vi "main4Ch.vi"() -> ()   [LabVIEW 2024]
doc: "Main VI for FLS imaging system."
uses:
  SubVI/DigitizerConfiguration/FLImDAQ.ctl
  <instrlib>/niScope/Controls/niScope trigger source.ctl
  SubVI/LabJack/LJ Pin Setting.ctl
  ConfigFiles/AimingBeamVideoConfig.ctl
  LaguerreDeconLib/DeconEngineClass/LaguerreDeconEngineClass.lvclass/LaguerreDeconEngineClass.ctl
  <vilib>/Utility/error.llb/DialogType.ctl
  LaguerreDeconLib/DeconEngineClass/LaguerreDeconEngineClass.lvclass
  <vilib>/event_ctls.llb/usereventprio.ctl
  <vilib>/Utility/miscctls.llb/LVMinMaxIncTypeDef.ctl
  SubVI/APD/APDClass.lvclass
  <vilib>/Analysis/baseanly.llb/Mean (DBL).vi
  SubVI/GlobalVariables.vi
  <vilib>/addons/control/pid/pid.llb/PID (DBL).vi
  <instrlib>/niScope/Acquire/Fetch/niScope Multi Fetch Binary 16.vi
  <vilib>/Instr/_visa.llb/VISA Configure Serial Port (Instr).vi
  <userlib>/_OpenG.lib/file/file.llb/openg_file.lvlib
  <userlib>/_OpenG.lib/time/time.llb/openg_time.lvlib
  <vilib>/Analysis/NI_AALBase.lvlib
  <vilib>/Utility/miscctls.llb/LVPointTypeDef.ctl
  <vilib>/addons/control/pid/NI_PID_pid.lvlib
panel:
  in  "Overlay selection":u16(ring)=1 items=["Gain", "Lifetime"]
  out "Record Backlog 2":i32
  in  "Auto gain ch4":bool=TRUE caption="Auto gain ch3"
  in  "V 4":dbl caption="Gain 3" min=0.0 max=4.67 step=0.1
  out "Gain4":dbl
  out "Lifetime 4":dbl caption="Lifetime 3"
  out "IntR4":dbl format="%#_2g"
  out "SNR4":dbl format="%#_3g"
  out "Channel 4":dbl[][](graph) caption="Channel 3"
  out "RunStartTime":u32
  out "Dig1 Temp":dbl
  out "Dig2 Temp":dbl
  out "Visualization PC video source":T1
  in  "V target(1.0)":dbl=1.0 caption="V target(1.5)" min=0.3 max=1.5 step=0.1 format="%#_4g"
  out "SNR3":dbl format="%#_3g"
  out "SNR2":dbl format="%#_3g"
  out "SNR1":dbl format="%#_3g"
  in  "Show BG removed?":bool=TRUE
  out "IntR3":dbl format="%#_2g"
  out "IntR2":dbl format="%#_2g"
  out "IntR1":dbl format="%#_2g"
  in  "Video Display":bool
  out "Gain3":dbl
  out "Gain2":dbl
  out "Gain1":dbl
  in  "Skip Data Save?":bool
  out "Aq Loop?":bool
  out "ML?":bool
  out "aquisition loop Error Out":errorcluster
  out "Laser f (Hz)":dbl
  out "Record Backlog":i32
  out "Fetch Record #":i32
  out "Sync Success?":bool
  out "Disclamer":picture
  out "Calibration #":i8
  out "BG #":i8
  in  "TCP Connect":bool
  out "Help":string
  in  "355nm Laser toggle":bool caption="355nm 460Hz"
  in  "Cali&iRF alignment":bool
  in  "Background":bool
  in  "Aiming beam toggle":bool caption="445nm 0Hz 32mA"
  out "Lifetime 3":dbl
  out "Lifetime 2":dbl
  in  "Auto gain ch3":bool=TRUE
  in  "Auto gain ch2":bool=TRUE
  in  "Auto gain ch1":bool=TRUE
  out "Run #":i8
  in  "StopButton":bool caption="Stop"
  out "Aquisition Status:":bool
  in  "StartButton":bool caption="Start"
  in  "V 3":dbl caption="Gain 3" min=0.0 max=4.65 step=0.1
  in  "V 2":dbl caption="Gain 2" min=0.0 max=4.59 step=0.1
  out "Lifetime 1":dbl
  in  "V 1":dbl caption="Gain 1" min=0.0 max=4.63 step=0.1 format="%#_4g"
  in  "Video Source":enum32{"Camera", "FrameGrabber"}(radio)
  out "Case #":string
  out "System Hardware Connection Status":T2
  out "Channel 3":dbl[][](graph)
  out "Channel 2":dbl[][](graph)
  out "Channel 1":dbl[][](graph)
  in  "Tab Control":T3(tab)
  out "display loop timing(ms)":u32
  out "Aquisition loop timing(ms)":u32 format="%.2f"
  out "DisplayLoop":i32
  out "PID loop":i32 caption="processing loop"
  out "PID loop timing(ms)":u32 caption="processing loop timing(ms)"
  out "Communication loop(ms)":u32
  out "laser EM lamp V":dbl format="%0.6f"
  out "Decon Loop timing (ms)":dbl
  out "Auisition Loop idx":i32
  out "LJ process (ms)":u32
  out "LJ time(ms)":u32[](array[numeric])
  out "output variable":i32
  out "Lifetime (ns)":dbl(graph)
  out "DeCon Speed(ms)":dbl(graph)
  in  "Truncation":u32=600
  out "iRF Graph":dbl[][](graph)
  in  "Show BG":bool
  out "iRF length":i32
  out "BG length":i32
  out "data length":i32
  out "LJ Pinout":T4={"Ch1 Bias"="DAC0", "Ch2 Bias"="DAC1", "Ch3 Bias"="DAC2", "Ch4 Bias"="DAC0", "355 PWM"="FIO0", "AimingBeam PWM"="FIO2", "Laser Ready"="FIO3", "Interlock"="FIO1", "Laser Start/Stop"="FIO1", "Red LED"="FIO1", "Green LED"="DIO3", "Foot Pedal"="DIO15"}
  out "FLImDAQ":T5={"Digitizer 1"="", "Digitizer 2"="", "Channel"=enum."Channel 0", "trigger source"="VAL_EXTERNAL", "trigger level"=0.5, "trigger delay"=1.35e-07, "min sample rate"=12500000000.0, "min record length"=2500, "vertical range"=1.0, "vertical offset"=-0.25, "Waveform to Avg"=2000} caption="FLIm DAQ Configuration" {"trigger delay" format="%^#.4e"; "trigger level" min=0.0 max=3.5 step=0.5 format="%.2f"; "vertical offset" format="%.4f"; "vertical range" format="%.2f"; "min sample rate" format="%#.2p"}
  in  "Sys Reconfig":bool
  out "data out(communcation loop)":string
  out "PID loop error out":errorcluster caption="processing Error Out"
  out "decon error out":errorcluster
  out "Laser Rep Rate":dbl
  out "V4 Size":i32 caption="V3 Size"
  in  "Data Class":enum16{"Data", "BG", "Cali"}(ring)
  out "V1 Size":i32
  out "V2 Size":i32
  out "V3 Size":i32
  out "data Size":i32[](array[numeric])
  out "State log":string
  out "SysConfigCluster":T7
  in  "Ch4 PID gains":T8={"proportional gain (Kc)"=30.0, "integral time (Ti, min)"=0.0003, "derivative time (Td, min)"=1e-05}
  in  "Ch3 PID gains":T8={"proportional gain (Kc)"=30.0, "integral time (Ti, min)"=0.0003, "derivative time (Td, min)"=1e-05}
  in  "Ch2 PID gains":T8={"proportional gain (Kc)"=30.0, "integral time (Ti, min)"=0.0003, "derivative time (Td, min)"=1e-05}
  in  "Ch1 PID gains":T8={"proportional gain (Kc)"=30.0, "integral time (Ti, min)"=0.0003, "derivative time (Td, min)"=1e-05}
  in  "Quit":bool
  in  "Radio Buttons":T9(radio)=enum."Ch2" caption="DeCon Chan"
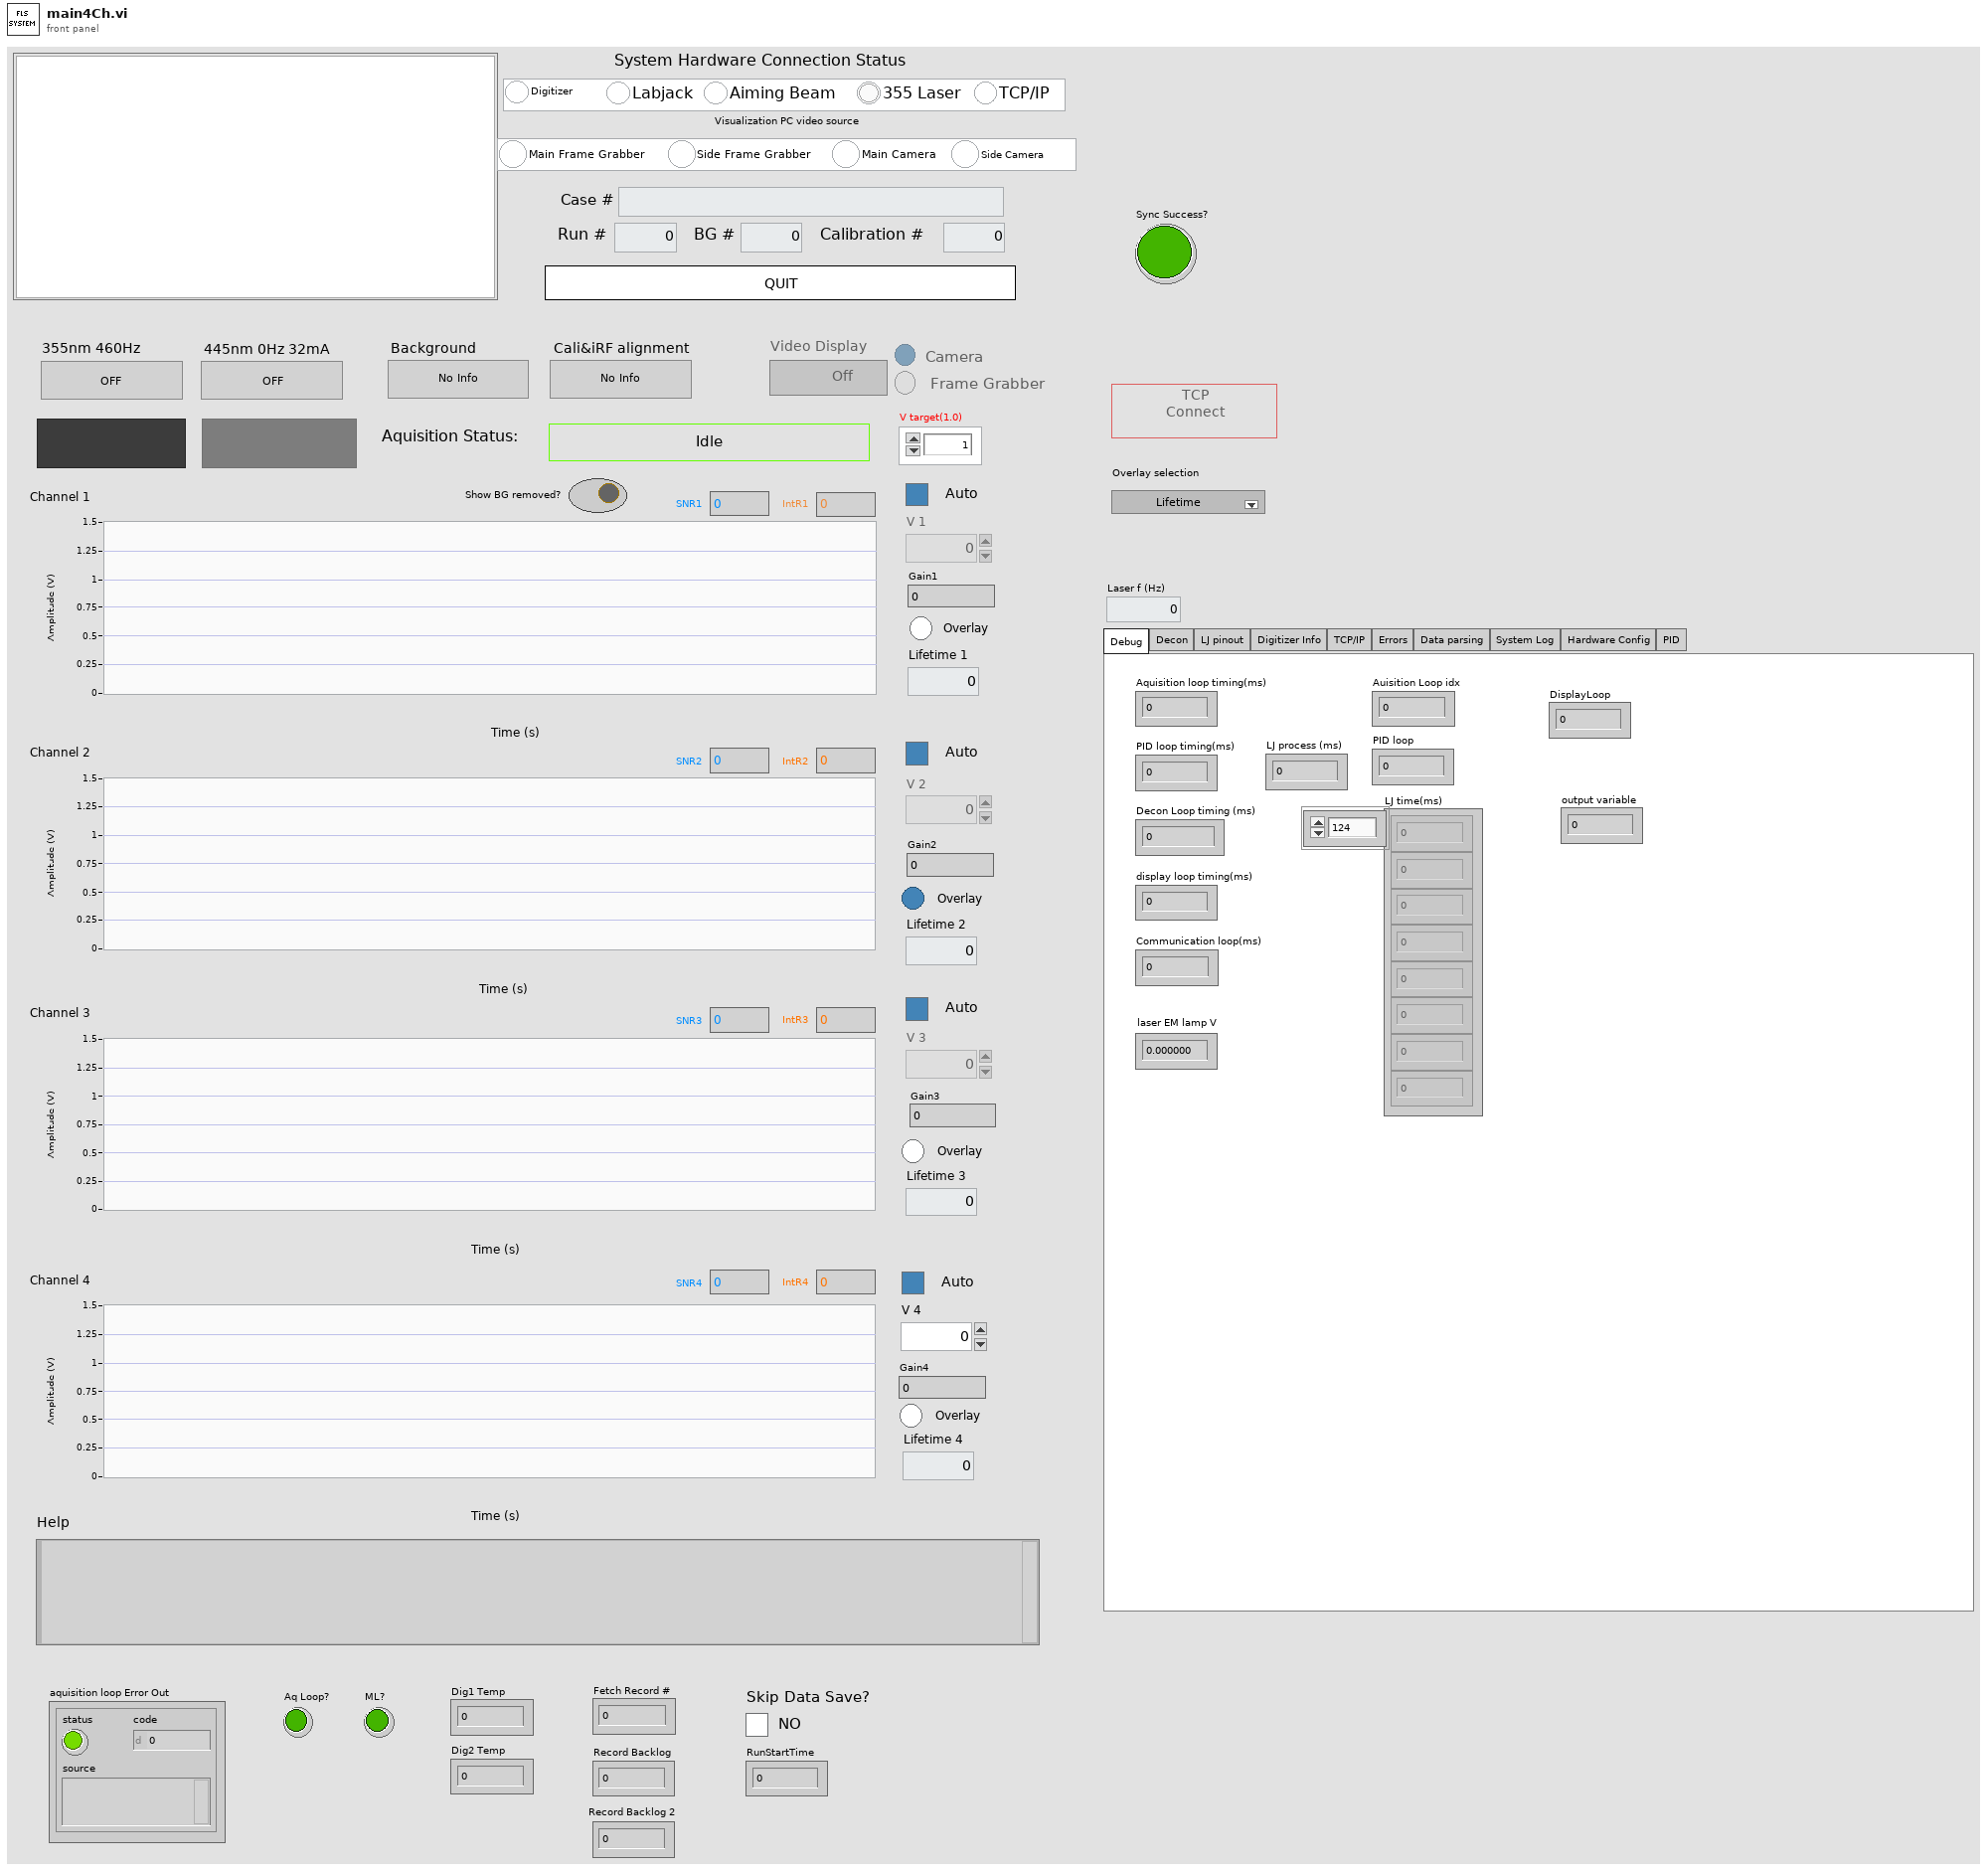
[diagram p1: front panel]
types:
  T1 = cluster{"Main Frame Grabber":bool, "Side Frame Grabber":bool, "Main Camera":bool, "Side Camera":bool}
  T2 = cluster{"Digitizer":bool, "Labjack":bool, "Aiming Beam":bool, "355 Laser":bool, "TCP/IP":bool}
  T3 = enum32{"Debug", "Decon", "LJ pinout", "Digitizer Info", "TCP/IP", "Errors", "Data parsing", "System Log", "Hardware Config", "PID"}
  T4 = typedef "LJ Pin Setting.ctl" = cluster{"Ch1 Bias":string, "Ch2 Bias":string, "Ch3 Bias":string, "Ch4 Bias":string, "355 PWM":string, "AimingBeam PWM":string, "Laser Ready":string, "Interlock":string, "Laser Start/Stop":string, "Red LED":string, "Green LED":string, "Foot Pedal":string}
  T5 = typedef "FLImDAQ.ctl" = cluster{"Digitizer 1":refnum<k15>, "Digitizer 2":refnum<k15>, "Channel":enum16{"Channel 0", "Channel 1", "Channel 0&1"}, "trigger source":T6, "trigger level":dbl, "trigger delay":dbl, "min sample rate":dbl, "min record length":i32, "vertical range":dbl, "vertical offset":dbl, "Waveform to Avg":i16}
  T6 = typedef "niScope trigger source.ctl" = string
  T7 = cluster{"Ch1Enable?":bool, "Ch2Enable?":bool, "Ch3Enable?":bool, "Ch1AutoGain?":bool, "Ch2AutoGain?":bool, "Ch3AutoGain?":bool, "AimingBeamEnable?":bool}
  T8 = cluster{"proportional gain (Kc)":dbl, "integral time (Ti, min)":dbl, "derivative time (Td, min)":dbl}
  T9 = enum32{"No Selection", "Ch1", "Ch2", "Ch3", "Ch4"}
  T10 = cluster{"remote start event":refnum<user-event>, "remote stop  event":refnum<user-event>}
  T11 = enum8{"Enabled", "Disabled", "Disabled and Grayed Out"}
  T12 = enum16{"open", "replace", "create", "open or create", "replace or create", "replace or create with confirmation"}
  T13 = cluster{"CH1":dbl[][], "CH2":dbl[][], "CH3":dbl[][], "CH4":dbl[][], "Gain cluster":cluster{"V1":dbl, "V2":dbl, "V3":dbl, "V4":dbl}}
  T14 = cluster{"idx":i32, "CH1&2":dbl[][], "CH3":dbl[][], "V cluster":cluster{"V1":dbl, "V2":dbl, "V3":dbl, "V4":dbl}}
  T15 = typedef "usereventprio.ctl" = enum32{"high priority", "normal priority"}
  T16 = cluster{"actualSamples":i32, "absoluteInitialX":dbl, "relativeInitialX":dbl, "xIncrement":dbl, "offset":dbl, "gain":dbl, "reserved1":dbl, "reserved2":dbl}[]
  T17 = cluster{"V1 out":dbl, "V2 out":dbl, "V3 out":dbl, "V3 out":dbl}
  T18 = cluster{i32, dbl[][], dbl[][], cluster{"V1 out":dbl, "V2 out":dbl, "V3 out":dbl, "V3 out":dbl}}
  T19 = cluster{"Ch1 iRF":dbl[], "Ch2 iRF":dbl[], "Ch3 iRF":dbl[], "Ch4 iRF":dbl[]}
  T20 = enum16{"open", "open or create", "create or replace", "create", "open (read-only)"}
  T21 = enum32{"Invalid", "Standard", "Closed", "Hidden", "Minimized", "Maximized"}
  T22 = enum32{"invalid app kind", "Development System", "Run Time System", "Student Edition", "Embedded LabVIEW", "Evaluation", "Custom"}
  T23 = enum32{"Bad", "Idle", "Run top level", "Running"}
  T24 = enum16{"Standard", "Buffered", "CRLF", "Immediate"}
  T25 = typedef "AimingBeamVideoConfig.ctl" = cluster{"DeCon Channel":enum16{"1", "2", "3"}, "Scale Bar":bool, "Scale Low":dbl, "Scale High":dbl, "ANSI":dbl, "Radius":dbl, "3D?":bool, "Firefly?":bool, "Pentero?":bool}
  T26 = cluster{"Core":cluster{"Current VI Reference":refnum<vi>, "Close Panel on Exit?":bool}, "SysConfigCluster":cluster{"Ch1Enable?":bool, "Ch2Enable?":bool, "Ch3Enable?":bool, "Ch1AutoGain?":bool, "Ch2AutoGain?":bool, "Ch3AutoGain?":bool, "AimingBeamEnable?":bool}, "System Status":cluster{"Digitizer":bool, "Labjack":bool, "Aiming Beam":bool, "355 Laser":bool, "TCP/IP":bool}, "IDs":cluster{"RunID":i8, "BG ID":i8, "Cali ID":i8}, "CaseID":string, "DefaultPath":path, "Pathes":cluster{"DataPath":path, "BG Path":path, "iRFPath":path, "CaliPath":path}, "FLImDAQ":cluster{"resource name":refnum<k15>, "resource name 2":refnum<k15>, "Channel":enum16{"Channel 0", "Channel 1", "Channel 0&1"}, "trigger source":T6, "trigger level":dbl, "trigger delay":dbl, "min sample rate":dbl, "min record length":i32, "vertical range":dbl, "vertical offset":dbl, "Waveform to Avg":i32}, "SysRunning?":bool, "AB Cluster":cluster{"Aiming Beam COM Port":refnum<visa-resource-name>, "Min Current":dbl, "Max Current":dbl, "Default Current":dbl, "Freq":i32}, "LJ Pinout":T4, "355 PWM setting":cluster{"DIO_EF_CLOCK1_DIVISOR":i16, "DIO_EF_CLOCK1_ROLL_VALUE":i32, "DIO#_EF_INDEX":i16, "DIO#_EF_OPTIONS":i16, "DIO#_EF_CONFIG_A":i32}, "AB PWM setting":cluster{"DIO_EF_CLOCK1_DIVISOR":i16, "DIO_EF_CLOCK1_ROLL_VALUE":i32, "DIO#_EF_INDEX":i16, "DIO#_EF_OPTIONS":i16, "DIO#_EF_CONFIG_A":i32}, "Last Trigger":u32, "niTClk sessions":refnum<k20>[], "Laser start tic":u32, "TCP attempt count":i32, "Ch1Data":dbl[][], "Ch2Data":dbl[][], "Ch3Data":dbl[][], "Ch4Data":dbl[][], "V1":dbl[], "V2":dbl[], "V3":dbl[], "V4":dbl[], "SlowTimer":u32, "FastTimer":u32, "listener ID":refnum<k5>, "TempPath":path, "CaliPath":path, "LED vi reference":refnum<vi>, "Aquisition Timer":u32, "APDSerialNum":cluster{"Ch1APDSerial#":string, "Ch2APDSerial#":string, "Ch3APDSerial#":string, "Ch4APDSerial#":string}, "VideoConfig":T25, "LED vi ref open?":bool, "video source":cluster{"Main Frame Grabber":bool, "Side Frame Grabber":bool, "Main Camera":bool, "Side Camera":bool}, "bothVidSourceAvail":bool}
  T27 = typedef "LVCursorListTypeDef.ctl" = cluster{"Name":string, "Color":u32, "Style":u8, "Point Style":u8, "Name Visible":bool, "Allow Drag":bool, "Cursor Mode":u32, "Plot":i32, "Index":i32, "Position":cluster{"X":dbl, "Y":dbl}, "X Scale":u32, "Y Scale":u32, "Watch Plots":i32[], "Watch All Plots":bool, "Plot Area":i32, "Label Offset":cluster{"X":dbl, "Y":dbl}}[]
  T28 = cluster{"Name":string, "Color":u32, "Style":u8, "Point Style":u8, "Name Visible":bool, "Allow Drag":bool, "Cursor Mode":u32, "Plot":i32, "Index":i32, "Position":cluster{"X":dbl, "Y":dbl}, "X Scale":u32, "Y Scale":u32, "Watch Plots":i32[], "Watch All Plots":bool, "Plot Area":i32, "Label Offset":cluster{"X":dbl, "Y":dbl}}
  T29 = cluster{"Ch1APDSerial#":string, "Ch2APDSerial#":string, "Ch3APDSerial#":string, "Ch4APDSerial#":string}
  T30 = cluster{"DataPath":path, "BG Path":path, "iRFPath":path, "CaliPath":path}
  T31 = cluster{"DIO_EF_CLOCK1_DIVISOR":i16, "DIO_EF_CLOCK1_ROLL_VALUE":i32, "DIO#_EF_INDEX":i16, "DIO#_EF_OPTIONS":i16, "DIO#_EF_CONFIG_A":i32}
  T32 = cluster{"Aiming Beam COM Port":refnum<visa-resource-name>, "Min Current":dbl, "Max Current":dbl, "Default Current":dbl, "Freq":i32}
  T33 = cluster{"resource name":refnum<k15>, "resource name 2":refnum<k15>, "Channel":enum16{"Channel 0", "Channel 1", "Channel 0&1"}, "trigger source":T6, "trigger level":dbl, "trigger delay":dbl, "min sample rate":dbl, "min record length":i32, "vertical range":dbl, "vertical offset":dbl, "Waveform to Avg":i32}
  T34 = cluster{"Current VI Reference":refnum<vi>, "Close Panel on Exit?":bool}
  T35 = cluster{"Channel 1":dbl[], "Channel 2":dbl[], "Channel 3":dbl[], "Channel 4":dbl[]}
  T36 = cluster{"V 1":dbl[], "V 2":dbl[], "V 3":dbl[], "V 4":dbl[]}
  T37 = cluster{"Ch1 WF":dbl[], "Ch2 WF":dbl[], "Ch3 WF":dbl[], "Ch4 WF":dbl[], "V1":dbl, "V2":dbl, "V3":dbl, "V4":dbl}
  T38 = typedef "iRFData.ctl" = cluster{"dt":dbl, "NumOfWFs":i32, "WFLength":i32, "iRFCtrlV":dbl[], "iRFWFsAvg":dbl[][], "iRFRaw":dbl[][]}
  T39 = cluster{"mean":dbl, "mean":dbl, "mean":dbl, "mean":dbl}
  T40 = cluster{"V1":dbl, "V2":dbl, "V3":dbl, "V4":dbl}[]
  T41 = cluster{"DataPath":path, "CaseID":string, "RunID":i16, "Ch1Data":dbl[][], "Ch2Data":dbl[][], "Ch3Data":dbl[][], "Ch4Data":dbl[][], "V1":dbl[], "V2":dbl[], "V3":dbl[], "V4":dbl[], "LaserRepRate":u16, "WFAverage":i16, "RunStartTime":u64}
  T42 = typedef "DialogType.ctl" = u16
  T43 = typedef "LJ PWM Setting.ctl" = cluster{"DIO_EF_CLOCK1_DIVISOR":i16, "DIO_EF_CLOCK1_ROLL_VALUE":i32, "DIO#_EF_INDEX":i16, "DIO#_EF_OPTIONS":i16, "DIO#_EF_CONFIG_A":i32}
  T44 = typedef "AimingBeam.ctl" = cluster{"Aiming Beam COM Port":refnum<visa-resource-name>, "Min Current":dbl, "Max Current":dbl, "Default Current":dbl, "Frequency(Hz)":u32}
  T45 = cluster{"DC1":i32, "DC2":i32, "BG1":i32, "BG2":i32}
  T46 = typedef "LVMinMaxIncTypeDef.ctl" = cluster{"Minimum":dbl, "Maximum":dbl, "Increment":dbl}
  T47 = typedef "LVBoundsTypeDef.ctl" = cluster{"Width":u32, "Height":u32}
  T48 = typedef "imagedata.ctl" = cluster{"image type":i32, "image depth":i32, "image":u8[], "mask":u8[], "colors":u32[], "Rectangle":cluster{"left":i16, "top":i16, "right":i16, "bottom":i16}}
  T49 = cluster{"DC Idx1":i32, "DC Idx2":i32, "BG Idx1":i32, "BG Idx2":i32}
  T50 = cluster{dbl[][], dbl[][], dbl[][], dbl[][], "V cluster":cluster{"V1":dbl, "V2":dbl, "V3":dbl, "V4":dbl}}
  T51 = typedef "LVPointTypeDef.ctl" = cluster{"Horizontal":i16, "Vertical":i16}
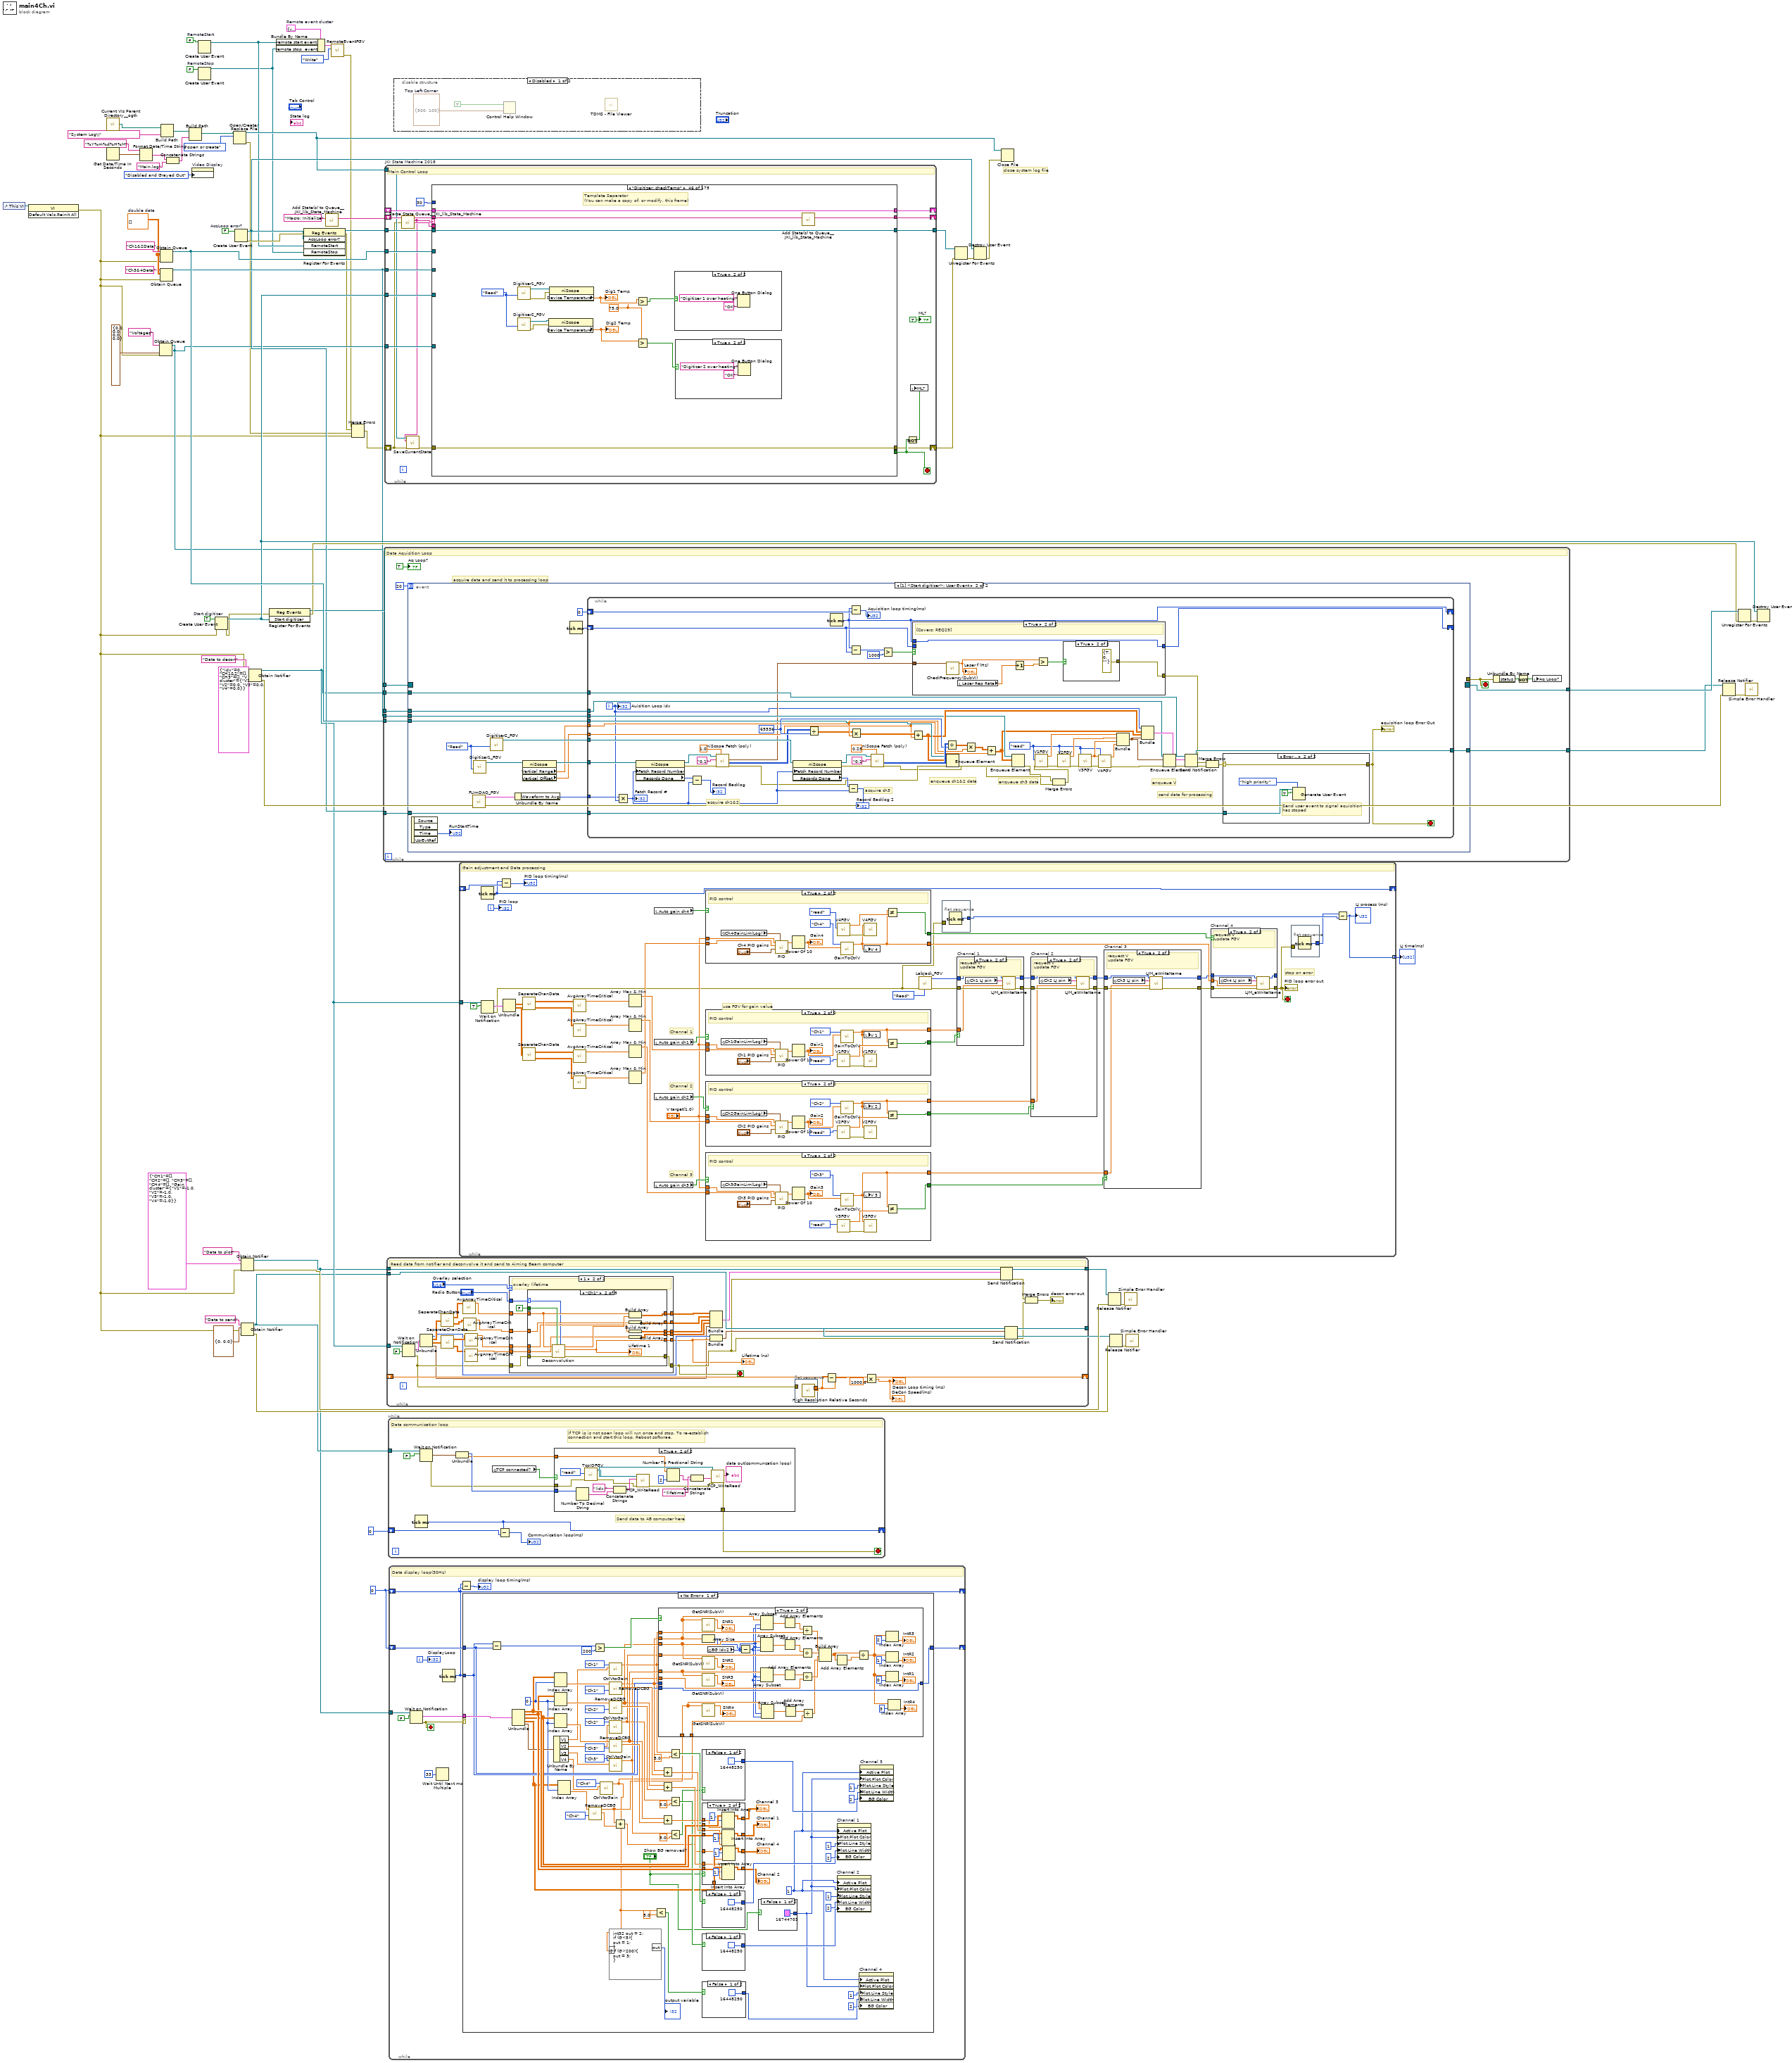
[diagram p0: block diagram]
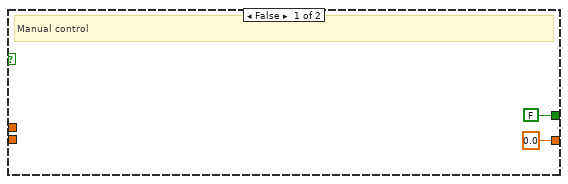
[diagram p6: hidden frame]
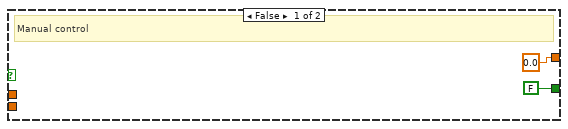
[diagram p7: hidden frame]
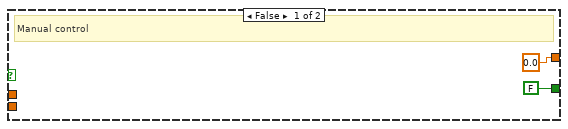
[diagram p8: hidden frame]
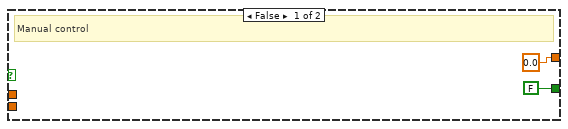
[diagram p9: hidden frame]
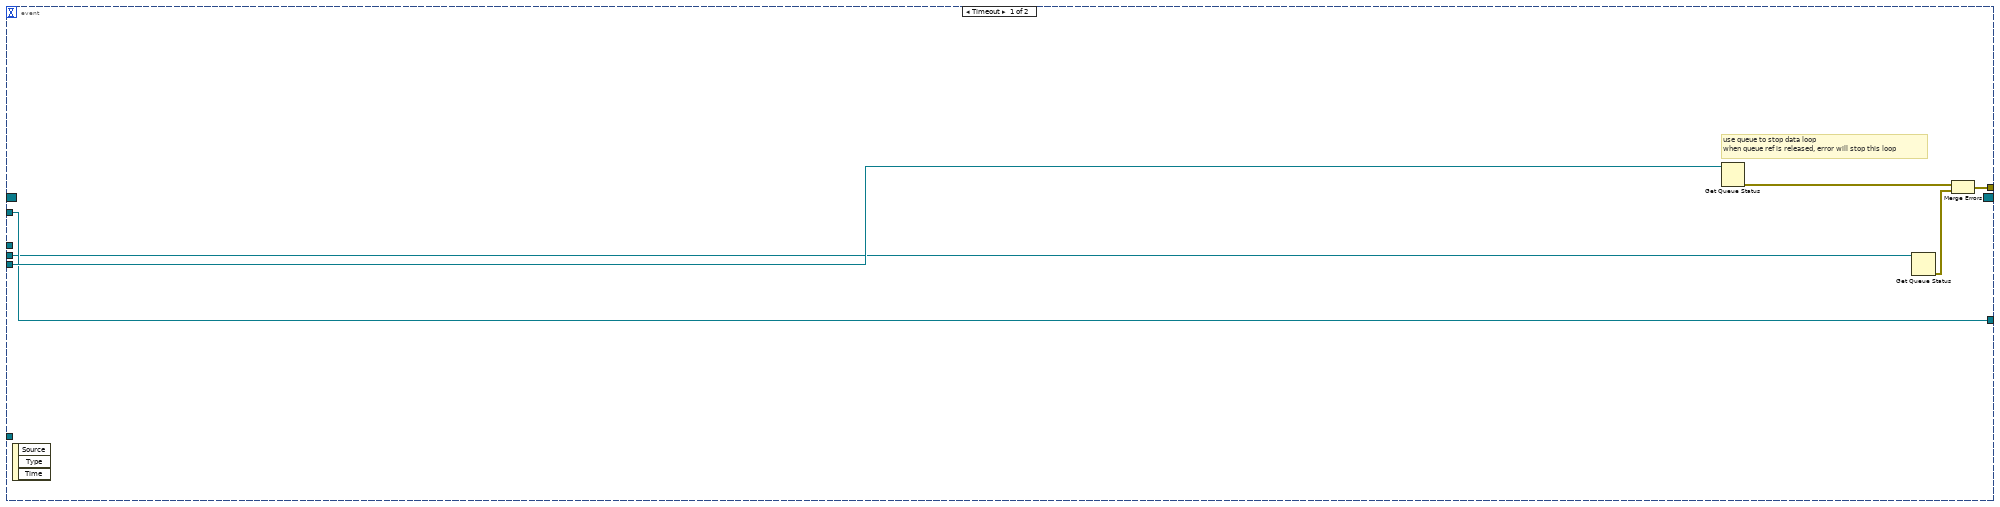
[diagram p10: hidden frame]
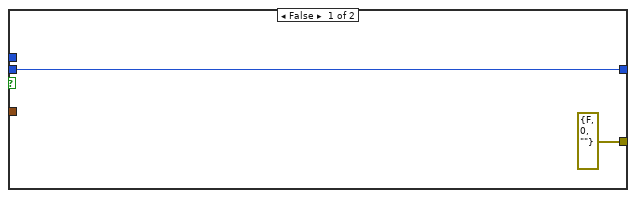
[diagram p11: hidden frame]
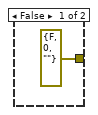
[diagram p12: hidden frame]
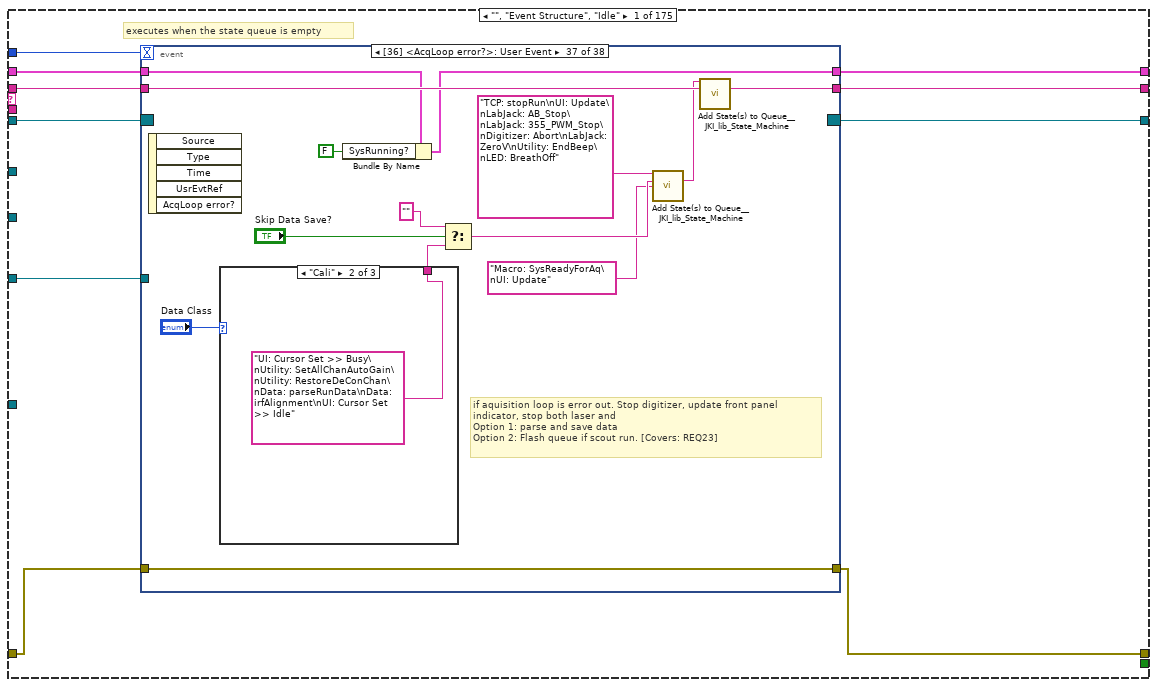
[diagram p14: hidden frame]
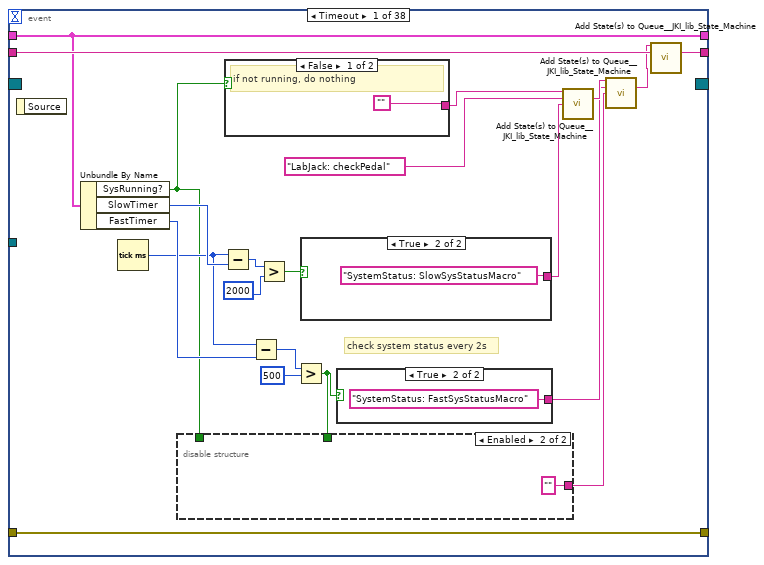
[diagram p15: hidden frame]
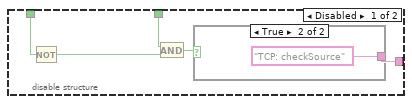
[diagram p16: hidden frame]
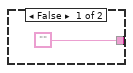
[diagram p17: hidden frame]
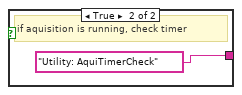
[diagram p18: hidden frame]
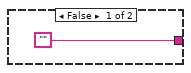
[diagram p19: hidden frame]
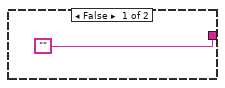
[diagram p20: hidden frame]
diagram:
  w8 = T10 {"remote start event"=refnum, "remote stop  event"=refnum}  # Remote event cluster
  w11 = FALSE  # RemoteStop
  w12 = FALSE  # RemoteStart
  w15 = u32 0 ("millisecond timer value")
  w54 = FALSE  # AcqLoop error?
  w64 = TRUE  # Start digitizer
  w67 = dbl[][] []  # double data
  # "close system log file"
  n1 = control-ref of="This VI"() -> (w69:refnum<vi>)
  n2 = invoke on="Invoke Node" class="VI" method="Default Vals.Reinit All"(reference=w69) -> (error out=w23:errorcluster)  [unwired: 2 in, 2 out]
  n3 = call <userlib>:"Current VIs Parent Directory__ogtk.vi"() -> ("Parent Directory (+ Relative)"=w34:path)  [unwired: 5 in]
  n4 = Get Date/Time In Seconds() -> (seconds since 1Jan1904=w32:timestamp)
  n5 = Format Date/Time String(time format string (%c)="%Y%m%d%H%M", seconds (now)=w32) -> (date/time string=w29:string)  [unwired: 1 in]
  n6 = Obtain Queue(name (unnamed)="Voltages", element data type=cluster{"V1":dbl, "V2":dbl, "V3":dbl, "V4":dbl} {"V1"=0.0, "V2"=0.0, "V3"=0.0, "V4"=0.0}, error in (no error)=w23) -> (queue out=w35:refnum<queue>)  [unwired: 2 in, 2 out]
  n7 = Obtain Queue(name (unnamed)="Ch3&4Data", element data type=w67, error in (no error)=w23) -> (queue out=w48:refnum<queue>)  [unwired: 2 in, 2 out]
  n8 = Obtain Queue(name (unnamed)="Ch1&2Data", element data type=w67, error in (no error)=w23) -> (queue out=w65:refnum<queue>)  [unwired: 2 in, 2 out]
  n9 = Build Path(base path=w34, name or relative path="System Log\\") -> (appended path=w25:path)
  n10 = Concatenate Strings(w29, "Main.log" ("string")) -> (w27:string)
  n11 = Build Path(base path=w25, name or relative path=w27) -> (appended path=w30:path)
  n12 = property on="Video Display" class="Bool (strict)"("DisabledEnum"=T11."Disabled and Grayed Out" ("Disabled")) -> ()  [unwired: 2 in, 2 out]
  n13 = Create User Event(user event datatype=w12) -> (user event=w10:refnum<user-event>)  [unwired: 1 in, 1 out]
  n14 = Create User Event(user event datatype=w11) -> (user event=w9:refnum<user-event>)  [unwired: 1 in, 1 out]
  n15 = Create User Event(user event datatype=w64, error in=w23) -> (user event=w53:refnum<user-event>, error out=w40:errorcluster)
  n16 = Open/Create/Replace File(file path (use dialog)=w30, operation (0:open)=T12."open or create") -> (refnum out=w21:refnum<file>, error out=w22:errorcluster)  [unwired: 4 in, 1 out]
  n17 = Create User Event(user event datatype=w54) -> (user event=w39:refnum<user-event>, error out=w41:errorcluster)  [unwired: 1 in]
  n18 = Obtain Notifier(name (unnamed)="Data to plot", notification data type=T13 {"CH1"=[], "CH2"=[], "CH3"=[], "CH4"=[], "Gain cluster"={"V1"=-1.0, "V2"=-1.0, "V3"=-1.0, "V4"=-1.0}}, error in (no error)=w23) -> (notifier out=w13:refnum<notifier>, error out=w49:errorcluster)  [unwired: 1 in, 1 out]
  n19 = Obtain Notifier(name (unnamed)="Data to send", notification data type=cluster{"idx":i32, "lifetime":dbl} {"idx"=0, "lifetime"=0.0}, error in (no error)=w23) -> (notifier out=w18:refnum<notifier>, error out=w38:errorcluster)  [unwired: 1 in, 1 out]
  n20 = Obtain Notifier(name (unnamed)="Data to decon", notification data type=T14 {"idx"=0, "CH1&2"=[], "CH3"=[], "V cluster"={"V1"=0.0, "V2"=0.0, "V3"=0.0, "V4"=0.0}}, error in (no error)=w23) -> (notifier out=w19:refnum<notifier>, error out=w58:errorcluster)  [unwired: 1 in, 1 out]
  n21 = register-events(error in=w40, w53) -> (reference out=w55:refnum<event-registration>, error out=w61:errorcluster)  [unwired: 1 in]
  n22 = Bundle By Name(cluster=w8, "remote start event"=w10, "remote stop  event"=w9) -> (w6:T10)
  n23 = register-events(error in=w41, w39, w10, w9) -> (reference out=w47:refnum<event-registration>, error out=w5:errorcluster)  [unwired: 1 in]
  n24 = call <vilib>:"Add State(s) to Queue__JKI_lib_State_Machine.vi"("State(s) in (\"\")"="Macro: Initialize") -> ("States Out"=w71:string)  [unwired: 14 in]
  n25 = call "RemoteEventFGV.vi"("Operation (Read)"=enum16{"Read", "Write"}."Write", "Remote Event in"=w6) -> ("Error Out"=w2:errorcluster)  [unwired: 8 in, 1 out]
  n26 = Merge Errors(w2, w5, w22, w23) -> (w24:errorcluster)
  n27 = while {
    tunnel: w65 -> [w84]
    tunnel: w55 -> [w83]
    tunnel: [w82] -> w63
    tunnel: w19 -> [w81]
    tunnel: [w80] -> w59
    tunnel: w39 -> [w78]
    tunnel: w48 -> [w77]
    tunnel: w35 -> [w72]
    stop <- w75 stop-if-true
    # "acquire data and send it to processing loop"
    # "Data Aquisition Loop"
    n28 = event shown="[1] <Start digitizer>: User Event" {
      selector: w83 -> [_ _]
      dyn-events: [_ _] -> w82
      timeout: 20 -> [_ _]
      tunnel: w84 -> [w90 w100]
      tunnel: [w85 _] -> w75
      tunnel: w81 -> [w89 w107]
      tunnel: [w89 w106] -> w80
      tunnel: w78 -> [_ w104]
      tunnel: w77 -> [w88 w99]
      tunnel: w72 -> [_ w97]
      event Timeout {
        # "use queue to stop data loop\nwhen queue ref is released, error will stop this loop"
        n29 = event-data() -> ()  [unwired: 1 in, 3 out]
        n30 = Get Queue Status(queue=w90) -> (error out=w87:errorcluster)  [unwired: 2 in, 7 out]
        n31 = Get Queue Status(queue=w88) -> (error out=w86:errorcluster)  [unwired: 2 in, 7 out]
        n32 = Merge Errors(w87, w86) -> (w85:errorcluster)
      }
      event User Event {
        w105 = enum16{"Write", "Read"}."Read" ("Operation")
        n33 = event-data() -> ("Time"=→"RunStartTime":u32)  [unwired: 1 in, 3 out]
        n34 = call "FLImDAQ_FGV.vi"() -> ("Read data"=w102:T5)  [unwired: 10 in, 1 out]
        n35 = call "Digitizer1_FGV.vi"("Operation (Read)"=w105) -> ("Read data"=w96:refnum<k15>)  [unwired: 9 in, 1 out]
        n36 = call "Digitizer2_FGV.vi"("Operation (Read)"=w105) -> ("Read data"=w103:refnum<k15>)  [unwired: 9 in, 1 out]
        n37 = Unbundle By Name(w102) -> ("Waveform to Avg"=w101:i16)
        n38 = property on="Property Node" class="niScope"(reference=w96) -> (reference out=w95:refnum<k15>, "Vertical Range"=w94:dbl, "Vertical Offset"=w93:dbl)  [unwired: 1 in, 1 out]
        n39 = Tick Count (ms)() -> (millisecond timer value=w92:u32)
        n40 = while {
          tunnel: w107 -> [w167]
          tunnel: [w166] -> w106
          tunnel: w103 -> [w160]
          tunnel: w95 -> [w159]
          tunnel: w104 -> [w158]
          shift-right: [w127] -> _
          shift-left: u32 0 ("millisecond timer value") -> [w152]
          tunnel: w101 -> [w108]
          tunnel: w100 -> [w149]
          tunnel: w99 -> [w147]
          tunnel: w97 -> [w140]
          tunnel: w94 -> [w137]
          tunnel: w93 -> [w138]
          shift-right: [w132] -> _
          shift-left: w92 -> [w131]
          i -> [w109]
          stop <- w130 stop-if-true
          w120 = enum16{"write", "read"}."read" ("action")
          w153 = 65536
          # "enqueue V"
          # "enqueue ch3 data"
          # "enqueue ch1&2 data"
          # "acquire ch3"
          # "acquire ch1&2"
          # "send data for processing"
          n41 = Multiply(x=w108, y=w109) -> (x*y=w117:i32)
          "Fetch Record #" <- w117
          n42 = property on="Property Node" class="niScope"(reference=w159, "Fetch Record Number"=w117) -> (reference out=w171:refnum<k15>, error out=w170:errorcluster, "Records Done"=w139:i32)  [unwired: 1 in]
          n43 = Subtract(x=w139, y=w117) -> (x-y=→"Record Backlog":i32)
          n44 = call-poly <instrlib>:"niScope Fetch (poly).vi"("timeout"=1.0, "error in"=w170, "channels"="0,1", "instrument handle"=w171) -> ("error out"=w114:errorcluster, "wfm"=w115:i16[][], "wfm info"=w136:T16)  [unwired: 4 in, 1 out]
          n45 = property on="Property Node" class="niScope"(reference=w160, "Fetch Record Number"=w117) -> (reference out=w164:refnum<k15>, error out=w161:errorcluster, "Records Done"=w118:i32)  [unwired: 1 in]
          n46 = Divide(x=w115, y=w153) -> (x/y=w126:dbl[][])
          n47 = Tick Count (ms)() -> (millisecond timer value=w127:u32)
          n48 = Subtract(x=w118, y=w117) -> (x-y=→"Record Backlog 2":i32)
          n49 = Subtract(x=w127, y=w152) -> (x-y=→"Aquisition loop timing(ms)":u32)
          n50 = Subtract(x=w127, y=w131) -> (x-y=w135:u32)
          n51 = Multiply(x=w126, y=w137) -> (x*y=w157:dbl[][])
          n52 = call-poly <instrlib>:"niScope Fetch (poly).vi"("timeout"=0.25, "error in"=w161, "channels"="0,1", "instrument handle"=w164) -> ("error out"=w113:errorcluster, "wfm"=w154:i16[][])  [unwired: 4 in, 2 out]
          n53 = Greater?(x=w135, y=u32 1000) -> (0:w133:bool)
          n54 = Add(x=w157, y=w138) -> (x+y=w148:dbl[][])
          n55 = case shown="True" w133 {
            tunnel: w136 -> [_ w180]
            tunnel: w127 -> [_ w179]
            tunnel: [w173 w179] -> w132
            tunnel: w131 -> [w173 _]
            tunnel: [errorcluster {"status"=FALSE, "code"=0, "source"=""} ("error constant") w176] -> w128
            frame False {
            }
            frame True {
              # "[Covers: REQ29]"
              n56 = call "CheckFrequency(SubVI).vi"("wfm info"=w180) -> ("f (Hz)"=w178:dbl)  [unwired: 10 in]
              "Laser f (Hz)" <- w178
              n57 = local read "Laser Rep Rate"() -> (w175:dbl)
              n58 = Increment(x=w175) -> (x+1=w174:dbl)
              n59 = Greater?(x=w178, y=w174) -> (0:w177:bool)
              n60 = case shown="True" w177 {
                tunnel: [errorcluster {"status"=FALSE, "code"=0, "source"=""} ("error constant") errorcluster {"status"=TRUE, "code"=0, "source"=""} ("error constant")] -> w176
                frame False {
                }
                frame True {
                }
              }
            }
          }
          n61 = Divide(x=w154, y=w153) -> (x/y=w156:dbl[][])
          n62 = Enqueue Element(queue=w149, element=w148, error in (no error)=w114) -> (error out=w112:errorcluster)  [unwired: 1 in, 2 out]
          n63 = Multiply(x=w156, y=w137) -> (x*y=w155:dbl[][])
          n64 = Add(x=w155, y=w138) -> (x+y=w146:dbl[][])
          n65 = Enqueue Element(queue=w147, element=w146, error in (no error)=w113) -> (error out=w111:errorcluster)  [unwired: 1 in, 2 out]
          n66 = Merge Errors(w112, w111) -> (w110:errorcluster)
          n67 = call "V1FGV.vi"("Error In"=w110, "action (write)"=w120) -> ("Error Out"=w144:errorcluster, "V1 out"=w142:dbl)  [unwired: 8 in]
          n68 = call "V2FGV.vi"("Error In"=w144, "action(write)"=w120) -> ("Error Out"=w143:errorcluster, "V2 out"=w141:dbl)  [unwired: 8 in]
          n69 = call "V3FGV.vi"("Error In"=w143, "action(write)"=w120) -> ("Error Out"=w123:errorcluster, "V3 out"=w122:dbl)  [unwired: 8 in]
          n70 = call "V4FGV.vi"("Error In"=w123, "action(write)"=w120, "V3 in"=w122) -> ("Error Out"=w121:errorcluster, "V3 out"=w119:dbl)  [unwired: 7 in]
          n71 = Bundle("V1 out"=w142, "V2 out"=w141, "V3 out"=w122, "V3 out"=w119) -> (w125:T17)  [unwired: 1 in]
          n72 = Bundle(w109, w148, w146, w125) -> (w150:T18)  [unwired: 1 in]
          n73 = Enqueue Element(queue=w140, element=w125, error in (no error)=w121) -> (error out=w124:errorcluster)  [unwired: 1 in, 2 out]
          n74 = Send Notification(notification=w150, notifier=w167, error in (no error)=w124) -> (notifier out=w166:refnum<notifier>, error out=w129:errorcluster)
          n75 = Merge Errors(w128, w129) -> (w145:errorcluster)
          n76 = case shown="Error .." w145 {
            selector: w145 -> [w183 w184]
            tunnel: w158 -> [_ w187]
            tunnel: [w183 w184] -> w130
            frame No Error {
            }
            frame Error {
              # "Send user event to signal aquisition has stoped"
              n77 = Generate User Event(priority (normal)=usereventprio."high priority", user event=w187, event data cluster=TRUE ("event data")) -> ()  [unwired: 1 in, 2 out]
            }
          }
          "aquisition loop Error Out" <- w130
          "Auisition Loop idx" <- w109
        }
      }
    }
    n78 = Unbundle By Name(w75) -> ("status"=w74:bool)
    n79 = Not(x=w74) -> (.not. x?=w73:bool)
    n80 = local write "Aq Loop?"(w73) -> ()
    "Aq Loop?" <- TRUE ("Aq L?")
  }
  n81 = while "JKI State Machine 2018" {
    shift-right: [w204] -> _
    shift-left: _ -> [w203]
    shift-right: [w188] -> w4
    shift-left: w24 -> [w190]
    shift-right: [w205] -> _
    shift-left: w71 -> [w206]
    tunnel: w65 -> [w201]
    tunnel: w48 -> [w200]
    tunnel: w53 -> [w199]
    tunnel: w47 -> [w198]
    tunnel: [w197] -> w46
    tunnel: w35 -> [w193]
    tunnel: w21 -> [w192]
    stop <- w196 stop-if-true
    # "Main Control Loop"
    n82 = call <vilib>:"Parse State Queue__JKI_lib_State_Machine.vi"("State Queue"=w206, "Error In (no error)"=w190) -> ("Remaining States"=w208:string, "Current State"=w191:string, "Arguments"=w207:string)  [unwired: 11 in]
    n83 = call "SaveCurrentState.vi"("error in (no error)"=w190, "Current State"=w191, "Byte Stream File in"=w192) -> ("error out"=w189:errorcluster)  [unwired: 8 in]
    n84 = case shown="\"Digitizer: checkTemp\"" w191 {
      selector: w191 -> [_ _ _ _ _ _ _ _ _ _ _ _ _ _ _ _ _ _ _ _ _ _ _ _ w1190 _ _ _ _ _ _ _ _ _ _ _ _ _ _ _ _ _ _ _ _ _ _ _ _ _ _ _ _ _ _ _ _ _ _ _ _ _ _ _ _ _ _ _ _ _ _ _ _ _ _ _ _ _ _ _ _ _ _ _ _ _ _ _ _ _ _ _ _ _ _ _ _ _ _ _ _ _ _ _ _ _ _ _ _ _ _ _ _ _ _ _ _ _ _ _ _ _ _ _ _ _ _ _ _ _ _ _ _ _ _ _ _ _ _ _ _ _ _ _ _ _ _ _ _ _ _ _ _ _ _ _ _ _ _ _ _ _ _ _ _ _ _ _ _ _ _ _ _ _ _]
      tunnel: w208 -> [w218 w626 w635 w641 w647 w669 w682 w724 w730 w757 w776 w847 w862 w893 w920 w952 w966 w995 w1009 w1094 w1131 w1170 w1183 w1188 w1194 w1222 w1230 w1253 w1258 w1271 w1290 w1318 w1346 w1384 w1389 w1395 w1419 w1443 w1467 w1491 w1496 w1513 w1560 w1582 w1598 w1613 w1633 w1638 w1650 w1679 w1705 w1717 w1755 w1768 w1774 w1785 w1797 w1828 w1841 w1855 w1870 w1889 w1924 w1929 w1943 w1953 w1969 w1981 w1993 w2021 w2036 w2041 w2053 w2065 w2070 w2078 w2086 w2095 w2104 w2109 w2117 w2126 w2144 w2161 w2181 w2192 w2214 w2229 w2246 w2251 w2259 w2267 w2272 w2280 w2287 w2295 w2302 w2312 w2340 w2348 w2355 w2363 w2368 w2376 w2383 w2389 w2398 w2414 w2419 w2426 w2438 w2508 w2520 w2529 w2546 w2555 w2578 w2595 w2606 w2619 w2644 w2667 w2673 w2689 w2711 w2719 w2725 w2730 w2737 w2747 w2759 w2768 w2773 w2785 w2790 w2800 w2806 w2812 w2817 w2822 w2827 w2837 w2861 w2882 w2887 w2898 w2923 w2950 w2973 w2978 w2993 w3044 w3090 w3135 w3146 w3164 w3184 w3198 w3211 w3219 w3236 w3258 w3282 w3301 w3319 w3337 w3355 w3369 w3383 w3402 w3416 w3431 w3446 w3455 w3460]
      tunnel: w207 -> [_ _ _ _ _ _ _ _ _ _ _ _ _ _ _ _ _ _ _ _ _ _ _ _ _ _ _ _ _ _ _ _ _ _ _ _ _ _ _ _ _ _ _ _ _ _ _ _ _ _ _ _ _ _ _ _ w1795 _ _ _ _ _ _ _ _ _ _ _ _ _ _ _ _ _ _ _ _ _ _ _ _ _ _ _ _ _ _ _ _ _ _ _ _ _ _ _ _ w2303 _ _ _ _ _ _ _ _ _ _ _ w2421 w2432 _ _ _ _ w2552 _ _ _ _ _ w2663 _ _ _ _ _ _ w2732 _ _ _ _ _ _ w2796 _ _ _ _ _ _ _ _ _ _ _ _ _ _ _ _ _ _ _ _ _ _ _ _ _ _ _ _ _ _ _ _ _ _ _ _ _ _ _]
      tunnel: w203 -> [w216 w623 w631 w638 w644 w666 w679 _ w726 w753 w772 w844 w853 w890 w912 w943 w963 w992 w1006 w1055 w1123 w1158 w1178 w1185 w1192 w1215 w1227 w1251 w1255 w1259 w1280 w1310 w1338 w1380 w1386 w1392 w1400 w1424 w1449 w1473 w1493 w1506 w1550 w1579 w1583 w1610 w1630 w1635 w1639 w1668 w1695 w1710 w1738 w1766 w1771 w1778 w1793 w1811 w1836 w1847 w1865 w1882 w1907 w1926 w1939 w1947 w1966 w1978 w1990 w2009 w2025 w2038 w2051 w2063 w2067 w2072 w2079 w2091 w2100 w2106 w2113 w2123 w2131 w2148 w2176 w2182 w2211 w2222 w2244 w2248 w2252 w2260 w2269 w2278 w2284 w2292 w2299 w2309 w2337 w2345 w2352 w2360 w2365 w2370 w2381 w2386 w2392 w2411 w2416 w2424 w2434 w2505 w2510 w2523 w2544 w2553 w2568 w2592 w2603 w2613 w2637 w2664 w2670 w2682 w2707 w2716 w2722 w2727 w2734 w2741 w2755 w2765 w2770 w2782 w2787 w2793 w2803 w2809 w2814 w2819 w2824 w2834 w2859 w2880 w2884 w2896 w2921 w2948 w2971 w2975 w2986 w3038 w3086 w3132 w3142 w3159 w3179 w3193 w3207 w3213 w3231 w3253 w3277 w3296 w3314 w3332 w3350 w3364 w3378 w3397 w3411 w3426 w3443 w3453 w3457]
      tunnel: [w209 w624 w633 w639 w645 w667 w680 w722 w728 w749 w768 w821 w849 w891 w900 w932 w956 w983 w1007 w1031 w1120 w1157 w1179 w1186 w1196 w1219 errorcluster {"status"=FALSE, "code"=0, "source"=""} ("error out") w1250 w1256 w1269 w1288 w1302 w1325 w1382 w1387 w1393 w1401 w1425 w1450 w1474 w1494 w1497 w1542 w1573 w1587 w1611 w1621 w1636 w1642 w1666 w1694 w1709 w1725 w1760 w1772 w1783 w1787 w1802 w1831 w1843 w1861 w1881 w1898 w1927 w1931 w1949 w1964 w1976 w1988 w2011 w2026 w2039 w2043 w2060 w2068 w2076 w2084 w2088 w2097 w2107 w2110 w2119 w2134 w2156 w2175 w2186 w2204 w2226 w2242 w2249 w2257 w2265 w2270 w2277 w2285 w2293 w2300 w2310 w2338 w2346 w2353 w2361 w2366 w2374 w2380 w2387 w2395 w2412 w2417 w2422 w2435 w2506 w2514 w2526 w2536 w2549 w2569 w2593 w2602 w2615 w2639 w2665 w2671 w2679 w2701 w2717 w2723 w2728 w2735 w2745 w2757 w2766 w2771 w2783 w2788 w2798 w2804 w2810 w2815 w2820 w2825 w2835 w2849 w2873 w2885 w2889 w2908 w2940 w2965 w2976 w2980 w3039 w3087 w3133 w3141 w3161 w3181 w3195 w3209 w3215 w3233 w3255 w3279 w3298 w3316 w3334 w3352 w3366 w3380 w3399 w3413 w3427 w3444 w3451 w3458] -> w188
      tunnel: w189 -> [w215 w624 w633 w639 w645 w667 w680 w722 w728 w750 w766 w821 w848 w891 w901 w939 w956 w973 w1007 w1031 w1121 w1160 w1180 w1186 w1195 w1219 w1223 w1250 w1256 w1269 w1288 w1301 w1337 w1382 w1387 w1393 w1405 w1429 w1454 w1478 w1494 w1504 w1545 w1572 w1586 w1611 w1623 w1636 w1641 w1667 w1685 w1715 w1736 w1759 w1772 w1780 w1790 w1801 w1830 w1846 w1860 w1880 w1897 w1927 w1937 w1950 w1963 w1975 w1987 w2010 w2027 w2039 w2042 w2055 w2068 w2076 w2084 w2087 w2096 w2107 w2111 w2120 w2139 w2155 w2174 w2185 w2210 w2225 w2241 w2249 w2257 w2265 w2270 w2277 w2285 w2293 w2300 w2310 w2338 w2346 w2353 w2361 w2366 w2374 w2380 w2387 w2395 w2412 w2417 w2423 w2436 w2506 w2515 w2525 w2532 w2548 w2570 w2593 w2602 w2610 w2642 w2665 w2671 w2684 w2700 w2717 w2723 w2728 w2735 w2745 w2757 w2766 w2771 w2783 w2788 w2798 w2804 w2810 w2815 w2820 w2825 w2835 w2848 w2872 w2885 w2888 w2907 w2930 w2956 w2976 _ w3040 w3087 w3133 w3140 w3160 w3180 w3194 w3209 w3214 w3232 w3254 w3278 w3297 w3315 w3333 w3351 w3365 w3379 w3398 w3412 w3425 w3444 w3450 w3458]
      tunnel: [w217 w625 w634 w640 w646 w668 w681 w723 w729 w756 w775 w846 w861 w892 w919 w951 w965 w994 w1008 w1093 w1130 w1169 w1182 w1187 w1193 w1221 w1229 w1252 w1257 w1270 w1289 w1317 w1345 w1383 w1388 w1394 w1418 w1442 w1466 w1490 w1495 w1512 w1559 w1581 w1597 w1612 w1632 w1637 w1649 w1678 w1704 w1716 w1754 w1767 w1773 w1784 w1796 w1827 w1840 w1854 w1869 w1888 w1923 w1928 w1942 w1952 w1968 w1980 w1992 w2020 w2035 w2040 w2052 w2064 w2069 w2077 w2085 w2094 w2103 w2108 w2116 w2125 w2143 w2160 w2180 w2191 w2213 w2228 w2245 w2250 w2258 w2266 w2271 w2279 w2286 w2294 w2301 w2311 w2339 w2347 w2354 w2362 w2367 w2375 w2382 w2388 w2397 w2413 w2418 w2425 w2437 w2507 w2519 w2528 w2545 w2554 w2577 w2594 w2605 w2618 w2643 w2666 w2672 w2688 w2710 w2718 w2724 w2729 w2736 w2746 w2758 w2767 w2772 w2784 w2789 w2799 w2805 w2811 w2816 w2821 w2826 w2836 w2860 w2881 w2886 w2897 w2922 w2949 w2972 w2977 w2992 w3043 w3089 w3134 w3145 w3163 w3183 w3197 w3210 w3218 w3235 w3257 w3281 w3300 w3318 w3336 w3354 w3368 w3382 w3401 w3415 w3430 w3445 w3454 w3459] -> w205
      tunnel: [_ _ _ _ _ _ _ _ _ _ _ _ _ _ _ _ _ _ _ _ _ _ _ _ _ _ _ TRUE _ _ _ _ _ _ _ _ _ _ _ _ _ _ _ _ _ _ _ _ _ _ _ _ _ _ _ _ _ _ _ _ _ _ _ _ _ _ _ _ _ _ _ _ _ _ _ _ _ _ _ _ _ _ _ _ _ _ _ _ _ _ _ _ _ _ _ _ _ _ _ _ _ _ _ _ _ _ _ _ _ _ _ _ _ _ _ _ _ _ _ _ _ _ _ _ _ _ _ _ _ _ _ _ _ _ _ _ _ _ _ _ _ _ _ _ _ _ _ _ _ _ _ _ _ _ _ _ _ _ _ _ _ _ _ _ _ _ _ _ _ _ _ _ _ _ _] -> w196
      tunnel: [w214 w623 w631 w638 w644 w666 w679 w697 w726 w753 w772 w844 w853 w890 w912 w943 w963 w992 w1006 w1055 w1124 w1159 w1178 w1185 w1192 w1220 w1227 w1251 w1255 w1260 w1281 w1311 w1339 w1381 w1386 w1392 w1400 w1424 w1449 w1473 w1493 w1506 w1551 w1579 w1584 w1610 w1631 w1635 w1640 w1668 w1695 w1714 w1738 w1766 w1771 w1781 w1793 w1811 w1836 w1847 w1865 w1882 w1907 w1926 w1940 w1947 w1966 w1978 w1990 w2009 w2025 w2038 w2051 w2063 w2067 w2073 w2080 w2092 w2101 w2106 w2114 w2124 w2132 w2154 w2163 w2187 w2212 w2223 w2244 w2248 w2253 w2261 w2269 w2278 w2284 w2292 w2299 w2309 w2337 w2345 w2352 w2360 w2365 w2370 w2381 w2386 w2392 w2411 w2416 w2424 w2434 w2505 w2511 w2524 w2544 w2553 w2568 w2592 w2603 w2614 w2638 w2664 w2670 w2683 w2707 w2716 w2722 w2727 w2734 w2742 w2755 w2765 w2770 w2782 w2787 w2793 w2803 w2809 w2814 w2819 w2824 w2834 w2859 w2880 w2884 w2896 w2921 w2948 w2971 w2975 w2991 w3037 w3086 w3132 w3142 w3159 w3179 w3193 w3207 w3213 w3231 w3253 w3277 w3296 w3314 w3332 w3350 w3364 w3378 w3397 w3411 w3428 w3443 w3453 w3457] -> w204
      tunnel: 30 ("Timeout") -> [w213 _ _ _ _ _ _ _ _ _ _ _ _ _ _ _ _ _ _ _ _ _ _ _ _ _ _ _ _ _ _ _ _ _ _ _ _ _ _ _ _ _ _ _ _ _ _ _ _ _ _ _ _ _ _ _ _ _ _ _ _ _ _ _ _ _ _ _ _ _ _ _ _ _ _ _ _ _ _ _ _ _ _ _ _ _ _ _ _ _ _ _ _ _ _ _ _ _ _ _ _ _ _ _ _ _ _ _ _ _ _ _ _ _ _ _ _ _ _ _ _ _ _ _ _ _ _ _ _ _ _ _ _ _ _ _ _ _ _ _ _ _ _ _ _ _ _ _ _ _ _ _ _ _ _ _ _ _ _ _ _ _ _ _ _ _ _ _ _ _ _ _ _ _ _]
      tunnel: w201 -> [_ _ _ _ _ _ _ _ _ _ _ _ _ _ _ _ _ _ _ _ w1128 _ _ _ _ _ _ _ _ _ _ _ _ _ _ _ _ _ _ _ _ _ _ _ _ _ _ _ _ _ _ _ _ _ _ _ _ _ _ _ _ _ _ _ _ _ _ _ _ _ _ _ w2048 w2059 _ _ _ _ _ _ _ _ _ _ _ _ _ _ _ _ _ _ _ _ _ _ _ _ _ _ _ _ _ _ _ _ _ _ _ _ _ _ _ _ _ _ _ _ _ _ _ _ _ _ _ _ _ _ _ _ _ _ _ _ _ _ _ _ _ _ _ _ _ _ _ _ _ _ _ _ _ _ _ _ _ _ _ _ _ _ _ _ _ _ _ _ _ _ _ _ _ _ _ _ _]
      tunnel: w200 -> [_ _ _ _ _ _ _ _ _ _ _ _ _ _ _ _ _ _ _ _ w1127 _ _ _ _ _ _ _ _ _ _ _ _ _ _ _ _ _ _ _ _ _ _ _ _ _ _ _ _ _ _ _ _ _ _ _ _ _ _ _ _ _ _ _ _ _ _ _ _ _ _ _ w2049 w2058 _ _ _ _ _ _ _ _ _ _ _ _ _ _ _ _ _ _ _ _ _ _ _ _ _ _ _ _ _ _ _ _ _ _ _ _ _ _ _ _ _ _ _ _ _ _ _ _ _ _ _ _ _ _ _ _ _ _ _ _ _ _ _ _ _ _ _ _ _ _ _ _ _ _ _ _ _ _ _ _ _ _ _ _ _ _ _ _ _ _ _ _ _ _ _ _ _ _ _ _ _]
      tunnel: w199 -> [w212 _ _ _ _ _ _ _ _ _ _ _ _ _ _ _ _ _ _ _ _ _ _ _ _ _ _ _ _ _ _ _ _ _ _ _ _ _ _ _ _ _ _ w1575 _ _ _ _ _ _ _ _ _ _ _ _ _ _ _ _ _ _ _ _ _ _ _ _ _ _ _ _ _ _ _ _ _ _ _ _ _ _ _ _ _ _ _ _ _ _ _ _ _ _ _ _ _ _ _ _ _ _ _ _ _ _ _ _ _ _ _ _ _ _ _ _ _ _ _ _ _ _ _ _ _ _ _ _ _ _ _ _ _ _ _ _ _ _ _ _ _ _ _ _ _ _ _ _ _ _ _ _ _ _ _ _ _ _ _ _ _ _ _ _ _ _ _ _ _ _ _ _ _ _ _]
      tunnel: w198 -> [w211 w622 w632 w637 w643 w658 w678 w707 w727 w755 w774 w845 w860 w889 w918 w950 w964 w993 w1005 w1092 w1129 w1168 w1177 w1184 w1189 w1207 w1226 w1249 w1254 w1268 w1287 w1316 w1336 w1379 w1385 w1391 w1399 w1423 w1448 w1472 w1492 w1501 w1525 w1580 w1596 w1609 w1618 w1634 w1648 w1677 w1703 w1708 w1753 w1758 w1770 w1777 w1786 w1798 w1829 w1845 w1859 w1879 w1894 w1925 w1941 w1951 w1967 w1979 w1991 w2019 w2022 w2037 w2050 w2057 w2066 w2075 w2083 w2090 w2099 w2105 w2115 w2118 w2130 w2149 w2164 w2183 w2209 w2227 w2243 w2247 w2255 w2263 w2268 w2276 w2283 w2291 w2298 w2308 w2336 w2344 w2351 w2356 w2364 w2373 w2379 w2385 w2394 w2406 w2415 w2420 w2431 w2504 w2509 w2521 w2531 w2547 w2576 w2591 w2604 w2616 w2640 w2660 w2668 w2681 w2709 w2714 w2720 w2726 w2733 w2744 w2756 w2764 w2769 w2781 w2786 w2797 w2802 w2808 w2813 w2818 w2823 w2833 w2858 w2879 w2883 w2895 w2920 w2947 w2970 w2974 w2990 w3042 w3088 w3129 w3144 w3162 w3182 w3196 w3208 w3217 w3234 w3256 w3280 w3299 w3317 w3335 w3353 w3367 w3381 w3400 w3414 w3429 w3442 w3452 w3456]
      tunnel: [w210 w622 w632 w637 w643 w658 w678 w707 w727 w755 w774 w845 w860 w889 w918 w950 w964 w993 w1005 w1092 w1129 w1168 w1177 w1184 w1189 w1207 w1226 w1249 w1254 w1268 w1287 w1316 w1336 w1379 w1385 w1391 w1399 w1423 w1448 w1472 w1492 w1501 w1525 w1580 w1596 w1609 w1618 w1634 w1648 w1677 w1703 w1708 w1753 w1758 w1770 w1777 w1786 w1798 w1829 w1845 w1859 w1879 w1894 w1925 w1941 w1951 w1967 w1979 w1991 w2019 w2022 w2037 w2050 w2057 w2066 w2075 w2083 w2090 w2099 w2105 w2115 w2118 w2130 w2149 w2164 w2183 w2209 w2227 w2243 w2247 w2255 w2263 w2268 w2276 w2283 w2291 w2298 w2308 w2336 w2344 w2351 w2356 w2364 w2373 w2379 w2385 w2394 w2406 w2415 w2420 w2431 w2504 w2509 w2521 w2531 w2547 w2576 w2591 w2604 w2616 w2640 w2660 w2668 w2681 w2709 w2714 w2720 w2726 w2733 w2744 w2756 w2764 w2769 w2781 w2786 w2797 w2802 w2808 w2813 w2818 w2823 w2833 w2858 w2879 w2883 w2895 w2920 w2947 w2970 w2974 w2990 w3042 w3088 w3129 w3144 w3162 w3182 w3196 w3208 w3217 w3234 w3256 w3280 w3299 w3317 w3335 w3353 w3367 w3381 w3400 w3414 w3429 w3442 w3452 w3456] -> w197
      tunnel: w193 -> [_ _ _ _ _ _ _ _ _ _ _ _ _ _ _ _ _ _ _ _ w1122 _ _ _ _ _ _ _ _ _ _ _ _ _ _ _ _ _ _ _ _ _ _ _ _ _ _ _ _ _ _ _ _ _ _ _ _ _ _ _ _ _ _ _ _ _ _ _ _ _ _ _ w2047 w2056 _ _ _ _ _ _ _ _ _ _ _ _ _ _ _ _ _ _ _ _ _ _ _ _ _ _ _ _ _ _ _ _ _ _ _ _ _ _ _ _ _ _ _ _ _ _ _ _ _ _ _ _ _ _ _ _ _ _ _ _ _ _ _ _ _ _ _ _ _ _ _ _ _ _ _ _ _ _ _ _ _ _ _ _ _ _ _ _ _ _ _ _ _ _ _ _ _ _ _ _ _]
      frame "", "Event Structure", "Idle" {
        # "executes when the state queue is empty"
        n85 = event shown="[36] <AcqLoop error?>: User Event" {
          selector: w211 -> [_ _ _ _ _ _ _ _ _ _ _ _ _ _ _ _ _ _ _ _ _ _ _ _ _ _ _ _ _ _ _ _ _ _ _ _ _ _]
          dyn-events: [_ _ _ _ _ _ _ _ _ _ _ _ _ _ _ _ _ _ _ _ _ _ _ _ _ _ _ _ _ _ _ _ _ _ _ _ _ _] -> w210
          timeout: w213 -> [_ _ _ _ _ _ _ _ _ _ _ _ _ _ _ _ _ _ _ _ _ _ _ _ _ _ _ _ _ _ _ _ _ _ _ _ _ _]
          tunnel: w218 -> [w238 w257 w265 w269 w273 w281 w287 w295 w303 w313 w320 w349 w369 w389 w409 w413 w420 w443 w457 w471 w485 w490 w493 w499 w506 w513 w519 w525 w531 w538 w551 w562 w574 w581 w585 w589 w605 w621]
          tunnel: [w239 w257 w264 w269 w272 w281 w287 w295 w303 w313 w319 w349 w369 w389 w409 w413 w419 w443 w457 w471 w485 w489 w492 w499 w507 w514 w518 w524 w531 w539 w552 w562 w575 w581 w585 w588 w606 w620] -> w217
          tunnel: w216 -> [w222 w255 w259 w267 w274 w280 w288 w296 w304 w311 w315 w347 w367 w387 w407 w411 w415 w442 w456 w470 w484 w486 w494 w497 w502 w509 w521 w526 w529 w533 w546 w560 w570 w579 w583 w590 w603 w618]
          tunnel: [w237 w256 w260 w268 w275 w279 w286 w294 w302 w312 w321 w348 w368 w388 w408 w412 w421 w440 w444 w467 w482 w488 w495 w498 w503 w510 w522 w527 w530 w537 w550 w561 w571 w580 w584 w591 w607 w619] -> w209
          tunnel: w215 -> [w237 w256 w260 w268 w275 w279 w286 w294 w302 w312 w321 w348 w368 w388 w408 w412 w421 w437 w446 w458 w474 w488 w495 w498 w503 w510 w522 w527 w530 w537 w550 w561 w573 w580 w584 w591 w607 w619]
          tunnel: [w222 w255 w259 w267 w274 w280 w288 w296 w304 w311 w316 w347 w367 w387 w407 w411 w416 w442 w456 w470 w484 w486 w494 w497 w504 w511 w521 w526 w529 w534 w547 w560 w576 w579 w583 w590 w604 w618] -> w214
          tunnel: w212 -> [_ _ _ _ _ _ _ _ _ _ _ _ _ _ _ _ _ _ _ _ _ _ _ _ _ _ _ _ _ _ _ _ _ _ _ _ _ _]
          event Timeout {
            # "check system status every 2s"
            n86 = event-data() -> ()  [unwired: 1 in, 1 out]
            n87 = Unbundle By Name(w222) -> ("SysRunning?"=w220:bool, "SlowTimer"=w236:u32, "FastTimer"=w230:u32)
            n88 = Tick Count (ms)() -> (millisecond timer value=w223:u32)
            n89 = Subtract(x=w223, y=w236) -> (x-y=w233:u32)
            n90 = case shown="False" w220 {
              tunnel: ["" "Utility: AquiTimerCheck" ("State(s) in Front (\"\")")] -> w228
              frame False {
                # "if not running, do nothing"
              }
              frame True {
                # "if aquisition is running, check timer"
              }
            }
            n91 = Subtract(x=w223, y=w230) -> (x-y=w231:u32)
            n92 = Greater?(x=w233, y=u32 2000) -> (0:w234:bool)
            n93 = Greater?(x=w231, y=u32 500) -> (0:w221:bool)
            n94 = disable-structure shown="Enabled" {
              disable-tunnel: w221 -> [w244 _]
              disable-tunnel: w220 -> [w243 _]
              disable-tunnel: [w240 "" ("State(s) at Back (\"\")")] -> w219
              frame Disabled {
                n95 = Not(x=w243) -> (.not. x?=w242:bool)
                n96 = And(x=w244, y=w242) -> (x .and. y?=w241:bool)
                n97 = case shown="True" w241 {
                  tunnel: ["" ("Empty String Constant") "TCP: checkSource" ("State(s) in Front (\"\")")] -> w240
                  frame False {
                  }
                  frame True {
                  }
                }
              }
              frame Enabled {
              }
            }
            n98 = case shown="True" w234 {
              tunnel: ["" ("Empty String Constant") "SystemStatus: SlowSysStatusMacro" ("State(s) in Front (\"\")")] -> w226
              frame False {
              }
              frame True {
              }
            }
            n99 = case shown="True" w221 {
              tunnel: ["" ("Empty String Constant") "SystemStatus: FastSysStatusMacro" ("State(s) in Front (\"\")")] -> w224
              frame False {
              }
              frame True {
              }
            }
            n100 = call <vilib>:"Add State(s) to Queue__JKI_lib_State_Machine.vi"("State(s) in Front (\"\")"=w228, "State(s) in (\"\")"="LabJack: checkPedal" ("State(s) in Front (\"\")"), "State(s) at Back (\"\")"=w226) -> ("States Out"=w225:string)  [unwired: 12 in]
            n101 = call <vilib>:"Add State(s) to Queue__JKI_lib_State_Machine.vi"("State(s) in Front (\"\")"=w225, "State(s) in (\"\")"=w224, "State(s) at Back (\"\")"=w219) -> ("States Out"=w229:string)  [unwired: 12 in]
            n102 = call <vilib>:"Add State(s) to Queue__JKI_lib_State_Machine.vi"("State(s) in Front (\"\")"=w229, "State(s) in (\"\")"=w238) -> ("States Out"=w239:string)  [unwired: 13 in]
          }
          event "355nm Laser toggle": Mouse Enter {
            n103 = event-data() -> ()  [unwired: 1 in, 4 out]
            n104 = local write "Help"("Toggle 355nm laser." ("Help")) -> ()
          }
          event "355nm Laser toggle": Value Change {
            # "[Covers: REQ34]"
            n105 = event-data() -> ()  [unwired: 1 in, 6 out]
            n106 = Select(t="LabJack: 355_PWM_Start\nLabJack: AB_Start", s="355nm Laser toggle", f="LabJack: 355_PWM_Stop\nLabJack: AB_Stop") -> (s? t:f=w262:string)
            n107 = call <vilib>:"Add State(s) to Queue__JKI_lib_State_Machine.vi"("State(s) in Front (\"\")"=w262, "State(s) in (\"\")"=w265) -> ("States Out"=w264:string)  [unwired: 13 in]
          }
          event "Aiming beam toggle": Mouse Enter {
            n108 = event-data() -> ()  [unwired: 1 in, 4 out]
            n109 = local write "Help"("Toggle aiming beam laser." ("Help")) -> ()
          }
          event "Aiming beam toggle": Value Change {
            # "[Covers: REQ33]"
            n110 = event-data() -> ()  [unwired: 1 in, 6 out]
            n111 = case shown="True" "Aiming beam toggle" {
              tunnel: ["LabJack: AB_Stop" ("State(s) in Front (\"\")") "LabJack: AB_Start" ("State(s) in Front (\"\")")] -> w271
              frame False {
              }
              frame True {
              }
            }
            n112 = call <vilib>:"Add State(s) to Queue__JKI_lib_State_Machine.vi"("State(s) in Front (\"\")"=w271, "State(s) in (\"\")"=w273) -> ("States Out"=w272:string)  [unwired: 13 in]
          }
          event "Auto gain ch1": Value Change {
            n113 = event-data() -> ("NewVal"=w278:bool)  [unwired: 1 in, 5 out]
            n114 = case shown="True" w278 {
              frame False {
                n115 = local read "V 1"() -> (w282:dbl)
                n116 = call "V1FGV.vi"("action (write)"=enum16{"write", "read"}."write" ("action"), "V1 in"=w282) -> ()  [unwired: 8 in, 2 out]
                n117 = property on="V 1" class="DigNum (strict)"("DisabledEnum"=T11."Enabled" ("Disabled")) -> ()  [unwired: 2 in, 2 out]
              }
              frame True {
                n118 = property on="V 1" class="DigNum (strict)"("DisabledEnum"=T11."Disabled and Grayed Out" ("Disabled")) -> ()  [unwired: 2 in, 2 out]
              }
            }
          }
          event "Auto gain ch2": Value Change {
            n119 = event-data() -> ("NewVal"=w289:bool)  [unwired: 1 in, 5 out]
            n120 = case shown="False" w289 {
              frame False {
                n121 = local read "V 2"() -> (w290:dbl)
                n122 = property on="V 2" class="DigNum (strict)"("DisabledEnum"=T11."Enabled" ("Disabled")) -> ()  [unwired: 2 in, 2 out]
                n123 = call "V2FGV.vi"("action(write)"=enum16{"write", "read"}."write" ("action"), "V2 in"=w290) -> ()  [unwired: 8 in, 2 out]
              }
              frame True {
                n124 = property on="V 2" class="DigNum (strict)"("DisabledEnum"=T11."Disabled and Grayed Out" ("Disabled")) -> ()  [unwired: 2 in, 2 out]
              }
            }
          }
          event "Auto gain ch3": Value Change {
            n125 = event-data() -> ("NewVal"=w297:bool)  [unwired: 1 in, 5 out]
            n126 = case shown="False" w297 {
              frame False {
                n127 = local read "V 3"() -> (w298:dbl)
                n128 = property on="V 3" class="DigNum (strict)"("DisabledEnum"=T11."Enabled" ("Disabled")) -> ()  [unwired: 2 in, 2 out]
                n129 = call "V3FGV.vi"("action(write)"=enum16{"write", "read"}."write" ("action"), "V3 in"=w298) -> ()  [unwired: 8 in, 2 out]
              }
              frame True {
                n130 = property on="V 3" class="DigNum (strict)"("DisabledEnum"=T11."Disabled and Grayed Out" ("Disabled")) -> ()  [unwired: 2 in, 2 out]
              }
            }
          }
          event "Auto gain ch4": Value Change {
            n131 = event-data() -> ("NewVal"=w305:bool)  [unwired: 1 in, 5 out]
            n132 = case shown="False" w305 {
              frame False {
                n133 = local read "V 4"() -> (w306:dbl)
                n134 = property on="V 4" class="DigNum (strict)"("DisabledEnum"=T11."Enabled" ("Disabled")) -> ()  [unwired: 2 in, 2 out]
                n135 = call "V4FGV.vi"("action(write)"=enum16{"write", "read"}."write" ("action"), "V3 in"=w306) -> ()  [unwired: 8 in, 2 out]
              }
              frame True {
                n136 = property on="V 4" class="DigNum (strict)"("DisabledEnum"=T11."Disabled and Grayed Out" ("Disabled")) -> ()  [unwired: 2 in, 2 out]
              }
            }
          }
          event "Background": Mouse Enter {
            n137 = event-data() -> ()  [unwired: 1 in, 4 out]
            n138 = local write "Help"("Click to record a background." ("Help")) -> ()
          }
          event "Background": Value Change {
            n139 = event-data() -> ("NewVal"=w317:bool)  [unwired: 1 in, 5 out]
            n140 = case shown="True" w317 {
              tunnel: ["Utility: SetAllChanManualGain\nQueue: Flash\nUtility: Dewelling >> 2500\nLabJack: 355_PWM_Stop\nLabJack: AB_Stop" "Utility: SetDataClass >> Bg\nUI: Update\nLabJack: 355_PWM_Start\nLabJack: AB_Start\nUtility: SaveDeconChan\nUtility: Dewelling >> 50\nLabJack: SetV\nDigitizer: Start\nUtility: AquiTimerReset\nLED: BreathGreen\nUI: duringBGAcquire"] -> w318
              tunnel: [FALSE TRUE] -> w314
              frame False {
                n141 = local read "Skip Data Save?"() -> (w322:bool)
                n142 = case shown="False" w322 {
                  frame False {
                    n143 = property on="Background" class="Bool (strict)"("BoolText.Text"="Done!" ("Boolean Text.Text")) -> ()  [unwired: 2 in, 2 out]
                  }
                  frame True {
                  }
                }
              }
              frame True {
                # "[Covers: REQ6]"
                n144 = property on="Background" class="Bool (strict)"("BoolText.Text"="Running" ("Boolean Text.Text"), "Colors [4]"=cluster{u32, u32}[] [{6618880, 6618880}, {16711680, 16711680}]) -> ()  [unwired: 2 in, 2 out]
              }
            }
            n145 = Bundle By Name(cluster=w315, "SysRunning?"=w314) -> (w316:T26)
            n146 = call <vilib>:"Add State(s) to Queue__JKI_lib_State_Machine.vi"("State(s) in Front (\"\")"=w318, "State(s) in (\"\")"=w320) -> ("States Out"=w319:string)  [unwired: 13 in]
          }
          event "Channel 1": Cursor Move {
            n147 = event-data() -> ("CursIdx"=w333:i32, "CursLoc"=w345:cluster{"X":dbl, "Y":dbl})  [unwired: 1 in, 7 out]
            n148 = property on="Channel 3" class="WFGraph (strict)"() -> ("CrsrList"=w340:T27)  [unwired: 2 in, 2 out]
            n149 = property on="Channel 4" class="WFGraph (strict)"() -> ("CrsrList"=w332:T27)  [unwired: 2 in, 2 out]
            n150 = property on="Channel 2" class="WFGraph (strict)"() -> ("CrsrList"=w343:T27)  [unwired: 2 in, 2 out]
            n151 = Index Array(array=w340, index=w333) -> (element=w344:T28)
            n152 = Index Array(array=w332, index=w333) -> (element=w335:T28)
            n153 = Unbundle By Name(w345) -> ("X"=w334:dbl)
            n154 = Index Array(array=w343, index=w333) -> (element=w346:T28)
            n155 = Bundle By Name(cluster=w344, "Position.X"=w334) -> (w339:T28)
            n156 = Bundle By Name(cluster=w335, "Position.X"=w334) -> (w331:T28)
            n157 = Bundle By Name(cluster=w346, "Position.X"=w334) -> (w342:T28)
            n158 = control-ref of="Channel 1"() -> (w336:refnum<vi>)
            n159 = Replace Array Subset(array=w340, new element=w339, index=w333) -> (w338:T27)
            n160 = Replace Array Subset(array=w332, new element=w331, index=w333) -> (w330:T27)
            n161 = Replace Array Subset(array=w343, new element=w342, index=w333) -> (w341:T27)
            n162 = property on="Channel 3" class="WFGraph (strict)"("CrsrList"=w338) -> (error out=w337:errorcluster)  [unwired: 2 in, 1 out]
            n163 = property on="Channel 4" class="WFGraph (strict)"("CrsrList"=w330) -> ()  [unwired: 2 in, 2 out]
            n164 = property on="Channel 2" class="WFGraph (strict)"("CrsrList"=w341) -> ()  [unwired: 2 in, 2 out]
            n165 = call "UpdateCurserIdx(SubVI).vi"("error in (no error)"=w337, "WaveformGraph in"=w336) -> ()  [unwired: 9 in, 1 out]
          }
          event "Channel 2": Cursor Move {
            n166 = event-data() -> ("CursIdx"=w352:i32, "CursLoc"=w366:cluster{"X":dbl, "Y":dbl})  [unwired: 1 in, 7 out]
            n167 = Unbundle By Name(w366) -> ("X"=w354:dbl)
            n168 = property on="Channel 1" class="WFGraph (strict)"() -> ("CrsrList"=w360:T27)  [unwired: 2 in, 2 out]
            n169 = property on="Channel 3" class="WFGraph (strict)"() -> ("CrsrList"=w362:T27)  [unwired: 2 in, 2 out]
            n170 = property on="Channel 4" class="WFGraph (strict)"() -> ("CrsrList"=w353:T27)  [unwired: 2 in, 2 out]
            n171 = Index Array(array=w360, index=w352) -> (element=w365:T28)
            n172 = Index Array(array=w362, index=w352) -> (element=w364:T28)
            n173 = Index Array(array=w353, index=w352) -> (element=w355:T28)
            n174 = Bundle By Name(cluster=w355, "Position.X"=w354) -> (w351:T28)
            n175 = Bundle By Name(cluster=w365, "Position.X"=w354) -> (w363:T28)
            n176 = Bundle By Name(cluster=w364, "Position.X"=w354) -> (w361:T28)
            n177 = Replace Array Subset(array=w360, new element=w363, index=w352) -> (w359:T27)
            n178 = Replace Array Subset(array=w362, new element=w361, index=w352) -> (w358:T27)
            n179 = Replace Array Subset(array=w353, new element=w351, index=w352) -> (w350:T27)
            n180 = control-ref of="Channel 1"() -> (w357:refnum<vi>)
            n181 = property on="Channel 1" class="WFGraph (strict)"("CrsrList"=w359) -> ()  [unwired: 2 in, 2 out]
            n182 = property on="Channel 3" class="WFGraph (strict)"("CrsrList"=w358) -> (error out=w356:errorcluster)  [unwired: 2 in, 1 out]
            n183 = property on="Channel 4" class="WFGraph (strict)"("CrsrList"=w350) -> ()  [unwired: 2 in, 2 out]
            n184 = call "UpdateCurserIdx(SubVI).vi"("error in (no error)"=w356, "WaveformGraph in"=w357) -> ()  [unwired: 9 in, 1 out]
          }
          event "Channel 3": Cursor Move {
            n185 = event-data() -> ("CursIdx"=w372:i32, "CursLoc"=w386:cluster{"X":dbl, "Y":dbl})  [unwired: 1 in, 7 out]
            n186 = Unbundle By Name(w386) -> ("X"=w374:dbl)
            n187 = property on="Channel 4" class="WFGraph (strict)"() -> ("CrsrList"=w373:T27)  [unwired: 2 in, 2 out]
            n188 = property on="Channel 1" class="WFGraph (strict)"() -> ("CrsrList"=w383:T27)  [unwired: 2 in, 2 out]
            n189 = property on="Channel 2" class="WFGraph (strict)"() -> ("CrsrList"=w381:T27)  [unwired: 2 in, 2 out]
            n190 = Index Array(array=w373, index=w372) -> (element=w375:T28)
            n191 = Index Array(array=w383, index=w372) -> (element=w385:T28)
            n192 = Index Array(array=w381, index=w372) -> (element=w384:T28)
            n193 = Bundle By Name(cluster=w375, "Position.X"=w374) -> (w371:T28)
            n194 = Bundle By Name(cluster=w385, "Position.X"=w374) -> (w382:T28)
            n195 = Bundle By Name(cluster=w384, "Position.X"=w374) -> (w380:T28)
            n196 = Replace Array Subset(array=w373, new element=w371, index=w372) -> (w370:T27)
            n197 = Replace Array Subset(array=w383, new element=w382, index=w372) -> (w379:T27)
            n198 = Replace Array Subset(array=w381, new element=w380, index=w372) -> (w378:T27)
            n199 = control-ref of="Channel 1"() -> (w376:refnum<vi>)
            n200 = property on="Channel 4" class="WFGraph (strict)"("CrsrList"=w370) -> ()  [unwired: 2 in, 2 out]
            n201 = property on="Channel 1" class="WFGraph (strict)"("CrsrList"=w379) -> ()  [unwired: 2 in, 2 out]
            n202 = property on="Channel 2" class="WFGraph (strict)"("CrsrList"=w378) -> (error out=w377:errorcluster)  [unwired: 2 in, 1 out]
            n203 = call "UpdateCurserIdx(SubVI).vi"("error in (no error)"=w377, "WaveformGraph in"=w376) -> ()  [unwired: 9 in, 1 out]
          }
          event "Channel 4": Cursor Move {
            n204 = event-data() -> ("CursIdx"=w394:i32, "CursLoc"=w406:cluster{"X":dbl, "Y":dbl})  [unwired: 1 in, 7 out]
            n205 = Unbundle By Name(w406) -> ("X"=w392:dbl)
            n206 = property on="Channel 1" class="WFGraph (strict)"() -> ("CrsrList"=w404:T27)  [unwired: 2 in, 2 out]
            n207 = property on="Channel 2" class="WFGraph (strict)"() -> ("CrsrList"=w400:T27)  [unwired: 2 in, 2 out]
            n208 = property on="Channel 3" class="WFGraph (strict)"() -> ("CrsrList"=w395:T27)  [unwired: 2 in, 2 out]
            n209 = Index Array(array=w404, index=w394) -> (element=w405:T28)
            n210 = Index Array(array=w400, index=w394) -> (element=w401:T28)
            n211 = Index Array(array=w395, index=w394) -> (element=w397:T28)
            n212 = Bundle By Name(cluster=w405, "Position.X"=w392) -> (w403:T28)
            n213 = Bundle By Name(cluster=w401, "Position.X"=w392) -> (w399:T28)
            n214 = Bundle By Name(cluster=w397, "Position.X"=w392) -> (w396:T28)
            n215 = Replace Array Subset(array=w404, new element=w403, index=w394) -> (w402:T27)
            n216 = Replace Array Subset(array=w400, new element=w399, index=w394) -> (w398:T27)
            n217 = Replace Array Subset(array=w395, new element=w396, index=w394) -> (w393:T27)
            n218 = control-ref of="Channel 1"() -> (w390:refnum<vi>)
            n219 = call "UpdateCurserIdx(SubVI).vi"() -> ()  [unwired: 11 in, 1 out]
            n220 = call "UpdateCurserIdx(SubVI).vi"() -> ()  [unwired: 11 in, 1 out]
            n221 = property on="Channel 1" class="WFGraph (strict)"("CrsrList"=w402) -> ()  [unwired: 2 in, 2 out]
            n222 = property on="Channel 2" class="WFGraph (strict)"("CrsrList"=w398) -> ()  [unwired: 2 in, 2 out]
            n223 = property on="Channel 3" class="WFGraph (strict)"("CrsrList"=w393) -> (error out=w391:errorcluster)  [unwired: 2 in, 1 out]
            n224 = call "UpdateCurserIdx(SubVI).vi"("error in (no error)"=w391, "WaveformGraph in"=w390) -> ()  [unwired: 9 in, 1 out]
          }
          event "Cali&iRF alignment": Mouse Enter {
            n225 = event-data() -> ()  [unwired: 1 in, 4 out]
            n226 = local write "Help"("Click to run system intensity calibration and irf alignment" ("Help")) -> ()
          }
          event "Cali&iRF alignment": Value Change {
            n227 = event-data() -> ("NewVal"=w417:bool)  [unwired: 1 in, 5 out]
            n228 = case shown="False" w417 {
              tunnel: ["Utility: SetAllChanManualGain\nQueue: Flash\nUtility: Dewelling >> 2500\nLabJack: 355_PWM_Stop\nLabJack: AB_Stop" "Utility: SetDataClass >> Cali\nUI: Update\nUtility: SaveDeconChan\nLabJack: 355_PWM_Start\nLabJack: AB_Start\nLabJack: SetV\nDigitizer: Start\nUtility: AquiTimerReset\nLED: BreathGreen\nUI: duringIRFAlign"] -> w418
              tunnel: [FALSE TRUE] -> w414
              frame False {
                n229 = local read "Skip Data Save?"() -> (w422:bool)
                n230 = case shown="False" w422 {
                  frame False {
                    n231 = property on="Cali&iRF alignment" class="Bool (strict)"("BoolText.Text"="Done!" ("Boolean Text.Text")) -> ()  [unwired: 2 in, 2 out]
                  }
                  frame True {
                  }
                }
              }
              frame True {
                n232 = property on="Cali&iRF alignment" class="Bool (strict)"("BoolText.Text"="Running" ("Boolean Text.Text"), "Colors [4]"=cluster{u32, u32}[] [{6618880, 6618880}, {16711680, 16711680}]) -> ()  [unwired: 2 in, 2 out]
              }
            }
            n233 = Bundle By Name(cluster=w415, "SysRunning?"=w414) -> (w416:T26)
            n234 = call <vilib>:"Add State(s) to Queue__JKI_lib_State_Machine.vi"("State(s) in Front (\"\")"=w418, "State(s) in (\"\")"=w420) -> ("States Out"=w419:string)  [unwired: 13 in]
          }
          event "V 1": Value Change {
            n235 = event-data() -> ()  [unwired: 1 in, 6 out]
            n236 = call "LabJack_FGV.vi"("Operation(Read)"=enum16{"Write", "Read"}."Read" ("Operation"), "error in (no error)"=w437) -> ("error out"=w434:errorcluster, "Read data"=w435:i32)  [unwired: 8 in]
            n237 = global read "GlobalVariables.vi" "Ch1 LJ pin"() -> (w433:string)
            n238 = call "LJM_eWriteName.vi"("Handle In"=w435, "Name"=w433, "Value"="V 1", "error in"=w434) -> ("error out"=w431:errorcluster)  [unwired: 10 in, 1 out]
            n239 = call "V1FGV.vi"("Error In"=w431, "action (write)"=enum16{"write", "read"}."write" ("action"), "V1 in"="V 1") -> ("Error Out"=w430:errorcluster)  [unwired: 7 in, 1 out]
            n240 = call "CtrlVtoGain.vi"("error in (no error)"=w430, "CtrlV(V)"="V 1", "Channel"=enum16{"Ch1", "Ch2", "Ch3"}."Ch1" ("Enum")) -> ("error out"=w440:errorcluster, "Gain"=w439:dbl)  [unwired: 7 in]
            n241 = local write "Gain1"(w439) -> ()
          }
          event "V 2": Value Change {
            n242 = event-data() -> ()  [unwired: 1 in, 6 out]
            n243 = call "LabJack_FGV.vi"("Operation(Read)"=enum16{"Write", "Read"}."Read" ("Operation"), "error in (no error)"=w446) -> ("error out"=w451:errorcluster, "Read data"=w452:i32)  [unwired: 8 in]
            n244 = global read "GlobalVariables.vi" "Ch2 LJ pin"() -> (w450:string)
            n245 = call "LJM_eWriteName.vi"("Handle In"=w452, "Name"=w450, "Value"="V 2", "error in"=w451) -> ("error out"=w449:errorcluster)  [unwired: 10 in, 1 out]
            n246 = call "V2FGV.vi"("Error In"=w449, "action(write)"=enum16{"write", "read"}."write" ("action"), "V2 in"="V 2") -> ("Error Out"=w448:errorcluster)  [unwired: 7 in, 1 out]
            n247 = call "CtrlVtoGain.vi"("error in (no error)"=w448, "CtrlV(V)"="V 2", "Channel"=enum16{"Ch1", "Ch2", "Ch3"}."Ch2" ("Enum")) -> ("error out"=w444:errorcluster, "Gain"=w445:dbl)  [unwired: 7 in]
            n248 = local write "Gain2"(w445) -> ()
          }
          event "V 3": Value Change {
            n249 = event-data() -> ()  [unwired: 1 in, 6 out]
            n250 = call "LabJack_FGV.vi"("Operation(Read)"=enum16{"Write", "Read"}."Read" ("Operation"), "error in (no error)"=w458) -> ("error out"=w463:errorcluster, "Read data"=w464:i32)  [unwired: 8 in]
            n251 = global read "GlobalVariables.vi" "Ch3 LJ pin"() -> (w462:string)
            n252 = call "LJM_eWriteName.vi"("Handle In"=w464, "Name"=w462, "Value"="V 3", "error in"=w463) -> ("error out"=w460:errorcluster)  [unwired: 10 in, 1 out]
            n253 = call "V3FGV.vi"("Error In"=w460, "action(write)"=enum16{"write", "read"}."write" ("action"), "V3 in"="V 3") -> ("Error Out"=w459:errorcluster)  [unwired: 7 in, 1 out]
            n254 = call "CtrlVtoGain.vi"("error in (no error)"=w459, "CtrlV(V)"="V 3", "Channel"=enum16{"Ch1", "Ch2", "Ch3"}."Ch3" ("Enum")) -> ("error out"=w467:errorcluster, "Gain"=w466:dbl)  [unwired: 7 in]
            n255 = local write "Gain3"(w466) -> ()
          }
          event "V 4": Value Change {
            n256 = event-data() -> ()  [unwired: 1 in, 6 out]
            n257 = call "LabJack_FGV.vi"("Operation(Read)"=enum16{"Write", "Read"}."Read" ("Operation"), "error in (no error)"=w474) -> ("error out"=w478:errorcluster, "Read data"=w479:i32)  [unwired: 8 in]
            n258 = global read "GlobalVariables.vi" "Ch4 LJ pin"() -> (w477:string)
            n259 = call "LJM_eWriteName.vi"("Handle In"=w479, "Name"=w477, "Value"="V 4", "error in"=w478) -> ("error out"=w476:errorcluster)  [unwired: 10 in, 1 out]
            n260 = call "V4FGV.vi"("Error In"=w476, "action(write)"=enum16{"write", "read"}."write" ("action"), "V3 in"="V 4") -> ("Error Out"=w475:errorcluster)  [unwired: 7 in, 1 out]
            n261 = call "CtrlVtoGain.vi"("error in (no error)"=w475, "CtrlV(V)"="V 4", "Channel"=enum16{"Ch1", "Ch2", "Ch3", "Ch4"}."Ch4") -> ("error out"=w482:errorcluster, "Gain"=w481:dbl)  [unwired: 7 in]
            n262 = local write "Gain4"(w481) -> ()
          }
          event "Quit": Value Change {
            # "Exit Button Value Change (pressed) Event\n(when pressed.  quite)"
            n263 = event-data() -> ()  [unwired: 1 in, 1 out]
            n264 = call <vilib>:"Add State(s) to Queue__JKI_lib_State_Machine.vi"("State(s) in Front (\"\")"="LED: Off\nMacro: Exit", "State(s) in (\"\")"=w490) -> ("States Out"=w489:string)  [unwired: 13 in]
          }
          event "Show BG": Value Change {
            n265 = event-data() -> ()  [unwired: 1 in, 6 out]
            n266 = call <vilib>:"Add State(s) to Queue__JKI_lib_State_Machine.vi"("State(s) in Front (\"\")"="Data: showBG" ("State(s) in Front (\"\")"), "State(s) in (\"\")"=w493) -> ("States Out"=w492:string)  [unwired: 13 in]
          }
          event "StartButton": Mouse Enter {
            n267 = event-data() -> ()  [unwired: 1 in, 4 out]
            n268 = local write "Help"("Press to start aquisition." ("Help")) -> ()
          }
          event "StartButton": Value Change {
            # "[Covers: REQ32]"
            # "start PWM before acquisition"
            # "Initialize both digitizer aquisition and\n send user event to trigger aquisition loop"
            n269 = event-data() -> ()  [unwired: 1 in, 6 out]
            n270 = local write "StartButton"(FALSE ("StartButton")) -> ()
            n271 = Bundle By Name(cluster=w502, "SysRunning?"=TRUE) -> (w504:T26)
            n272 = call <vilib>:"Add State(s) to Queue__JKI_lib_State_Machine.vi"("State(s) in Front (\"\")"="TCP: stopCam\nUtility: SetDataClass >> Data\nQueue: Flash\nUI: Update\nUtility: StartBeep\nLabJack: 355_PWM_Start\nLabJack: AB_Start\nLabJack: SetV\nDigitizer: Start\nUtility: AquiTimerReset\nUI: DuringAquisition\nLED: BreathGreen\nTCP: sendRunNum\nTCP: sendVideoSource\nTCP: sendChannel\nTCP: startRun", "State(s) in (\"\")"=w506) -> ("States Out"=w507:string)  [unwired: 13 in]
          }
          event User Event {
            # "[Covers: REQ32]"
            # "start PWM before acquisition"
            # "Initialize both digitizer aquisition and\n send user event to trigger aquisition loop"
            n273 = event-data() -> ()  [unwired: 1 in, 5 out]
            n274 = Bundle By Name(cluster=w509, "SysRunning?"=TRUE) -> (w511:T26)
            n275 = call <vilib>:"Add State(s) to Queue__JKI_lib_State_Machine.vi"("State(s) in Front (\"\")"="TCP: stopCam\nUtility: SetDataClass >> Data\nQueue: Flash\nUI: Update\nUtility: StartBeep\nLabJack: 355_PWM_Start\nLabJack: AB_Start\nLabJack: SetV\nDigitizer: Start\nUtility: AquiTimerReset\nUI: DuringAquisition\nLED: BreathGreen\nTCP: sendRunNum\nTCP: sendVideoSource\nTCP: sendChannel\nTCP: startRun", "State(s) in (\"\")"=w513) -> ("States Out"=w514:string)  [unwired: 13 in]
          }
          event "Video Display": Value Change {
            n276 = event-data() -> ("NewVal"=w520:bool)  [unwired: 1 in, 5 out]
            n277 = Select(t="TCP: startCam", s=w520, f="TCP: stopCam") -> (s? t:f=w517:string)
            n278 = call <vilib>:"Add State(s) to Queue__JKI_lib_State_Machine.vi"("State(s) in (\"\")"=w519, "State(s) at Back (\"\")"=w517) -> ("States Out"=w518:string)  [unwired: 13 in]
          }
          event "Video Source": Value Change {
            n279 = event-data() -> ()  [unwired: 1 in, 6 out]
            n280 = call <vilib>:"Add State(s) to Queue__JKI_lib_State_Machine.vi"("State(s) in Front (\"\")"="TCP: sendVideoSource" ("State(s) in Front (\"\")"), "State(s) in (\"\")"=w525) -> ("States Out"=w524:string)  [unwired: 13 in]
          }
          event "StopButton": Mouse Enter {
            n281 = event-data() -> ()  [unwired: 1 in, 4 out]
            n282 = local write "Help"("Press to stop data aquisition." ("Help")) -> ()
          }
          event "StopButton": Value Change {
            # "if system is running, send stop command, if not do nothing."
            # "stop aquisition\nupdate UI"
            n283 = event-data() -> ()  [unwired: 1 in, 6 out]
            n284 = Unbundle By Name(w533) -> ("SysRunning?"=w535:bool)
            n285 = case shown="True" w535 {
              tunnel: ["" ("Empty String Constant") "LabJack: AB_Stop\nLabJack: 355_PWM_Stop\n/*Digitizer: Abort"] -> w536
              tunnel: w533 -> [w540 w544]
              tunnel: [w540 w543] -> w534
              frame False {
              }
              frame True {
                n286 = Bundle By Name(cluster=w544, "SysRunning?"=FALSE) -> (w543:T26)
              }
            }
            n287 = call <vilib>:"Add State(s) to Queue__JKI_lib_State_Machine.vi"("State(s) in Front (\"\")"=w536, "State(s) in (\"\")"=w538) -> ("States Out"=w539:string)  [unwired: 13 in]
            n288 = local write "StopButton"(FALSE ("StopButton")) -> ()
          }
          event User Event {
            # "if system is running, send stop command, if not do nothing."
            # "stop aquisition\nupdate UI"
            n289 = event-data() -> ()  [unwired: 1 in, 5 out]
            n290 = Unbundle By Name(w546) -> ("SysRunning?"=w548:bool)
            n291 = case shown="True" w548 {
              tunnel: ["" ("Empty String Constant") "LabJack: AB_Stop\nLabJack: 355_PWM_Stop\n/*Digitizer: Abort"] -> w549
              tunnel: w546 -> [w553 w557]
              tunnel: [w553 w556] -> w547
              frame False {
              }
              frame True {
                n292 = Bundle By Name(cluster=w557, "SysRunning?"=FALSE) -> (w556:T26)
              }
            }
            n293 = call <vilib>:"Add State(s) to Queue__JKI_lib_State_Machine.vi"("State(s) in Front (\"\")"=w549, "State(s) in (\"\")"=w551) -> ("States Out"=w552:string)  [unwired: 13 in]
          }
          event "Sys Reconfig": Mouse Enter {
            n294 = event-data() -> ()  [unwired: 1 in, 4 out]
            n295 = local write "Help"("Click to reconfig digitizer settings." ("Help")) -> ()
          }
          event "Sys Reconfig": Value Change {
            # "everytime the user change data aquisition setting, need to reinitilize decon engine and realign iRF.\ncheck whether data length has changed, if changed, reinitialize Decon engine\nreset BG ready, need a new BG"
            # "update DAQ FGV"
            n296 = event-data() -> ()  [unwired: 1 in, 6 out]
            n297 = call "SystemConfigEditorV6.vi"("error in"=w573) -> ("error out"=w572:errorcluster, "FLImDAQ out"=w567:T5)  [unwired: 1 in]
            n298 = Unbundle By Name(w570) -> ("FLImDAQ.min record length"=w569:i32)
            n299 = Unbundle By Name(w567) -> ("min record length"=w568:i32)
            n300 = call "FLImDAQ_FGV.vi"("error in (no error)"=w572, "Operation (Read)"=enum16{"Write", "Read"}."Write" ("Operation"), "Write data"=w567) -> ("error out"=w571:errorcluster, "Read data"=w566:T5)  [unwired: 7 in]
            n301 = Equal?(x=w569, y=w568) -> (x = y?=w565:bool)
            n302 = case shown="False" w565 {
              tunnel: ["UI: Cursor Set >> Busy\nDigitizer: Config\nDeconEngine: InitializeCh1\nDeconEngine: InitializeCh2\nDeconEngine: InitializeCh3\nUI: CaliAndiRFNotReady\n/*UI iRF not ready\nUI: Update\nUI: Cursor Set >> Idle" "UI: Cursor Set >> Busy\nDigitizer: Config\nUI: Update\nUI: Cursor Set >> Idle"] -> w564
              frame False {
              }
              frame True {
              }
            }
            n303 = Bundle By Name(cluster=w570, "FLImDAQ"=w566) -> (w576:T26)
            n304 = call <vilib>:"Add State(s) to Queue__JKI_lib_State_Machine.vi"("State(s) in Front (\"\")"=w564, "State(s) in (\"\")"=w574) -> ("States Out"=w575:string)  [unwired: 13 in]
          }
          event "System Hardware Connection Status", "StartButton", "StopButton", "355nm Laser toggle", "Aiming beam toggle", "Cali&iRF alignment", "Background", "Sys Reconfig": Mouse Leave {
            n305 = event-data() -> ()  [unwired: 1 in, 4 out]
            n306 = invoke on="Help" class="Str" method="Reinit To Default"() -> ()  [unwired: 3 in, 3 out]
          }
          event "System Hardware Connection Status.Digitizer": Mouse Enter {
            n307 = event-data() -> ()  [unwired: 1 in, 4 out]
            n308 = local write "Help"("Status of hardware connections. TCP/IP is optional." ("Help")) -> ()
          }
          event "TCP Connect": Value Change {
            n309 = event-data() -> ("NewVal"=w586:bool)  [unwired: 1 in, 5 out]
            n310 = case shown="True" w586 {
              tunnel: ["TCP: Close\nUI: Update" ("State(s) in Front (\"\")") "TCP: SendSettingMacro\nUI: Update" ("State(s) in Front (\"\")")] -> w587
              frame False {
              }
              frame True {
              }
            }
            n311 = call <vilib>:"Add State(s) to Queue__JKI_lib_State_Machine.vi"("State(s) in Front (\"\")"=w587, "State(s) in (\"\")"=w589) -> ("States Out"=w588:string)  [unwired: 13 in]
          }
          event User Event {
            # "if aquisition loop is error out. Stop digitizer, update front panel indicator, stop both laser and \nOption 1: parse and save data\nOption 2: Flash queue if scout run. [Covers: REQ23]"
            n312 = event-data() -> ()  [unwired: 1 in, 5 out]
            n313 = case shown="\"Cali\"" "Data Class" {
              tunnel: [w611 "UI: Cursor Set >> Busy\nUtility: SetAllChanAutoGain\nUtility: RestoreDeConChan\nData: parseRunData\nData: irfAlignment\nUI: Cursor Set >> Idle" "UI: Cursor Set >> Busy\nUtility: SetAllChanAutoGain\nUtility: RestoreDeConChan\nData: parseRunData\nData: saveBGtoFGV\nData: saveBGtoFile\nUI: Cursor Set >> Idle\nData: showBG\nRun: BGIncrement"] -> w601
              frame "Data", Default {
                n314 = local read "Video Display"() -> (w613:bool)
                n315 = Select(t="TCP: startCam", s=w613, f="") -> (s? t:f=w609:string)
                n316 = call <vilib>:"Add State(s) to Queue__JKI_lib_State_Machine.vi"("State(s) in Front (\"\")"="UI: Cursor Set >> Busy\nData: parseRunData\nData: saveRunData\nUI: Cursor Set>>Idle" ("State(s) in Front (\"\")"), "State(s) in (\"\")"=w609) -> ("States Out"=w611:string)  [unwired: 13 in]
              }
              frame "Cali" {
              }
              frame "BG" {
              }
            }
            n317 = Bundle By Name(cluster=w603, "SysRunning?"=FALSE) -> (w604:T26)
            n318 = Select(t="" ("State(s) in Front (\"\")"), s="Skip Data Save?", f=w601) -> (s? t:f=w598:string)
            n319 = call <vilib>:"Add State(s) to Queue__JKI_lib_State_Machine.vi"("State(s) in Front (\"\")"="TCP: stopRun\nUI: Update\nLabJack: AB_Stop\nLabJack: 355_PWM_Stop\nDigitizer: Abort\nLabJack: ZeroV\nUtility: EndBeep\nLED: BreathOff" ("State(s) in Front (\"\")"), "State(s) in (\"\")"=w598, "State(s) at Back (\"\")"="Macro: SysReadyForAq\nUI: Update" ("State(s) in Front (\"\")")) -> ("States Out"=w596:string)  [unwired: 12 in]
            n320 = call <vilib>:"Add State(s) to Queue__JKI_lib_State_Machine.vi"("State(s) in Front (\"\")"=w596, "State(s) in (\"\")"=w605) -> ("States Out"=w606:string)  [unwired: 13 in]
          }
          event Panel Close? {
            # "Discard the event because we'll close the front panel ourselves in Macro: Exit"
            # "Close Panel button (pressed) Event\n(this executes Macro: Exit to terminate the VI)"
            n321 = event-data() -> ()  [unwired: 1 in, 1 out]
            n322 = event-data ("Event Filter Node")("Discard?"=TRUE) -> ()  [unwired: 1 in, 1 out]
            n323 = call <vilib>:"Add State(s) to Queue__JKI_lib_State_Machine.vi"("State(s) in Front (\"\")"="Macro: Exit", "State(s) in (\"\")"=w621) -> ("States Out"=w620:string)  [unwired: 13 in]
          }
        }
      }
      frame "---------- Macro ----------" {
        # "Do not put any code in this frame.\n(It is a separator no-op. You can make a copy of this frame to create a new Macro frame)"
        n324 = call <vilib>:"Add State(s) to Queue__JKI_lib_State_Machine.vi"("State(s) in (\"\")"=w626) -> ("States Out"=w625:string)  [unwired: 14 in]
      }
      frame "Macro: Initialize" {
        # "load Labjack setting 1st as it contaisn laser pin infortmation"
        # "start laser 1st, need 7.5s for laser to get ready"
        # "Initialization Macro\n(This is called once, when the VI starts)"
        n325 = call <vilib>:"Add State(s) to Queue__JKI_lib_State_Machine.vi"("State(s) in Front (\"\")"="UI: showDisclaimer\nUI: Cursor Set >> Busy\nData: Initialize\nInitialize Core Data\nUI: Initialize\nUI: Front Panel State >> Open\nMacro: LoadSysConfig\nTCP: InitializeNew\nTCP: checkSource\nUI: Update\nLabJack: Open\nLabJack: SetDefaultSub\nLED: OpenVIRef\nLED: BreathOrange\nUI: Update\n355 Laser: CheckControllerStatus\n355 Laser: Laser enable\n355 Laser: Dewelling>>500\n355 Laser: CheckControllerStatus\nUI: Update\nLabJack: 355_PWM_Config\nLabJack: AB_PWM_Config\nUI: Update", "State(s) in (\"\")"="Digitizer: Initialize\nDigitizer: Config\nUI: Update\nAimingBeam: Initialize\nAimingBeam: Set Status>>Enable\nAimingBeam: Set Current\nUI: Update\n355 Laser: Check Dewelling\nUI: Cursor Set >> Idle\nCase: GetID\nUI: Update\nTCP: SendSettingMacro\nCase: CreatFileStruct\nUI: Update\nData: loadLastUseMacro\nDeconEngine: InitilizeMacro\nGraph: SetXMultiplier\nGraph: AddCursors\nAPD: Initialize\nAPD: LoadFromSerial\nAPD: UpdateCtrlVLimit\nAPD: GetGainLimits\nPID: loadPID\nLED: BreathOff\nMacro: SysReadyForAq") -> ("States Out"=w627:string)  [unwired: 13 in]
        n326 = call <vilib>:"Add State(s) to Queue__JKI_lib_State_Machine.vi"("State(s) in Front (\"\")"=w627, "State(s) in (\"\")"=w635) -> ("States Out"=w634:string)  [unwired: 13 in]
        "Help" <- "Hover over controls to see help!" ("Help")
      }
      frame "Macro: LoadSysConfig" {
        # "System configuration Macro. [Covers: REQ15]\n(Load configurations for different component of the system)"
        n327 = call <vilib>:"Add State(s) to Queue__JKI_lib_State_Machine.vi"("State(s) in Front (\"\")"="SysConfig: Load Sys Config\nSysConfig: Load Digitizer Setting\nSysConfig: Load AB setting\nSysConfig: Load LJ Pinout\nSysConfig: Load 355 PWM\nSysConfig: LoadAPDSerialNumber\nSysConfig: LoadABVideoSetting\nSysConfig: LoadCursorLocation", "State(s) in (\"\")"=w641) -> ("States Out"=w640:string)  [unwired: 13 in]
      }
      frame "Macro: SysReadyForAq" {
        # "Macro for system ready\n(It is a separator no-op. You can make a copy of this frame to create a new Macro frame)"
        n328 = call <vilib>:"Add State(s) to Queue__JKI_lib_State_Machine.vi"("State(s) in Front (\"\")"="UI: ReadyForAquisition\nLED: Green" ("State(s) in Front (\"\")"), "State(s) in (\"\")"=w647) -> ("States Out"=w646:string)  [unwired: 13 in]
      }
      frame "Macro: Exit" {
        # "close LJ last"
        # "check whether hardware is initilized, if so close, if not do nothing"
        # "Exit Macro, close all hardware\n(This is called once, when the VI exits)"
        n329 = Unbundle By Name(w666) -> ("System Status.Digitizer"=w662:bool, "System Status.Aiming Beam"=w661:bool, "System Status.355 Laser"=w660:bool, "System Status.Labjack"=w651:bool, "Core.Close Panel on Exit?"=w655:bool)
        n330 = case shown="True" w662 {
          tunnel: ["" ("Empty String Constant") "Digitizer: Close"] -> w657
          frame False {
          }
          frame True {
          }
        }
        n331 = case shown="True" w651 {
          tunnel: ["" ("Empty String Constant") "LabJack: SetDefaultAndClose"] -> w648
          frame False {
          }
          frame True {
          }
        }
        n332 = case shown="True" w661 {
          tunnel: ["" ("Empty String Constant") w673] -> w650
          frame False {
          }
          frame True {
            w673 = "AimingBeam: Set Status >> Disable\nAimingBeam: Close"  # AimingBeam: Set Status >> Disable AimingBeam: Close
          }
        }
        n333 = case shown="True" w660 {
          tunnel: ["" ("Empty String Constant") "355 Laser: Close\n355 Laser: CheckControllerStatus"] -> w649
          frame False {
          }
          frame True {
          }
        }
        n334 = Select(t="UI: Front Panel State >> Close", s=w655, f="" ("Empty String Constant")) -> (s? t:f=w652:string)
        n335 = call <vilib>:"Add State(s) to Queue__JKI_lib_State_Machine.vi"("State(s) in Front (\"\")"="TCP: Close", "State(s) in (\"\")"=w657, "State(s) at Back (\"\")"=w650) -> ("States Out"=w659:string)  [unwired: 12 in]
        n336 = call <vilib>:"Add State(s) to Queue__JKI_lib_State_Machine.vi"("State(s) in Front (\"\")"=w659, "State(s) in (\"\")"=w649, "State(s) at Back (\"\")"=w648) -> ("States Out"=w654:string)  [unwired: 12 in]
        n337 = call <vilib>:"Add State(s) to Queue__JKI_lib_State_Machine.vi"("State(s) in Front (\"\")"=w654, "State(s) in (\"\")"="UI: Update\nUI: Reset\nGraph: SaveCursorLoc\nLED: CloseVIRef\nQueue: Destory\nData: Cleanup\nExit", "State(s) at Back (\"\")"=w652) -> ("States Out"=w663:string)  [unwired: 12 in]
        n338 = call <vilib>:"Add State(s) to Queue__JKI_lib_State_Machine.vi"("State(s) in Front (\"\")"=w663, "State(s) in (\"\")"=w669) -> ("States Out"=w668:string)  [unwired: 13 in]
      }
      frame "---------- Data ----------" {
        # "Do not put any code in this frame.\n(It is a separator no-op. You can make a copy of this frame to create a new Data frame)"
        n339 = call <vilib>:"Add State(s) to Queue__JKI_lib_State_Machine.vi"("State(s) in (\"\")"=w682) -> ("States Out"=w681:string)  [unwired: 14 in]
      }
      frame "Data: Initialize" {
        w683 = path ""  # CaliPath
        w684 = dbl[] []  # V4
        w685 = dbl[][] []  # Ch4Data
        w686 = FALSE  # bothVidSourceAvail
        w687 = T1 {"Main Frame Grabber"=FALSE, "Side Frame Grabber"=FALSE, "Main Camera"=FALSE, "Side Camera"=FALSE}  # video source
        w688 = FALSE  # LED vi ref open?
        w690 = T25 {"DeCon Channel"=enum."1", "Scale Bar"=FALSE, "Scale Low"=3.0, "Scale High"=8.0, "ANSI"=20.0, "Radius"=1.0, "3D?"=FALSE, "Firefly?"=FALSE, "Pentero?"=FALSE}  # VideoConfig
        w691 = T29 {"Ch1APDSerial#"="", "Ch2APDSerial#"="", "Ch3APDSerial#"="", "Ch4APDSerial#"=""}  # APDSerialNum
        w692 = u32 0  # Aquisition Timer
        w693 = cluster{"RunID":i8, "BG ID":i8, "Cali ID":i8} {"RunID"=1, "BG ID"=1, "Cali ID"=1}  # IDs
        w694 = refnum<vi> refnum  # LED vi reference
        w695 = path ""  # TempPath
        w696 = T30 {"DataPath"=path "", "BG Path"=path "", "iRFPath"=path "", "CaliPath"=path ""}  # Pathes
        w698 = dbl[] []  # V3
        w699 = dbl[] []  # V2
        w700 = dbl[] []  # V1
        w702 = u32 0  # FastTimer
        w703 = u32 0  # SlowTimer
        w704 = dbl[][] []  # Ch3Data
        w705 = dbl[][] []  # Ch2Data
        w689 = dbl[][] []  # Ch1Data
        w708 = T2 {"Digitizer"=FALSE, "Labjack"=FALSE, "Aiming Beam"=FALSE, "355 Laser"=FALSE, "TCP/IP"=FALSE}  # System Status
        w709 = T31 {"DIO_EF_CLOCK1_DIVISOR"=16, "DIO_EF_CLOCK1_ROLL_VALUE"=25000, "DIO#_EF_INDEX"=0, "DIO#_EF_OPTIONS"=1, "DIO#_EF_CONFIG_A"=6250}  # AB PWM setting
        w710 = T4 {"Ch1 Bias"="TDA11", "Ch2 Bias"="DAC10", "Ch3 Bias"="DAC0", "Ch4 Bias"="DAC0", "355 PWM"="FIO0", "AimingBeam PWM"="FIO2", "Laser Ready"="FIO3", "Interlock"="FIO1", "Laser Start/Stop"="FIO1", "Red LED"="FIO1", "Green LED"="FIO1", "Foot Pedal"="DIO15"}  # LJ Pinout
        w711 = 0  # TCP attempt count
        w712 = u32 0  # Laser start tic
        w713 = refnum<k20>[] []  # niTClk sessions
        w714 = u32 0  # Last Trigger
        w715 = T31 {"DIO_EF_CLOCK1_DIVISOR"=16, "DIO_EF_CLOCK1_ROLL_VALUE"=25000, "DIO#_EF_INDEX"=0, "DIO#_EF_OPTIONS"=1, "DIO#_EF_CONFIG_A"=6250}  # 355 PWM setting
        w716 = T32 {"Aiming Beam COM Port"="COM3", "Min Current"=0.0, "Max Current"=63.0, "Default Current"=20.0, "Freq"=0}  # AB Cluster
        w717 = T33 {"resource name"="", "resource name 2"="", "Channel"=enum."Channel 0", "trigger source"="VAL_EXTERNAL", "trigger level"=0.5, "trigger delay"=1.35e-07, "min sample rate"=12500000000.0, "min record length"=2500, "vertical range"=1.0, "vertical offset"=-0.25, "Waveform to Avg"=2000}  # FLImDAQ
        w718 = FALSE  # SysRunning?
        w706 = path ""  # DefaultPath
        w719 = ""  # CaseID
        w720 = T7 {"Ch1Enable?"=FALSE, "Ch2Enable?"=FALSE, "Ch3Enable?"=FALSE, "Ch1AutoGain?"=FALSE, "Ch2AutoGain?"=FALSE, "Ch3AutoGain?"=FALSE, "AimingBeamEnable?"=FALSE}  # SysConfigCluster
        w721 = T34 {"Current VI Reference"=refnum, "Close Panel on Exit?"=FALSE}  # Core
        # "Initialize the shift-register data, here.\n(data names are defined by what you wire into the bundle function)"
        n340 = Bundle("Core"=w721, "SysConfigCluster"=w720, "System Status"=w708, "IDs"=w693, "CaseID"=w719, "DefaultPath"=w706, "Pathes"=w696, "FLImDAQ"=w717, "SysRunning?"=w718, "AB Cluster"=w716, "LJ Pinout"=w710, "355 PWM setting"=w715, "AB PWM setting"=w709, "Last Trigger"=w714, "niTClk sessions"=w713, "Laser start tic"=w712, "TCP attempt count"=w711, "Ch1Data"=w689, "Ch2Data"=w705, "Ch3Data"=w704, "Ch4Data"=w685, "V1"=w700, "V2"=w699, "V3"=w698, "V4"=w684, "SlowTimer"=w703, "FastTimer"=w702, "listener ID"=refnum<k5> refnum, "TempPath"=w695, "CaliPath"=w683, "LED vi reference"=w694, "Aquisition Timer"=w692, "APDSerialNum"=w691, "VideoConfig"=w690, "LED vi ref open?"=w688, "video source"=w687, "bothVidSourceAvail"=w686) -> (w697:T26)  [unwired: 1 in]
        n341 = call <vilib>:"Add State(s) to Queue__JKI_lib_State_Machine.vi"("State(s) in (\"\")"=w724) -> ("States Out"=w723:string)  [unwired: 14 in]
      }
      frame "Data: loadLastUseMacro" {
        # "Load last use BG and Cali and iRF.\n(It is a separator no-op. You can make a copy of this frame to create a new Data frame)"
        n342 = call <vilib>:"Add State(s) to Queue__JKI_lib_State_Machine.vi"("State(s) in Front (\"\")"="Data: loadLastUseBG\nData: loadSystemCali\nData: loadLastUseiRF\n/*Data: LoadiRFFromAPDFile\nUI: CaliAndiRFLoaded\nData: ShowiRF" ("State(s) in Front (\"\")"), "State(s) in (\"\")"=w730) -> ("States Out"=w729:string)  [unwired: 13 in]
      }
      frame "Data: loadLastUseBG" {
        w734 = enum16{"write", "read"}."write" ("action")
        # "Load last use BG.\n()"
        n343 = Unbundle By Name(w753) -> ("TempPath"=w752:path)
        n344 = call "FLImDAQ_FGV.vi"() -> ("Read data"=w748:T5)  [unwired: 10 in, 1 out]
        n345 = Build Path(base path=w752, name or relative path="Background.tdms") -> (appended path=w751:path)
        n346 = call "ReadBGorCali (SubVI).vi"("DataType"=enum16{"BG", "Cali"}."BG", "error in (no error)"=w750, "file path in"=w751) -> ("error out"=w749:errorcluster, "AvgDataCluster"=w744:T35)  [unwired: 6 in, 1 out]
        n347 = Unbundle By Name(w744) -> ("Channel 1"=w731:dbl[], "Channel 2"=w743:dbl[], "Channel 3"=w736:dbl[], "Channel 4"=w733:dbl[])
        n348 = Unbundle By Name(w748) -> ("min record length"=w740:i32)
        n349 = Array Size(array=w731) -> (size(s)=w742:i32)
        "BG length" <- w742
        n350 = Equal?(x=w742, y=w740) -> (x = y?=w741:bool)
        n351 = Select(t="UI: BGLoaded" ("State(s) in Front (\"\")"), s=w741, f="UI: BGSizeError" ("State(s) in Front (\"\")")) -> (s? t:f=w745:string)
        n352 = case shown="True" w741 {
          tunnel: w731 -> [_ w764]
          tunnel: w743 -> [_ w763]
          tunnel: w736 -> [_ w762]
          tunnel: w740 -> [w759 _]
          tunnel: [w758 w764] -> w739
          tunnel: [w758 w763] -> w738
          tunnel: [w758 w762] -> w737
          tunnel: w733 -> [_ w761]
          tunnel: [w758 w761] -> w732
          frame False {
            # "If error set BG all 0, update UI"
            n353 = for {
              N: w759 -> [_]
              tunnel: [0.0] -> w758 mode=indexing
            }
          }
          frame True {
            # "If no error, check size match"
          }
        }
        n354 = call "BG4FGV.vi"("action"=w734, "BG4 in"=w732) -> ()  [unwired: 8 in, 2 out]
        n355 = call "BG3FGV.vi"("action"=w734, "BG3 in"=w737) -> ()  [unwired: 8 in, 2 out]
        n356 = call "BG1FGV.vi"("action"=w734, "BG1 in"=w739) -> ()  [unwired: 8 in, 2 out]
        n357 = call "BG2FGV.vi"("action"=w734, "BG2 in"=w738) -> ()  [unwired: 8 in, 2 out]
        n358 = call <vilib>:"Add State(s) to Queue__JKI_lib_State_Machine.vi"("State(s) in Front (\"\")"=w745, "State(s) in (\"\")"=w757) -> ("States Out"=w756:string)  [unwired: 13 in]
      }
      frame "Data: loadSystemCali" {
        # "Load last use calibration.\n()"
        n359 = Unbundle By Name(w772) -> ("CaliPath"=w771:path)
        n360 = Build Path(base path=w771, name or relative path="Calibration.tdms") -> (appended path=w767:path)
        n361 = call "ReadBGorCali (SubVI).vi"("DataType"=enum16{"BG", "Cali"}."Cali", "error in (no error)"=w766, "file path in"=w767) -> ("error out"=w768:errorcluster, "CtrlVCluster"=w770:T36, "AvgDataCluster"=w769:T35)  [unwired: 6 in]
        n362 = case shown="No Error" w768 {
          tunnel: w770 -> [w791 _]
          tunnel: w769 -> [w790 _]
          frame No Error {
            w781 = T37 {"Ch1 WF"=[], "Ch2 WF"=[], "Ch3 WF"=[], "Ch4 WF"=[], "V1"=0.0, "V2"=0.0, "V3"=0.0, "V4"=0.0}  # SysCaliData
            n363 = Unbundle By Name(w790) -> ("Channel 1"=w789:dbl[], "Channel 2"=w788:dbl[], "Channel 3"=w787:dbl[], "Channel 4"=w780:dbl[])
            n364 = Unbundle By Name(w791) -> ("V 1"=w786:dbl[], "V 2"=w785:dbl[], "V 3"=w779:dbl[], "V 4"=w777:dbl[])
            n365 = Index Array(array=w786) -> (element=w784:dbl)  [unwired: 1 in]
            n366 = Index Array(array=w785) -> (element=w783:dbl)  [unwired: 1 in]
            n367 = Index Array(array=w779) -> (element=w782:dbl)  [unwired: 1 in]
            n368 = Index Array(array=w777) -> (element=w778:dbl)  [unwired: 1 in]
            n369 = Bundle By Name(cluster=w781, "Ch1 WF"=w789, "Ch2 WF"=w788, "Ch3 WF"=w787, "Ch4 WF"=w780, "V1"=w784, "V2"=w783, "V3"=w782, "V4"=w778) -> (w792:T37)
            n370 = global write "GlobalVariables.vi" "SysCaliData"(w792) -> ()
          }
          frame Error {
          }
        }
        n371 = call <vilib>:"Add State(s) to Queue__JKI_lib_State_Machine.vi"("State(s) in (\"\")"=w776) -> ("States Out"=w775:string)  [unwired: 14 in]
      }
      frame "Data: LoadiRFFromAPDFile" {
        w822 = T19 {"Ch1 iRF"=[], "Ch2 iRF"=[], "Ch3 iRF"=[], "Ch4 iRF"=[]}  # LastUseiRF
        # "only load the last 5th  iRF for the moment"
        # "Load APD detector data\n(It is a separator no-op. You can make a copy of this frame to create a new Data frame)"
        n372 = Unbundle By Name(w844) -> ("APDSerialNum.Ch1APDSerial#"=w843:string, "APDSerialNum.Ch2APDSerial#"=w824:string, "APDSerialNum.Ch3APDSerial#"=w823:string, "APDSerialNum.Ch4APDSerial#"=w820:string)
        n373 = call "CreatFromSerialNumNoRaw.vi"("error in (no error)"=w821, "APD Serial #"=w843) -> ("error out"=w841:errorcluster, "APDClass out"=w842:refnum<class "APDClass.lvclass">)  [unwired: 8 in]
        n374 = call "CreatFromSerialNumNoRaw.vi"("error in (no error)"=w821, "APD Serial #"=w824) -> ("error out"=w832:errorcluster, "APDClass out"=w833:refnum<class "APDClass.lvclass">)  [unwired: 8 in]
        n375 = call "CreatFromSerialNumNoRaw.vi"("error in (no error)"=w821, "APD Serial #"=w823) -> ("error out"=w826:errorcluster, "APDClass out"=w827:refnum<class "APDClass.lvclass">)  [unwired: 8 in]
        n376 = call "CreatFromSerialNumNoRaw.vi"("error in (no error)"=w821, "APD Serial #"=w820) -> ("error out"=w818:errorcluster, "APDClass out"=w819:refnum<class "APDClass.lvclass">)  [unwired: 8 in]
        n377 = call-dynamic "Read iRFData.vi"("error in (no error)"=w841, "APDClass in"=w842) -> ("iRFData"=w840:T38)  [unwired: 7 in, 2 out]
        n378 = call-dynamic "Read iRFData.vi"("error in (no error)"=w832, "APDClass in"=w833) -> ("iRFData"=w836:T38)  [unwired: 7 in, 2 out]
        n379 = call-dynamic "Read iRFData.vi"("error in (no error)"=w826, "APDClass in"=w827) -> ("iRFData"=w830:T38)  [unwired: 7 in, 2 out]
        n380 = call-dynamic "Read iRFData.vi"("error in (no error)"=w818, "APDClass in"=w819) -> ("iRFData"=w817:T38)  [unwired: 7 in, 2 out]
        n381 = Unbundle By Name(w840) -> ("iRFWFsAvg"=w839:dbl[][])
        n382 = Unbundle By Name(w836) -> ("iRFWFsAvg"=w835:dbl[][])
        n383 = Unbundle By Name(w830) -> ("iRFWFsAvg"=w829:dbl[][])
        n384 = Unbundle By Name(w817) -> ("iRFWFsAvg"=w814:dbl[][])
        n385 = Array Size(array=w839) -> (size(s)=w838:i32[])
        n386 = Array Size(array=w835) -> (size(s)=w831:i32[])
        n387 = Array Size(array=w829) -> (size(s)=w825:i32[])
        n388 = Array Size(array=w814) -> (size(s)=w815:i32[])
        n389 = Index Array(array=w838, index=0) -> (element=w813:i32)
        n390 = Index Array(array=w831, index=0) -> (element=w809:i32)
        n391 = Index Array(array=w825, index=0) -> (element=w806:i32)
        n392 = Index Array(array=w815, index=0) -> (element=w803:i32)
        n393 = Subtract(x=w813, y=5) -> (x-y=w811:i32)
        n394 = Subtract(x=w809, y=5) -> (x-y=w808:i32)
        n395 = Subtract(x=w806, y=5) -> (x-y=w805:i32)
        n396 = Subtract(x=w803, y=5) -> (x-y=w802:i32)
        n397 = Index Array(array=w839, index (row)=w811) -> (element=w801:dbl[])  [unwired: 1 in]
        n398 = Index Array(array=w835, index (row)=w808) -> (element=w800:dbl[])  [unwired: 1 in]
        n399 = Index Array(array=w829, index (row)=w805) -> (element=w799:dbl[])  [unwired: 1 in]
        n400 = Index Array(array=w814, index (row)=w802) -> (element=w798:dbl[])  [unwired: 1 in]
        n401 = call "DownSampleAndShiftiRF (SubVI).vi"("ArrayIn"=w801) -> ("ArrayOut"=w797:dbl[])  [unwired: 10 in]
        n402 = call "DownSampleAndShiftiRF (SubVI).vi"("ArrayIn"=w800) -> ("ArrayOut"=w793:dbl[])  [unwired: 10 in]
        n403 = call "DownSampleAndShiftiRF (SubVI).vi"("ArrayIn"=w799) -> ("ArrayOut"=w794:dbl[])  [unwired: 10 in]
        n404 = call "DownSampleAndShiftiRF (SubVI).vi"("ArrayIn"=w798) -> ("ArrayOut"=w796:dbl[])  [unwired: 10 in]
        n405 = call <vilib>:"Add State(s) to Queue__JKI_lib_State_Machine.vi"("State(s) in (\"\")"=w847) -> ("States Out"=w846:string)  [unwired: 14 in]
        n406 = Bundle(cluster=w822, "Ch1 iRF"=w797, "Ch2 iRF"=w793, "Ch3 iRF"=w794, "Ch4 iRF"=w796) -> (w795:T19)
        n407 = global write "GlobalVariables.vi" "LastUseiRF"(w795) -> ()
      }
      frame "Data: loadLastUseiRF" {
        # "Load last use iRF.\n()"
        n408 = Unbundle By Name(w853) -> ("TempPath"=w852:path)
        n409 = Build Path(base path=w852, name or relative path="iRF.tdms") -> (appended path=w858:path)
        n410 = TDMS Open(8:w848, 11:w858) -> (0:w856:errorcluster, 3:w857:refnum<k34>)  [unwired: 5 in]
        n411 = TDMS Read(0:w857, 11:w856, 12:dbl[][] []) -> (4:w851:refnum<k34>, 10:w854:dbl[][], 15:w850:errorcluster)  [unwired: 5 in, 3 out]
        n412 = TDMS Close(8:w850, 11:w851) -> (0:w849:errorcluster)  [unwired: 1 out]
        n413 = case shown="No Error" w850 {
          tunnel: w854 -> [w868 _]
          frame No Error {
            w871 = T19 {"Ch1 iRF"=[], "Ch2 iRF"=[], "Ch3 iRF"=[], "Ch4 iRF"=[]}  # LastUseiRF
            n414 = Index Array(array=w868, index (row)=0) -> (element=w863:dbl[])  [unwired: 1 in]
            n415 = Index Array(array=w868, index (row)=1) -> (element=w864:dbl[])  [unwired: 1 in]
            n416 = Index Array(array=w868, index (row)=2) -> (element=w865:dbl[])  [unwired: 1 in]
            n417 = Index Array(array=w868, index (row)=3) -> (element=w866:dbl[])  [unwired: 1 in]
            n418 = Add Array Elements(numeric array=w863) -> (sum=w877:dbl)
            n419 = Add Array Elements(numeric array=w864) -> (sum=w875:dbl)
            n420 = Add Array Elements(numeric array=w865) -> (sum=w873:dbl)
            n421 = Add Array Elements(numeric array=w866) -> (sum=w869:dbl)
            n422 = Divide(x=w863, y=w877) -> (x/y=w876:dbl[])
            n423 = Divide(x=w864, y=w875) -> (x/y=w874:dbl[])
            n424 = Divide(x=w865, y=w873) -> (x/y=w872:dbl[])
            n425 = Divide(x=w866, y=w869) -> (x/y=w867:dbl[])
            n426 = Bundle(cluster=w871, "Ch1 iRF"=w876, "Ch2 iRF"=w874, "Ch3 iRF"=w872, "Ch4 iRF"=w867) -> (w879:T19)
            n427 = Array Size(array=w863) -> (size(s)=→"iRF length":i32)
            n428 = global write "GlobalVariables.vi" "LastUseiRF"(w879) -> ()
          }
          frame Error {
          }
        }
        n429 = call <vilib>:"Add State(s) to Queue__JKI_lib_State_Machine.vi"("State(s) in (\"\")"=w862) -> ("States Out"=w861:string)  [unwired: 14 in]
      }
      frame "Data: ShowiRF" {
        # "Show loaded iRF.\n(It is a separator no-op. You can make a copy of this frame to create a new Data frame)"
        n430 = global read "GlobalVariables.vi" "LastUseiRF"() -> (w888:T19)
        n431 = Unbundle By Name(w888) -> ("Ch1 iRF"=w887:dbl[], "Ch2 iRF"=w886:dbl[], "Ch3 iRF"=w885:dbl[], "Ch4 iRF"=w884:dbl[])
        n432 = Build Array(w887, w886, w885, w884) -> (→"iRF Graph":dbl[][])
        n433 = call <vilib>:"Add State(s) to Queue__JKI_lib_State_Machine.vi"("State(s) in (\"\")"=w893) -> ("States Out"=w892:string)  [unwired: 14 in]
      }
      frame "Data: saveCalibration" {
        # "Average data and save calibration file. [Covers: REQ11]\n(It is a separator no-op. You can make a copy of this frame to create a new Data frame)"
        n434 = Unbundle By Name(w912) -> ("Ch1Data"=w911:dbl[][], "V1"=w910:dbl[], "Ch2Data"=w909:dbl[][], "V2"=w908:dbl[], "Ch3Data"=w907:dbl[][], "V3"=w906:dbl[], "Ch4Data"=w897:dbl[][], "V4"=w896:dbl[], "Pathes.CaliPath"=w915:path, "IDs.Cali ID"=w914:i8)
        n435 = Increment(x=w914) -> (x+1=w898:i8)
        n436 = Bundle("Ch1Data"=w911, "V1"=w910) -> (w905:cluster{"Ch1Data":dbl[][], "V1":dbl[]})  [unwired: 1 in]
        n437 = Bundle("Ch4Data"=w897, "V4"=w896) -> (w895:cluster{"Ch4Data":dbl[][], "V4":dbl[]})  [unwired: 1 in]
        n438 = Bundle("Ch2Data"=w909, "V2"=w908) -> (w904:cluster{"Ch2Data":dbl[][], "V2":dbl[]})  [unwired: 1 in]
        n439 = Bundle("Ch3Data"=w907, "V3"=w906) -> (w903:cluster{"Ch3Data":dbl[][], "V3":dbl[]})  [unwired: 1 in]
        n440 = Format Value(string ("")="Calibration" ("default name"), format string="%02d", value (0)=w898) -> (output string=w917:string)
        n441 = Build Path(base path=w915, name or relative path=w917) -> (appended path=w902:path)
        n442 = call "SaveBGorCali(SubVI).vi"("Channel1"=w905, "BG path"=w902, "DataType"=enum16{"BG", "Cali"}."Cali", "Channel 2"=w904, "Channel 3"=w903, "Channel 4"=w895, "error in (no error)"=w901, "SytemID"="UCDVetMed") -> ("error out"=w900:errorcluster)  [unwired: 7 in]
        n443 = call <vilib>:"Add State(s) to Queue__JKI_lib_State_Machine.vi"("State(s) in (\"\")"=w920) -> ("States Out"=w919:string)  [unwired: 14 in]
      }
      frame "Data: saveiRF" {
        w926 = enum16{"write", "read"}."read" ("action")
        # "Get iRF from decon stracture and save it on disk.\n(It is a separator no-op. You can make a copy of this frame to create a new Data frame)"
        n444 = Unbundle By Name(w943) -> ("TempPath"=w942:path)
        n445 = call "Ch1DeconEngineFGV.vi"("action(read)"=w926) -> ("Error Out"=w948:errorcluster, "Ch1DeconEngine out"=w949:refnum<class "LaguerreDeconEngineClass.lvclass">)  [unwired: 9 in]
        n446 = call "Ch2DeconEngineFGV.vi"("action(read)"=w926) -> ("Error Out"=w946:errorcluster, "Ch2DeconEngine out"=w947:refnum<class "LaguerreDeconEngineClass.lvclass">)  [unwired: 9 in]
        n447 = call "Ch3DeconEngineFGV.vi"("action(read)"=w926) -> ("Error Out"=w944:errorcluster, "Ch3DeconEngine out"=w945:refnum<class "LaguerreDeconEngineClass.lvclass">)  [unwired: 9 in]
        n448 = call "Ch4DeconEngineFGV.vi"("action(read)"=w926) -> ("Error Out"=w925:errorcluster, "Ch3DeconEngine out"=w924:refnum<class "LaguerreDeconEngineClass.lvclass">)  [unwired: 9 in]
        n449 = Build Path(base path=w942, name or relative path="iRF" ("default name")) -> (appended path=w940:path)
        n450 = call "getIRF.vi"("error in (no error)"=w925, "LaguerreDeconEngineClass in"=w924) -> ("iRF"=w923:dbl[])  [unwired: 7 in, 2 out]
        n451 = call "getIRF.vi"("error in (no error)"=w948, "LaguerreDeconEngineClass in"=w949) -> ("iRF"=w931:dbl[])  [unwired: 7 in, 2 out]
        n452 = call "getIRF.vi"("error in (no error)"=w946, "LaguerreDeconEngineClass in"=w947) -> ("iRF"=w930:dbl[])  [unwired: 7 in, 2 out]
        n453 = call "getIRF.vi"("error in (no error)"=w944, "LaguerreDeconEngineClass in"=w945) -> ("iRF"=w929:dbl[])  [unwired: 7 in, 2 out]
        n454 = TDMS Open(8:w939, 10:T20."create or replace" ("operation (0:open)"), 11:w940) -> (0:w936:errorcluster, 3:w937:refnum<k34>)  [unwired: 4 in]
        n455 = Bundle(cluster=T19 {"Ch1 iRF"=[], "Ch2 iRF"=[], "Ch3 iRF"=[], "Ch4 iRF"=[]} ("LastUseiRF"), "Ch1 iRF"=w931, "Ch2 iRF"=w930, "Ch3 iRF"=w929, "Ch4 iRF"=w923) -> (w927:T19)
        n456 = Build Array(w931, w930, w929, w923) -> (w935:dbl[][])
        n457 = global write "GlobalVariables.vi" "LastUseiRF"(w927) -> ()
        n458 = TDMS Write(0:w937, 5:"iRF" ("group name in (Untitled)"), 7:string[] ["Ch1", "Ch2", "Ch3", "Ch4"] ("channel name(s) in (Untitled)"), 9:w935, 11:w936) -> (4:w934:refnum<k34>, 15:w933:errorcluster)  [unwired: 1 in, 2 out]
        n459 = TDMS Close(8:w933, 11:w934) -> (0:w932:errorcluster)  [unwired: 1 out]
        n460 = call <vilib>:"Add State(s) to Queue__JKI_lib_State_Machine.vi"("State(s) in (\"\")"=w952) -> ("States Out"=w951:string)  [unwired: 14 in]
      }
      frame "Data: saveBGtoFGV" {
        w953 = enum16{"write", "read"}."write" ("action")
        # "Save BG and pass it to FGV.\n(save BG to disk and set it to FGV)"
        n461 = Unbundle By Name(w963) -> ("Ch1Data"=w962:dbl[][], "Ch2Data"=w961:dbl[][], "Ch3Data"=w960:dbl[][], "Ch4Data"=w955:dbl[][])
        n462 = call "AvgArrayTimeCritical.vi"("2D array"=w962) -> ("1D Avg"=w959:dbl[])  [unwired: 10 in]
        n463 = call "AvgArrayTimeCritical.vi"("2D array"=w961) -> ("1D Avg"=w958:dbl[])  [unwired: 10 in]
        n464 = call "AvgArrayTimeCritical.vi"("2D array"=w960) -> ("1D Avg"=w957:dbl[])  [unwired: 10 in]
        n465 = call "AvgArrayTimeCritical.vi"("2D array"=w955) -> ("1D Avg"=w954:dbl[])  [unwired: 10 in]
        n466 = call "BG1FGV.vi"("action"=w953, "BG1 in"=w959) -> ()  [unwired: 8 in, 2 out]
        n467 = call "BG2FGV.vi"("action"=w953, "BG2 in"=w958) -> ()  [unwired: 8 in, 2 out]
        n468 = call "BG3FGV.vi"("action"=w953, "BG3 in"=w957) -> ()  [unwired: 8 in, 2 out]
        n469 = call "BG4FGV.vi"("action"=w953, "BG4 in"=w954) -> ()  [unwired: 8 in, 2 out]
        n470 = call <vilib>:"Add State(s) to Queue__JKI_lib_State_Machine.vi"("State(s) in (\"\")"=w966) -> ("States Out"=w965:string)  [unwired: 14 in]
      }
      frame "Data: saveBGtoFile" {
        w988 = "Background" ("name or relative path")
        # "Save BG to file.\n(save BG to disk both data folder and temp folder)"
        n471 = Unbundle By Name(w992) -> ("Pathes.BG Path"=w985:path, "IDs.BG ID"=w984:i8, "Ch1Data"=w982:dbl[][], "V1"=w981:dbl[], "Ch2Data"=w980:dbl[][], "V2"=w979:dbl[], "Ch3Data"=w978:dbl[][], "V3"=w977:dbl[], "Ch4Data"=w969:dbl[][], "V4"=w968:dbl[], "TempPath"=w990:path)
        n472 = Increment(x=w984) -> (x+1=w989:i8)
        n473 = Format Value(string ("")=w988, format string="%02d", value (0)=w989) -> (output string=w987:string)
        n474 = Build Path(base path=w990, name or relative path=w988) -> (appended path=w971:path)
        n475 = call "File Dialog2"("start path"=w985, "prompt"="Please select BG name, DO NOT CANCEL!", "default name"=w987) -> ("selected path"=w972:path)  [unwired: 9 in, 3 out]
        n476 = Bundle("Ch1Data"=w982, "V1"=w981) -> (w976:cluster{"Ch1Data":dbl[][], "V1":dbl[]})  [unwired: 1 in]
        n477 = Bundle("Ch4Data"=w969, "V4"=w968) -> (w967:cluster{"Ch4Data":dbl[][], "V4":dbl[]})  [unwired: 1 in]
        n478 = Bundle("Ch2Data"=w980, "V2"=w979) -> (w975:cluster{"Ch2Data":dbl[][], "V2":dbl[]})  [unwired: 1 in]
        n479 = Bundle("Ch3Data"=w978, "V3"=w977) -> (w974:cluster{"Ch3Data":dbl[][], "V3":dbl[]})  [unwired: 1 in]
        n480 = Build Array(w972, w971) -> (w970:path[])
        n481 = for {
          tunnel: w976 -> [w1003]
          tunnel: w975 -> [w1002]
          tunnel: w974 -> [w1001]
          shift-right: [w1004] -> w983
          shift-left: w973 -> [w1000]
          tunnel: w970 -> [w999] mode=indexing
          tunnel: w967 -> [w997]
          n482 = call "SaveBGorCali(SubVI).vi"("Channel1"=w1003, "BG path"=w999, "DataType"=enum16{"BG", "Cali"}."BG", "Channel 2"=w1002, "Channel 3"=w1001, "Channel 4"=w997, "error in (no error)"=w1000, "SytemID"="UCDVetMed") -> ("error out"=w1004:errorcluster)  [unwired: 7 in]
        }
        n483 = call <vilib>:"Add State(s) to Queue__JKI_lib_State_Machine.vi"("State(s) in (\"\")"=w995) -> ("States Out"=w994:string)  [unwired: 14 in]
      }
      frame "Data: showBG" {
        # "Show BG in seperate window.\n()"
        n484 = call "showBG.vi"() -> ()  [unwired: 12 in]
        n485 = call <vilib>:"Add State(s) to Queue__JKI_lib_State_Machine.vi"("State(s) in (\"\")"=w1009) -> ("States Out"=w1008:string)  [unwired: 14 in]
      }
      frame "Data: irfAlignment" {
        w1010 = enum16{"write", "read"}."write" ("action")
        # "do iRF alignment in this state\n(It is a separator no-op. You can make a copy of this frame to create a new Data frame)"
        n486 = Unbundle By Name(w1055) -> ("Ch1Data"=w1091:dbl[][], "Ch2Data"=w1090:dbl[][], "Ch3Data"=w1089:dbl[][], "Ch4Data"=w1032:dbl[][])
        n487 = call "Ch1DeconEngineFGV.vi"("Error In"=w1031) -> ("Error Out"=w1087:errorcluster, "Ch1DeconEngine out"=w1088:refnum<class "LaguerreDeconEngineClass.lvclass">)  [unwired: 9 in]
        n488 = call "Ch2DeconEngineFGV.vi"("Error In"=w1031) -> ("Error Out"=w1085:errorcluster, "Ch2DeconEngine out"=w1086:refnum<class "LaguerreDeconEngineClass.lvclass">)  [unwired: 9 in]
        n489 = call "Ch3DeconEngineFGV.vi"("Error In"=w1031) -> ("Error Out"=w1083:errorcluster, "Ch3DeconEngine out"=w1084:refnum<class "LaguerreDeconEngineClass.lvclass">)  [unwired: 9 in]
        n490 = call "Ch4DeconEngineFGV.vi"("Error In"=w1031) -> ("Error Out"=w1022:errorcluster, "Ch3DeconEngine out"=w1021:refnum<class "LaguerreDeconEngineClass.lvclass">)  [unwired: 9 in]
        n491 = call "AvgArray.vi"("2D array in"=w1090) -> ("1D Avg out"=w1037:dbl[])  [unwired: 10 in]
        n492 = call "AvgArray.vi"("2D array in"=w1089) -> ("1D Avg out"=w1036:dbl[])  [unwired: 10 in]
        n493 = call "AvgArray.vi"("2D array in"=w1032) -> ("1D Avg out"=w1011:dbl[])  [unwired: 10 in]
        n494 = call "AvgArray.vi"("2D array in"=w1091) -> ("1D Avg out"=w1038:dbl[])  [unwired: 10 in]
        n495 = call "RemoveDCBG.vi"("WF in"=w1038) -> ("DC"=w1045:dbl, "WF out"=w1035:dbl[])  [unwired: 8 in, 1 out]
        n496 = call "RemoveDCBG.vi"("WF in"=w1037) -> ("DC"=w1042:dbl, "WF out"=w1048:dbl[])  [unwired: 8 in, 1 out]
        n497 = call "RemoveDCBG.vi"("WF in"=w1036) -> ("DC"=w1040:dbl, "WF out"=w1047:dbl[])  [unwired: 8 in, 1 out]
        n498 = call "RemoveDCBG.vi"("WF in"=w1011) -> ("DC"=w1015:dbl, "WF out"=w1013:dbl[])  [unwired: 8 in, 1 out]
        n499 = call "computeIRFAlignment.vi"("error in (no error)"=w1087, "fIRF temp"=w1035, "LaguerreDeconEngineClass in"=w1088) -> ("error out"=w1079:errorcluster, "LaguerreDeconEngineClass out"=w1080:refnum<class "LaguerreDeconEngineClass.lvclass">)  [unwired: 6 in, 1 out]
        n500 = call "computeIRFAlignment.vi"("error in (no error)"=w1085, "fIRF temp"=w1048, "LaguerreDeconEngineClass in"=w1086) -> ("error out"=w1077:errorcluster, "LaguerreDeconEngineClass out"=w1078:refnum<class "LaguerreDeconEngineClass.lvclass">)  [unwired: 6 in, 1 out]
        n501 = call "computeIRFAlignment.vi"("error in (no error)"=w1083, "fIRF temp"=w1047, "LaguerreDeconEngineClass in"=w1084) -> ("error out"=w1081:errorcluster, "LaguerreDeconEngineClass out"=w1082:refnum<class "LaguerreDeconEngineClass.lvclass">)  [unwired: 6 in, 1 out]
        n502 = call "computeIRFAlignment.vi"("error in (no error)"=w1022, "fIRF temp"=w1013, "LaguerreDeconEngineClass in"=w1021) -> ("error out"=w1029:errorcluster, "LaguerreDeconEngineClass out"=w1030:refnum<class "LaguerreDeconEngineClass.lvclass">)  [unwired: 6 in, 1 out]
        n503 = call "Ch1DeconEngineFGV.vi"("Error In"=w1079, "action(read)"=w1010, "Ch1DeconEngine in"=w1080) -> ("Error Out"=w1075:errorcluster, "Ch1DeconEngine out"=w1076:refnum<class "LaguerreDeconEngineClass.lvclass">)  [unwired: 7 in]
        n504 = call "Ch2DeconEngineFGV.vi"("Error In"=w1077, "action(read)"=w1010, "Ch2DeconEngine in"=w1078) -> ("Error Out"=w1065:errorcluster, "Ch2DeconEngine out"=w1066:refnum<class "LaguerreDeconEngineClass.lvclass">)  [unwired: 7 in]
        n505 = call "Ch3DeconEngineFGV.vi"("Error In"=w1081, "action(read)"=w1010, "Ch3DeconEngine in"=w1082) -> ("Error Out"=w1059:errorcluster, "Ch3DeconEngine out"=w1060:refnum<class "LaguerreDeconEngineClass.lvclass">)  [unwired: 7 in]
        n506 = call "Ch4DeconEngineFGV.vi"("Error In"=w1029, "action(read)"=w1010, "Ch3DeconEngine in"=w1030) -> ("Error Out"=w1023:errorcluster, "Ch3DeconEngine out"=w1024:refnum<class "LaguerreDeconEngineClass.lvclass">)  [unwired: 7 in]
        n507 = call "setfIRF.vi"("error in (no error)"=w1059, "fIRF"=w1047, "LaguerreDeconEngineClass in"=w1060) -> ("error out"=w1063:errorcluster, "LaguerreDeconEngineClass out"=w1064:refnum<class "LaguerreDeconEngineClass.lvclass">)  [unwired: 7 in]
        n508 = call "setfIRF.vi"("error in (no error)"=w1023, "fIRF"=w1013, "LaguerreDeconEngineClass in"=w1024) -> ("error out"=w1027:errorcluster, "LaguerreDeconEngineClass out"=w1028:refnum<class "LaguerreDeconEngineClass.lvclass">)  [unwired: 7 in]
        n509 = call "setfIRF.vi"("error in (no error)"=w1065, "fIRF"=w1048, "LaguerreDeconEngineClass in"=w1066) -> ("error out"=w1069:errorcluster, "LaguerreDeconEngineClass out"=w1070:refnum<class "LaguerreDeconEngineClass.lvclass">)  [unwired: 7 in]
        n510 = call "setfIRF.vi"("error in (no error)"=w1075, "fIRF"=w1035, "LaguerreDeconEngineClass in"=w1076) -> ("error out"=w1073:errorcluster, "LaguerreDeconEngineClass out"=w1074:refnum<class "LaguerreDeconEngineClass.lvclass">)  [unwired: 7 in]
        n511 = Unbundle By Name(w1055) -> ("V1"=w1034:dbl[], "V2"=w1054:dbl[], "V3"=w1053:dbl[], "V4"=w1020:dbl[])
        n512 = call "computeLCs.vi"("error in (no error)"=w1073, "LaguerreDeconClass in"=w1074) -> ("error out"=w1071:errorcluster, "LaguerreDeconClass out"=w1072:refnum<class "LaguerreDeconEngineClass.lvclass">)  [unwired: 8 in]
        n513 = call "computeLCs.vi"("error in (no error)"=w1069, "LaguerreDeconClass in"=w1070) -> ("error out"=w1067:errorcluster, "LaguerreDeconClass out"=w1068:refnum<class "LaguerreDeconEngineClass.lvclass">)  [unwired: 8 in]
        n514 = call "computeLCs.vi"("error in (no error)"=w1063, "LaguerreDeconClass in"=w1064) -> ("error out"=w1061:errorcluster, "LaguerreDeconClass out"=w1062:refnum<class "LaguerreDeconEngineClass.lvclass">)  [unwired: 8 in]
        n515 = call "computeLCs.vi"("error in (no error)"=w1027, "LaguerreDeconClass in"=w1028) -> ("error out"=w1025:errorcluster, "LaguerreDeconClass out"=w1026:refnum<class "LaguerreDeconEngineClass.lvclass">)  [unwired: 8 in]
        n516 = call-poly <vilib>:"Mean.vi"("X"=w1034) -> ("mean"=w1033:dbl)  [unwired: 1 out]
        n517 = call-poly <vilib>:"Mean.vi"("X"=w1020) -> ("mean"=w1019:dbl)  [unwired: 1 out]
        n518 = call-poly <vilib>:"Mean.vi"("X"=w1054) -> ("mean"=w1052:dbl)  [unwired: 1 out]
        n519 = call "getFitting.vi"("error in (no error)"=w1071, "LaguerreDeconEngineClass in"=w1072) -> ("Fitting"=w1044:dbl[])  [unwired: 7 in, 2 out]
        n520 = call "getFitting.vi"("error in (no error)"=w1067, "LaguerreDeconEngineClass in"=w1068) -> ("Fitting"=w1041:dbl[])  [unwired: 7 in, 2 out]
        n521 = call "getFitting.vi"("error in (no error)"=w1061, "LaguerreDeconEngineClass in"=w1062) -> ("Fitting"=w1017:dbl[])  [unwired: 7 in, 2 out]
        n522 = call "getFitting.vi"("error in (no error)"=w1025, "LaguerreDeconEngineClass in"=w1026) -> ("Fitting"=w1016:dbl[])  [unwired: 7 in, 2 out]
        n523 = Add(x=w1045, y=w1044) -> (x+y=w1046:dbl[])
        n524 = Add(x=w1042, y=w1041) -> (x+y=w1043:dbl[])
        n525 = call-poly <vilib>:"Mean.vi"("X"=w1053) -> ("mean"=w1051:dbl)  [unwired: 1 out]
        n526 = Add(x=w1040, y=w1017) -> (x+y=w1039:dbl[])
        n527 = Build Array(w1038, w1046) -> (w1058:dbl[][])
        n528 = Build Array(w1037, w1043) -> (w1057:dbl[][])
        n529 = Build Array(w1036, w1039) -> (w1056:dbl[][])
        n530 = Add(x=w1015, y=w1016) -> (x+y=w1014:dbl[])
        n531 = Bundle("mean"=w1033, "mean"=w1052, "mean"=w1051, "mean"=w1019) -> (w1018:T39)  [unwired: 1 in]
        n532 = Build Array(w1011, w1014) -> (w1012:dbl[][])
        n533 = call "Calib_and_iRFAlign_confirm.vi"("Current V"=w1018, "Ch4 Data"=w1012, "Ch3 Data"=w1056, "Ch2 Data"=w1057, "Ch1 Data"=w1058) -> ("Save?"=w1050:bool)  [unwired: 6 in]
        n534 = case shown="True" w1050 {
          tunnel: ["" ("Empty String Constant") "Data: saveCalibration\nData: saveiRF\nRun: CaliIncrement"] -> w1049
          frame False {
          }
          frame True {
            # "[Covers: REQ2]"
          }
        }
        n535 = call <vilib>:"Add State(s) to Queue__JKI_lib_State_Machine.vi"("State(s) in Front (\"\")"=w1049, "State(s) in (\"\")"=w1094) -> ("States Out"=w1093:string)  [unwired: 13 in]
      }
      frame "Data: parseRunData" {
        # "All APD bias"
        # "flash queue"
        # "Ch3&4"
        # "Ch1&2"
        # "Flash data from queue and save it in structure\n()"
        n536 = Flush Queue(queue=w1122, error in (no error)=w1121) -> (remaining elements=w1116:T40, error out=w1117:errorcluster)  [unwired: 1 out]
        n537 = Flush Queue(queue=w1127, error in (no error)=w1121) -> (remaining elements=w1125:cluster{"double data":dbl[][]}[], error out=w1118:errorcluster)  [unwired: 1 out]
        n538 = Flush Queue(queue=w1128, error in (no error)=w1121) -> (remaining elements=w1126:cluster{"double data":dbl[][]}[], error out=w1119:errorcluster)  [unwired: 1 out]
        n539 = for {
          tunnel: w1126 -> [w1144] mode=indexing
          tunnel: [w1142] -> w1111 mode=concatenating
          tunnel: [w1141] -> w1112 mode=concatenating
          n540 = Unbundle By Name(w1144) -> ("double data"=w1143:dbl[][])
          n541 = call "SeperateChanData.vi"("Input (Ch1&2)"=w1143) -> ("Ch1"=w1142:dbl[][], "Ch2"=w1141:dbl[][])
        }
        n542 = for {
          tunnel: w1125 -> [w1140] mode=indexing
          tunnel: [w1139] -> w1101 mode=concatenating
          tunnel: [w1137] -> w1102 mode=concatenating
          n543 = Unbundle By Name(w1140) -> ("double data"=w1138:dbl[][])
          n544 = call "SeperateChanData.vi"("Input (Ch1&2)"=w1138) -> ("Ch1"=w1139:dbl[][], "Ch2"=w1137:dbl[][])
        }
        n545 = call "FLImDAQ_FGV.vi"() -> ("Read data"=w1109:T5)  [unwired: 10 in, 1 out]
        n546 = Unbundle By Name(w1109) -> ("Waveform to Avg"=w1099:i16)
        n547 = for {
          tunnel: w1116 -> [w1136] mode=indexing
          tunnel: [w1135] -> w1108 mode=indexing
          tunnel: [w1134] -> w1106 mode=indexing
          tunnel: [w1133] -> w1104 mode=indexing
          tunnel: [w1132] -> w1100 mode=indexing
          n548 = Unbundle By Name(w1136) -> ("V1"=w1135:dbl, "V2"=w1134:dbl, "V3"=w1133:dbl, "V4"=w1132:dbl)
        }
        n549 = call "DuplicateV(SubVI).vi"("Averaging"=w1099, "V in"=w1108) -> ("V out"=w1107:dbl[])  [unwired: 9 in]
        n550 = Array Size(array=w1101) -> (size(s)=→"data Size":i32[])
        n551 = call "DuplicateV(SubVI).vi"("Averaging"=w1099, "V in"=w1106) -> ("V out"=w1105:dbl[])  [unwired: 9 in]
        n552 = call "DuplicateV(SubVI).vi"("Averaging"=w1099, "V in"=w1104) -> ("V out"=w1103:dbl[])  [unwired: 9 in]
        n553 = call "DuplicateV(SubVI).vi"("Averaging"=w1099, "V in"=w1100) -> ("V out"=w1097:dbl[])  [unwired: 9 in]
        n554 = Bundle By Name(cluster=w1123, "Ch1Data"=w1111, "Ch2Data"=w1112, "Ch3Data"=w1101, "Ch4Data"=w1102, "V1"=w1107, "V2"=w1105, "V3"=w1103, "V4"=w1097) -> (w1124:T26)
        n555 = Merge Errors(w1119, w1118, w1117) -> (w1120:errorcluster)
        n556 = Array Size(array=w1107) -> (size(s)=→"V1 Size":i32)
        n557 = Array Size(array=w1105) -> (size(s)=→"V2 Size":i32)
        n558 = Array Size(array=w1103) -> (size(s)=→"V3 Size":i32)
        n559 = Array Size(array=w1097) -> (size(s)=→"V4 Size":i32)
        n560 = call <vilib>:"Add State(s) to Queue__JKI_lib_State_Machine.vi"("State(s) in (\"\")"=w1131) -> ("States Out"=w1130:string)  [unwired: 14 in]
      }
      frame "Data: saveRunData" {
        w1147 = T41 {"DataPath"=path "", "CaseID"="", "RunID"=0, "Ch1Data"=[], "Ch2Data"=[], "Ch3Data"=[], "Ch4Data"=[], "V1"=[], "V2"=[], "V3"=[], "V4"=[], "LaserRepRate"=0, "WFAverage"=0, "RunStartTime"=0}  # Data cluster
        # "Save FLIm data to disk.\n(Save to LV tdms file format)"
        n561 = Unbundle By Name(w1158) -> ("Pathes.DataPath"=w1154:path, "CaseID"=w1166:string, "IDs.RunID"=w1156:i8, "Ch1Data"=w1165:dbl[][], "Ch2Data"=w1164:dbl[][], "Ch3Data"=w1153:dbl[][], "Ch4Data"=w1146:dbl[][], "V1"=w1148:dbl[], "V2"=w1163:dbl[], "V3"=w1162:dbl[], "V4"=w1145:dbl[])
        n562 = call "FLImDAQ_FGV.vi"() -> ("Read data"=w1151:T5)  [unwired: 10 in, 1 out]
        n563 = Unbundle By Name(w1151) -> ("Waveform to Avg"=w1150:i16)
        n564 = local read "RunStartTime"() -> (w1149:u32)
        n565 = local read "Laser Rep Rate"() -> (w1152:dbl)
        n566 = Increment(x=w1156) -> (x+1=w1155:i8)
        n567 = Bundle By Name(cluster=w1147, "DataPath"=w1154, "CaseID"=w1166, "RunID"=w1155, "Ch1Data"=w1165, "Ch2Data"=w1164, "Ch3Data"=w1153, "Ch4Data"=w1146, "V1"=w1148, "V2"=w1163, "V3"=w1162, "V4"=w1145, "LaserRepRate"=w1152, "WFAverage"=w1150, "RunStartTime"=w1149) -> (w1161:T41)
        n568 = call "SaveRunData(SubVI).vi"("Data cluster"=w1161, "error in (no error)"=w1160) -> ("error out"=w1157:errorcluster)  [unwired: 13 in]
        n569 = flat-sequence {
          tunnel: w1158 -> [w1174]
          tunnel: [w1173] -> w1159
          tunnel: w1157 -> [_]
          frame #0 {
            w1171 = dbl[][] [] ("Ch1Data")
            w1172 = dbl[] [] ("V1")
            # "reset local data"
            n570 = Bundle By Name(cluster=w1174, "Ch1Data"=w1171, "Ch2Data"=w1171, "Ch3Data"=w1171, "Ch4Data"=w1171, "V1"=w1172, "V2"=w1172, "V3"=w1172, "V4"=w1172) -> (w1173:T26)
          }
        }
        n571 = case shown="No Error" w1157 {
          tunnel: ["Run: Increment" "" ("Empty String Constant")] -> w1167
          frame No Error {
          }
          frame Error {
          }
        }
        n572 = call <vilib>:"Add State(s) to Queue__JKI_lib_State_Machine.vi"("State(s) in Front (\"\")"=w1167, "State(s) in (\"\")"=w1170) -> ("States Out"=w1169:string)  [unwired: 13 in]
      }
      frame "Data: Cleanup" {
        # "Cleanup any data and references, here.\n(this is called automatically, by the Macro: Exit)"
        n573 = Unbundle By Name(w1178) -> ("Core.Current VI Reference"=w1181:refnum<vi>)
        n574 = Close Reference(reference=w1181, error in (no error)=w1180) -> (error out=w1179:errorcluster)
        n575 = call <vilib>:"Add State(s) to Queue__JKI_lib_State_Machine.vi"("State(s) in (\"\")"=w1183) -> ("States Out"=w1182:string)  [unwired: 14 in]
      }
      frame "---------- Core ----------" {
        # "Do not put any code in this frame.\n(it is a separator no-op)"
        n576 = call <vilib>:"Add State(s) to Queue__JKI_lib_State_Machine.vi"("State(s) in (\"\")"=w1188) -> ("States Out"=w1187:string)  [unwired: 14 in]
      }
      frame Default {
        w1199 = 42 items=["No error", "Argument error", "Memory is full", "Out of zone", "End of file", "File already open", "Generic file I/O error", "File not found", "File permission error", "Disk is full", "Duplicate path", "Too many files open", "System feature not enabled", "Resource file not found", "Cannot add resource", "Resource not found", "Image not found", "Image memory error", "Pen does not exist", "Config type invalid", "Config token not found", "Config parse error", "Config memory error", "Bad external code format", "Bad external code offset", "External code not present", "Null window", "Destroy window error", "Null menu", "Print aborted", "Bad print record", "Print driver error", "Windows error during printing", "Memory error during printing", "Print dialog error", "Generic print error", "Invalid device refnum", "Device not found", "Device parameter error", "Device unit error", "Cannot open device", "Device call aborted", "Generic error", "Cancelled by user", "Object ID too low", "Object ID too high", "Object not in heap", "Unknown heap", "Unknown object (invalid DefProc)", "Unknown object (DefProc not in table)", "Message out of range", "Invalid (null) method", "Unknown message", "Manager call not supported", "Bad address", "Network operation in progress", "Network operation timed out", "Connection is busy", "Network attribute not supported", "Network error", "Address in use", "System out of memory", "Connection aborted", "Connection refused", "Not connected", "Already connected", "Connection closed", "Initialization error (interapplication manager)", "Bad occurrence", "Wait on unbound occurrence handler", "Occurrence queue overflow", "Datalog type conflict", "Unused", "Unrecognized type (interapplication manager)", "Memory corrupt", "Failed to make temporary DLL", "Old CIN version", "Drag socket not found", "Failed to load drop-object", "Failed to register OLE object", "Failed to release OLE object", "Format specifier type mismatch", "Unknown format specifier", "Too few format specifiers", "Too many format specifiers", "Scan failed", "Newer CIN version", "Error converting to variant", "Runtime menu error", "Password tampered", "Variant attribute not found", "Incompatible variant data type", "Event data is not available", "Event Store is not present", "Occurrence is not found", "Event Queue is not created", "Event info is not available", "Refnum passed is NULL", "Error retrieving Class GUID", "Error retrieving CoClass GUID", "Error retrieving TypeLib GUID.", "Bad built application magic bytes.", "Specific driver is different from the specific driver associated with the Logical Name.", "There is no session opened to the class driver.", "Max Error", "MAX - Error with config objects", "MAX - Error loading configuration", "MAX - Group not supported"]
        # "Current State"
        # "Do not delete, rename, or modify this frame.\n(this is used to capture unhandled states and typos)"
        # "Handle mistyped state name (developer tool)"
        n577 = Format Into String(format string="Software Exception: Unhandled State \"%s\"." ("message"), error in=w1195, w1190) -> (resulting string=w1198:string, error out=w1197:errorcluster)  [unwired: 1 in]
        n578 = call <vilib>:"Error Cluster From Error Code.vi"("show call chain? (False)"=TRUE, "error in (no error)"=w1197, "error message (\"\")"=w1198, "error code (0)"=w1199) -> ("error out"=w1196:errorcluster)  [unwired: 5 in]
        n579 = call <vilib>:"Add State(s) to Queue__JKI_lib_State_Machine.vi"("State(s) in (\"\")"=w1194) -> ("States Out"=w1193:string)  [unwired: 14 in]
      }
      frame "Initialize Core Data" {
        # "Build default path based on the location of project"
        # "Do not delete, rename, or modify this frame.\n(this is used to determine panel behavior on exit)"
        # "originally closed?"
        # "exe?"
        # "If panel starts closed or is an EXE, then close it when we exit"
        n580 = call <vilib>:"Application Directory.vi"() -> ("Application Directory"=w1202:path)
        n581 = property on="Property Node" class="App"() -> ("App.Kind"=w1218:T22)  [unwired: 2 in, 2 out]
        n582 = property on="Property Node" class="VI"() -> ("FP.State"=w1212:T21)  [unwired: 2 in, 2 out]
        n583 = control-ref of="Current VI Reference"() -> (w1213:refnum<vi>)
        n584 = Equal?(x=w1212, y=T21."Closed" ("Front Panel Window:State")) -> (x = y?=w1210:bool)
        n585 = Strip Path(path=w1202) -> (stripped path=w1201:path)  [unwired: 1 out]
        n586 = Equal?(x=w1218, y=T22."Run Time System" ("Application:Kind")) -> (x = y?=w1216:bool)
        n587 = Build Path(base path=w1201, name or relative path="Data") -> (appended path=w1208:path)
        n588 = Build Path(base path=w1202, name or relative path="SystemTemp") -> (appended path=w1205:path)
        n589 = Build Path(base path=w1202, name or relative path="SystemCalibrationFile") -> (appended path=w1203:path)
        n590 = Or(x=w1210, y=w1216) -> (x .or. y?=w1214:bool)
        n591 = Bundle By Name(cluster=w1215, "Core.Current VI Reference"=w1213, "Core.Close Panel on Exit?"=w1214, "DefaultPath"=w1208, "TempPath"=w1205, "CaliPath"=w1203) -> (w1220:T26)
        n592 = call <vilib>:"Add State(s) to Queue__JKI_lib_State_Machine.vi"("State(s) in (\"\")"=w1222) -> ("States Out"=w1221:string)  [unwired: 14 in]
      }
      frame "Error Handler" {
        # "Unhandled Error -- Display it"
        # "Handle any errors here.\nYou can also output any states to clean-up after errors occur"
        # "Clear error"
        n593 = Unbundle By Name(w1223) -> ("code"=w1225:i32)
        n594 = case shown="Default" w1225 {
          tunnel: ["Macro: Exit" w1235 w1241] -> w1224
          tunnel: w1223 -> [w1231 _ _]
          frame Default {
            w1233 = T42 1 items=["no dialog", "OK message", "continue or stop message", "OK message + warnings", "continue/stop + warnings"] ("type of dialog (OK msg:1)")
            n595 = call <vilib>:"General Error Handler.vi"("type of dialog (OK msg:1)"=w1233, "error in (no error)"=w1231) -> ()  [unwired: 9 in, 5 out]
          }
          frame 5002 {
            n596 = Two Button Dialog(message="Laser interlock open! Please close interlock and try again! ", 1:"Safely Shutdown" ("F button name (\"Cancel\")"), 2:"OK" ("T button name (\"OK\")")) -> (T button?=w1236:bool)
            n597 = case shown="True" w1236 {
              tunnel: ["Macro: Exit" "355 Laser: CheckControllerStatus"] -> w1235
              frame False {
              }
              frame True {
              }
            }
          }
          frame 5001 {
            n598 = Two Button Dialog(message="Unable to connect to imaging computer, do you want to run data aquisiton alone? ", 1:"No" ("F button name (\"Cancel\")"), 2:"Yes" ("T button name (\"OK\")")) -> (T button?=w1242:bool)
            n599 = case shown="False" w1242 {
              tunnel: ["Macro: Exit" "" ("Empty String Constant")] -> w1241
              frame False {
              }
              frame True {
              }
            }
          }
        }
        n600 = call <vilib>:"Add State(s) to Queue__JKI_lib_State_Machine.vi"("State(s) in Front (\"\")"=w1224, "State(s) in (\"\")"=w1230) -> ("States Out"=w1229:string)  [unwired: 13 in]
      }
      frame "Exit" {
        # "Do not put any code in this frame.\n(No errors that occur here will be handled.)"
        n601 = call <vilib>:"Add State(s) to Queue__JKI_lib_State_Machine.vi"("State(s) in (\"\")"=w1253) -> ("States Out"=w1252:string)  [unwired: 14 in]
      }
      frame "---------- Case ----------" {
        # "Template Separator\n(You can make a copy of, or modify, this frame)"
        n602 = call <vilib>:"Add State(s) to Queue__JKI_lib_State_Machine.vi"("State(s) in (\"\")"=w1258) -> ("States Out"=w1257:string)  [unwired: 14 in]
      }
      frame "Case: getCaliID" {
        # "Get Calibration file #\n(You can make a copy of, or modify, this frame)"
        n603 = Unbundle By Name(w1259) -> ("Pathes.CaliPath"=w1262:path)
        n604 = call <vilib>:"Recursive File List.vi"("pattern"="*.tdms", "Treat LLBs as Folders?"=FALSE, "Folder Path"=w1262) -> ("All Files in Dir"=w1267:path[])  [unwired: 4 in, 4 out]
        n605 = for {
          tunnel: w1267 -> [w1277] mode=indexing
          tunnel: [w1276] -> w1266 mode=indexing
          tunnel: "Calibration" -> [w1273]
          n606 = Strip Path(path=w1277) -> (name=w1274:string)  [unwired: 1 out]
          n607 = Search and Replace String(input string=w1274, search string=w1273) -> (result string=w1272:string)  [unwired: 6 in, 3 out]
          n608 = Scan From String(format string="%d" ("string"), input string=w1272) -> (output 1=w1276:i32)  [unwired: 3 in, 3 out]
        }
        n609 = Array Max & Min(array=w1266) -> (max value=w1265:i32)  [unwired: 3 out]
        n610 = Bundle By Name(cluster=w1259, "IDs.Cali ID"=w1265) -> (w1260:T26)
        n611 = call <vilib>:"Add State(s) to Queue__JKI_lib_State_Machine.vi"("State(s) in (\"\")"=w1271) -> ("States Out"=w1270:string)  [unwired: 14 in]
      }
      frame "Case: getBGID" {
        # "Get background #\n(You can make a copy of, or modify, this frame)"
        n612 = Unbundle By Name(w1280) -> ("Pathes.BG Path"=w1285:path)
        n613 = call <vilib>:"Recursive File List.vi"("pattern"="*.tdms", "Treat LLBs as Folders?"=FALSE, "Folder Path"=w1285) -> ("All Files in Dir"=w1283:path[])  [unwired: 4 in, 4 out]
        n614 = for {
          tunnel: w1283 -> [w1300] mode=indexing
          tunnel: "Background" ("name or relative path") -> [w1298]
          shift-right: [w1291] -> w1278
          shift-left: 0 -> [w1295]
          n615 = Strip Path(path=w1300) -> (name=w1299:string)  [unwired: 1 out]
          n616 = Search and Replace String(input string=w1299, search string=w1298) -> (number of replacements=w1297:i32)  [unwired: 6 in, 3 out]
          n617 = Greater Than 0?(x=w1297) -> (x > 0?=w1296:bool)
          n618 = Select(t=1, s=w1296, f=0) -> (s? t:f=w1294:i32)
          n619 = Add(x=w1294, y=w1295) -> (x+y=w1291:i32)
        }
        n620 = Bundle By Name(cluster=w1280, "IDs.BG ID"=w1278) -> (w1281:T26)
        n621 = call <vilib>:"Add State(s) to Queue__JKI_lib_State_Machine.vi"("State(s) in (\"\")"=w1290) -> ("States Out"=w1289:string)  [unwired: 14 in]
      }
      frame "Case: getRunID" {
        # "Check folder for run ID\n(You can make a copy of, or modify, this frame)"
        n622 = Unbundle By Name(w1310) -> ("Pathes.DataPath"=w1309:path, "CaseID"=w1305:string)
        n623 = Build Array("Background" ("name or relative path"), "Calibration", "3DScanData" ("element")) -> (w1315:string[])
        n624 = call <vilib>:"Recursive File List.vi"("Folders to Exclude"=w1315, "pattern"="*.tdms", "Treat LLBs as Folders?"=FALSE, "Folder Path"=w1309) -> ("All Files in Dir"=w1306:path[])  [unwired: 3 in, 4 out]
        n625 = for {
          tunnel: w1306 -> [w1324] mode=indexing
          tunnel: [w1323] -> w1312 mode=indexing
          tunnel: w1305 -> [w1320]
          n626 = Strip Path(path=w1324) -> (name=w1321:string)  [unwired: 1 out]
          n627 = Search and Replace String(input string=w1321, search string=w1320) -> (result string=w1319:string)  [unwired: 6 in, 3 out]
          n628 = Scan From String(format string="_%d" ("string"), input string=w1319) -> (output 1=w1323:i32)  [unwired: 3 in, 3 out]
        }
        n629 = Array Max & Min(array=w1312) -> (max value=w1303:i32)  [unwired: 3 out]
        n630 = Bundle By Name(cluster=w1310, "IDs.RunID"=w1303) -> (w1311:T26)
        n631 = call "RunIDFGV.vi"("Error In"=w1301, "RunID in"=w1303) -> ("Error Out"=w1302:errorcluster)  [unwired: 8 in, 1 out]
        n632 = call <vilib>:"Add State(s) to Queue__JKI_lib_State_Machine.vi"("State(s) in (\"\")"=w1318) -> ("States Out"=w1317:string)  [unwired: 14 in]
      }
      frame "Case: CreatFileStruct" {
        # "Creat case file structure"
        n633 = Unbundle By Name(w1338) -> ("DefaultPath"=w1344:path, "CaseID"=w1331:string)
        n634 = Build Path(base path=w1344, name or relative path=w1331) -> (appended path=w1343:path)
        n635 = call <vilib>:"Check if File or Folder Exists.vi"("error in (no error)"=w1337, "path"=w1343) -> ("error out"=w1340:errorcluster, "file or folder exists?"=w1342:bool, "dup path"=w1341:path)  [unwired: 7 in]
        n636 = case shown="True" w1342 {
          tunnel: w1341 -> [w1361 w1369]
          tunnel: w1340 -> [w1359 w1364]
          tunnel: [w1353 w1369] -> w1329
          tunnel: [w1357 w1371] -> w1328
          tunnel: [u32 0 u32 0] -> w1327
          tunnel: [w1355 w1374] -> w1335
          tunnel: "Background" ("name or relative path") -> [w1354 w1366]
          tunnel: "Calibration" -> [w1352 w1365]
          tunnel: [w1348 w1367] -> w1332
          tunnel: w1331 -> [_ _]
          tunnel: ["" ("Empty String Constant") "Case: getRunID\nCase: getBGID\nCase: getCaliID\nUI: Update"] -> w1330
          frame False {
            # "Folder not exist. Creat folders."
            n637 = Create Folder(path (use dialog)=w1361, error in=w1359) -> (created path=w1353:path, error out=w1350:errorcluster)  [unwired: 1 in, 1 out]
            n638 = Build Path(base path=w1353, name or relative path=w1352) -> (appended path=w1351:path)
            n639 = Build Path(base path=w1353, name or relative path=w1354) -> (appended path=w1360:path)
            n640 = Create Folder(path (use dialog)=w1360, error in=w1350) -> (created path=w1355:path, error out=w1356:errorcluster)  [unwired: 1 in, 1 out]
            n641 = Create Folder(path (use dialog)=w1351, error in=w1350) -> (created path=w1348:path, error out=w1349:errorcluster)  [unwired: 1 in, 1 out]
            n642 = Merge Errors(w1356, w1349) -> (w1357:errorcluster)
          }
          frame True {
            # "Folder exsit, check file #"
            n643 = Build Path(base path=w1369, name or relative path=w1365) -> (appended path=w1370:path)
            n644 = Build Path(base path=w1369, name or relative path=w1366) -> (appended path=w1375:path)
            n645 = call <vilib>:"Check if File or Folder Exists.vi"("path"=w1370) -> ("file or folder exists?"=w1368:bool, "dup path"=w1367:path)  [unwired: 8 in, 1 out]
            n646 = call <vilib>:"Check if File or Folder Exists.vi"("path"=w1375) -> ("file or folder exists?"=w1373:bool, "dup path"=w1374:path)  [unwired: 8 in, 1 out]
            n647 = And(x=w1373, y=w1368) -> (x .and. y?=w1372:bool)
            n648 = case shown="False" w1372 {
              tunnel: w1364 -> [_ w1377]
              tunnel: [errorcluster {"status"=TRUE, "code"=5003, "source"="File structure error."} ("error out") w1377] -> w1371
              frame False {
              }
              frame True {
              }
            }
          }
        }
        n649 = Bundle By Name(cluster=w1338, "Pathes.DataPath"=w1329, "Pathes.BG Path"=w1335, "Pathes.CaliPath"=w1332, "IDs.RunID"=w1327, "IDs.BG ID"=w1327, "IDs.Cali ID"=w1327) -> (w1339:T26)
        n650 = call "DataRootPathFGV.vi"("Error In"=w1328, "PathIn"=w1329) -> ("Error Out"=w1326:errorcluster)  [unwired: 8 in, 1 out]
        n651 = call "RunIDFGV.vi"("Error In"=w1326, "RunID in"=w1327) -> ("Error Out"=w1325:errorcluster)  [unwired: 8 in, 1 out]
        n652 = call <vilib>:"Add State(s) to Queue__JKI_lib_State_Machine.vi"("State(s) in Front (\"\")"=w1330, "State(s) in (\"\")"=w1346) -> ("States Out"=w1345:string)  [unwired: 13 in]
      }
      frame "Case: GetID" {
        # "Template Separator\n(You can make a copy of, or modify, this frame)"
        n653 = call "set_subjectID.vi"() -> ("subject_id"=w1378:string)  [unwired: 10 in]
        n654 = Bundle By Name(cluster=w1380, "CaseID"=w1378) -> (w1381:T26)
        n655 = call <vilib>:"Add State(s) to Queue__JKI_lib_State_Machine.vi"("State(s) in (\"\")"=w1384) -> ("States Out"=w1383:string)  [unwired: 14 in]
      }
      frame "---------- DeconEngine ----------" {
        # "start data aquisition and then set irfAligh to ture and decon channel to 1,2 and 3."
        # "Template Separator\n(You can make a copy of, or modify, this frame)"
        n656 = call <vilib>:"Add State(s) to Queue__JKI_lib_State_Machine.vi"("State(s) in (\"\")"=w1389) -> ("States Out"=w1388:string)  [unwired: 14 in]
      }
      frame "DeconEngine: InitilizeMacro" {
        # "start data aquisition and then set irfAligh to ture and decon channel to 1,2 and 3."
        # "Initilize Decon Engine for all channel\n(You can make a copy of, or modify, this frame)"
        n657 = call <vilib>:"Add State(s) to Queue__JKI_lib_State_Machine.vi"("State(s) in Front (\"\")"="DeconEngine: InitializeCh1\nDeconEngine: InitializeCh2\nDeconEngine: InitializeCh3\nDeconEngine: InitializeCh4" ("State(s) in Front (\"\")"), "State(s) in (\"\")"=w1395) -> ("States Out"=w1394:string)  [unwired: 13 in]
      }
      frame "DeconEngine: InitializeCh1" {
        w1417 = refnum<class "LaguerreDeconEngineClass.lvclass"> refnum  # Ch1DeconObj
        # "Initilize Laguerre Deconvolution engine Object\n(You can make a copy of, or modify, this frame)"
        n658 = global read "GlobalVariables.vi" "LastUseiRF"() -> (w1398:T19)
        n659 = local read "Truncation"() -> (w1396:u32)
        n660 = call "setLaguerreOrder.vi"("error in (no error)"=w1405, "LaguerreOrder"=u32 12, "LaguerreDeconClass in"=w1417) -> ("error out"=w1414:errorcluster, "LaguerreDeconClass out"=w1415:refnum<class "LaguerreDeconEngineClass.lvclass">)  [unwired: 7 in]
        n661 = Unbundle By Name(w1398) -> ("Ch1 iRF"=w1397:dbl[])
        n662 = call "setDataLength.vi"("error in (no error)"=w1414, "dataLength"=w1396, "LaguerreDeconClass in"=w1415) -> ("error out"=w1413:errorcluster, "LaguerreDeconClass out"=w1412:refnum<class "LaguerreDeconEngineClass.lvclass">)  [unwired: 7 in]
        n663 = call "setIRF.vi"("error in (no error)"=w1413, "iRF"=w1397, "LaguerreDeconClass in"=w1412) -> ("error out"=w1410:errorcluster, "LaguerreDeconClass out"=w1411:refnum<class "LaguerreDeconEngineClass.lvclass">)  [unwired: 7 in]
        n664 = call "computeAlpha.vi"("error in (no error)"=w1410, "LaguerreDeconClass in"=w1411) -> ("error out"=w1408:errorcluster, "LaguerreDeconClass out"=w1409:refnum<class "LaguerreDeconEngineClass.lvclass">)  [unwired: 8 in]
        n665 = call "dataInitilize.vi"("error in (no error)"=w1408, "LaguerreDeconClass in"=w1409) -> ("error out"=w1406:errorcluster, "LaguerreDeconClass out"=w1407:refnum<class "LaguerreDeconEngineClass.lvclass">)  [unwired: 8 in]
        n666 = call "computeDeconMatrix.vi"("error in (no error)"=w1406, "LaguerreDeconClass in"=w1407) -> ("error out"=w1402:errorcluster, "LaguerreDeconClass out"=w1404:refnum<class "LaguerreDeconEngineClass.lvclass">)  [unwired: 8 in]
        n667 = call "Ch1DeconEngineFGV.vi"("Error In"=w1402, "action(read)"=enum16{"write", "read"}."write" ("action"), "Ch1DeconEngine in"=w1404) -> ("Error Out"=w1401:errorcluster)  [unwired: 7 in, 1 out]
        n668 = call <vilib>:"Add State(s) to Queue__JKI_lib_State_Machine.vi"("State(s) in (\"\")"=w1419) -> ("States Out"=w1418:string)  [unwired: 14 in]
      }
      frame "DeconEngine: InitializeCh2" {
        w1441 = refnum<class "LaguerreDeconEngineClass.lvclass"> refnum  # Ch2DeconObj
        # "Initilize Laguerre Deconvolution engine Object\n(You can make a copy of, or modify, this frame)"
        n669 = global read "GlobalVariables.vi" "LastUseiRF"() -> (w1422:T19)
        n670 = call "setLaguerreOrder.vi"("error in (no error)"=w1429, "LaguerreOrder"=u32 12, "LaguerreDeconClass in"=w1441) -> ("error out"=w1438:errorcluster, "LaguerreDeconClass out"=w1439:refnum<class "LaguerreDeconEngineClass.lvclass">)  [unwired: 7 in]
        n671 = local read "Truncation"() -> (w1420:u32)
        n672 = Unbundle By Name(w1422) -> ("Ch2 iRF"=w1421:dbl[])
        n673 = call "setDataLength.vi"("error in (no error)"=w1438, "dataLength"=w1420, "LaguerreDeconClass in"=w1439) -> ("error out"=w1437:errorcluster, "LaguerreDeconClass out"=w1436:refnum<class "LaguerreDeconEngineClass.lvclass">)  [unwired: 7 in]
        n674 = call "setIRF.vi"("error in (no error)"=w1437, "iRF"=w1421, "LaguerreDeconClass in"=w1436) -> ("error out"=w1434:errorcluster, "LaguerreDeconClass out"=w1435:refnum<class "LaguerreDeconEngineClass.lvclass">)  [unwired: 7 in]
        n675 = call "computeAlpha.vi"("error in (no error)"=w1434, "LaguerreDeconClass in"=w1435) -> ("error out"=w1432:errorcluster, "LaguerreDeconClass out"=w1433:refnum<class "LaguerreDeconEngineClass.lvclass">)  [unwired: 8 in]
        n676 = call "dataInitilize.vi"("error in (no error)"=w1432, "LaguerreDeconClass in"=w1433) -> ("error out"=w1430:errorcluster, "LaguerreDeconClass out"=w1431:refnum<class "LaguerreDeconEngineClass.lvclass">)  [unwired: 8 in]
        n677 = call "computeDeconMatrix.vi"("error in (no error)"=w1430, "LaguerreDeconClass in"=w1431) -> ("error out"=w1426:errorcluster, "LaguerreDeconClass out"=w1428:refnum<class "LaguerreDeconEngineClass.lvclass">)  [unwired: 8 in]
        n678 = call "Ch2DeconEngineFGV.vi"("Error In"=w1426, "action(read)"=enum16{"write", "read"}."write" ("action"), "Ch2DeconEngine in"=w1428) -> ("Error Out"=w1425:errorcluster)  [unwired: 7 in, 1 out]
        n679 = call <vilib>:"Add State(s) to Queue__JKI_lib_State_Machine.vi"("State(s) in (\"\")"=w1443) -> ("States Out"=w1442:string)  [unwired: 14 in]
      }
      frame "DeconEngine: InitializeCh3" {
        w1445 = refnum<class "LaguerreDeconEngineClass.lvclass"> refnum  # Ch3DeconObj
        # "Initilize Laguerre Deconvolution engine Object\n(You can make a copy of, or modify, this frame)"
        n680 = global read "GlobalVariables.vi" "LastUseiRF"() -> (w1447:T19)
        n681 = local read "Truncation"() -> (w1444:u32)
        n682 = call "setLaguerreOrder.vi"("error in (no error)"=w1454, "LaguerreOrder"=u32 12, "LaguerreDeconClass in"=w1445) -> ("error out"=w1463:errorcluster, "LaguerreDeconClass out"=w1464:refnum<class "LaguerreDeconEngineClass.lvclass">)  [unwired: 7 in]
        n683 = Unbundle By Name(w1447) -> ("Ch3 iRF"=w1446:dbl[])
        n684 = call "setDataLength.vi"("error in (no error)"=w1463, "dataLength"=w1444, "LaguerreDeconClass in"=w1464) -> ("error out"=w1462:errorcluster, "LaguerreDeconClass out"=w1461:refnum<class "LaguerreDeconEngineClass.lvclass">)  [unwired: 7 in]
        n685 = call "setIRF.vi"("error in (no error)"=w1462, "iRF"=w1446, "LaguerreDeconClass in"=w1461) -> ("error out"=w1459:errorcluster, "LaguerreDeconClass out"=w1460:refnum<class "LaguerreDeconEngineClass.lvclass">)  [unwired: 7 in]
        n686 = call "computeAlpha.vi"("error in (no error)"=w1459, "LaguerreDeconClass in"=w1460) -> ("error out"=w1457:errorcluster, "LaguerreDeconClass out"=w1458:refnum<class "LaguerreDeconEngineClass.lvclass">)  [unwired: 8 in]
        n687 = call "dataInitilize.vi"("error in (no error)"=w1457, "LaguerreDeconClass in"=w1458) -> ("error out"=w1455:errorcluster, "LaguerreDeconClass out"=w1456:refnum<class "LaguerreDeconEngineClass.lvclass">)  [unwired: 8 in]
        n688 = call "computeDeconMatrix.vi"("error in (no error)"=w1455, "LaguerreDeconClass in"=w1456) -> ("error out"=w1451:errorcluster, "LaguerreDeconClass out"=w1453:refnum<class "LaguerreDeconEngineClass.lvclass">)  [unwired: 8 in]
        n689 = call "Ch3DeconEngineFGV.vi"("Error In"=w1451, "action(read)"=enum16{"write", "read"}."write" ("action"), "Ch3DeconEngine in"=w1453) -> ("Error Out"=w1450:errorcluster)  [unwired: 7 in, 1 out]
        n690 = call <vilib>:"Add State(s) to Queue__JKI_lib_State_Machine.vi"("State(s) in (\"\")"=w1467) -> ("States Out"=w1466:string)  [unwired: 14 in]
      }
      frame "DeconEngine: InitializeCh4" {
        w1469 = refnum<class "LaguerreDeconEngineClass.lvclass"> refnum  # Ch3DeconObj
        # "Initilize Laguerre Deconvolution engine Object\n(You can make a copy of, or modify, this frame)"
        n691 = global read "GlobalVariables.vi" "LastUseiRF"() -> (w1471:T19)
        n692 = local read "Truncation"() -> (w1468:u32)
        n693 = call "setLaguerreOrder.vi"("error in (no error)"=w1478, "LaguerreOrder"=u32 12, "LaguerreDeconClass in"=w1469) -> ("error out"=w1487:errorcluster, "LaguerreDeconClass out"=w1488:refnum<class "LaguerreDeconEngineClass.lvclass">)  [unwired: 7 in]
        n694 = Unbundle By Name(w1471) -> ("Ch4 iRF"=w1470:dbl[])
        n695 = call "setDataLength.vi"("error in (no error)"=w1487, "dataLength"=w1468, "LaguerreDeconClass in"=w1488) -> ("error out"=w1486:errorcluster, "LaguerreDeconClass out"=w1485:refnum<class "LaguerreDeconEngineClass.lvclass">)  [unwired: 7 in]
        n696 = call "setIRF.vi"("error in (no error)"=w1486, "iRF"=w1470, "LaguerreDeconClass in"=w1485) -> ("error out"=w1483:errorcluster, "LaguerreDeconClass out"=w1484:refnum<class "LaguerreDeconEngineClass.lvclass">)  [unwired: 7 in]
        n697 = call "computeAlpha.vi"("error in (no error)"=w1483, "LaguerreDeconClass in"=w1484) -> ("error out"=w1481:errorcluster, "LaguerreDeconClass out"=w1482:refnum<class "LaguerreDeconEngineClass.lvclass">)  [unwired: 8 in]
        n698 = call "dataInitilize.vi"("error in (no error)"=w1481, "LaguerreDeconClass in"=w1482) -> ("error out"=w1479:errorcluster, "LaguerreDeconClass out"=w1480:refnum<class "LaguerreDeconEngineClass.lvclass">)  [unwired: 8 in]
        n699 = call "computeDeconMatrix.vi"("error in (no error)"=w1479, "LaguerreDeconClass in"=w1480) -> ("error out"=w1475:errorcluster, "LaguerreDeconClass out"=w1477:refnum<class "LaguerreDeconEngineClass.lvclass">)  [unwired: 8 in]
        n700 = call "Ch4DeconEngineFGV.vi"("Error In"=w1475, "action(read)"=enum16{"write", "read"}."write" ("action"), "Ch3DeconEngine in"=w1477) -> ("Error Out"=w1474:errorcluster)  [unwired: 7 in, 1 out]
        n701 = call <vilib>:"Add State(s) to Queue__JKI_lib_State_Machine.vi"("State(s) in (\"\")"=w1491) -> ("States Out"=w1490:string)  [unwired: 14 in]
      }
      frame "---------- Digitizer ----------" {
        # "Template Separator\n(You can make a copy of, or modify, this frame)"
        n702 = call <vilib>:"Add State(s) to Queue__JKI_lib_State_Machine.vi"("State(s) in (\"\")"=w1496) -> ("States Out"=w1495:string)  [unwired: 14 in]
      }
      frame "Digitizer: Initialize" {
        # "reset digitizer to everytime the system runs"
        # "reset digitizer to everytime the system runs"
        # "Initialize digitizer.\nInitialize both digitizer and update status."
        n703 = call "FLImDAQ_FGV.vi"("error in (no error)"=w1504) -> ("error out"=w1498:errorcluster, "Read data"=w1503:T5)  [unwired: 9 in]
        n704 = Unbundle By Name(w1506) -> ("SysConfigCluster.Ch1Enable?"=w1511:bool, "SysConfigCluster.Ch2Enable?"=w1510:bool, "SysConfigCluster.Ch3Enable?"=w1508:bool)
        n705 = Unbundle By Name(w1503) -> ("Digitizer 1"=w1499:refnum<k15>, "Digitizer 2"=w1502:refnum<k15>)
        n706 = property on="Digitizer" class="Bool (strict)"("Blinking"=TRUE) -> ()  [unwired: 2 in, 2 out]
        n707 = Or(x=w1511, y=w1510) -> (x .or. y?=w1509:bool)
        n708 = case shown="True" w1509 {
          tunnel: w1498 -> [w1519 w1522]
          tunnel: [w1519 w1521] -> w1500
          tunnel: w1499 -> [_ w1523]
          frame False {
          }
          frame True {
            n709 = call <instrlib>:"niScope Initialize.vi"("resource name"=w1523, "reset device"=TRUE, "error in"=w1522) -> ("error out"=w1521:errorcluster)  [unwired: 11 in, 1 out]
          }
        }
        n710 = case shown="True" w1508 {
          tunnel: w1498 -> [w1514 w1516]
          tunnel: [w1514 w1518] -> w1505
          tunnel: w1502 -> [_ w1517]
          frame False {
          }
          frame True {
            n711 = call <instrlib>:"niScope Initialize.vi"("resource name"=w1517, "reset device"=TRUE, "error in"=w1516) -> ("error out"=w1518:errorcluster)  [unwired: 11 in, 1 out]
          }
        }
        n712 = Merge Errors(w1500, w1505) -> (w1497:errorcluster)
        n713 = call <vilib>:"Add State(s) to Queue__JKI_lib_State_Machine.vi"("State(s) in (\"\")"=w1513) -> ("States Out"=w1512:string)  [unwired: 14 in]
      }
      frame "Digitizer: Config" {
        # "Synchronize is taking time ~3s."
        # "Config  digitizer\nCall subVi to config digitizer"
        n714 = call "FLImDAQ_FGV.vi"() -> ("Read data"=w1541:T5)  [unwired: 10 in, 1 out]
        n715 = Unbundle By Name(w1550) -> ("SysConfigCluster.Ch1Enable?"=w1558:bool, "SysConfigCluster.Ch2Enable?"=w1557:bool, "SysConfigCluster.Ch3Enable?"=w1555:bool, "FLImDAQ"=w1552:T33)
        n716 = Unbundle By Name(w1541) -> ("Digitizer 1"=w1544:refnum<k15>, "Digitizer 2"=w1543:refnum<k15>)
        n717 = property on="Digitizer" class="Bool (strict)"(error in=w1545, "Blinking"=TRUE) -> (error out=w1546:errorcluster)  [unwired: 1 in, 1 out]
        n718 = Or(x=w1558, y=w1557) -> (x .or. y?=w1556:bool)
        n719 = case shown="True" w1556 {
          tunnel: w1552 -> [_ w1571]
          tunnel: w1546 -> [w1567 w1570]
          tunnel: [w1567 w1569] -> w1553
          tunnel: w1544 -> [_ w1568]
          frame False {
          }
          frame True {
            n720 = call "DigitizerConfig.vi"("error in (no error)"=w1570, "FLImDAQ"=w1571, "IVI Refnum in"=w1568) -> ("error out"=w1569:errorcluster)  [unwired: 7 in, 1 out]
          }
        }
        n721 = case shown="True" w1555 {
          tunnel: w1552 -> [_ w1566]
          tunnel: w1553 -> [w1561 w1565]
          tunnel: [w1561 w1564] -> w1529
          tunnel: w1543 -> [_ w1562]
          frame False {
          }
          frame True {
            n722 = call "DigitizerConfig.vi"("Config Trigger? (T)"=FALSE ("Config Trigge(T)r:"), "error in (no error)"=w1565, "FLImDAQ"=w1566, "IVI Refnum in"=w1562) -> ("error out"=w1564:errorcluster)  [unwired: 6 in, 1 out]
          }
        }
        n723 = call "Digitizer1_FGV.vi"("error in (no error)"=w1529) -> ("error out"=w1539:errorcluster, "Read data"=w1540:refnum<k15>)  [unwired: 9 in]
        n724 = call <instrlib>:"niScope Get Session Reference.vi"("instrument handle"=w1540, "error in"=w1539) -> ("session reference"=w1533:refnum<k20>, "error out"=w1531:errorcluster)  [unwired: 11 in, 1 out]
        n725 = call "Digitizer2_FGV.vi"("error in (no error)"=w1531) -> ("error out"=w1537:errorcluster, "Read data"=w1538:refnum<k15>)  [unwired: 9 in]
        n726 = call <instrlib>:"niScope Get Session Reference.vi"("instrument handle"=w1538, "error in"=w1537) -> ("session reference"=w1532:refnum<k20>, "error out"=w1530:errorcluster)  [unwired: 11 in, 1 out]
        n727 = Build Array(w1533, w1532) -> (w1536:refnum<k20>[])
        n728 = call <instrlib>:"niTClk Configure For Homogeneous Triggers.vi"("error in (no error)"=w1530, "sessions"=w1536) -> ("error out"=w1535:errorcluster, "sessions out"=w1534:refnum<k20>[])  [unwired: 8 in]
        n729 = call <instrlib>:"niTClk Synchronize.vi"("error in (no error)"=w1535, "sessions"=w1534) -> ("error out"=w1528:errorcluster, "sessions out"=w1526:refnum<k20>[])  [unwired: 8 in]
        n730 = call <userlib>:"Wait (ms)__ogtk.vi"("error in (no error)"=w1528, "milliseconds to wait"=u32 1500) -> ("error out"=w1524:errorcluster)  [unwired: 8 in, 1 out]
        n731 = Unbundle By Name(w1524) -> ("status"=w1549:bool)
        n732 = Not(x=w1549) -> (.not. x?=w1548:bool)
        n733 = Bundle By Name(cluster=w1550, "System Status.Digitizer"=w1548, "niTClk sessions"=w1526) -> (w1551:T26)
        n734 = property on="Digitizer" class="Bool (strict)"(error in=w1524, "Blinking"=FALSE) -> (error out=w1542:errorcluster)  [unwired: 1 in, 1 out]
        n735 = call <vilib>:"Add State(s) to Queue__JKI_lib_State_Machine.vi"("State(s) in (\"\")"=w1560) -> ("States Out"=w1559:string)  [unwired: 14 in]
      }
      frame "Digitizer: Start" {
        # "send trigger to start acquisition loop"
        # "initilize aquisition"
        # "Start Digitizer\n(TClk start)"
        n736 = Unbundle By Name(w1579) -> ("niTClk sessions"=w1578:refnum<k20>[])
        n737 = call <instrlib>:"niTClk Initiate.vi"("error in (no error)"=w1572, "sessions"=w1578) -> ("error out"=w1574:errorcluster)  [unwired: 8 in, 1 out]
        n738 = Generate User Event(priority (normal)=usereventprio."high priority", user event=w1575, event data cluster=TRUE ("event data"), error in=w1574) -> (error out=w1573:errorcluster)  [unwired: 1 out]
        n739 = call <vilib>:"Add State(s) to Queue__JKI_lib_State_Machine.vi"("State(s) in (\"\")"=w1582) -> ("States Out"=w1581:string)  [unwired: 14 in]
      }
      frame "Digitizer: Abort" {
        # "Template Separator\n(You can make a copy of, or modify, this frame)"
        n740 = call "Digitizer1_FGV.vi"("error in (no error)"=w1586, "Operation (Read)"=enum16{"Write", "Read"}."Read" ("Operation")) -> ("error out"=w1593:errorcluster, "Read data"=w1590:refnum<k15>)  [unwired: 8 in]
        n741 = call "Digitizer2_FGV.vi"("error in (no error)"=w1586, "Operation (Read)"=enum16{"Write", "Read"}."Read" ("Operation")) -> ("error out"=w1589:errorcluster, "Read data"=w1591:refnum<k15>)  [unwired: 8 in]
        n742 = Bundle By Name(cluster=w1583, "SysRunning?"=FALSE ("System Status")) -> (w1584:T26)
        n743 = call <instrlib>:"niScope Abort.vi"("instrument handle"=w1590, "error in"=w1593) -> ("error out"=w1595:errorcluster)  [unwired: 12 in, 1 out]
        n744 = call <instrlib>:"niScope Abort.vi"("instrument handle"=w1591, "error in"=w1589) -> ("error out"=w1594:errorcluster)  [unwired: 12 in, 1 out]
        n745 = Merge Errors(w1595, w1594) -> (w1587:errorcluster)
        n746 = call <vilib>:"Add State(s) to Queue__JKI_lib_State_Machine.vi"("State(s) in (\"\")"=w1598) -> ("States Out"=w1597:string)  [unwired: 14 in]
      }
      frame "Digitizer: checkTemp" {
        w1601 = 75.0 ("y")
        w1606 = enum16{"Write", "Read"}."Read" ("Operation")
        # "Template Separator\n(You can make a copy of, or modify, this frame)"
        n747 = call "Digitizer1_FGV.vi"("Operation (Read)"=w1606) -> ("error out"=w1607:errorcluster, "Read data"=w1608:refnum<k15>)  [unwired: 9 in]
        n748 = call "Digitizer2_FGV.vi"("Operation (Read)"=w1606) -> ("error out"=w1604:errorcluster, "Read data"=w1605:refnum<k15>)  [unwired: 9 in]
        n749 = property on="Property Node" class="niScope"(reference=w1605, error in=w1604) -> ("Device Temperature"=w1602:dbl)  [unwired: 2 out]
        "Dig2 Temp" <- w1602
        n750 = property on="Property Node" class="niScope"(reference=w1608, error in=w1607) -> ("Device Temperature"=w1603:dbl)  [unwired: 2 out]
        "Dig1 Temp" <- w1603
        n751 = Greater?(x=w1603, y=w1601) -> (0:w1600:bool)
        n752 = Greater?(x=w1602, y=w1601) -> (0:w1599:bool)
        n753 = case shown="True" w1600 {
          frame False {
          }
          frame True {
            n754 = One Button Dialog(message="Digitizer 1 over heating!", button name ("OK")="OK") -> ()  [unwired: 1 out]
          }
        }
        n755 = case shown="True" w1599 {
          frame False {
          }
          frame True {
            n756 = One Button Dialog(message="Digitizer 2 over heating!", button name ("OK")="OK") -> ()  [unwired: 1 out]
          }
        }
        n757 = call <vilib>:"Add State(s) to Queue__JKI_lib_State_Machine.vi"("State(s) in (\"\")"=w1613) -> ("States Out"=w1612:string)  [unwired: 14 in]
      }
      frame "Digitizer: Close" {
        # "Close Digitizer"
        n758 = call "Digitizer1_FGV.vi"("error in (no error)"=w1623, "Operation (Read)"=enum16{"Write", "Read"}."Read" ("Operation")) -> ("error out"=w1625:errorcluster, "Read data"=w1629:refnum<k15>)  [unwired: 8 in]
        n759 = call "Digitizer2_FGV.vi"("error in (no error)"=w1623, "Operation (Read)"=enum16{"Write", "Read"}."Read" ("Operation")) -> ("error out"=w1624:errorcluster, "Read data"=w1627:refnum<k15>)  [unwired: 8 in]
        n760 = call <instrlib>:"niScope Close.vi"("instrument handle"=w1629, "error in"=w1625) -> ("error out"=w1622:errorcluster)  [unwired: 13 in]
        n761 = call <instrlib>:"niScope Close.vi"("instrument handle"=w1627, "error in"=w1624) -> ("error out"=w1621:errorcluster)  [unwired: 13 in]
        n762 = Merge Errors(w1622, w1621) -> (w1620:errorcluster)
        n763 = Unbundle By Name(w1620) -> ("status"=w1619:bool)
        n764 = Bundle By Name(cluster=w1630, "System Status.Digitizer"=w1619) -> (w1631:T26)
        n765 = call <vilib>:"Add State(s) to Queue__JKI_lib_State_Machine.vi"("State(s) in (\"\")"=w1633) -> ("States Out"=w1632:string)  [unwired: 14 in]
      }
      frame "---------- LabJack ----------" {
        # "Template Separator\n(You can make a copy of, or modify, this frame)"
        n766 = call <vilib>:"Add State(s) to Queue__JKI_lib_State_Machine.vi"("State(s) in (\"\")"=w1638) -> ("States Out"=w1637:string)  [unwired: 14 in]
      }
      frame "LabJack: checkPedal" {
        # "Template Separator\n(You can make a copy of, or modify, this frame)"
        n767 = Unbundle By Name(w1639) -> ("LJ Pinout.Foot Pedal"=w1643:string)
        n768 = call "LabJack_FGV.vi"("Operation(Read)"=enum16{"Write", "Read"}."Read" ("Operation"), "error in (no error)"=w1641) -> ("error out"=w1645:errorcluster, "Read data"=w1646:i32)  [unwired: 8 in]
        n769 = call "LJM_eReadName.vi"("Handle In"=w1646, "Name"=w1643, "error in"=w1645) -> ("Value"=w1644:dbl, "error out"=w1642:errorcluster)  [unwired: 10 in, 1 out]
        n770 = case shown="1" w1644 {
          tunnel: w1639 -> [w1651 w1654]
          tunnel: [w1651 w1652] -> w1640
          frame 0, Default {
          }
          frame 1 {
            # "If Pedal pressed"
            n771 = Tick Count (ms)() -> (millisecond timer value=w1658:u32)
            n772 = Unbundle By Name(w1654) -> ("Last Trigger"=w1653:u32)
            n773 = Subtract(x=w1658, y=w1653) -> (x-y=w1657:u32)
            n774 = Greater Or Equal?(x=w1657, y=u32 2000) -> (x >= y?=w1655:bool)
            n775 = case shown="True" w1655 {
              tunnel: w1654 -> [w1659 w1660]
              tunnel: w1653 -> [_ _]
              tunnel: [w1659 w1661] -> w1652
              frame False {
              }
              frame True {
                n776 = Tick Count (ms)() -> (millisecond timer value=w1662:u32)
                n777 = Unbundle By Name(w1660) -> ("SysRunning?"=w1663:bool)
                n778 = case shown="False" w1663 {
                  frame False {
                    n779 = property on="StartButton" class="Bool (strict)"("Val(Sgnl)"=TRUE ("Value (Signaling)")) -> ()  [unwired: 2 in, 2 out]
                  }
                  frame True {
                    n780 = property on="StopButton" class="Bool (strict)"("Val(Sgnl)"=TRUE ("Value (Signaling)")) -> ()  [unwired: 2 in, 2 out]
                  }
                }
                n781 = Bundle By Name(cluster=w1660, "Last Trigger"=w1662) -> (w1661:T26)
              }
            }
          }
        }
        n782 = call <vilib>:"Add State(s) to Queue__JKI_lib_State_Machine.vi"("State(s) in (\"\")"=w1650) -> ("States Out"=w1649:string)  [unwired: 14 in]
      }
      frame "LabJack: ZeroV" {
        # "Just Zero V\nDO not update FGV and front panel\nWIll resume from last V"
        # "set bias to 0"
        # "Zero APD bias\n(You can make a copy of, or modify, this frame)"
        n783 = Unbundle By Name(w1668) -> ("LJ Pinout.Ch1 Bias"=w1673:string, "LJ Pinout.Ch2 Bias"=w1672:string, "LJ Pinout.Ch3 Bias"=w1671:string)
        n784 = Build Array(w1673, w1672, w1671) -> (w1670:string[])
        n785 = call "LabJack_FGV.vi"("Operation(Read)"=enum16{"Write", "Read"}."Read" ("Operation"), "error in (no error)"=w1667) -> ("error out"=w1674:errorcluster, "Read data"=w1675:i32)  [unwired: 8 in]
        n786 = call "LJM_eWriteNames.vi"("Handle In"=w1675, "aNames"=w1670, "aValuesIn"=dbl[] [0.0, 0.0, 0.0], "error in"=w1674) -> ("error out"=w1666:errorcluster)  [unwired: 9 in, 2 out]
        n787 = call <vilib>:"Add State(s) to Queue__JKI_lib_State_Machine.vi"("State(s) in (\"\")"=w1679) -> ("States Out"=w1678:string)  [unwired: 14 in]
      }
      frame "LabJack: SetV" {
        w1686 = enum16{"write", "read"}."read" ("action (write)")
        # "set bias to user specifid"
        # "Set APD bias\n(You can make a copy of, or modify, this frame)"
        n788 = Unbundle By Name(w1695) -> ("LJ Pinout.Ch1 Bias"=w1699:string, "LJ Pinout.Ch2 Bias"=w1698:string, "LJ Pinout.Ch3 Bias"=w1697:string, "LJ Pinout.Ch4 Bias"=w1689:string)
        n789 = call "V2FGV.vi"("Error In"=w1685, "action(write)"=w1686) -> ("Error Out"=w1683:errorcluster, "V2 out"=w1691:dbl)  [unwired: 8 in]
        n790 = call "V4FGV.vi"("Error In"=w1685, "action(write)"=w1686) -> ("Error Out"=w1681:errorcluster, "V3 out"=w1687:dbl)  [unwired: 8 in]
        n791 = call "V1FGV.vi"("Error In"=w1685, "action (write)"=w1686) -> ("Error Out"=w1684:errorcluster, "V1 out"=w1688:dbl)  [unwired: 8 in]
        n792 = call "V3FGV.vi"("Error In"=w1685, "action(write)"=w1686) -> ("Error Out"=w1682:errorcluster, "V3 out"=w1690:dbl)  [unwired: 8 in]
        n793 = local write "V 3"(w1690) -> ()
        n794 = local write "V 2"(w1691) -> ()
        n795 = local write "V 4"(w1687) -> ()
        n796 = local write "V 1"(w1688) -> ()
        n797 = Build Array(w1699, w1698, w1697, w1689) -> (w1696:string[])
        n798 = call "LabJack_FGV.vi"("Operation(Read)"=enum16{"Write", "Read"}."Read" ("Operation"), "error in (no error)"=w1685) -> ("error out"=w1700:errorcluster, "Read data"=w1701:i32)  [unwired: 8 in]
        n799 = Build Array(w1688, w1691, w1690, w1687) -> (w1692:dbl[])
        n800 = call "LJM_eWriteNames.vi"("Handle In"=w1701, "aNames"=w1696, "aValuesIn"=w1692, "error in"=w1700) -> ("error out"=w1693:errorcluster)  [unwired: 9 in, 2 out]
        n801 = Merge Errors(w1684, w1683, w1682, w1681) -> (w1680:errorcluster)
        n802 = call <vilib>:"Add State(s) to Queue__JKI_lib_State_Machine.vi"("State(s) in (\"\")"=w1705) -> ("States Out"=w1704:string)  [unwired: 14 in]
        n803 = Merge Errors(w1680, w1693) -> (w1694:errorcluster)
      }
      frame "LabJack: Open" {
        # "Initialize LabJack T7\nEstablish connection and initialize pins"
        n804 = call "LJ_Open.vi"("error in"=w1715, "DeviceType"="LJM_dtT7") -> ("error out"=w1712:errorcluster, "Success?"=w1713:bool, "Handle Out"=w1707:i32)  [unwired: 7 in]
        n805 = call "LabJack_FGV.vi"("Operation(Read)"=enum16{"Write", "Read"}."Write" ("Operation"), "error in (no error)"=w1712, "Write data"=w1707) -> ("error out"=w1709:errorcluster)  [unwired: 7 in, 1 out]
        n806 = Bundle By Name(cluster=w1710, "System Status.Labjack"=w1713) -> (w1714:T26)
        n807 = call <vilib>:"Add State(s) to Queue__JKI_lib_State_Machine.vi"("State(s) in (\"\")"=w1717) -> ("States Out"=w1716:string)  [unwired: 14 in]
      }
      frame "LabJack: SetDefaultSub" {
        w1727 = enum16{"write", "read"}."write" ("action")
        w1728 = 0.0 ("V1 in")
        w1741 = "_EF_ENABLE" ("string")
        # "1. Disable PWM\n2. Set all V to 0\n3. Set 355 relay to open\n4. Set LED to off"
        # "read once to set DIO to input"
        # "set all initila V to 0. Set footpedal to input. Set PWM to low. Set laser relay to open. Set LEDs to yellow."
        # "Set Labjack to correct input and output state and initial values"
        n808 = disable-structure shown="Disabled" {
          frame Disabled {
            (unwired) dbl[] [0.0, 0.0, 0.0, 0.0, 0.0, 0.0, 0.0, 0.0, 0.0] ("aValuesIn")
          }
          frame Enabled {
          }
        }
        n809 = Unbundle By Name(w1738) -> ("LJ Pinout.355 PWM"=w1743:string, "LJ Pinout.AimingBeam PWM"=w1742:string, "LJ Pinout.Ch1 Bias"=w1748:string, "LJ Pinout.Ch2 Bias"=w1718:string, "LJ Pinout.Ch3 Bias"=w1752:string, "LJ Pinout.Ch4 Bias"=w1732:string, "LJ Pinout.Laser Start/Stop"=w1751:string, "LJ Pinout.Red LED"=w1750:string, "LJ Pinout.Green LED"=w1749:string)
        n810 = call "V1FGV.vi"("Error In"=w1736, "action (write)"=w1727, "V1 in"=w1728) -> ("Error Out"=w1731:errorcluster, "V1 out"=w1735:dbl)  [unwired: 7 in]
        n811 = local write "V 1"(w1735) -> ()
        n812 = call "V2FGV.vi"("Error In"=w1731, "action(write)"=w1727, "V2 in"=w1728) -> ("Error Out"=w1730:errorcluster, "V2 out"=w1734:dbl)  [unwired: 7 in]
        n813 = call "LabJack_FGV.vi"("Operation(Read)"=enum16{"Write", "Read"}."Read" ("Operation"), "error in (no error)"=w1736) -> ("error out"=w1724:errorcluster, "Read data"=w1746:i32)  [unwired: 8 in]
        n814 = Concatenate Strings(w1743, w1741) -> (w1740:string)
        n815 = Concatenate Strings(w1742, w1741) -> (w1739:string)
        n816 = local write "V 2"(w1734) -> ()
        n817 = call "V3FGV.vi"("Error In"=w1730, "action(write)"=w1727, "V3 in"=w1728) -> ("Error Out"=w1729:errorcluster, "V3 out"=w1733:dbl)  [unwired: 7 in]
        n818 = Build Array(w1740, w1739, w1748, w1718, w1752, w1732, w1751, w1750, w1749) -> (w1722:string[])
        n819 = local write "V 3"(w1733) -> ()
        n820 = call "V4FGV.vi"("Error In"=w1729, "action(write)"=w1727, "V3 in"=w1728) -> ("Error Out"=w1725:errorcluster, "V3 out"=w1726:dbl)  [unwired: 7 in]
        n821 = Array Size(array=w1722) -> (size(s)=w1721:i32)
        n822 = local write "V 4"(w1726) -> ()
        n823 = Initialize Array(0.0 ("element"), w1721) -> (w1719:dbl[])
        n824 = Unbundle By Name(w1738) -> ("LJ Pinout.Foot Pedal"=w1737:string)
        n825 = call "LJM_eWriteNames.vi"("Handle In"=w1746, "aNames"=w1722, "aValuesIn"=w1719, "error in"=w1724) -> ("Handle Out"=w1745:i32, "error out"=w1744:errorcluster)  [unwired: 9 in, 1 out]
        n826 = call "LJM_eReadName.vi"("Handle In"=w1745, "Name"=w1737, "error in"=w1744) -> ("error out"=w1723:errorcluster)  [unwired: 10 in, 2 out]
        n827 = case shown="Error .." w1723 {
          frame No Error {
            # "no error"
          }
          frame Error {
            # "handle error"
            n828 = One Button Dialog(message="Labjack error! The pin assignment is likely wrong. Please check pin setting of Labjack. Program will terminate.", button name ("OK")="OK") -> ()  [unwired: 1 out]
          }
        }
        n829 = call <vilib>:"Add State(s) to Queue__JKI_lib_State_Machine.vi"("State(s) in (\"\")"=w1755) -> ("States Out"=w1754:string)  [unwired: 14 in]
      }
      frame "LabJack: FootPedalConfig" {
        # "Setup footPedal\n(You can make a copy of, or modify, this frame)"
        n830 = call "LabJack_FGV.vi"("Operation(Read)"=enum16{"Write", "Read"}."Read" ("Operation"), "error in (no error)"=w1759) -> ("error out"=w1763:errorcluster, "Read data"=w1764:i32)  [unwired: 8 in]
        n831 = call "LJM_eWriteName.vi"("Handle In"=w1764, "Name"="DIO15", "Value"=1.0, "error in"=w1763) -> ("error out"=w1760:errorcluster)  [unwired: 10 in, 1 out]
        n832 = call <vilib>:"Add State(s) to Queue__JKI_lib_State_Machine.vi"("State(s) in (\"\")"=w1768) -> ("States Out"=w1767:string)  [unwired: 14 in]
      }
      frame "LabJack: SetDefaultAndClose" {
        # "Template Separator\n(You can make a copy of, or modify, this frame)"
        n833 = call <vilib>:"Add State(s) to Queue__JKI_lib_State_Machine.vi"("State(s) in Front (\"\")"="LabJack: SetDefaultSub\nLabJack: Close" ("State(s) in Front (\"\")"), "State(s) in (\"\")"=w1774) -> ("States Out"=w1773:string)  [unwired: 13 in]
      }
      frame "LabJack: Close" {
        # "Close LabJack Refnum"
        n834 = call "LabJack_FGV.vi"("Operation(Read)"=enum16{"Write", "Read"}."Read" ("Operation"), "error in (no error)"=w1780) -> ("error out"=w1775:errorcluster, "Read data"=w1776:i32)  [unwired: 8 in]
        n835 = Bundle By Name(cluster=w1778, "System Status.Labjack"=FALSE ("System Status.Gain Control")) -> (w1781:T26)
        n836 = call "LJM_Close.vi"("error in"=w1775, "Handle"=w1776) -> ("error out"=w1783:errorcluster)  [unwired: 9 in]
        n837 = call <vilib>:"Add State(s) to Queue__JKI_lib_State_Machine.vi"("State(s) in (\"\")"=w1785) -> ("States Out"=w1784:string)  [unwired: 14 in]
      }
      frame "LabJack: Interlock enable/disable" {
        w1794 = i8 0  # int8
        # "[Covers: REQ8]"
        # "Interlock enable/disable\n(Usage: \"LabJack: Interlock enable/disable >> 1|0\")"
        n838 = Fract/Exp String To Number(string=w1795, default (0 dbl)=w1794) -> (number=w1791:i8)  [unwired: 2 in, 1 out]
        n839 = Unbundle By Name(w1793) -> ("LJ Pinout.Interlock"=w1792:string)
        n840 = call "LabJack_FGV.vi"("Operation(Read)"=enum16{"Write", "Read"}."Read" ("Operation")) -> ("Read data"=w1789:i32)  [unwired: 9 in, 1 out]
        n841 = call "LJM_eWriteName.vi"("Handle In"=w1789, "Name"=w1792, "Value"=w1791, "error in"=w1790) -> ("error out"=w1787:errorcluster)  [unwired: 10 in, 1 out]
        n842 = call <vilib>:"Add State(s) to Queue__JKI_lib_State_Machine.vi"("State(s) in (\"\")"=w1797) -> ("States Out"=w1796:string)  [unwired: 14 in]
      }
      frame "LabJack: 355_PWM_Config" {
        w1799 = 0.0 ("element")
        w1819 = "DIO_EF_CLOCK1_ENABLE"
        # "Config PWM frequency"
        n843 = Unbundle By Name(w1811) -> ("LJ Pinout.355 PWM"=w1818:string)
        n844 = Unbundle By Name(w1811) -> ("355 PWM setting.DIO_EF_CLOCK1_DIVISOR"=w1810:i16, "355 PWM setting.DIO_EF_CLOCK1_ROLL_VALUE"=w1809:i32, "355 PWM setting.DIO#_EF_INDEX"=w1806:i16, "355 PWM setting.DIO#_EF_OPTIONS"=w1805:i16, "355 PWM setting.DIO#_EF_CONFIG_A"=w1804:i32)
        n845 = Concatenate Strings(w1818, "_EF_ENABLE" ("string")) -> (w1814:string)
        n846 = Concatenate Strings(w1818, "_EF_INDEX") -> (w1817:string)
        n847 = Concatenate Strings(w1818, "_EF_OPTIONS") -> (w1816:string)
        n848 = Concatenate Strings(w1818, "_EF_CONFIG_A") -> (w1815:string)
        n849 = call "LabJack_FGV.vi"("Operation(Read)"=enum16{"Write", "Read"}."Read" ("Operation")) -> ("Read data"=w1812:i32)  [unwired: 9 in, 1 out]
        n850 = Build Array(w1799, w1799, w1810, w1809, 1.0 ("element"), 0.0 ("element"), w1806, w1805, w1804) -> (w1803:dbl[])
        n851 = Build Array("DIO_EF_CLOCK0_ENABLE", w1819, "DIO_EF_CLOCK1_DIVISOR", "DIO_EF_CLOCK1_ROLL_VALUE", w1819, w1814, w1817, w1816, w1815) -> (w1813:string[])
        n852 = call "LJM_eWriteNames.vi"("Handle In"=w1812, "aNames"=w1813, "aValuesIn"=w1803, "error in"=w1801) -> ("error out"=w1802:errorcluster)  [unwired: 9 in, 2 out]
        n853 = call <vilib>:"Add State(s) to Queue__JKI_lib_State_Machine.vi"("State(s) in (\"\")"=w1828) -> ("States Out"=w1827:string)  [unwired: 14 in]
      }
      frame "LabJack: 355_PWM_Start" {
        # "Template Separator\n(You can make a copy of, or modify, this frame)"
        n854 = Unbundle By Name(w1836) -> ("LJ Pinout.355 PWM"=w1835:string)
        n855 = call "LabJack_FGV.vi"("Operation(Read)"=enum16{"Write", "Read"}."Read" ("Operation"), "error in (no error)"=w1830) -> ("error out"=w1837:errorcluster, "Read data"=w1838:i32)  [unwired: 8 in]
        n856 = Concatenate Strings(w1835, "_EF_ENABLE" ("string")) -> (w1833:string)
        n857 = call "LJM_eWriteName.vi"("Handle In"=w1838, "Name"=w1833, "Value"=1.0, "error in"=w1837) -> ("error out"=w1831:errorcluster)  [unwired: 10 in, 1 out]
        n858 = call <vilib>:"Add State(s) to Queue__JKI_lib_State_Machine.vi"("State(s) in (\"\")"=w1841) -> ("States Out"=w1840:string)  [unwired: 14 in]
      }
      frame "LabJack: 355_PWM_Stop" {
        # "Template Separator\n(You can make a copy of, or modify, this frame)"
        n859 = Unbundle By Name(w1847) -> ("LJ Pinout.355 PWM"=w1851:string)
        n860 = call "LabJack_FGV.vi"("Operation(Read)"=enum16{"Write", "Read"}."Read" ("Operation"), "error in (no error)"=w1846) -> ("error out"=w1852:errorcluster, "Read data"=w1844:i32)  [unwired: 8 in]
        n861 = Concatenate Strings(w1851, "_EF_ENABLE" ("string")) -> (w1849:string)
        n862 = call "LJM_eWriteName.vi"("Handle In"=w1844, "Name"=w1849, "Value"=0.0, "error in"=w1852) -> ("error out"=w1843:errorcluster)  [unwired: 10 in, 1 out]
        n863 = local write "355nm Laser toggle"(FALSE ("355nm Laser toggle")) -> ()
        n864 = call <vilib>:"Add State(s) to Queue__JKI_lib_State_Machine.vi"("State(s) in (\"\")"=w1855) -> ("States Out"=w1854:string)  [unwired: 14 in]
      }
      frame "LabJack: AB_Start" {
        # "Aiming Beam Start\n(Based on aimging beam frequency, set LabJack pin)"
        n865 = Unbundle By Name(w1865) -> ("AB Cluster.Freq"=w1857:i32, "LJ Pinout.AimingBeam PWM"=w1864:string)
        n866 = Greater Than 0?(x=w1857) -> (x > 0?=w1856:bool)
        n867 = case shown="False" w1856 {
          tunnel: w1864 -> [w1871 w1874]
          tunnel: [w1871 w1872] -> w1863
          frame False {
            # "if 0 freq, set PWM pin"
          }
          frame True {
            # "if non zero freq, set PWM enable"
            n868 = Concatenate Strings(w1874, "_EF_ENABLE" ("string")) -> (w1872:string)
          }
        }
        n869 = call "LabJack_FGV.vi"("Operation(Read)"=enum16{"Write", "Read"}."Read" ("Operation"), "error in (no error)"=w1860) -> ("error out"=w1866:errorcluster, "Read data"=w1867:i32)  [unwired: 8 in]
        n870 = call "LJM_eWriteName.vi"("Handle In"=w1867, "Name"=w1863, "Value"=1.0, "error in"=w1866) -> ("error out"=w1861:errorcluster)  [unwired: 10 in, 1 out]
        n871 = local write "Aiming beam toggle"(TRUE ("Aiming beam toggle")) -> ()
        n872 = call <vilib>:"Add State(s) to Queue__JKI_lib_State_Machine.vi"("State(s) in (\"\")"=w1870) -> ("States Out"=w1869:string)  [unwired: 14 in]
      }
      frame "LabJack: AB_Stop" {
        # "Aiming Beam Stop\n(Based on aiming beam frequency, set LabJack pin low)"
        n873 = Unbundle By Name(w1882) -> ("AB Cluster.Freq"=w1877:i32, "LJ Pinout.AimingBeam PWM"=w1884:string)
        n874 = Greater Than 0?(x=w1877) -> (x > 0?=w1876:bool)
        n875 = case shown="False" w1876 {
          tunnel: w1884 -> [w1890 w1893]
          tunnel: [w1890 w1891] -> w1875
          frame False {
          }
          frame True {
            n876 = Concatenate Strings(w1893, "_EF_ENABLE" ("string")) -> (w1891:string)
          }
        }
        n877 = call "LabJack_FGV.vi"("Operation(Read)"=enum16{"Write", "Read"}."Read" ("Operation"), "error in (no error)"=w1880) -> ("error out"=w1885:errorcluster, "Read data"=w1886:i32)  [unwired: 8 in]
        n878 = call "LJM_eWriteName.vi"("Handle In"=w1886, "Name"=w1875, "Value"=0.0, "error in"=w1885) -> ("error out"=w1881:errorcluster)  [unwired: 10 in, 1 out]
        n879 = local write "Aiming beam toggle"(FALSE ("Aiming beam toggle")) -> ()
        n880 = call <vilib>:"Add State(s) to Queue__JKI_lib_State_Machine.vi"("State(s) in (\"\")"=w1889) -> ("States Out"=w1888:string)  [unwired: 14 in]
      }
      frame "LabJack: AB_PWM_Config" {
        w1895 = 0.0 ("element")
        w1915 = "DIO_EF_CLOCK2_ENABLE"
        # "Config PWM frequency"
        n881 = Unbundle By Name(w1907) -> ("LJ Pinout.AimingBeam PWM"=w1914:string)
        n882 = Unbundle By Name(w1907) -> ("AB PWM setting.DIO_EF_CLOCK1_DIVISOR"=w1906:i16, "AB PWM setting.DIO_EF_CLOCK1_ROLL_VALUE"=w1905:i32, "AB PWM setting.DIO#_EF_INDEX"=w1902:i16, "AB PWM setting.DIO#_EF_OPTIONS"=w1901:i16, "AB PWM setting.DIO#_EF_CONFIG_A"=w1900:i32)
        n883 = Concatenate Strings(w1914, "_EF_ENABLE" ("string")) -> (w1910:string)
        n884 = Concatenate Strings(w1914, "_EF_INDEX") -> (w1913:string)
        n885 = Concatenate Strings(w1914, "_EF_OPTIONS") -> (w1912:string)
        n886 = Concatenate Strings(w1914, "_EF_CONFIG_A") -> (w1911:string)
        n887 = call "LabJack_FGV.vi"("Operation(Read)"=enum16{"Write", "Read"}."Read" ("Operation")) -> ("Read data"=w1908:i32)  [unwired: 9 in, 1 out]
        n888 = Build Array(w1895, w1895, w1906, w1905, 1.0 ("element"), 0.0 ("element"), w1902, w1901, w1900) -> (w1899:dbl[])
        n889 = Build Array("DIO_EF_CLOCK0_ENABLE", w1915, "DIO_EF_CLOCK2_DIVISOR", "DIO_EF_CLOCK2_ROLL_VALUE", w1915, w1910, w1913, w1912, w1911) -> (w1909:string[])
        n890 = call "LJM_eWriteNames.vi"("Handle In"=w1908, "aNames"=w1909, "aValuesIn"=w1899, "error in"=w1897) -> ("error out"=w1898:errorcluster)  [unwired: 9 in, 2 out]
        n891 = call <vilib>:"Add State(s) to Queue__JKI_lib_State_Machine.vi"("State(s) in (\"\")"=w1924) -> ("States Out"=w1923:string)  [unwired: 14 in]
      }
      frame "---------- LED ----------" {
        # "Template Separator\n(You can make a copy of, or modify, this frame)"
        n892 = call <vilib>:"Add State(s) to Queue__JKI_lib_State_Machine.vi"("State(s) in (\"\")"=w1929) -> ("States Out"=w1928:string)  [unwired: 14 in]
      }
      frame "LED: OpenVIRef" {
        # "Template Separator\n(You can make a copy of, or modify, this frame)"
        n893 = call <vilib>:"Application Directory.vi"() -> ("Application Directory"=w1936:path)
        n894 = Build Path(base path=w1936, name or relative path="SubVI") -> (appended path=w1934:path)
        n895 = Build Path(base path=w1934, name or relative path="LEDBreath.vi") -> (appended path=w1932:path)
        n896 = Open VI Reference(vi path=w1932, error in (no error)=w1937) -> (vi reference=w1938:refnum<vi>, error out=w1931:errorcluster)  [unwired: 4 in]
        n897 = case shown="Error .." w1931 {
          tunnel: [TRUE FALSE] -> w1930
          frame No Error {
          }
          frame Error {
          }
        }
        n898 = Bundle By Name(cluster=w1939, "LED vi reference"=w1938, "LED vi ref open?"=w1930) -> (w1940:T26)
        n899 = call <vilib>:"Add State(s) to Queue__JKI_lib_State_Machine.vi"("State(s) in (\"\")"=w1943) -> ("States Out"=w1942:string)  [unwired: 14 in]
      }
      frame "LED: CloseVIRef" {
        # "Template Separator\n(You can make a copy of, or modify, this frame)"
        n900 = Unbundle By Name(w1947) -> ("LED vi reference"=w1948:refnum<vi>, "LED vi ref open?"=w1946:bool)
        n901 = case shown="True" w1946 {
          tunnel: w1950 -> [w1954 w1957]
          tunnel: [w1954 w1956] -> w1949
          tunnel: w1948 -> [_ w1955]
          frame False {
          }
          frame True {
            n902 = Close Reference(reference=w1955, error in (no error)=w1957) -> (error out=w1956:errorcluster)
          }
        }
        n903 = call <vilib>:"Add State(s) to Queue__JKI_lib_State_Machine.vi"("State(s) in (\"\")"=w1953) -> ("States Out"=w1952:string)  [unwired: 14 in]
      }
      frame "LED: BreathGreen" {
        w1958 = FALSE ("Wait Until Done")
        # "Breath system LED\n(LED: Breath >> True/False)"
        n904 = Unbundle By Name(w1966) -> ("LED vi reference"=w1965:refnum<vi>)
        n905 = invoke class="VI" method="Ctrl Val.Set"(reference=w1965, error in=w1963, "Control Name"="Color", "Value"=0) -> (reference out=w1962:refnum<vi>, error out=w1961:errorcluster)  [unwired: 1 in, 3 out]
        n906 = invoke on="Invoke Node" class="VI" method="Run VI"(reference=w1962, error in=w1961, "Wait until done"=w1958, "Auto Dispose Ref"=w1958) -> (error out=w1964:errorcluster)  [unwired: 1 in, 4 out]
        n907 = call <vilib>:"Add State(s) to Queue__JKI_lib_State_Machine.vi"("State(s) in (\"\")"=w1969) -> ("States Out"=w1968:string)  [unwired: 14 in]
      }
      frame "LED: BreathOrange" {
        w1970 = FALSE ("Wait Until Done")
        # "Breath system LED\n(LED: Breath >> True/False)"
        n908 = Unbundle By Name(w1978) -> ("LED vi reference"=w1977:refnum<vi>)
        n909 = invoke class="VI" method="Ctrl Val.Set"(reference=w1977, error in=w1975, "Control Name"="Color", "Value"=1) -> (reference out=w1974:refnum<vi>, error out=w1973:errorcluster)  [unwired: 1 in, 3 out]
        n910 = invoke on="Invoke Node" class="VI" method="Run VI"(reference=w1974, error in=w1973, "Wait until done"=w1970, "Auto Dispose Ref"=w1970) -> (error out=w1976:errorcluster)  [unwired: 1 in, 4 out]
        n911 = call <vilib>:"Add State(s) to Queue__JKI_lib_State_Machine.vi"("State(s) in (\"\")"=w1981) -> ("States Out"=w1980:string)  [unwired: 14 in]
      }
      frame "LED: BreathOff" {
        # "System LED Breath Off\n(Breath off, check VI status to make sure it is off)"
        n912 = Unbundle By Name(w1990) -> ("LED vi reference"=w1989:refnum<vi>)
        n913 = invoke on="Invoke Node" class="VI" method="Ctrl Val.Set"(reference=w1989, error in=w1987, "Control Name"="Stop", "Value"=TRUE) -> (reference out=w1982:refnum<vi>, error out=w1983:errorcluster)  [unwired: 1 in, 3 out]
        n914 = case shown="No Error" w1983 {
          selector: w1983 -> [w1995 _]
          tunnel: [w1994 errorcluster {"status"=FALSE, "code"=0, "source"=""} ("error IO")] -> w1988
          tunnel: ["" ("State(s) in Front (\"\")") "LED: BreathOff" ("State(s) in Front (\"\")")] -> w1986
          tunnel: w1982 -> [w1996 _]
          frame No Error {
            # "No error, wait for VI to stop"
            n915 = while {
              tunnel: w1996 -> [w2004]
              shift-right: [w1998] -> w1994
              shift-left: w1995 -> [w2003]
              stop <- w2000 stop-if-true
              # "continue check whether vi is running"
              n916 = property class="VI"(reference=w2004, error in=w2003) -> (error out=w1998:errorcluster, "Exec.State"=w2002:T23)  [unwired: 1 out]
              n917 = Wait (ms)(milliseconds to wait=u32 50) -> ()  [unwired: 1 out]
              n918 = Equal?(x=w2002, y=T23."Idle") -> (x = y?=w2000:bool)
            }
          }
          frame Error {
            # "try again when error"
          }
        }
        n919 = call <vilib>:"Add State(s) to Queue__JKI_lib_State_Machine.vi"("State(s) in Front (\"\")"=w1986, "State(s) in (\"\")"=w1993) -> ("States Out"=w1992:string)  [unwired: 13 in]
      }
      frame "LED: Off" {
        # "set LED to red"
        # "Template Separator\n(You can make a copy of, or modify, this frame)"
        n920 = Unbundle By Name(w2009) -> ("LJ Pinout.Red LED"=w2008:string, "LJ Pinout.Green LED"=w2007:string)
        n921 = call "LabJack_FGV.vi"("Operation(Read)"=enum16{"Write", "Read"}."Read" ("Operation"), "error in (no error)"=w2010) -> ("error out"=w2017:errorcluster, "Read data"=w2016:i32)  [unwired: 8 in]
        n922 = call "LJM_eWriteName.vi"("Handle In"=w2016, "Name"=w2008, "Value"=0.0, "error in"=w2017) -> ("Handle Out"=w2014:i32, "error out"=w2013:errorcluster)  [unwired: 10 in]
        n923 = call "LJM_eWriteName.vi"("Handle In"=w2014, "Name"=w2007, "Value"=0.0, "error in"=w2013) -> ("error out"=w2011:errorcluster)  [unwired: 10 in, 1 out]
        n924 = call <vilib>:"Add State(s) to Queue__JKI_lib_State_Machine.vi"("State(s) in (\"\")"=w2021) -> ("States Out"=w2020:string)  [unwired: 14 in]
      }
      frame "LED: Green" {
        # "set LED to green"
        # "Template Separator\n(You can make a copy of, or modify, this frame)"
        n925 = Unbundle By Name(w2025) -> ("LJ Pinout.Red LED"=w2023:string, "LJ Pinout.Green LED"=w2024:string)
        n926 = call "LabJack_FGV.vi"("Operation(Read)"=enum16{"Write", "Read"}."Read" ("Operation"), "error in (no error)"=w2027) -> ("error out"=w2033:errorcluster, "Read data"=w2032:i32)  [unwired: 8 in]
        n927 = call "LJM_eWriteName.vi"("Handle In"=w2032, "Name"=w2023, "Value"=0.0, "error in"=w2033) -> ("Handle Out"=w2030:i32, "error out"=w2029:errorcluster)  [unwired: 10 in]
        n928 = call "LJM_eWriteName.vi"("Handle In"=w2030, "Name"=w2024, "Value"=9.0, "error in"=w2029) -> ("error out"=w2026:errorcluster)  [unwired: 10 in, 1 out]
        n929 = call <vilib>:"Add State(s) to Queue__JKI_lib_State_Machine.vi"("State(s) in (\"\")"=w2036) -> ("States Out"=w2035:string)  [unwired: 14 in]
      }
      frame "---------- Queue ----------" {
        # "Template Separator\n(You can make a copy of, or modify, this frame)"
        n930 = call <vilib>:"Add State(s) to Queue__JKI_lib_State_Machine.vi"("State(s) in (\"\")"=w2041) -> ("States Out"=w2040:string)  [unwired: 14 in]
      }
      frame "Queue: Flash" {
        # "Clear queue contnet\n(clear queue content by flash it)"
        n931 = Flush Queue(queue=w2048, error in (no error)=w2042) -> (error out=w2046:errorcluster)  [unwired: 2 out]
        n932 = Flush Queue(queue=w2049, error in (no error)=w2042) -> (error out=w2045:errorcluster)  [unwired: 2 out]
        n933 = Flush Queue(queue=w2047, error in (no error)=w2042) -> (error out=w2044:errorcluster)  [unwired: 2 out]
        n934 = Merge Errors(w2046, w2045, w2044) -> (w2043:errorcluster)
        n935 = call <vilib>:"Add State(s) to Queue__JKI_lib_State_Machine.vi"("State(s) in (\"\")"=w2053) -> ("States Out"=w2052:string)  [unwired: 14 in]
      }
      frame "Queue: Destory" {
        # "Destory Data Queue\nDistory data queue ref so the aquisition loop stop"
        n936 = Release Queue(queue=w2059, error in (no error)=w2055) -> (error out=w2062:errorcluster)  [unwired: 1 in, 2 out]
        n937 = Release Queue(queue=w2058, error in (no error)=w2055) -> (error out=w2061:errorcluster)  [unwired: 1 in, 2 out]
        n938 = Release Queue(queue=w2056, error in (no error)=w2055) -> (error out=w2054:errorcluster)  [unwired: 1 in, 2 out]
        n939 = Merge Errors(w2062, w2061, w2054) -> (w2060:errorcluster)
        n940 = call <vilib>:"Simple Error Handler.vi"("error in (no error)"=w2060) -> ()  [unwired: 4 in, 5 out]
        n941 = call <vilib>:"Add State(s) to Queue__JKI_lib_State_Machine.vi"("State(s) in (\"\")"=w2065) -> ("States Out"=w2064:string)  [unwired: 14 in]
      }
      frame "---------- Run ----------" {
        # "Template Separator\n(You can make a copy of, or modify, this frame)"
        n942 = call <vilib>:"Add State(s) to Queue__JKI_lib_State_Machine.vi"("State(s) in (\"\")"=w2070) -> ("States Out"=w2069:string)  [unwired: 14 in]
      }
      frame "Run: CaliIncrement" {
        # "Increment Calibration #\n(You can make a copy of, or modify, this frame)"
        n943 = Unbundle By Name(w2072) -> ("IDs.Cali ID"=w2074:i8)
        n944 = Increment(x=w2074) -> (x+1=w2071:i8)
        n945 = Bundle By Name(cluster=w2072, "IDs.Cali ID"=w2071) -> (w2073:T26)
        n946 = call <vilib>:"Add State(s) to Queue__JKI_lib_State_Machine.vi"("State(s) in (\"\")"=w2078) -> ("States Out"=w2077:string)  [unwired: 14 in]
      }
      frame "Run: BGIncrement" {
        # "Increment BG #\n(You can make a copy of, or modify, this frame)"
        n947 = Unbundle By Name(w2079) -> ("IDs.BG ID"=w2082:i8)
        n948 = Increment(x=w2082) -> (x+1=w2081:i8)
        n949 = Bundle By Name(cluster=w2079, "IDs.BG ID"=w2081) -> (w2080:T26)
        n950 = call <vilib>:"Add State(s) to Queue__JKI_lib_State_Machine.vi"("State(s) in (\"\")"=w2086) -> ("States Out"=w2085:string)  [unwired: 14 in]
      }
      frame "Run: Increment" {
        # "Increase Run# by 1"
        n951 = Unbundle By Name(w2091) -> ("IDs.RunID"=w2093:i8)
        n952 = Increment(x=w2093) -> (x+1=w2089:i8)
        n953 = Bundle By Name(cluster=w2091, "IDs.RunID"=w2089) -> (w2092:T26)
        n954 = call "RunIDFGV.vi"("Error In"=w2087, "RunID in"=w2089) -> ("Error Out"=w2088:errorcluster)  [unwired: 8 in, 1 out]
        n955 = call <vilib>:"Add State(s) to Queue__JKI_lib_State_Machine.vi"("State(s) in (\"\")"=w2095) -> ("States Out"=w2094:string)  [unwired: 14 in]
      }
      frame "Run: Decrement" {
        # "Increase Run# by 1"
        n956 = Unbundle By Name(w2100) -> ("IDs.RunID"=w2102:i8)
        n957 = Decrement(x=w2102) -> (x-1=w2098:i8)
        n958 = Bundle By Name(cluster=w2100, "IDs.RunID"=w2098) -> (w2101:T26)
        n959 = call "RunIDFGV.vi"("Error In"=w2096, "RunID in"=w2098) -> ("Error Out"=w2097:errorcluster)  [unwired: 8 in, 1 out]
        n960 = call <vilib>:"Add State(s) to Queue__JKI_lib_State_Machine.vi"("State(s) in (\"\")"=w2104) -> ("States Out"=w2103:string)  [unwired: 14 in]
      }
      frame "---------- SysConfig ----------" {
        # "Template Separator\n(You can make a copy of, or modify, this frame)"
        n961 = call <vilib>:"Add State(s) to Queue__JKI_lib_State_Machine.vi"("State(s) in (\"\")"=w2109) -> ("States Out"=w2108:string)  [unwired: 14 in]
      }
      frame "SysConfig: LoadAPDSerialNumber" {
        # "Template Separator\n(You can make a copy of, or modify, this frame)"
        n962 = call "readAPDSerial.vi"("Error In"=w2111) -> ("Error Out"=w2110:errorcluster, "output cluster"=w2112:T29)  [unwired: 9 in]
        n963 = Bundle By Name(cluster=w2113, "APDSerialNum"=w2112) -> (w2114:T26)
        n964 = call <vilib>:"Add State(s) to Queue__JKI_lib_State_Machine.vi"("State(s) in (\"\")"=w2117) -> ("States Out"=w2116:string)  [unwired: 14 in]
      }
      frame "SysConfig: Load Sys Config" {
        # "[Covers: REQ5]"
        # "Load System config"
        # "Load system configuration\n(Load both hardware and DAQ config)"
        n965 = call "LoadSysConfig.vi"("Error In"=w2120, "Enum"=enum16{"LastUse", "Default"}."LastUse") -> ("Error Out"=w2119:errorcluster, "SysConfigCluster"=w2122:T7)  [unwired: 8 in]
        "SysConfigCluster" <- w2122
        n966 = Bundle By Name(cluster=w2123, "SysConfigCluster"=w2122) -> (w2124:T26)
        n967 = call <vilib>:"Add State(s) to Queue__JKI_lib_State_Machine.vi"("State(s) in (\"\")"=w2126) -> ("States Out"=w2125:string)  [unwired: 14 in]
      }
      frame "SysConfig: Load Digitizer Setting" {
        w2127 = enum16{"Write", "Read"}."Write" ("Operation")
        # "Load DAQ config\nSave to FGV"
        # "Template Separator\n(You can make a copy of, or modify, this frame)"
        n968 = call <userlib>:"Current VIs Parent Directory__ogtk.vi"() -> ("Parent Directory (+ Relative)"=w2141:path)  [unwired: 5 in]
        n969 = Build Path(base path=w2141, name or relative path="SubVI\\DigitizerConfiguration\\V6_Scope_last_use.config") -> (appended path=w2142:path)
        n970 = call "ReadDigitizerConfig(SubVI).vi"("error in (no error)"=w2139, "appended path"=w2142) -> ("error out"=w2135:errorcluster, "FLImDAQ"=w2133:T5)  [unwired: 8 in]
        n971 = call "FLImDAQ_FGV.vi"("error in (no error)"=w2135, "Operation (Read)"=w2127, "Write data"=w2133) -> ("error out"=w2137:errorcluster)  [unwired: 7 in, 1 out]
        n972 = Unbundle By Name(w2133) -> ("min record length"=→"data length":i32, "Digitizer 1"=w2129:refnum<k15>, "Digitizer 2"=w2136:refnum<k15>)
        n973 = Bundle By Name(cluster=w2131, "FLImDAQ"=w2133) -> (w2132:T26)
        n974 = call "Digitizer1_FGV.vi"("error in (no error)"=w2137, "Operation (Read)"=w2127, "Write data"=w2129) -> ("error out"=w2138:errorcluster)  [unwired: 7 in, 1 out]
        n975 = call "Digitizer2_FGV.vi"("error in (no error)"=w2138, "Operation (Read)"=w2127, "Write data"=w2136) -> ("error out"=w2134:errorcluster)  [unwired: 7 in, 1 out]
        n976 = call <vilib>:"Add State(s) to Queue__JKI_lib_State_Machine.vi"("State(s) in (\"\")"=w2144) -> ("States Out"=w2143:string)  [unwired: 14 in]
      }
      frame "SysConfig: Load LJ Pinout" {
        # "Template Separator\n(You can make a copy of, or modify, this frame)"
        n977 = call <userlib>:"Current VIs Parent Directory__ogtk.vi"() -> ("Parent Directory (+ Relative)"=w2159:path)  [unwired: 5 in]
        n978 = Build Path(base path=w2159, name or relative path="SubVI\\LabJack\\LJ_pin_setting.config") -> (appended path=w2157:path)
        n979 = call "ReadLabjackConfig(SubVI).vi"("error in (no error)"=w2155, "appended path"=w2157) -> ("error out"=w2156:errorcluster, "Utility"=w2153:T4)  [unwired: 8 in]
        n980 = Unbundle By Name(w2153) -> ("Ch1 Bias"=w2152:string, "Ch2 Bias"=w2151:string, "Ch3 Bias"=w2150:string, "Ch4 Bias"=w2145:string, "Red LED"=w2147:string, "Green LED"=w2146:string)
        n981 = global write "GlobalVariables.vi" "LED Green pin"(w2146) -> ()
        n982 = global write "GlobalVariables.vi" "Ch1 LJ pin"(w2152) -> ()
        n983 = global write "GlobalVariables.vi" "Ch2 LJ pin"(w2151) -> ()
        n984 = global write "GlobalVariables.vi" "Ch3 LJ pin"(w2150) -> ()
        n985 = global write "GlobalVariables.vi" "Ch4 LJ pin"(w2145) -> ()
        n986 = global write "GlobalVariables.vi" "LED Red pin"(w2147) -> ()
        n987 = Bundle By Name(cluster=w2148, "LJ Pinout"=w2153) -> (w2154:T26)
        n988 = call <vilib>:"Add State(s) to Queue__JKI_lib_State_Machine.vi"("State(s) in (\"\")"=w2161) -> ("States Out"=w2160:string)  [unwired: 14 in]
      }
      frame "SysConfig: Load 355 PWM" {
        # "Template Separator\n(You can make a copy of, or modify, this frame)"
        n989 = call <userlib>:"Current VIs Parent Directory__ogtk.vi"() -> ("Parent Directory (+ Relative)"=w2179:path)  [unwired: 5 in]
        n990 = Build Path(base path=w2179, name or relative path="SubVI\\LabJack\\PWM_setting_355.config") -> (appended path=w2177:path)
        n991 = call "ReadPWMConfig(SubVI).vi"("error in (no error)"=w2174, "appended path"=w2177) -> ("error out"=w2175:errorcluster, "PWM Setting"=w2173:T43)  [unwired: 8 in]
        n992 = Unbundle By Name(w2173) -> ("DIO_EF_CLOCK1_DIVISOR"=w2170:i16, "DIO_EF_CLOCK1_ROLL_VALUE"=w2169:i32)
        n993 = Multiply(x=w2170, y=w2169) -> (x*y=w2171:i32)
        n994 = Bundle By Name(cluster=w2176, "355 PWM setting"=w2173) -> (w2163:T26)
        n995 = Divide(x=80000000.0, y=w2171) -> (x/y=w2168:dbl)
        "Laser Rep Rate" <- w2168
        n996 = Number To Decimal String(number=w2168) -> (decimal integer string=w2167:string)  [unwired: 1 in]
        n997 = Concatenate Strings("355nm " ("string"), w2167, "Hz" ("string")) -> (w2165:string)
        n998 = property on="355nm Laser toggle" class="Bool (strict)"("Caption.Text"=w2165) -> ()  [unwired: 2 in, 2 out]
        n999 = call <vilib>:"Add State(s) to Queue__JKI_lib_State_Machine.vi"("State(s) in (\"\")"=w2181) -> ("States Out"=w2180:string)  [unwired: 14 in]
      }
      frame "SysConfig: Load AB PWM" {
        # "Template Separator\n(You can make a copy of, or modify, this frame)"
        n1000 = call <userlib>:"Current VIs Parent Directory__ogtk.vi"() -> ("Parent Directory (+ Relative)"=w2190:path)  [unwired: 5 in]
        n1001 = Build Path(base path=w2190, name or relative path="SubVI\\LabJack\\PWM_setting_AB.config") -> (appended path=w2188:path)
        n1002 = call "ReadPWMConfig(SubVI).vi"("error in (no error)"=w2185, "appended path"=w2188) -> ("error out"=w2186:errorcluster, "PWM Setting"=w2184:T43)  [unwired: 8 in]
        n1003 = Bundle By Name(cluster=w2182, "AB PWM setting"=w2184) -> (w2187:T26)
        n1004 = call <vilib>:"Add State(s) to Queue__JKI_lib_State_Machine.vi"("State(s) in (\"\")"=w2192) -> ("States Out"=w2191:string)  [unwired: 14 in]
      }
      frame "SysConfig: Load AB setting" {
        # "load aming beam setting\n(check frequency, if 0 do nothing, if not zero, config PWM)"
        n1005 = call "readAimingBeamSetting.vi"("error in (no error)"=w2210) -> ("error out"=w2205:errorcluster, "Aiming Beam Setting"=w2197:T44)  [unwired: 9 in]
        n1006 = Unbundle By Name(w2197) -> ("Default Current"=w2196:dbl)
        n1007 = Unbundle By Name(w2197) -> ("Frequency(Hz)"=w2193:u32)
        n1008 = Equal To 0?(x=w2193) -> (x = 0?=w2203:bool)
        n1009 = Select(t="", s=w2203, f="SysConfig: Load AB PWM" ("State(s) in Front (\"\")")) -> (s? t:f=w2206:string)
        n1010 = Number To Decimal String(number=w2193) -> (decimal integer string=w2202:string)  [unwired: 1 in]
        n1011 = Number To Decimal String(number=w2196, width (-)=i16 2) -> (decimal integer string=w2195:string)
        n1012 = Concatenate Strings("445nm " ("string"), w2202, "Hz " ("string"), w2195, "mA" ("string")) -> (w2201:string)
        n1013 = property on="Aiming beam toggle" class="Bool (strict)"("Caption.Text"=w2201) -> ()  [unwired: 2 in, 2 out]
        n1014 = case shown="False" w2203 {
          tunnel: w2205 -> [w2218 w2221]
          tunnel: [w2217 w2221] -> w2204
          tunnel: w2193 -> [w2216 _]
          frame False {
            n1015 = call "LJ_calculate_PWM_parameters.vi"("Duty Cycle (%)"=u32 10, "Error In"=w2218, "Show Confirmation"=FALSE, "Laser Rep Rate (Hz)"=w2216, "Laser"=enum16{"355nm", "AimingBeam"}."AimingBeam") -> ("Error Out"=w2217:errorcluster)  [unwired: 5 in, 1 out]
          }
          frame True {
          }
        }
        n1016 = Bundle By Name(cluster=w2211, "AB Cluster"=w2197) -> (w2212:T26)
        n1017 = call <vilib>:"Add State(s) to Queue__JKI_lib_State_Machine.vi"("State(s) in Front (\"\")"=w2206, "State(s) in (\"\")"=w2214) -> ("States Out"=w2213:string)  [unwired: 13 in]
      }
      frame "SysConfig: LoadABVideoSetting" {
        # "Load AB video setting form ini file\n()"
        n1018 = call "readVideoConfig.vi"("error in (no error)"=w2225) -> ("error out"=w2226:errorcluster, "Aiming Beam Config"=w2224:T25)  [unwired: 8 in, 1 out]
        n1019 = Bundle By Name(cluster=w2222, "VideoConfig"=w2224) -> (w2223:T26)
        n1020 = call <vilib>:"Add State(s) to Queue__JKI_lib_State_Machine.vi"("State(s) in (\"\")"=w2229) -> ("States Out"=w2228:string)  [unwired: 14 in]
      }
      frame "SysConfig: LoadCursorLocation" {
        # "Load cursor location from ini file\n(load cursor from system setting ini file)"
        n1021 = call "readCursorConfigMain.vi"("error in (no error)"=w2241) -> ("error out"=w2242:errorcluster, "Cursor Locations"=w2240:T45)  [unwired: 9 in]
        n1022 = Unbundle By Name(w2240) -> ("DC1"=w2239:i32, "DC2"=w2238:i32, "BG1"=w2233:i32, "BG2"=w2232:i32)
        n1023 = Build Array(w2239, w2238) -> (w2237:i32[])
        n1024 = Build Array(w2233, w2232) -> (w2234:i32[])
        n1025 = Array Max & Min(array=w2237) -> (max value=w2236:i32, min value=w2235:i32)  [unwired: 2 out]
        n1026 = Array Max & Min(array=w2234) -> (max value=w2231:i32, min value=w2230:i32)  [unwired: 2 out]
        n1027 = global write "GlobalVariables.vi" "DC Idx2"(w2236) -> ()
        n1028 = global write "GlobalVariables.vi" "DC Idx1"(w2235) -> ()
        n1029 = global write "GlobalVariables.vi" "BG Idx2"(w2231) -> ()
        n1030 = global write "GlobalVariables.vi" "BG Idx1"(w2230) -> ()
        n1031 = call <vilib>:"Add State(s) to Queue__JKI_lib_State_Machine.vi"("State(s) in (\"\")"=w2246) -> ("States Out"=w2245:string)  [unwired: 14 in]
      }
      frame "---------- SystemStatus ----------" {
        # "Template Separator\n(You can make a copy of, or modify, this frame)"
        n1032 = call <vilib>:"Add State(s) to Queue__JKI_lib_State_Machine.vi"("State(s) in (\"\")"=w2251) -> ("States Out"=w2250:string)  [unwired: 14 in]
      }
      frame "SystemStatus: SlowSysStatusMacro" {
        # "store system check time"
        # "Template Separator\n(You can make a copy of, or modify, this frame)"
        n1033 = Tick Count (ms)() -> (millisecond timer value=w2254:u32)
        n1034 = Bundle By Name(cluster=w2252, "SlowTimer"=w2254) -> (w2253:T26)
        n1035 = call <vilib>:"Add State(s) to Queue__JKI_lib_State_Machine.vi"("State(s) in Front (\"\")"="Digitizer: checkTemp\nTCP: CheckConnection" ("State(s) in Front (\"\")"), "State(s) in (\"\")"=w2259) -> ("States Out"=w2258:string)  [unwired: 13 in]
      }
      frame "SystemStatus: FastSysStatusMacro" {
        # "store system check time"
        # "Template Separator\n(You can make a copy of, or modify, this frame)"
        n1036 = Tick Count (ms)() -> (millisecond timer value=w2262:u32)
        n1037 = Bundle By Name(cluster=w2260, "FastTimer"=w2262) -> (w2261:T26)
        n1038 = call <vilib>:"Add State(s) to Queue__JKI_lib_State_Machine.vi"("State(s) in Front (\"\")"="355 Laser: CheckPWMStatus\nAimingBeam: GetPWMStatus\n/*355 Laser: CheckControllerStatus" ("State(s) in Front (\"\")"), "State(s) in (\"\")"=w2267) -> ("States Out"=w2266:string)  [unwired: 13 in]
      }
      frame "---------- UI ----------" {
        # "Do not put any code in this frame.\n(It is a separator no-op. You can make a copy of this frame to create a new UI frame)"
        n1039 = call <vilib>:"Add State(s) to Queue__JKI_lib_State_Machine.vi"("State(s) in (\"\")"=w2272) -> ("States Out"=w2271:string)  [unwired: 14 in]
      }
      frame "UI: Initialize" {
        w2274 = T46 {"Minimum"=0.0, "Maximum"=4.6, "Increment"=0.1} ("Data Entry Limits")
        w2273 = T11."Disabled and Grayed Out" ("Disabled")
        # "Disable all button on startup"
        # "Initialize the User Interface, here.\n(this is called automatically, by the Macro: Init)"
        n1040 = property on="V 1" class="DigNum (strict)"("DisabledEnum"=w2273) -> ()  [unwired: 2 in, 2 out]
        n1041 = property on="V 2" class="DigNum (strict)"("DisabledEnum"=w2273) -> ()  [unwired: 2 in, 2 out]
        n1042 = property on="StopButton" class="Bool (strict)"("DisabledEnum"=w2273) -> ()  [unwired: 2 in, 2 out]
        n1043 = property on="Sys Reconfig" class="Bool"("DisabledEnum"=w2273) -> ()  [unwired: 2 in, 2 out]
        n1044 = property on="StartButton" class="Bool (strict)"("DisabledEnum"=w2273) -> ()  [unwired: 2 in, 2 out]
        n1045 = property on="355nm Laser toggle" class="Bool (strict)"("DisabledEnum"=w2273) -> ()  [unwired: 2 in, 2 out]
        n1046 = property on="Aiming beam toggle" class="Bool (strict)"("DisabledEnum"=w2273) -> ()  [unwired: 2 in, 2 out]
        n1047 = property on="Background" class="Bool (strict)"("DisabledEnum"=w2273) -> ()  [unwired: 2 in, 2 out]
        n1048 = property on="Cali&iRF alignment" class="Bool (strict)"("DisabledEnum"=w2273) -> ()  [unwired: 2 in, 2 out]
        n1049 = property on="V 3" class="DigNum (strict)"("DisabledEnum"=w2273) -> ()  [unwired: 2 in, 2 out]
        n1050 = property on="Video Source" class="RadioBtnsControl (strict)"("DisabledEnum"=w2273) -> ()  [unwired: 2 in, 2 out]
        n1051 = property on="V 1" class="DigNum (strict)"("Data Range"=w2274) -> ()  [unwired: 2 in, 2 out]
        n1052 = property on="V 2" class="DigNum (strict)"("Data Range"=w2274) -> ()  [unwired: 2 in, 2 out]
        n1053 = property on="V 3" class="DigNum (strict)"("Data Range"=w2274) -> ()  [unwired: 2 in, 2 out]
        n1054 = call <vilib>:"Add State(s) to Queue__JKI_lib_State_Machine.vi"("State(s) in Front (\"\")"="UI: CaliAndiRFNotReady" ("State(s) in Front (\"\")"), "State(s) in (\"\")"=w2280) -> ("States Out"=w2279:string)  [unwired: 13 in]
      }
      frame "UI: BGLoaded" {
        # "[Covers: REQ24]"
        # "Do not put any code in this frame.\n(It is a separator no-op. You can make a copy of this frame to create a new UI frame)"
        n1055 = property on="Background" class="Bool (strict)"("BoolText.Text"="Loaded!" ("Boolean Text.Text"), "Colors [4]"=cluster{u32, u32}[] [{15764023, 15764023}, {16711680, 16711680}]) -> ()  [unwired: 2 in, 2 out]
        n1056 = call <vilib>:"Add State(s) to Queue__JKI_lib_State_Machine.vi"("State(s) in (\"\")"=w2287) -> ("States Out"=w2286:string)  [unwired: 14 in]
      }
      frame "UI: BGSizeError" {
        # "[Covers: REQ24]"
        # "Do not put any code in this frame.\n(It is a separator no-op. You can make a copy of this frame to create a new UI frame)"
        n1057 = property on="Background" class="Bool (strict)"("BoolText.Text"="Loaded!" ("Boolean Text.Text"), "Colors [4]"=cluster{u32, u32}[] [{7171459, 7171459}, {16711680, 16711680}]) -> ()  [unwired: 2 in, 2 out]
        n1058 = One Button Dialog(message="Background waveform length and current digitizer setting mismatch! Please take a new background before any aquisition!") -> ()  [unwired: 1 in, 1 out]
        n1059 = call <vilib>:"Add State(s) to Queue__JKI_lib_State_Machine.vi"("State(s) in (\"\")"=w2295) -> ("States Out"=w2294:string)  [unwired: 14 in]
      }
      frame "UI: CaliAndiRFLoaded" {
        # "[Covers: REQ24]"
        # "Do not put any code in this frame.\n(It is a separator no-op. You can make a copy of this frame to create a new UI frame)"
        n1060 = property on="Cali&iRF alignment" class="Bool (strict)"("BoolText.Text"="Loaded!" ("Boolean Text.Text"), "Colors [4]"=cluster{u32, u32}[] [{15764023, 15764023}, {16711680, 16711680}]) -> ()  [unwired: 2 in, 2 out]
        n1061 = call <vilib>:"Add State(s) to Queue__JKI_lib_State_Machine.vi"("State(s) in (\"\")"=w2302) -> ("States Out"=w2301:string)  [unwired: 14 in]
      }
      frame "UI: WFAutoScale" {
        # "Set graph auto scale.\n(UI: WFAutoScale >> T/F)"
        n1062 = Equal?(x=w2303, y="F") -> (x = y?=w2304:bool)
        n1063 = Equal?(x=w2303, y="T") -> (x = y?=w2306:bool)
        n1064 = case shown="True" w2306 {
          frame False {
          }
          frame True {
            w2322 = u8 2 ("Y Scale.Scale Fit")
            n1065 = property on="Channel 1" class="WFGraph (strict)"("YScale.ScaleFit"=w2322) -> ()  [unwired: 2 in, 2 out]
            n1066 = property on="Channel 2" class="WFGraph (strict)"("YScale.ScaleFit"=w2322) -> ()  [unwired: 2 in, 2 out]
            n1067 = property on="Channel 3" class="WFGraph (strict)"("YScale.ScaleFit"=w2322) -> ()  [unwired: 2 in, 2 out]
          }
        }
        n1068 = case shown="True" w2304 {
          frame False {
          }
          frame True {
            w2319 = 0.0 ("Y Scale.Range:Maximum")
            w2320 = 2.0 ("Y Scale.Range:Maximum")
            w2321 = u8 0 ("Y Scale.Scale Fit")
            n1069 = property on="Channel 1" class="WFGraph (strict)"("YScale.ScaleFit"=w2321) -> (error out=w2318:errorcluster)  [unwired: 2 in, 1 out]
            n1070 = property on="Channel 2" class="WFGraph (strict)"("YScale.ScaleFit"=w2321) -> (error out=w2317:errorcluster)  [unwired: 2 in, 1 out]
            n1071 = property on="Channel 3" class="WFGraph (strict)"("YScale.ScaleFit"=w2321) -> (error out=w2316:errorcluster)  [unwired: 2 in, 1 out]
            n1072 = property on="Channel 1" class="WFGraph (strict)"(error in=w2318, "YScale.Maximum"=w2320) -> (error out=w2315:errorcluster)  [unwired: 1 in, 1 out]
            n1073 = property on="Channel 2" class="WFGraph (strict)"(error in=w2317, "YScale.Maximum"=w2320) -> (error out=w2314:errorcluster)  [unwired: 1 in, 1 out]
            n1074 = property on="Channel 3" class="WFGraph (strict)"(error in=w2316, "YScale.Maximum"=w2320) -> (error out=w2313:errorcluster)  [unwired: 1 in, 1 out]
            n1075 = property on="Channel 1" class="WFGraph (strict)"(error in=w2315, "YScale.Minimum"=w2319) -> ()  [unwired: 1 in, 2 out]
            n1076 = property on="Channel 2" class="WFGraph (strict)"(error in=w2314, "YScale.Minimum"=w2319) -> ()  [unwired: 1 in, 2 out]
            n1077 = property on="Channel 3" class="WFGraph (strict)"(error in=w2313, "YScale.Minimum"=w2319) -> ()  [unwired: 1 in, 2 out]
          }
        }
        n1078 = call <vilib>:"Add State(s) to Queue__JKI_lib_State_Machine.vi"("State(s) in (\"\")"=w2312) -> ("States Out"=w2311:string)  [unwired: 14 in]
      }
      frame "UI: showDisclaimer" {
        # "Show disclamer window.\n(It is a separator no-op. You can make a copy of this frame to create a new UI frame)"
        n1079 = call <vilib>:"Application Directory.vi"() -> ("Application Directory"=w2335:path)
        n1080 = Build Path(base path=w2335, name or relative path="Disclamer.png") -> (appended path=w2333:path)
        n1081 = property on="Disclamer" class="Pict"() -> ("Draw Area Size"=w2331:T47)  [unwired: 2 in, 2 out]
        n1082 = disable-structure "Diagram Disable Structure" shown="Disabled" {
          frame Disabled {
            n1083 = flat-sequence {
              frame #0 {
                n1084 = call "disclaimer.vi"() -> ()  [unwired: 12 in]
              }
              frame #1 {
                n1085 = Wait (ms)(milliseconds to wait=u32 250) -> ()  [unwired: 1 out]
              }
              frame #2 {
                n1086 = call "SoftwareNote.vi"() -> ()  [unwired: 12 in]
              }
            }
          }
          frame Enabled {
          }
        }
        n1087 = call <vilib>:"Read PNG File.vi"("path to PNG file"=w2333) -> ("image data"=w2330:T48)  [unwired: 8 in, 2 out]
        n1088 = Unbundle By Name(w2330) -> ("Rectangle.right"=w2328:i16, "Rectangle.bottom"=w2326:i16)
        n1089 = Unbundle By Name(w2331) -> ("Width"=w2329:u32, "Height"=w2327:u32)
        n1090 = call <vilib>:"Draw Flattened Pixmap.vi"("image data"=w2330) -> ("new picture"=→"Disclamer":picture)  [unwired: 8 in]
        n1091 = Divide(x=w2329, y=w2328) -> (x/y=w2325:dbl)
        n1092 = Divide(x=w2327, y=w2326) -> (x/y=w2324:dbl)
        n1093 = Max & Min(x=w2325, y=w2324) -> (min(x,y)=w2323:dbl)  [unwired: 1 out]
        n1094 = property on="Disclamer" class="Pict"("ZoomFactor"=w2323) -> ()  [unwired: 2 in, 2 out]
        n1095 = call <vilib>:"Add State(s) to Queue__JKI_lib_State_Machine.vi"("State(s) in (\"\")"=w2340) -> ("States Out"=w2339:string)  [unwired: 14 in]
      }
      frame "UI: CaliAndiRFNotReady" {
        # "Do not put any code in this frame.\n(It is a separator no-op. You can make a copy of this frame to create a new UI frame)"
        n1096 = property on="Cali&iRF alignment" class="Bool (strict)"("BoolText.Text"="No Info" ("Boolean Text.Text"), "Colors [4]"=cluster{u32, u32}[] [{13816530, 13816530}, {16711680, 16711680}]) -> ()  [unwired: 2 in, 2 out]
        n1097 = call <vilib>:"Add State(s) to Queue__JKI_lib_State_Machine.vi"("State(s) in (\"\")"=w2348) -> ("States Out"=w2347:string)  [unwired: 14 in]
      }
      frame "UI: BGnotReady" {
        # "Do not put any code in this frame.\n(It is a separator no-op. You can make a copy of this frame to create a new UI frame)"
        n1098 = property on="Background" class="Bool (strict)"("BoolText.Text"="No Info" ("Boolean Text.Text"), "Colors [4]"=cluster{u32, u32}[] [{13816530, 13816530}, {16711680, 16711680}]) -> ()  [unwired: 2 in, 2 out]
        n1099 = call <vilib>:"Add State(s) to Queue__JKI_lib_State_Machine.vi"("State(s) in (\"\")"=w2355) -> ("States Out"=w2354:string)  [unwired: 14 in]
      }
      frame "UI: Reset" {
        w2357 = cluster{u32, u32}[] [{13816530, 13816530}, {13816530, 13816530}] ("Colors [4]")
        # "Do not put any code in this frame.\n(It is a separator no-op. You can make a copy of this frame to create a new UI frame)"
        n1100 = property on="Cali&iRF alignment" class="Bool (strict)"("BoolText.Text"="No Info" ("Boolean Text.Text"), "Colors [4]"=w2357) -> ()  [unwired: 2 in, 2 out]
        n1101 = property on="Background" class="Bool (strict)"("BoolText.Text"="No Info" ("Boolean Text.Text"), "Colors [4]"=w2357) -> ()  [unwired: 2 in, 2 out]
        n1102 = call <vilib>:"Add State(s) to Queue__JKI_lib_State_Machine.vi"("State(s) in (\"\")"=w2363) -> ("States Out"=w2362:string)  [unwired: 14 in]
      }
      frame "UI: SetButtonText" {
        # "Set button text of 355nm laser and aiming beam."
        n1103 = call <vilib>:"Add State(s) to Queue__JKI_lib_State_Machine.vi"("State(s) in (\"\")"=w2368) -> ("States Out"=w2367:string)  [unwired: 14 in]
      }
      frame "UI: DuringAquisition" {
        w2371 = T11."Disabled and Grayed Out" ("Disabled")
        # "Do not put any code in this frame.\n(It is a separator no-op. You can make a copy of this frame to create a new UI frame)"
        n1104 = Unbundle By Name(w2370) -> ("bothVidSourceAvail"=w2369:bool)
        n1105 = case shown="True" w2369 {
          tunnel: w2371 -> [_ w2377]
          frame False {
          }
          frame True {
            n1106 = property on="Video Source" class="RadioBtnsControl (strict)"("DisabledEnum"=w2377) -> ()  [unwired: 2 in, 2 out]
          }
        }
        n1107 = property on="StartButton" class="Bool (strict)"("DisabledEnum"=w2371) -> ()  [unwired: 2 in, 2 out]
        n1108 = property on="Sys Reconfig" class="Bool"("DisabledEnum"=w2371) -> ()  [unwired: 2 in, 2 out]
        n1109 = property on="355nm Laser toggle" class="Bool (strict)"("DisabledEnum"=w2371) -> ()  [unwired: 2 in, 2 out]
        n1110 = property on="Aiming beam toggle" class="Bool (strict)"("DisabledEnum"=w2371) -> ()  [unwired: 2 in, 2 out]
        n1111 = property on="Background" class="Bool (strict)"("DisabledEnum"=w2371) -> ()  [unwired: 2 in, 2 out]
        n1112 = property on="Radio Buttons" class="RadioBtnsControl (strict)"("DisabledEnum"=w2371) -> ()  [unwired: 2 in, 2 out]
        n1113 = property on="Cali&iRF alignment" class="Bool (strict)"("DisabledEnum"=w2371) -> ()  [unwired: 2 in, 2 out]
        n1114 = property on="Quit" class="Bool"("DisabledEnum"=w2371) -> ()  [unwired: 2 in, 2 out]
        n1115 = property on="Skip Data Save?" class="Bool (strict)"("DisabledEnum"=w2371) -> ()  [unwired: 2 in, 2 out]
        n1116 = property on="Video Display" class="Bool (strict)"("DisabledEnum"=w2371) -> ()  [unwired: 2 in, 2 out]
        n1117 = property on="StopButton" class="Bool (strict)"("DisabledEnum"=T11."Enabled" ("Disabled")) -> ()  [unwired: 2 in, 2 out]
        n1118 = call <vilib>:"Add State(s) to Queue__JKI_lib_State_Machine.vi"("State(s) in (\"\")"=w2376) -> ("States Out"=w2375:string)  [unwired: 14 in]
      }
      frame "UI: duringIRFAlign" {
        w2378 = T11."Disabled and Grayed Out" ("Disabled")
        # "Set UI to during iRF alignment\n(It is a separator no-op. You can make a copy of this frame to create a new UI frame)"
        n1119 = property on="StartButton" class="Bool (strict)"("DisabledEnum"=w2378) -> ()  [unwired: 2 in, 2 out]
        n1120 = property on="Sys Reconfig" class="Bool"("DisabledEnum"=w2378) -> ()  [unwired: 2 in, 2 out]
        n1121 = property on="355nm Laser toggle" class="Bool (strict)"("DisabledEnum"=w2378) -> ()  [unwired: 2 in, 2 out]
        n1122 = property on="Aiming beam toggle" class="Bool (strict)"("DisabledEnum"=w2378) -> ()  [unwired: 2 in, 2 out]
        n1123 = property on="Background" class="Bool (strict)"("DisabledEnum"=w2378) -> ()  [unwired: 2 in, 2 out]
        n1124 = property on="StopButton" class="Bool (strict)"("DisabledEnum"=w2378) -> ()  [unwired: 2 in, 2 out]
        n1125 = call <vilib>:"Add State(s) to Queue__JKI_lib_State_Machine.vi"("State(s) in (\"\")"=w2383) -> ("States Out"=w2382:string)  [unwired: 14 in]
      }
      frame "UI: duringBGAcquire" {
        w2384 = T11."Disabled and Grayed Out" ("Disabled")
        # "Do not put any code in this frame.\n(It is a separator no-op. You can make a copy of this frame to create a new UI frame)"
        n1126 = property on="StartButton" class="Bool (strict)"("DisabledEnum"=w2384) -> ()  [unwired: 2 in, 2 out]
        n1127 = property on="StopButton" class="Bool (strict)"("DisabledEnum"=w2384) -> ()  [unwired: 2 in, 2 out]
        n1128 = property on="Sys Reconfig" class="Bool"("DisabledEnum"=w2384) -> ()  [unwired: 2 in, 2 out]
        n1129 = property on="355nm Laser toggle" class="Bool (strict)"("DisabledEnum"=w2384) -> ()  [unwired: 2 in, 2 out]
        n1130 = property on="Aiming beam toggle" class="Bool (strict)"("DisabledEnum"=w2384) -> ()  [unwired: 2 in, 2 out]
        n1131 = property on="Cali&iRF alignment" class="Bool (strict)"("DisabledEnum"=w2384) -> ()  [unwired: 2 in, 2 out]
        n1132 = call <vilib>:"Add State(s) to Queue__JKI_lib_State_Machine.vi"("State(s) in (\"\")"=w2389) -> ("States Out"=w2388:string)  [unwired: 14 in]
      }
      frame "UI: ReadyForAquisition" {
        w2393 = T11."Enabled" ("Disabled")
        # "Do not put any code in this frame.\n(It is a separator no-op. You can make a copy of this frame to create a new UI frame)"
        n1133 = Unbundle By Name(w2392) -> ("System Status.TCP/IP"=w2391:bool, "bothVidSourceAvail"=w2390:bool)
        n1134 = property on="StartButton" class="Bool (strict)"("DisabledEnum"=w2393) -> ()  [unwired: 2 in, 2 out]
        n1135 = property on="Sys Reconfig" class="Bool"("DisabledEnum"=w2393) -> ()  [unwired: 2 in, 2 out]
        n1136 = property on="355nm Laser toggle" class="Bool (strict)"("DisabledEnum"=w2393) -> ()  [unwired: 2 in, 2 out]
        n1137 = property on="Aiming beam toggle" class="Bool (strict)"("DisabledEnum"=w2393) -> ()  [unwired: 2 in, 2 out]
        n1138 = property on="Cali&iRF alignment" class="Bool (strict)"("DisabledEnum"=w2393) -> ()  [unwired: 2 in, 2 out]
        n1139 = property on="Background" class="Bool (strict)"("DisabledEnum"=w2393) -> ()  [unwired: 2 in, 2 out]
        n1140 = property on="Quit" class="Bool"("DisabledEnum"=w2393) -> ()  [unwired: 2 in, 2 out]
        n1141 = property on="Radio Buttons" class="RadioBtnsControl (strict)"("DisabledEnum"=w2393) -> ()  [unwired: 2 in, 2 out]
        n1142 = case shown="True" w2390 {
          tunnel: w2393 -> [_ w2399]
          frame False {
          }
          frame True {
            n1143 = property on="Video Source" class="RadioBtnsControl (strict)"("DisabledEnum"=w2399) -> ()  [unwired: 2 in, 2 out]
          }
        }
        n1144 = property on="Skip Data Save?" class="Bool (strict)"("DisabledEnum"=w2393) -> ()  [unwired: 2 in, 2 out]
        n1145 = case shown="True" w2391 {
          tunnel: w2393 -> [_ w2400]
          frame False {
          }
          frame True {
            n1146 = property on="Video Display" class="Bool (strict)"("DisabledEnum"=w2400) -> ()  [unwired: 2 in, 2 out]
          }
        }
        n1147 = property on="StopButton" class="Bool (strict)"("DisabledEnum"=T11."Disabled and Grayed Out" ("Disabled")) -> ()  [unwired: 2 in, 2 out]
        n1148 = call <vilib>:"Add State(s) to Queue__JKI_lib_State_Machine.vi"("State(s) in (\"\")"=w2398) -> ("States Out"=w2397:string)  [unwired: 14 in]
      }
      frame "UI: Update" {
        # "Do not put any code in this frame.\n(It is a separator no-op. You can make a copy of this frame to create a new UI frame)"
        n1149 = Unbundle By Name(w2411) -> ("System Status"=→"System Hardware Connection Status":T2, "IDs.RunID"=→"Run #":i8, "CaseID"=→"Case #":string, "FLImDAQ"=→"FLImDAQ":T33, "SysRunning?"=→"Aquisition Status:":bool, "LJ Pinout"=→"LJ Pinout":T4, "IDs.BG ID"=→"BG #":i8, "IDs.Cali ID"=→"Calibration #":i8, "video source"=→"Visualization PC video source":T1)
        n1150 = call <vilib>:"Add State(s) to Queue__JKI_lib_State_Machine.vi"("State(s) in (\"\")"=w2414) -> ("States Out"=w2413:string)  [unwired: 14 in]
      }
      frame "UI: updateVideoToggle" {
        # "Set video toggle based on visualization PC video source.\n(take )"
        n1151 = call <vilib>:"Add State(s) to Queue__JKI_lib_State_Machine.vi"("State(s) in (\"\")"=w2419) -> ("States Out"=w2418:string)  [unwired: 14 in]
      }
      frame "UI: Cursor Set" {
        # "Argument"
        # "Set and Unset Cursor Busy.\n(Usage: \"UI: Cursor Set >> Busy|Idle\")"
        n1152 = case shown="\"Idle\", Default" w2421 {
          tunnel: w2423 -> [w2428 w2430]
          tunnel: [w2427 w2429] -> w2422
          frame "Idle", Default {
            n1153 = call <vilib>:"Unset Busy.vi"("error in (no error)"=w2428) -> ("error out"=w2427:errorcluster)  [unwired: 10 in]
          }
          frame "Busy" {
            n1154 = call <vilib>:"Set Busy.vi"("error in (no error)"=w2430) -> ("error out"=w2429:errorcluster)  [unwired: 9 in, 1 out]
          }
        }
        n1155 = call <vilib>:"Add State(s) to Queue__JKI_lib_State_Machine.vi"("State(s) in (\"\")"=w2426) -> ("States Out"=w2425:string)  [unwired: 14 in]
      }
      frame "UI: Front Panel State" {
        # "Argument"
        # "Set Front Panel Open or Closed\n(Usage: \"UI: Front Panel State >> Open|Close\")"
        n1156 = Unbundle By Name(w2434) -> ("Core.Current VI Reference"=w2433:refnum<vi>)
        n1157 = case shown="\"Open\", \"Standard\", Default" w2432 {
          tunnel: w2436 -> [w2444 w2459 w2470 w2483 w2496]
          tunnel: [w2446 w2460 w2472 w2485 w2498] -> w2435
          tunnel: w2433 -> [w2445 w2457 w2471 w2484 w2497]
          frame "Open", "Standard", Default {
            w2439 = T21."Standard" ("State")
            n1158 = property on="Property Node" class="VI"(reference=w2445, error in=w2444) -> (reference out=w2442:refnum<vi>, error out=w2443:errorcluster, "FP.State"=w2441:T21)
            n1159 = Not Equal?(x=w2441, y=w2439) -> (x != y?=w2440:bool)
            n1160 = case shown="True" w2440 {
              tunnel: [w2450 w2452] -> w2446
              tunnel: w2443 -> [w2449 w2452]
              tunnel: w2442 -> [w2448 _]
              tunnel: w2439 -> [w2447 _]
              frame True {
                n1161 = invoke on="Invoke Node" class="VI" method="FP.Open"(reference=w2448, error in=w2449, "Activate"=TRUE, "State"=w2447) -> (error out=w2450:errorcluster)  [unwired: 1 in, 4 out]
              }
              frame False {
              }
            }
          }
          frame "Close", "Closed" {
            n1162 = property on="Property Node" class="VI"(reference=w2457, error in=w2459) -> (reference out=w2456:refnum<vi>, error out=w2458:errorcluster, "FP.State"=w2454:T21)
            n1163 = Not Equal?(x=w2454, y=T21."Closed" ("Front Panel Window:State")) -> (x != y?=w2453:bool)
            n1164 = case shown="True" w2453 {
              tunnel: [w2461 w2464] -> w2460
              tunnel: w2458 -> [w2461 w2463]
              tunnel: w2456 -> [_ w2462]
              frame False {
              }
              frame True {
                n1165 = invoke on="Invoke Node" class="VI" method="FP.Close"(reference=w2462, error in=w2463) -> (error out=w2464:errorcluster)  [unwired: 1 in, 2 out]
              }
            }
          }
          frame "Hidden", "Hide" {
            w2465 = T21."Hidden" ("State")
            n1166 = property on="Property Node" class="VI"(reference=w2471, error in=w2470) -> (reference out=w2468:refnum<vi>, error out=w2469:errorcluster, "FP.State"=w2467:T21)
            n1167 = Not Equal?(x=w2467, y=w2465) -> (x != y?=w2466:bool)
            n1168 = case shown="True" w2466 {
              tunnel: [w2476 w2477] -> w2472
              tunnel: w2469 -> [w2475 w2477]
              tunnel: w2468 -> [w2474 _]
              tunnel: w2465 -> [w2473 _]
              frame True {
                n1169 = invoke on="Invoke Node" class="VI" method="FP.Open"(reference=w2474, error in=w2475, "State"=w2473) -> (error out=w2476:errorcluster)  [unwired: 2 in, 4 out]
              }
              frame False {
              }
            }
          }
          frame "Minimize", "Minimized" {
            w2478 = T21."Minimized" ("State")
            n1170 = property on="Property Node" class="VI"(reference=w2484, error in=w2483) -> (reference out=w2481:refnum<vi>, error out=w2482:errorcluster, "FP.State"=w2480:T21)
            n1171 = Not Equal?(x=w2480, y=w2478) -> (x != y?=w2479:bool)
            n1172 = case shown="True" w2479 {
              tunnel: [w2489 w2490] -> w2485
              tunnel: w2482 -> [w2488 w2490]
              tunnel: w2481 -> [w2487 _]
              tunnel: w2478 -> [w2486 _]
              frame True {
                n1173 = invoke on="Invoke Node" class="VI" method="FP.Open"(reference=w2487, error in=w2488, "State"=w2486) -> (error out=w2489:errorcluster)  [unwired: 2 in, 4 out]
              }
              frame False {
              }
            }
          }
          frame "Maximize", "Maximized" {
            w2491 = T21."Maximized" ("State")
            n1174 = property on="Property Node" class="VI"(reference=w2497, error in=w2496) -> (reference out=w2494:refnum<vi>, error out=w2495:errorcluster, "FP.State"=w2493:T21)
            n1175 = Not Equal?(x=w2493, y=w2491) -> (x != y?=w2492:bool)
            n1176 = case shown="True" w2492 {
              tunnel: [w2502 w2503] -> w2498
              tunnel: w2495 -> [w2501 w2503]
              tunnel: w2494 -> [w2500 _]
              tunnel: w2491 -> [w2499 _]
              frame True {
                n1177 = invoke on="Invoke Node" class="VI" method="FP.Open"(reference=w2500, error in=w2501, "State"=w2499) -> (error out=w2502:errorcluster)  [unwired: 2 in, 4 out]
              }
              frame False {
              }
            }
          }
        }
        n1178 = call <vilib>:"Add State(s) to Queue__JKI_lib_State_Machine.vi"("State(s) in (\"\")"=w2438) -> ("States Out"=w2437:string)  [unwired: 14 in]
      }
      frame "---------- AimingBeam ----------" {
        # "Template Separator\n(You can make a copy of, or modify, this frame)"
        n1179 = call <vilib>:"Add State(s) to Queue__JKI_lib_State_Machine.vi"("State(s) in (\"\")"=w2508) -> ("States Out"=w2507:string)  [unwired: 14 in]
      }
      frame "AimingBeam: Initialize" {
        # "set aiming beam button color"
        # "Open COM port for Aiming Beam\n(Require USB connection)"
        n1180 = Unbundle By Name(w2510) -> ("AB Cluster.Aiming Beam COM Port"=w2518:refnum<visa-resource-name>)
        n1181 = call-poly "VISA Configure Serial Port"("VISA resource name"=w2518, "Enable Termination\nChar (T)"=TRUE ("Enable Termination\nChar (T)"), "baud rate (9600)"=u32 9600, "error in (no error)"=w2515) -> ("error out"=w2514:errorcluster)  [unwired: 10 in, 1 out]
        n1182 = Unbundle By Name(w2514) -> ("status"=w2513:bool)
        n1183 = Not(x=w2513) -> (.not. x?=w2512:bool)
        n1184 = Bundle By Name(cluster=w2510, "System Status.Aiming Beam"=w2512) -> (w2511:T26)
        n1185 = call <vilib>:"Add State(s) to Queue__JKI_lib_State_Machine.vi"("State(s) in (\"\")"=w2520) -> ("States Out"=w2519:string)  [unwired: 14 in]
      }
      frame "AimingBeam: Close" {
        # "Close Aiming Beam COM port\n(Require USB connection to Aiming Beam Laser)"
        n1186 = Unbundle By Name(w2523) -> ("AB Cluster.Aiming Beam COM Port"=w2527:refnum<visa-resource-name>)
        n1187 = VISA Close(VISA resource name=w2527, error in (no error)=w2525) -> (error out=w2526:errorcluster)
        n1188 = Bundle By Name(cluster=w2523, "System Status.Aiming Beam"=FALSE) -> (w2524:T26)
        n1189 = call <vilib>:"Add State(s) to Queue__JKI_lib_State_Machine.vi"("State(s) in (\"\")"=w2529) -> ("States Out"=w2528:string)  [unwired: 14 in]
      }
      frame "AimingBeam: Set Current" {
        # "Set Aiming Beam Current\n(You can make a copy of, or modify, this frame)"
        n1190 = Unbundle By Name(w2544) -> ("AB Cluster.Aiming Beam COM Port"=w2537:refnum<visa-resource-name>, "AB Cluster.Max Current"=w2533:dbl, "AB Cluster.Default Current"=w2535:dbl, "AB Cluster.Min Current"=w2534:dbl)
        n1191 = In Range and Coerce(upper limit=w2533, x=w2535, lower limit=w2534) -> (coerced(x)=w2530:dbl)  [unwired: 1 out]
        n1192 = Number To Fractional String(number=w2530, precision (6)=i16 2) -> (F-format string=w2538:string)  [unwired: 2 in]
        n1193 = Concatenate Strings("slc:", w2538, "\r" ("Carriage Return Constant"), "\n" ("Line Feed Constant")) -> (w2541:string)
        n1194 = VISA Write(VISA resource name=w2537, write buffer=w2541, error in (no error)=w2532) -> (error out=w2536:errorcluster)  [unwired: 2 out]
        n1195 = call <vilib>:"Add State(s) to Queue__JKI_lib_State_Machine.vi"("State(s) in (\"\")"=w2546) -> ("States Out"=w2545:string)  [unwired: 14 in]
      }
      frame "AimingBeam: Set Status" {
        # "Enable Aiming Beam\n(Usage: \"AimingBeam: Set >> Enable|Disable\")"
        n1196 = Unbundle By Name(w2553) -> ("AB Cluster.Aiming Beam COM Port"=w2550:refnum<visa-resource-name>)
        n1197 = case shown="\"Enable\"" w2552 {
          tunnel: [w2556 w2560] -> w2551
          frame "Disable", Default {
            n1198 = Concatenate Strings("cof", "\r" ("Carriage Return Constant"), "\n" ("Line Feed Constant")) -> (w2556:string)
          }
          frame "Enable" {
            n1199 = Concatenate Strings("con", "\r" ("Carriage Return Constant"), "\n" ("Line Feed Constant")) -> (w2560:string)
          }
        }
        n1200 = VISA Write(VISA resource name=w2550, write buffer=w2551, error in (no error)=w2548) -> (error out=w2549:errorcluster)  [unwired: 2 out]
        n1201 = call <vilib>:"Add State(s) to Queue__JKI_lib_State_Machine.vi"("State(s) in (\"\")"=w2555) -> ("States Out"=w2554:string)  [unwired: 14 in]
      }
      frame "AimingBeam: GetPWMStatus" {
        # "Get aiming beam PWM status\n()"
        n1202 = Unbundle By Name(w2568) -> ("AB Cluster.Freq"=w2567:i32, "LJ Pinout.AimingBeam PWM"=w2574:string)
        n1203 = Equal To 0?(x=w2567) -> (x = 0?=w2566:bool)
        n1204 = call "LabJack_FGV.vi"("Operation(Read)"=enum16{"Write", "Read"}."Read" ("Operation"), "error in (no error)"=w2570) -> ("error out"=w2572:errorcluster, "Read data"=w2573:i32)  [unwired: 8 in]
        n1205 = case shown="True" w2566 {
          tunnel: w2574 -> [w2587 _]
          tunnel: [w2585 "DIO_STATE"] -> w2571
          frame False {
            n1206 = Concatenate Strings(w2587, "_EF_ENABLE" ("string")) -> (w2585:string)
          }
          frame True {
          }
        }
        n1207 = call "LJM_eReadName.vi"("Handle In"=w2573, "Name"=w2571, "error in"=w2572) -> ("Value"=w2565:dbl, "error out"=w2569:errorcluster)  [unwired: 10 in, 1 out]
        n1208 = case shown="True" w2566 {
          tunnel: w2565 -> [w2580 w2584]
          tunnel: [w2579 w2581] -> w2564
          frame False {
            n1209 = Greater Than 0?(x=w2580) -> (x > 0?=w2579:bool)
          }
          frame True {
            n1210 = Number To Boolean Array(number=w2584) -> (Boolean array=w2583:bool[])
            n1211 = Index Array(array=w2583, index=3) -> (element=w2581:bool)
          }
        }
        n1212 = case shown="False" w2564 {
          frame False {
            # "PWM is off\nset color to dark green"
            n1213 = local write "Aiming beam toggle"(FALSE ("Aimging beam")) -> ()
          }
          frame True {
            # "PWM is on\nset color to light green"
            n1214 = local write "Aiming beam toggle"(TRUE ("Aimging beam")) -> ()
          }
        }
        n1215 = call <vilib>:"Add State(s) to Queue__JKI_lib_State_Machine.vi"("State(s) in (\"\")"=w2578) -> ("States Out"=w2577:string)  [unwired: 14 in]
      }
      frame "---------- 355 Laser ----------" {
        # "Template Separator\n(You can make a copy of, or modify, this frame)"
        n1216 = call <vilib>:"Add State(s) to Queue__JKI_lib_State_Machine.vi"("State(s) in (\"\")"=w2595) -> ("States Out"=w2594:string)  [unwired: 14 in]
      }
      frame "355 Laser: Check Dewelling" {
        # "if time laser start time is less than 7.5s before, wait 250ms then check again."
        # "Template Separator\n(You can make a copy of, or modify, this frame)"
        n1217 = Unbundle By Name(w2603) -> ("Laser start tic"=w2600:u32)
        n1218 = Tick Count (ms)() -> (millisecond timer value=w2601:u32)
        n1219 = Subtract(x=w2601, y=w2600) -> (x-y=w2599:u32)
        n1220 = Greater?(x=w2599, y=u32 5000) -> (0:w2597:bool)
        n1221 = case shown="False" w2597 {
          tunnel: ["355 Laser: Check Dewelling" ""] -> w2596
          frame False {
            n1222 = Wait (ms)(milliseconds to wait=u32 250) -> ()  [unwired: 1 out]
          }
          frame True {
          }
        }
        n1223 = call <vilib>:"Add State(s) to Queue__JKI_lib_State_Machine.vi"("State(s) in Front (\"\")"=w2596, "State(s) in (\"\")"=w2606) -> ("States Out"=w2605:string)  [unwired: 13 in]
      }
      frame "355 Laser: Laser enable" {
        # "Laser enable/disable\n(Usage: \"LabJack: Laser enable/disable >> 1|0\")"
        n1224 = Unbundle By Name(w2613) -> ("LJ Pinout.Laser Start/Stop"=w2617:string, "System Status.355 Laser"=w2611:bool)
        n1225 = case shown="False" w2611 {
          tunnel: w2610 -> [w2632 w2633]
          tunnel: w2617 -> [w2626 _]
          tunnel: [w2621 w2633] -> w2615
          tunnel: [w2620 u32 0 ("millisecond timer value")] -> w2612
          frame False {
            n1226 = call "LabJack_FGV.vi"("Operation(Read)"=enum16{"Write", "Read"}."Read" ("Operation")) -> ("Read data"=w2628:i32)  [unwired: 9 in, 1 out]
            n1227 = call "LJM_eWriteName.vi"("Handle In"=w2628, "Name"=w2626, "Value"=1.0, "error in"=w2632) -> ("Handle Out"=w2627:i32, "error out"=w2625:errorcluster)  [unwired: 10 in]
            n1228 = call <userlib>:"Wait (ms)__ogtk.vi"("error in (no error)"=w2625, "milliseconds to wait"=u32 250) -> ("error out"=w2624:errorcluster)  [unwired: 8 in, 1 out]
            n1229 = call "LJM_eWriteName.vi"("Handle In"=w2627, "Name"=w2626, "Value"=0.0, "error in"=w2624) -> ("error out"=w2622:errorcluster)  [unwired: 10 in, 1 out]
            n1230 = call <userlib>:"Tick Count (ms)__ogtk.vi"("error in (no error)"=w2622) -> ("error out"=w2621:errorcluster, "millisecond timer value"=w2620:u32)  [unwired: 9 in]
          }
          frame True {
          }
        }
        n1231 = Bundle By Name(cluster=w2613, "Laser start tic"=w2612) -> (w2614:T26)
        n1232 = call <vilib>:"Add State(s) to Queue__JKI_lib_State_Machine.vi"("State(s) in (\"\")"=w2619) -> ("States Out"=w2618:string)  [unwired: 14 in]
      }
      frame "355 Laser: Laser disable" {
        # "Laser enable/disable\n(Usage: \"LabJack: Laser enable/disable >> 1|0\")"
        n1233 = Unbundle By Name(w2637) -> ("LJ Pinout.Laser Start/Stop"=w2641:string, "System Status.355 Laser"=w2635:bool)
        n1234 = case shown="True" w2635 {
          tunnel: w2642 -> [w2645 w2659]
          tunnel: w2641 -> [_ w2653]
          tunnel: [w2645 w2648] -> w2639
          tunnel: [u32 0 ("millisecond timer value") w2647] -> w2636
          frame False {
          }
          frame True {
            n1235 = call "LabJack_FGV.vi"("Operation(Read)"=enum16{"Write", "Read"}."Read" ("Operation")) -> ("Read data"=w2655:i32)  [unwired: 9 in, 1 out]
            n1236 = call "LJM_eWriteName.vi"("Handle In"=w2655, "Name"=w2653, "Value"=1.0, "error in"=w2659) -> ("Handle Out"=w2654:i32, "error out"=w2652:errorcluster)  [unwired: 10 in]
            n1237 = call <userlib>:"Wait (ms)__ogtk.vi"("error in (no error)"=w2652, "milliseconds to wait"=u32 250) -> ("error out"=w2651:errorcluster)  [unwired: 8 in, 1 out]
            n1238 = call "LJM_eWriteName.vi"("Handle In"=w2654, "Name"=w2653, "Value"=0.0, "error in"=w2651) -> ("error out"=w2649:errorcluster)  [unwired: 10 in, 1 out]
            n1239 = call <userlib>:"Tick Count (ms)__ogtk.vi"("error in (no error)"=w2649) -> ("error out"=w2648:errorcluster, "millisecond timer value"=w2647:u32)  [unwired: 9 in]
          }
        }
        n1240 = Bundle By Name(cluster=w2637, "Laser start tic"=w2636) -> (w2638:T26)
        n1241 = call <vilib>:"Add State(s) to Queue__JKI_lib_State_Machine.vi"("State(s) in (\"\")"=w2644) -> ("States Out"=w2643:string)  [unwired: 14 in]
      }
      frame "355 Laser: Dewelling" {
        # "Wait some time (ms)\n(355 Laser: Dewelling >> #)"
        n1242 = Fract/Exp String To Number(string=w2663, default (0 dbl)=0) -> (number=w2661:i32)  [unwired: 2 in, 1 out]
        n1243 = Wait (ms)(milliseconds to wait=w2661) -> ()  [unwired: 1 out]
        n1244 = call <vilib>:"Add State(s) to Queue__JKI_lib_State_Machine.vi"("State(s) in (\"\")"=w2667) -> ("States Out"=w2666:string)  [unwired: 14 in]
      }
      frame "355 Laser: Close" {
        # "Template Separator\n(You can make a copy of, or modify, this frame)"
        n1245 = call <vilib>:"Add State(s) to Queue__JKI_lib_State_Machine.vi"("State(s) in Front (\"\")"="355 Laser: CheckControllerStatus\n355 Laser: Laser disable\n355 Laser: Dewelling >>1000", "State(s) in (\"\")"=w2673) -> ("States Out"=w2672:string)  [unwired: 13 in]
      }
      frame "355 Laser: CheckControllerStatus" {
        # "if average < 2, laser no power\nif average 2 < average < 9.3, laser on\nif 9.3<average<10, interlock open, blink indicator\nif average > 10, laser off\n[Covers: REQ30]"
        # "take 10 measuremt and look at average"
        # "Check 355 laser controller status\nBy probing Emisison Lamp negative terminal voltage"
        n1246 = Unbundle By Name(w2682) -> ("LJ Pinout.Laser Ready"=w2685:string)
        n1247 = call "LabJack_FGV.vi"("Operation(Read)"=enum16{"Write", "Read"}."Read" ("Operation")) -> ("Read data"=w2686:i32)  [unwired: 9 in, 1 out]
        n1248 = for {
          N: 20 -> [_]
          tunnel: w2686 -> [w2697]
          tunnel: w2685 -> [w2696]
          shift-right: [w2695] -> w2678
          shift-left: w2684 -> [w2694]
          tunnel: [w2692] -> w2677 mode=indexing
          n1249 = call "LJM_eReadName.vi"("Handle In"=w2697, "Name"=w2696, "error in"=w2694) -> ("Value"=w2692:dbl, "error out"=w2695:errorcluster)  [unwired: 10 in, 1 out]
          n1250 = Wait (ms)(milliseconds to wait=u32 25) -> ()  [unwired: 1 out]
        }
        n1251 = call "checkLaserStatus.vi"("error in (no error)"=w2678, "Laser LED voltage"=w2677) -> ("error out"=w2679:errorcluster, "Interlock open?"=w2674:bool, "Laser on?"=w2676:bool, "Mean voltage"=→"laser EM lamp V":dbl)  [unwired: 6 in]
        n1252 = Bundle By Name(cluster=w2682, "System Status.355 Laser"=w2676) -> (w2683:T26)
        n1253 = case shown="True" w2674 {
          frame False {
            n1254 = property on="355 Laser" class="Bool (strict)"("Blinking"=FALSE) -> ()  [unwired: 2 in, 2 out]
          }
          frame True {
            n1255 = property on="355 Laser" class="Bool (strict)"("Blinking"=TRUE) -> ()  [unwired: 2 in, 2 out]
          }
        }
        n1256 = call <vilib>:"Add State(s) to Queue__JKI_lib_State_Machine.vi"("State(s) in (\"\")"=w2689) -> ("States Out"=w2688:string)  [unwired: 14 in]
      }
      frame "355 Laser: CheckPWMStatus" {
        # "Check 355 laser PWM status\n(Read LJ DIO#EF_ENABLE register to determine PWM status)"
        n1257 = Unbundle By Name(w2707) -> ("LJ Pinout.355 PWM"=w2706:string)
        n1258 = call "LabJack_FGV.vi"("Operation(Read)"=enum16{"Write", "Read"}."Read" ("Operation"), "error in (no error)"=w2700) -> ("error out"=w2703:errorcluster, "Read data"=w2704:i32)  [unwired: 8 in]
        n1259 = Concatenate Strings(w2706, "_EF_ENABLE" ("string")) -> (w2702:string)
        n1260 = call "LJM_eReadName.vi"("Handle In"=w2704, "Name"=w2702, "error in"=w2703) -> ("Value"=w2699:dbl, "error out"=w2701:errorcluster)  [unwired: 10 in, 1 out]
        n1261 = Greater Than 0?(x=w2699) -> (x > 0?=w2698:bool)
        n1262 = case shown="False" w2698 {
          frame False {
            # "PWM is off\nset color to gray"
            n1263 = local write "355nm Laser toggle"(FALSE ("355nm Laser")) -> ()
          }
          frame True {
            # "PWM is on\nset color to light green"
            n1264 = local write "355nm Laser toggle"(TRUE ("355nm Laser")) -> ()
          }
        }
        n1265 = call <vilib>:"Add State(s) to Queue__JKI_lib_State_Machine.vi"("State(s) in (\"\")"=w2711) -> ("States Out"=w2710:string)  [unwired: 14 in]
      }
      frame "355 Laser: Start" {
        # "Template Separator\n(You can make a copy of, or modify, this frame)"
        n1266 = call <vilib>:"Add State(s) to Queue__JKI_lib_State_Machine.vi"("State(s) in Front (\"\")"="LabJack: 355_PWM_Start", "State(s) in (\"\")"=w2719) -> ("States Out"=w2718:string)  [unwired: 13 in]
      }
      frame "355 Laser: Stop" {
        # "Template Separator\n(You can make a copy of, or modify, this frame)"
        n1267 = call <vilib>:"Add State(s) to Queue__JKI_lib_State_Machine.vi"("State(s) in Front (\"\")"="LabJack: 355_PWM_Stop", "State(s) in (\"\")"=w2725) -> ("States Out"=w2724:string)  [unwired: 13 in]
      }
      frame "---------- Utility ----------" {
        # "Template Separator\n(You can make a copy of, or modify, this frame)"
        n1268 = call <vilib>:"Add State(s) to Queue__JKI_lib_State_Machine.vi"("State(s) in (\"\")"=w2730) -> ("States Out"=w2729:string)  [unwired: 14 in]
      }
      frame "Utility: SetDataClass" {
        # "Set Data Class in Queues\n(Set data class to either Data, Bg or Cali)"
        n1269 = case shown="\"Cali\"" w2732 {
          tunnel: [enum16{"Data", "BG", "Cali"}."Data" ("Data Class") enum16{"Data", "BG", "Cali"}."BG" ("Data Class") enum16{"Data", "BG", "Cali"}."Cali" ("Data Class")] -> w2731
          frame "Data", Default {
          }
          frame "Bg" {
          }
          frame "Cali" {
          }
        }
        n1270 = local write "Data Class"(w2731) -> ()
        n1271 = call <vilib>:"Add State(s) to Queue__JKI_lib_State_Machine.vi"("State(s) in (\"\")"=w2737) -> ("States Out"=w2736:string)  [unwired: 14 in]
      }
      frame "Utility: AquiTimerReset" {
        # "Set Aquisition Timer\n(You can make a copy of, or modify, this frame)"
        n1272 = Tick Count (ms)() -> (millisecond timer value=w2743:u32)
        n1273 = Bundle By Name(cluster=w2741, "Aquisition Timer"=w2743) -> (w2742:T26)
        n1274 = call <vilib>:"Add State(s) to Queue__JKI_lib_State_Machine.vi"("State(s) in (\"\")"=w2747) -> ("States Out"=w2746:string)  [unwired: 14 in]
      }
      frame "Utility: AquiTimerCheck" {
        # "5min to ms"
        # "Set Aquisition Timer\n([Covers: REQ35])"
        n1275 = Unbundle By Name(w2755) -> ("Aquisition Timer"=w2753:u32)
        n1276 = Tick Count (ms)() -> (millisecond timer value=w2754:u32)
        n1277 = Subtract(x=w2754, y=w2753) -> (x-y=w2752:u32)
        n1278 = Multiply(x=1000, y=300) -> (x*y=w2749:i32)
        n1279 = Greater Or Equal?(x=w2752, y=w2749) -> (x >= y?=w2748:bool)
        n1280 = case shown="True" w2748 {
          frame False {
            # "do nothing"
          }
          frame True {
            # "if timed out, stop aquisition"
            n1281 = property on="StopButton" class="Bool (strict)"("Val(Sgnl)"=TRUE ("Value (Signaling)")) -> ()  [unwired: 2 in, 2 out]
          }
        }
        n1282 = call <vilib>:"Add State(s) to Queue__JKI_lib_State_Machine.vi"("State(s) in (\"\")"=w2759) -> ("States Out"=w2758:string)  [unwired: 14 in]
      }
      frame "Utility: StartBeep" {
        # "Beep\n([Covers: REQ18])"
        n1283 = call <vilib>:"Beep.vi"("use system alert? (T)"=FALSE, "duration (msec)"=u32 1000, "frequency (Hz)"=u32 2000) -> ()  [unwired: 9 in]
        n1284 = call <vilib>:"Add State(s) to Queue__JKI_lib_State_Machine.vi"("State(s) in (\"\")"=w2768) -> ("States Out"=w2767:string)  [unwired: 14 in]
      }
      frame "Utility: EndBeep" {
        # "Beep\n([Covers: REQ18])"
        n1285 = flat-sequence {
          frame #0 {
            n1286 = call <vilib>:"Beep.vi"("use system alert? (T)"=FALSE, "duration (msec)"=u32 500, "frequency (Hz)"=u32 2000) -> ()  [unwired: 9 in]
          }
          frame #1 {
            n1287 = call <vilib>:"Beep.vi"("use system alert? (T)"=FALSE, "duration (msec)"=u32 500, "frequency (Hz)"=u32 2000) -> ()  [unwired: 9 in]
          }
        }
        n1288 = call <vilib>:"Add State(s) to Queue__JKI_lib_State_Machine.vi"("State(s) in (\"\")"=w2773) -> ("States Out"=w2772:string)  [unwired: 14 in]
      }
      frame "Utility: RestoreDeConChan" {
        # "Template Separator\n(You can make a copy of, or modify, this frame)"
        n1289 = global read "GlobalVariables.vi" "DeconChan Temp"() -> (w2780:T9)
        n1290 = local write "Radio Buttons"(w2780) -> ()
        n1291 = call <vilib>:"Add State(s) to Queue__JKI_lib_State_Machine.vi"("State(s) in (\"\")"=w2785) -> ("States Out"=w2784:string)  [unwired: 14 in]
      }
      frame "Utility: SaveDeconChan" {
        # "Save Decon Channel to global temp\n(You can make a copy of, or modify, this frame)"
        n1292 = flat-sequence {
          frame #0 {
            n1293 = local read "Radio Buttons"() -> (w2791:T9)
            n1294 = global write "GlobalVariables.vi" "DeconChan Temp"(w2791) -> ()
          }
          frame #1 {
            n1295 = local write "Radio Buttons"(T9."No Selection" ("Radio Buttons")) -> ()
          }
        }
        n1296 = flat-sequence {
          frame #0 {
          }
          frame #1 {
            (unwired) enum32{"No Selection", "Ch1", "Ch2", "Ch3"}."No Selection" ("Radio Buttons")
          }
        }
        n1297 = call <vilib>:"Add State(s) to Queue__JKI_lib_State_Machine.vi"("State(s) in (\"\")"=w2790) -> ("States Out"=w2789:string)  [unwired: 14 in]
      }
      frame "Utility: Dewelling" {
        # "Main loop dewell\n(Dewelling >> #)"
        n1298 = Fract/Exp String To Number(string=w2796, default (0 dbl)=0) -> (number=w2794:i32)  [unwired: 2 in, 1 out]
        n1299 = Wait (ms)(milliseconds to wait=w2794) -> ()  [unwired: 1 out]
        n1300 = call <vilib>:"Add State(s) to Queue__JKI_lib_State_Machine.vi"("State(s) in (\"\")"=w2800) -> ("States Out"=w2799:string)  [unwired: 14 in]
      }
      frame "Utility: SetAllChanManualGain" {
        w2801 = FALSE ("Value (Signaling)")
        # "Set all channel to manual gain\n(You can make a copy of, or modify, this frame)"
        n1301 = property on="Auto gain ch1" class="Bool (strict)"("Val(Sgnl)"=w2801) -> ()  [unwired: 2 in, 2 out]
        n1302 = property on="Auto gain ch2" class="Bool (strict)"("Val(Sgnl)"=w2801) -> ()  [unwired: 2 in, 2 out]
        n1303 = property on="Auto gain ch3" class="Bool (strict)"("Val(Sgnl)"=w2801) -> ()  [unwired: 2 in, 2 out]
        n1304 = property on="Auto gain ch4" class="Bool (strict)"("Val(Sgnl)"=w2801) -> ()  [unwired: 2 in, 2 out]
        n1305 = call <vilib>:"Add State(s) to Queue__JKI_lib_State_Machine.vi"("State(s) in (\"\")"=w2806) -> ("States Out"=w2805:string)  [unwired: 14 in]
      }
      frame "Utility: SetAllChanAutoGain" {
        w2807 = TRUE ("Value (Signaling)")
        # "Set all channels to auto gain\n(You can make a copy of, or modify, this frame)"
        n1306 = property on="Auto gain ch1" class="Bool (strict)"("Val(Sgnl)"=w2807) -> ()  [unwired: 2 in, 2 out]
        n1307 = property on="Auto gain ch2" class="Bool (strict)"("Val(Sgnl)"=w2807) -> ()  [unwired: 2 in, 2 out]
        n1308 = property on="Auto gain ch3" class="Bool (strict)"("Val(Sgnl)"=w2807) -> ()  [unwired: 2 in, 2 out]
        n1309 = property on="Auto gain ch4" class="Bool (strict)"("Val(Sgnl)"=w2807) -> ()  [unwired: 2 in, 2 out]
        n1310 = call <vilib>:"Add State(s) to Queue__JKI_lib_State_Machine.vi"("State(s) in (\"\")"=w2812) -> ("States Out"=w2811:string)  [unwired: 14 in]
      }
      frame "---------- SysLog ----------" {
        # "Template Separator\n(You can make a copy of, or modify, this frame)"
        n1311 = call <vilib>:"Add State(s) to Queue__JKI_lib_State_Machine.vi"("State(s) in (\"\")"=w2817) -> ("States Out"=w2816:string)  [unwired: 14 in]
      }
      frame "SysLog: OpenLogFile" {
        # "Template Separator\n(You can make a copy of, or modify, this frame)"
        n1312 = call <vilib>:"Add State(s) to Queue__JKI_lib_State_Machine.vi"("State(s) in (\"\")"=w2822) -> ("States Out"=w2821:string)  [unwired: 14 in]
      }
      frame "---------- Graph ----------" {
        # "Template Separator\n(You can make a copy of, or modify, this frame)"
        n1313 = call <vilib>:"Add State(s) to Queue__JKI_lib_State_Machine.vi"("State(s) in (\"\")"=w2827) -> ("States Out"=w2826:string)  [unwired: 14 in]
      }
      frame "Graph: SetXMultiplier" {
        # "Set X multiplier of WF graphs\n(You can make a copy of, or modify, this frame)"
        n1314 = call "Digitizer1_FGV.vi"() -> ("error out"=w2831:errorcluster, "Read data"=w2832:refnum<k15>)  [unwired: 10 in]
        n1315 = property class="niScope"(reference=w2832, error in=w2831) -> ("Min Sample Rate"=w2830:dbl)  [unwired: 2 out]
        n1316 = Divide(x=1.0, y=w2830) -> (x/y=w2828:dbl)
        n1317 = property on="Channel 1" class="WFGraph (strict)"("XScale.Multiplier"=w2828) -> ()  [unwired: 2 in, 2 out]
        n1318 = property on="Channel 2" class="WFGraph (strict)"("XScale.Multiplier"=w2828) -> ()  [unwired: 2 in, 2 out]
        n1319 = property on="Channel 3" class="WFGraph (strict)"("XScale.Multiplier"=w2828) -> ()  [unwired: 2 in, 2 out]
        n1320 = property on="Channel 4" class="WFGraph (strict)"("XScale.Multiplier"=w2828) -> ()  [unwired: 2 in, 2 out]
        n1321 = call <vilib>:"Add State(s) to Queue__JKI_lib_State_Machine.vi"("State(s) in (\"\")"=w2837) -> ("States Out"=w2836:string)  [unwired: 14 in]
      }
      frame "Graph: AddCursors" {
        # "Add BG and DC cursor to all graphs\n(You can make a copy of, or modify, this frame)"
        n1322 = property on="Channel 1" class="WFGraph (strict)"() -> ("XScale.Multiplier"=w2846:dbl)  [unwired: 2 in, 2 out]
        n1323 = global read "GlobalVariables.vi" "DC Idx1"() -> (w2845:i32)
        n1324 = global read "GlobalVariables.vi" "DC Idx2"() -> (w2844:i32)
        n1325 = global read "GlobalVariables.vi" "BG Idx1"() -> (w2843:i32)
        n1326 = global read "GlobalVariables.vi" "BG Idx2"() -> (w2842:i32)
        n1327 = property on="Channel 1" class="WFGraph (strict)"(error in=w2848) -> ("CrsrList"=w2857:T27)  [unwired: 1 in, 2 out]
        n1328 = property on="Channel 2" class="WFGraph (strict)"() -> ("CrsrList"=w2854:T27)  [unwired: 2 in, 2 out]
        n1329 = property on="Channel 3" class="WFGraph (strict)"() -> ("CrsrList"=w2853:T27)  [unwired: 2 in, 2 out]
        n1330 = property on="Channel 4" class="WFGraph (strict)"() -> ("CrsrList"=w2839:T27)  [unwired: 2 in, 2 out]
        n1331 = Build Array(w2845, w2844, w2843, w2842) -> (w2841:i32[])
        n1332 = Multiply(x=w2841, y=w2846) -> (x*y=w2840:dbl[])
        n1333 = for {
          tunnel: w2857 -> [w2871] mode=indexing
          tunnel: w2840 -> [w2864] mode=indexing
          tunnel: [w2870] -> w2856 mode=indexing
          tunnel: u32[] [6618880, 6618880, 16711680, 16711680] -> [w2863] mode=indexing
          tunnel: w2854 -> [w2869] mode=indexing
          tunnel: w2853 -> [w2868] mode=indexing
          tunnel: [w2867] -> w2852 mode=indexing
          tunnel: [w2866] -> w2851 mode=indexing
          tunnel: w2839 -> [w2865] mode=indexing
          tunnel: [w2862] -> w2838 mode=indexing
          n1334 = Bundle By Name(cluster=w2871, "Position.X"=w2864, "Color"=w2863) -> (w2870:T28)
          n1335 = Bundle By Name(cluster=w2869, "Position.X"=w2864, "Color"=w2863) -> (w2867:T28)
          n1336 = Bundle By Name(cluster=w2868, "Position.X"=w2864, "Color"=w2863) -> (w2866:T28)
          n1337 = Bundle By Name(cluster=w2865, "Position.X"=w2864, "Color"=w2863) -> (w2862:T28)
        }
        n1338 = property on="Channel 1" class="WFGraph (strict)"("CrsrList"=w2856) -> (error out=w2847:errorcluster)  [unwired: 2 in, 1 out]
        n1339 = property on="Channel 2" class="WFGraph (strict)"("CrsrList"=w2852) -> ()  [unwired: 2 in, 2 out]
        n1340 = property on="Channel 3" class="WFGraph (strict)"("CrsrList"=w2851) -> ()  [unwired: 2 in, 2 out]
        n1341 = property on="Channel 4" class="WFGraph (strict)"("CrsrList"=w2838) -> ()  [unwired: 2 in, 2 out]
        n1342 = control-ref of="Channel 1"() -> (w2850:refnum<vi>)
        n1343 = call <vilib>:"Add State(s) to Queue__JKI_lib_State_Machine.vi"("State(s) in (\"\")"=w2861) -> ("States Out"=w2860:string)  [unwired: 14 in]
        n1344 = call "UpdateCurserIdx(SubVI).vi"("error in (no error)"=w2847, "WaveformGraph in"=w2850) -> ("error out"=w2849:errorcluster)  [unwired: 9 in]
      }
      frame "Graph: SaveCursorLoc" {
        # "Save cursor location to ini file\n(Save cursor location to system setting ini file)"
        n1345 = global read "GlobalVariables.vi" "DC Idx1"() -> (w2878:i32)
        n1346 = global read "GlobalVariables.vi" "DC Idx2"() -> (w2877:i32)
        n1347 = global read "GlobalVariables.vi" "BG Idx1"() -> (w2876:i32)
        n1348 = global read "GlobalVariables.vi" "BG Idx2"() -> (w2875:i32)
        n1349 = Bundle("DC Idx1"=w2878, "DC Idx2"=w2877, "BG Idx1"=w2876, "BG Idx2"=w2875) -> (w2874:T49)  [unwired: 1 in]
        n1350 = call "writeCursorConfigMain.vi"("error in (no error)"=w2872, "Cursor Locations"=w2874) -> ("error out"=w2873:errorcluster)  [unwired: 9 in]
        n1351 = call <vilib>:"Add State(s) to Queue__JKI_lib_State_Machine.vi"("State(s) in (\"\")"=w2882) -> ("States Out"=w2881:string)  [unwired: 14 in]
      }
      frame "---------- APD ----------" {
        # "Template Separator\n(You can make a copy of, or modify, this frame)"
        n1352 = call <vilib>:"Add State(s) to Queue__JKI_lib_State_Machine.vi"("State(s) in (\"\")"=w2887) -> ("States Out"=w2886:string)  [unwired: 14 in]
      }
      frame "APD: Initialize" {
        w2894 = enum16{"Read", "Write"}."Write" ("Operation (Read)")
        w2893 = refnum<class "APDClass.lvclass"> refnum  # APDClass.lvclass
        # "Initialize APD FGV\n(Initialized APD FGV for holding data)"
        n1353 = call "APD1FGV.vi"("Error In"=w2888, "Operation (Read)"=w2894, "APDClass in"=w2893) -> ("Error Out"=w2892:errorcluster)  [unwired: 7 in, 1 out]
        n1354 = call "APD2FGV.vi"("Error In"=w2888, "Operation (Read)"=w2894, "APDClass in"=w2893) -> ("Error Out"=w2891:errorcluster)  [unwired: 7 in, 1 out]
        n1355 = call "APD3FGV.vi"("Error In"=w2888, "Operation (Read)"=w2894, "APDClass in"=w2893) -> ("Error Out"=w2890:errorcluster)  [unwired: 7 in, 1 out]
        n1356 = Merge Errors(w2892, w2891, w2890) -> (w2889:errorcluster)
        n1357 = call <vilib>:"Add State(s) to Queue__JKI_lib_State_Machine.vi"("State(s) in (\"\")"=w2898) -> ("States Out"=w2897:string)  [unwired: 14 in]
      }
      frame "APD: LoadFromSerial" {
        w2900 = enum16{"Read", "Write"}."Write" ("Operation (Read)")
        # "Load APD data from tdms file\n(load and update FGV)"
        n1358 = call "readAPDSerial.vi"("Error In"=w2907) -> ("Error Out"=w2903:errorcluster, "output cluster"=w2906:T29)  [unwired: 9 in]
        n1359 = Unbundle By Name(w2906) -> ("Ch1APDSerial#"=w2919:string, "Ch2APDSerial#"=w2905:string, "Ch3APDSerial#"=w2918:string, "Ch4APDSerial#"=w2904:string)
        n1360 = call "CreatFromSerialNumNoRaw.vi"("error in (no error)"=w2903, "APD Serial #"=w2919) -> ("error out"=w2916:errorcluster, "APDClass out"=w2917:refnum<class "APDClass.lvclass">)  [unwired: 8 in]
        n1361 = call "CreatFromSerialNumNoRaw.vi"("error in (no error)"=w2903, "APD Serial #"=w2905) -> ("error out"=w2914:errorcluster, "APDClass out"=w2915:refnum<class "APDClass.lvclass">)  [unwired: 8 in]
        n1362 = call "CreatFromSerialNumNoRaw.vi"("error in (no error)"=w2903, "APD Serial #"=w2918) -> ("error out"=w2912:errorcluster, "APDClass out"=w2913:refnum<class "APDClass.lvclass">)  [unwired: 8 in]
        n1363 = call "CreatFromSerialNumNoRaw.vi"("error in (no error)"=w2903, "APD Serial #"=w2904) -> ("error out"=w2901:errorcluster, "APDClass out"=w2902:refnum<class "APDClass.lvclass">)  [unwired: 8 in]
        n1364 = call "APD1FGV.vi"("Error In"=w2916, "Operation (Read)"=w2900, "APDClass in"=w2917) -> ("Error Out"=w2911:errorcluster)  [unwired: 7 in, 1 out]
        n1365 = call "APD2FGV.vi"("Error In"=w2914, "Operation (Read)"=w2900, "APDClass in"=w2915) -> ("Error Out"=w2909:errorcluster)  [unwired: 7 in, 1 out]
        n1366 = call "APD3FGV.vi"("Error In"=w2912, "Operation (Read)"=w2900, "APDClass in"=w2913) -> ("Error Out"=w2910:errorcluster)  [unwired: 7 in, 1 out]
        n1367 = call "APD4FGV.vi"("Error In"=w2901, "Operation (Read)"=w2900, "APDClass in"=w2902) -> ("Error Out"=w2899:errorcluster)  [unwired: 7 in, 1 out]
        n1368 = Merge Errors(w2911, w2909, w2910, w2899) -> (w2908:errorcluster)
        n1369 = call <vilib>:"Add State(s) to Queue__JKI_lib_State_Machine.vi"("State(s) in (\"\")"=w2923) -> ("States Out"=w2922:string)  [unwired: 14 in]
      }
      frame "APD: UpdateCtrlVLimit" {
        w2929 = enum16{"Read", "Write"}."Read" ("Operation (Read)")
        # "Set V limit\n(You can make a copy of, or modify, this frame)"
        n1370 = call "APD1FGV.vi"("Error In"=w2930, "Operation (Read)"=w2929) -> ("Error Out"=w2945:errorcluster, "APDClass out"=w2946:refnum<class "APDClass.lvclass">)  [unwired: 8 in]
        n1371 = call "APD2FGV.vi"("Error In"=w2930, "Operation (Read)"=w2929) -> ("Error Out"=w2943:errorcluster, "APDClass out"=w2944:refnum<class "APDClass.lvclass">)  [unwired: 8 in]
        n1372 = call "APD3FGV.vi"("Error In"=w2930, "Operation (Read)"=w2929) -> ("Error Out"=w2941:errorcluster, "APDClass out"=w2942:refnum<class "APDClass.lvclass">)  [unwired: 8 in]
        n1373 = call "APD4FGV.vi"("Error In"=w2930, "Operation (Read)"=w2929) -> ("Error Out"=w2927:errorcluster, "APDClass out"=w2928:refnum<class "APDClass.lvclass">)  [unwired: 8 in]
        n1374 = call-dynamic "ReadMaxCtrlV.vi"("error in (no error)"=w2945, "APDClass in"=w2946) -> ("error out"=w2936:errorcluster, "Numeric"=w2939:dbl)  [unwired: 7 in, 1 out]
        n1375 = call-dynamic "ReadMaxCtrlV.vi"("error in (no error)"=w2943, "APDClass in"=w2944) -> ("error out"=w2934:errorcluster, "Numeric"=w2938:dbl)  [unwired: 7 in, 1 out]
        n1376 = call-dynamic "ReadMaxCtrlV.vi"("error in (no error)"=w2941, "APDClass in"=w2942) -> ("error out"=w2932:errorcluster, "Numeric"=w2937:dbl)  [unwired: 7 in, 1 out]
        n1377 = call-dynamic "ReadMaxCtrlV.vi"("error in (no error)"=w2927, "APDClass in"=w2928) -> ("error out"=w2925:errorcluster, "Numeric"=w2926:dbl)  [unwired: 7 in, 1 out]
        n1378 = property on="V 1" class="DigNum (strict)"(error in=w2936, "Maximum"=w2939) -> (error out=w2935:errorcluster)  [unwired: 1 in, 1 out]
        n1379 = property on="V 2" class="DigNum (strict)"(error in=w2934, "Maximum"=w2938) -> (error out=w2933:errorcluster)  [unwired: 1 in, 1 out]
        n1380 = property on="V 4" class="DigNum (strict)"(error in=w2925, "Maximum"=w2926) -> (error out=w2924:errorcluster)  [unwired: 1 in, 1 out]
        n1381 = property on="V 3" class="DigNum (strict)"(error in=w2932, "Maximum"=w2937) -> (error out=w2931:errorcluster)  [unwired: 1 in, 1 out]
        n1382 = Merge Errors(w2935, w2933, w2931, w2924) -> (w2940:errorcluster)
        n1383 = call <vilib>:"Add State(s) to Queue__JKI_lib_State_Machine.vi"("State(s) in (\"\")"=w2950) -> ("States Out"=w2949:string)  [unwired: 14 in]
      }
      frame "APD: GetGainLimits" {
        w2955 = enum16{"Read", "Write"}."Read" ("Operation (Read)")
        # "Template Separator\n(You can make a copy of, or modify, this frame)"
        n1384 = call "APD1FGV.vi"("Error In"=w2956, "Operation (Read)"=w2955) -> ("Error Out"=w2961:errorcluster, "APDClass out"=w2962:refnum<class "APDClass.lvclass">)  [unwired: 8 in]
        n1385 = call "APD2FGV.vi"("Error In"=w2956, "Operation (Read)"=w2955) -> ("Error Out"=w2968:errorcluster, "APDClass out"=w2969:refnum<class "APDClass.lvclass">)  [unwired: 8 in]
        n1386 = call "APD3FGV.vi"("Error In"=w2956, "Operation (Read)"=w2955) -> ("Error Out"=w2966:errorcluster, "APDClass out"=w2967:refnum<class "APDClass.lvclass">)  [unwired: 8 in]
        n1387 = call "APD4FGV.vi"("Error In"=w2956, "Operation (Read)"=w2955) -> ("Error Out"=w2953:errorcluster, "APDClass out"=w2954:refnum<class "APDClass.lvclass">)  [unwired: 8 in]
        n1388 = call-dynamic "Read Gain Limits(Log).vi"("error in (no error)"=w2961, "APDClass in"=w2962) -> ("error out"=w2960:errorcluster, "GainLimits(Log)"=w2957:cluster{"GainMax":dbl, "GainMin":dbl})  [unwired: 7 in, 1 out]
        n1389 = call-dynamic "Read Gain Limits(Log).vi"("error in (no error)"=w2968, "APDClass in"=w2969) -> ("error out"=w2964:errorcluster, "GainLimits(Log)"=w2959:cluster{"GainMax":dbl, "GainMin":dbl})  [unwired: 7 in, 1 out]
        n1390 = call-dynamic "Read Gain Limits(Log).vi"("error in (no error)"=w2966, "APDClass in"=w2967) -> ("error out"=w2963:errorcluster, "GainLimits(Log)"=w2958:cluster{"GainMax":dbl, "GainMin":dbl})  [unwired: 7 in, 1 out]
        n1391 = call-dynamic "Read Gain Limits(Log).vi"("error in (no error)"=w2953, "APDClass in"=w2954) -> ("error out"=w2951:errorcluster, "GainLimits(Log)"=w2952:cluster{"GainMax":dbl, "GainMin":dbl})  [unwired: 7 in, 1 out]
        n1392 = Merge Errors(w2960, w2964, w2963, w2951) -> (w2965:errorcluster)
        n1393 = global write "GlobalVariables.vi" "Ch1GainLim(Log)"(w2957) -> ()
        n1394 = global write "GlobalVariables.vi" "Ch2GainLim(Log)"(w2959) -> ()
        n1395 = global write "GlobalVariables.vi" "Ch3GainLim(Log)"(w2958) -> ()
        n1396 = global write "GlobalVariables.vi" "Ch4GainLim(Log)"(w2952) -> ()
        n1397 = call <vilib>:"Add State(s) to Queue__JKI_lib_State_Machine.vi"("State(s) in (\"\")"=w2973) -> ("States Out"=w2972:string)  [unwired: 14 in]
      }
      frame "---------- TCP ----------" {
        # "Template Separator\n(You can make a copy of, or modify, this frame)"
        n1398 = call <vilib>:"Add State(s) to Queue__JKI_lib_State_Machine.vi"("State(s) in (\"\")"=w2978) -> ("States Out"=w2977:string)  [unwired: 14 in]
      }
      frame "TCP: InitializeNew" {
        # "if unsuccessful and count <10, increament count \nand try again"
        # "Initialize TCP connection to aimging beam computer\n(You can make a copy of, or modify, this frame)"
        n1399 = TCP Create Listener(10:u16 2100 ("port"), 11:"RTLT" ("service name")) -> (0:w2987:errorcluster, 3:w2979:refnum<k5>)  [unwired: 3 in, 1 out]
        n1400 = while {
          tunnel: w2979 -> [w3007]
          tunnel: w2987 -> [w3006]
          tunnel: [w2997] -> w2985
          tunnel: [w2994] -> w2981
          i -> [w3003]
          stop <- w2994 stop-if-true
          n1401 = TCP Wait On Listener(8:w3006, 9:200 ("timeout ms (wait forever: -1)"), 11:w3007) -> (0:w3004:errorcluster, 4:w3001:refnum<k5>)  [unwired: 1 in, 3 out]
          n1402 = Less Or Equal?(x=50, y=w3003) -> (x <= y?=w3000:bool)
          n1403 = case shown="No Error" w3004 {
            selector: w3004 -> [w3017 w3027]
            tunnel: w3001 -> [w3018 _]
            tunnel: [errorcluster {"status"=TRUE, "code"=0, "source"=""} ("No error") w3028] -> w2996
            tunnel: [w3009 FALSE ("TCP connected?")] -> w2997
            frame No Error {
              # "connection is ready, read data"
              n1404 = TCP Read(connection ID=w3018, bytes to read=512, error in (no error)=w3017, 7:T24."CRLF" ("mode (standard)"), 9:5000 ("timeout ms (25000)")) -> (connection ID out=w3011:refnum<k5>, data out=w3013:string, error out=w3010:errorcluster)
              n1405 = Concatenate Strings("alive" ("string"), "\r\n" ("End of Line Constant")) -> (w3014:string)
              n1406 = Equal?(x=w3014, y=w3013) -> (x = y?=w3012:bool)
              n1407 = case shown="False" w3012 {
                tunnel: w3011 -> [_ w3023]
                tunnel: w3010 -> [_ _]
                tunnel: [FALSE ("TCP connected?") TRUE ("TCP connected?")] -> w3009
                frame False {
                }
                frame True {
                  n1408 = call "TcpIDFGV.vi"("action"=enum16{"write", "read"}."write", "connection ID in"=w3023) -> ()  [unwired: 8 in, 2 out]
                }
              }
            }
            frame Error {
              # "connection not ready, keep waiting"
              n1409 = Unbundle By Name(w3027) -> ("code"=w3029:i32)
              n1410 = case shown="56" w3029 {
                tunnel: w3027 -> [w3030 _]
                tunnel: [w3030 w3031] -> w3028
                frame Default {
                }
                frame 56 {
                  w3031 = errorcluster {"status"=FALSE, "code"=0, "source"=""}  # No error
                }
              }
            }
          }
          n1411 = Select(t=errorcluster {"status"=TRUE, "code"=5001, "source"=""} ("error in (no error)"), s=w3000, f=errorcluster {"status"=FALSE, "code"=0, "source"=""} ("error in (no error)")) -> (s? t:f=w2995:errorcluster)
          n1412 = Merge Errors(w2996, w2995) -> (w2994:errorcluster)
        }
        n1413 = Unbundle By Name(w2981) -> ("code"=w2984:i32)
        n1414 = Bundle By Name(cluster=w2986, "System Status.TCP/IP"=w2985, "listener ID"=w2979) -> (w2991:T26)
        n1415 = global write "GlobalVariables.vi" "TCP connected?"(w2985) -> ()
        n1416 = Equal To 0?(x=w2984) -> (x = 0?=w2983:bool)
        n1417 = Select(t=errorcluster {"status"=FALSE, "code"=0, "source"=""} ("error in (no error)"), s=w2983, f=w2981) -> (s? t:f=w2980:errorcluster)
        n1418 = call <vilib>:"Add State(s) to Queue__JKI_lib_State_Machine.vi"("State(s) in (\"\")"=w2993) -> ("States Out"=w2992:string)  [unwired: 14 in]
      }
      frame "TCP: checkSource" {
        # "Check visualization PC video source\n(send !video_source message, listen for response, then parse it to binary mask)"
        n1419 = Unbundle By Name(w3038) -> ("System Status.TCP/IP"=w3041:bool)
        n1420 = case shown="True" w3041 {
          tunnel: w3040 -> [w3046 w3069]
          tunnel: [w3046 w3053] -> w3039
          tunnel: [w3045 w3058] -> w3036
          tunnel: [w3045 w3056] -> w3035
          tunnel: [w3045 w3057] -> w3034
          tunnel: [w3045 w3055] -> w3033
          tunnel: [w3045 w3047] -> w3032
          frame False {
            w3045 = FALSE
          }
          frame True {
            n1421 = call "TcpIDFGV.vi"("Error In"=w3069, "action"=enum16{"write", "read"}."read") -> ("Error Out"=w3066:errorcluster, "connection ID out"=w3068:refnum<k5>)  [unwired: 8 in]
            n1422 = call "TCP_WriteRead.vi"("error in (no error)"=w3066, "data in"="!video_source", "connectin ID in"=w3068) -> ("error out"=w3063:errorcluster, "data out"=w3065:string)  [unwired: 4 in, 1 out]
            n1423 = Scan From String(format string="!video_source:%d", input string=w3065, error in=w3063) -> (error out=w3054:errorcluster, output 1=w3052:i32)  [unwired: 2 in, 2 out]
            n1424 = case shown="5..7, 9..11, 13..15" w3052 {
              tunnel: w3054 -> [_ _ _ _]
              tunnel: [errorcluster {"status"=TRUE, "code"=5007, "source"="Visualization PC"} ("error out") errorcluster {"status"=FALSE, "code"=0, "source"=""} ("error out") errorcluster {"status"=FALSE, "code"=0, "source"=""} ("error out") errorcluster {"status"=FALSE, "code"=0, "source"=""} ("error out")] -> w3053
              tunnel: [FALSE FALSE FALSE TRUE] -> w3047
              frame 0, Default {
                # "No video source available or default"
                n1425 = property on="Video Source" class="RadioBtnsControl (strict)"("DisabledEnum"=T11."Disabled and Grayed Out" ("Disabled")) -> ()  [unwired: 2 in, 2 out]
              }
              frame 1..3 {
                # "one or both camera available"
                n1426 = local write "Video Source"(enum32{"Camera", "FrameGrabber"}."Camera" ("Video Source")) -> ()
                n1427 = property on="Video Source" class="RadioBtnsControl (strict)"("DisabledEnum"=T11."Disabled and Grayed Out" ("Disabled")) -> ()  [unwired: 2 in, 2 out]
              }
              frame 4, 8, 12 {
                # "one or both frame grabber available"
                n1428 = local write "Video Source"(enum32{"Camera", "FrameGrabber"}."FrameGrabber" ("Video Source")) -> ()
                n1429 = property on="Video Source" class="RadioBtnsControl (strict)"("DisabledEnum"=T11."Disabled and Grayed Out" ("Disabled")) -> ()  [unwired: 2 in, 2 out]
              }
              frame 5..7, 9..11, 13..15 {
                n1430 = property on="Video Source" class="RadioBtnsControl (strict)"("DisabledEnum"=T11."Enabled" ("Disabled")) -> ()  [unwired: 2 in, 2 out]
              }
            }
            n1431 = Integer to Fixed-Point Cast(fixed-point type=fxp<+,4,4> 0.0, integer=w3052) -> (fixed-point=w3051:fxp<+,4,4>)
            n1432 = Number To Boolean Array(number=w3051) -> (Boolean array=w3049:bool[])
            n1433 = Reverse 1D Array(array=w3049) -> (reversed array=w3048:bool[])
            n1434 = Index Array(array=w3048, index=0) -> (element=w3058:bool)
            n1435 = Index Array(array=w3048, index=1) -> (element=w3056:bool)
            n1436 = Index Array(array=w3048, index=2) -> (element=w3057:bool)
            n1437 = Index Array(array=w3048, index=3) -> (element=w3055:bool)
          }
        }
        n1438 = Bundle By Name(cluster=w3038, "video source.Main Frame Grabber"=w3036, "video source.Side Frame Grabber"=w3035, "video source.Main Camera"=w3034, "video source.Side Camera"=w3033, "bothVidSourceAvail"=w3032) -> (w3037:T26)
        n1439 = call <vilib>:"Add State(s) to Queue__JKI_lib_State_Machine.vi"("State(s) in (\"\")"=w3044) -> ("States Out"=w3043:string)  [unwired: 14 in]
      }
      frame "TCP: SyncTime" {
        # "Template Separator\n(You can make a copy of, or modify, this frame)"
        n1440 = Unbundle By Name(w3086) -> ("System Status.TCP/IP"=w3085:bool)
        n1441 = case shown="True" w3085 {
          tunnel: w3087 -> [_ w3095]
          frame False {
          }
          frame True {
            n1442 = call "TcpIDFGV.vi"("Error In"=w3095, "action"=enum16{"write", "read"}."read") -> ("Error Out"=w3094:errorcluster, "connection ID out"=w3091:refnum<k5>)  [unwired: 8 in]
            n1443 = call <userlib>:"Tick Count (ms)__ogtk.vi"("error in (no error)"=w3094) -> ("error out"=w3093:errorcluster, "millisecond timer value"=w3092:u32)  [unwired: 9 in]
            n1444 = while {
              tunnel: w3093 -> [w3115]
              tunnel: w3091 -> [w3114]
              tunnel: w3092 -> [w3103]
              stop <- w3098 stop-if-true
              n1445 = Concatenate Strings("latencycheck" ("string"), "\r\n" ("End of Line Constant")) -> (w3110:string)
              n1446 = TCP Read(connection ID=w3114, bytes to read=512, error in (no error)=w3115, 7:T24."CRLF" ("mode (standard)"), 9:2000 ("timeout ms (25000)")) -> (connection ID out=w3107:refnum<k5>, data out=w3105:string, error out=w3097:errorcluster)
              n1447 = Tick Count (ms)() -> (millisecond timer value=w3104:u32)
              n1448 = Subtract(x=w3104, y=w3103) -> (x-y=w3102:u32)
              n1449 = Equal?(x=w3105, y=w3110) -> (x = y?=w3106:bool)
              n1450 = case shown="False" w3106 {
                tunnel: w3107 -> [_ w3128]
                tunnel: w3105 -> [w3120 _]
                tunnel: [w3116 FALSE] -> w3100
                tunnel: w3097 -> [_ w3122]
                frame False {
                  n1451 = Concatenate Strings("synctimer" ("string"), "\r\n" ("End of Line Constant")) -> (w3117:string)
                  n1452 = Equal?(x=w3120, y=w3117) -> (x = y?=w3116:bool)
                  "Sync Success?" <- w3116
                }
                frame True {
                  n1453 = Concatenate Strings("latencycheck:" ("string"), "\r\n" ("End of Line Constant")) -> (w3127:string)
                  n1454 = TCP Write(connection ID=w3128, data in=w3127, error in (no error)=w3122, 9:1000 ("timeout ms (25000)")) -> (error out=w3121:errorcluster)  [unwired: 2 out]
                  n1455 = call <vilib>:"Clear Errors.vi"("error in (no error)"=w3121) -> ()  [unwired: 5 in, 2 out]
                }
              }
              n1456 = Greater?(x=w3102, y=u32 10000 ("x-y")) -> (0:w3099:bool)
              n1457 = Or(x=w3100, y=w3099) -> (x .or. y?=w3098:bool)
            }
          }
        }
        n1458 = call <vilib>:"Add State(s) to Queue__JKI_lib_State_Machine.vi"("State(s) in (\"\")"=w3090) -> ("States Out"=w3089:string)  [unwired: 14 in]
      }
      frame "TCP: SendSettingMacro" {
        # "Template Separator\n(You can make a copy of, or modify, this frame)"
        n1459 = Unbundle By Name(w3132) -> ("System Status.TCP/IP"=w3131:bool)
        n1460 = case shown="True" w3131 {
          tunnel: ["" ("Empty String Constant") "TCP: sendSubjectID\nTCP: sendScaleBarSetting\nTCP: sendScaleMaxMin\nTCP: sendDeconChannel\nTCP: sendANSI\nTCP: sendRadius\nTCP: send3Dsetting\nTCP: sendFirefly\nTCP: sendPentero"] -> w3130
          frame False {
          }
          frame True {
          }
        }
        n1461 = call <vilib>:"Add State(s) to Queue__JKI_lib_State_Machine.vi"("State(s) in Front (\"\")"=w3130, "State(s) in (\"\")"=w3135) -> ("States Out"=w3134:string)  [unwired: 13 in]
      }
      frame "TCP: sendRunNum" {
        # "Send run number to AB PC\n(You can make a copy of, or modify, this frame)"
        n1462 = Unbundle By Name(w3142) -> ("System Status.TCP/IP"=w3139:bool, "IDs.RunID"=w3143:i8)
        n1463 = Increment(x=w3143) -> (x+1=w3138:i8)
        n1464 = case shown="True" w3139 {
          tunnel: w3138 -> [_ w3157]
          tunnel: [w3147 w3149] -> w3141
          tunnel: w3140 -> [w3147 w3148]
          frame False {
          }
          frame True {
            n1465 = Number To Decimal String(number=w3157, width (-)=i16 3) -> (decimal integer string=w3152:string)
            n1466 = call "TcpIDFGV.vi"("Error In"=w3148, "action"=enum16{"write", "read"}."read") -> ("Error Out"=w3150:errorcluster, "connection ID out"=w3154:refnum<k5>)  [unwired: 8 in]
            n1467 = Concatenate Strings("!run:", w3152) -> (w3151:string)
            n1468 = call "TCP_WriteRead.vi"("error in (no error)"=w3150, "data in"=w3151, "connectin ID in"=w3154) -> ("error out"=w3149:errorcluster)  [unwired: 4 in, 2 out]
          }
        }
        n1469 = call <vilib>:"Add State(s) to Queue__JKI_lib_State_Machine.vi"("State(s) in (\"\")"=w3146) -> ("States Out"=w3145:string)  [unwired: 14 in]
      }
      frame "TCP: sendVideoSource" {
        # "Send video source \n(You can make a copy of, or modify, this frame)"
        n1470 = Unbundle By Name(w3159) -> ("System Status.TCP/IP"=w3158:bool)
        n1471 = case shown="True" w3158 {
          tunnel: [w3165 w3167] -> w3161
          tunnel: w3160 -> [w3165 w3166]
          frame False {
          }
          frame True {
            n1472 = case shown="\"Camera\", Default" "Video Source" {
              tunnel: [0 1] -> w3172
              frame "Camera", Default {
              }
              frame "FrameGrabber" {
              }
            }
            n1473 = call "TcpIDFGV.vi"("Error In"=w3166, "action"=enum16{"write", "read"}."read") -> ("Error Out"=w3168:errorcluster, "connection ID out"=w3174:refnum<k5>)  [unwired: 8 in]
            n1474 = Number To Decimal String(number=w3172) -> (decimal integer string=w3170:string)  [unwired: 1 in]
            n1475 = Concatenate Strings("!invivo:" ("data in"), w3170) -> (w3169:string)
            n1476 = call "TCP_WriteRead.vi"("error in (no error)"=w3168, "data in"=w3169, "connectin ID in"=w3174) -> ("error out"=w3167:errorcluster)  [unwired: 4 in, 2 out]
          }
        }
        n1477 = call <vilib>:"Add State(s) to Queue__JKI_lib_State_Machine.vi"("State(s) in (\"\")"=w3164) -> ("States Out"=w3163:string)  [unwired: 14 in]
      }
      frame "TCP: startRun" {
        # "Template Separator\n(You can make a copy of, or modify, this frame)"
        n1478 = Unbundle By Name(w3179) -> ("System Status.TCP/IP"=w3178:bool)
        n1479 = case shown="True" w3178 {
          tunnel: [w3185 w3187] -> w3181
          tunnel: w3180 -> [w3185 w3186]
          frame False {
          }
          frame True {
            n1480 = call "TcpIDFGV.vi"("Error In"=w3186, "action"=enum16{"write", "read"}."read") -> ("Error Out"=w3188:errorcluster, "connection ID out"=w3189:refnum<k5>)  [unwired: 8 in]
            n1481 = call "TCP_WriteRead.vi"("error in (no error)"=w3188, "data in"="!acquire:1", "connectin ID in"=w3189) -> ("error out"=w3187:errorcluster)  [unwired: 4 in, 2 out]
          }
        }
        n1482 = call <vilib>:"Add State(s) to Queue__JKI_lib_State_Machine.vi"("State(s) in (\"\")"=w3184) -> ("States Out"=w3183:string)  [unwired: 14 in]
      }
      frame "TCP: stopRun" {
        # "Send stop run to AB PC\n(You can make a copy of, or modify, this frame)"
        n1483 = Unbundle By Name(w3193) -> ("System Status.TCP/IP"=w3192:bool)
        n1484 = case shown="True" w3192 {
          tunnel: [w3199 w3201] -> w3195
          tunnel: w3194 -> [w3199 w3200]
          frame False {
            # "if not connected, do nothing"
          }
          frame True {
            # "If TCP connected, send stop run"
            n1485 = call "TcpIDFGV.vi"("Error In"=w3200, "action"=enum16{"write", "read"}."read") -> ("Error Out"=w3202:errorcluster, "connection ID out"=w3204:refnum<k5>)  [unwired: 8 in]
            n1486 = call "TCP_WriteRead.vi"("error in (no error)"=w3202, "data in"="!acquire:0", "connectin ID in"=w3204) -> ("error out"=w3201:errorcluster)  [unwired: 4 in, 2 out]
          }
        }
        n1487 = call <vilib>:"Add State(s) to Queue__JKI_lib_State_Machine.vi"("State(s) in (\"\")"=w3198) -> ("States Out"=w3197:string)  [unwired: 14 in]
      }
      frame "TCP: CheckConnection" {
        # "Check TCP/IP connection statuse\n(If connection is lost, throw error)"
        n1488 = Unbundle By Name(w3207) -> ("System Status.TCP/IP"=w3206:bool)
        n1489 = case shown="False" w3206 {
          frame False {
          }
          frame True {
            # "If TCP/IP is true check, otherwise skip"
          }
        }
        n1490 = call <vilib>:"Add State(s) to Queue__JKI_lib_State_Machine.vi"("State(s) in (\"\")"=w3211) -> ("States Out"=w3210:string)  [unwired: 14 in]
      }
      frame "TCP: sendSubjectID" {
        # "Send subject ID"
        n1491 = Unbundle By Name(w3213) -> ("System Status.TCP/IP"=w3212:bool, "CaseID"=w3216:string)
        n1492 = case shown="True" w3212 {
          tunnel: w3216 -> [_ w3227]
          tunnel: [w3220 w3222] -> w3215
          tunnel: w3214 -> [w3220 w3221]
          frame False {
          }
          frame True {
            n1493 = call "TcpIDFGV.vi"("Error In"=w3221, "action"=enum16{"write", "read"}."read") -> ("Error Out"=w3223:errorcluster, "connection ID out"=w3225:refnum<k5>)  [unwired: 8 in]
            n1494 = Concatenate Strings("!subject:", w3227) -> (w3224:string)
            n1495 = call "TCP_WriteRead.vi"("error in (no error)"=w3223, "data in"=w3224, "connectin ID in"=w3225) -> ("error out"=w3222:errorcluster)  [unwired: 4 in, 2 out]
          }
        }
        n1496 = call <vilib>:"Add State(s) to Queue__JKI_lib_State_Machine.vi"("State(s) in (\"\")"=w3219) -> ("States Out"=w3218:string)  [unwired: 14 in]
      }
      frame "TCP: sendScaleBarSetting" {
        # "Template Separator\n(You can make a copy of, or modify, this frame)"
        n1497 = Unbundle By Name(w3231) -> ("System Status.TCP/IP"=w3229:bool, "VideoConfig.Scale Bar"=w3230:bool)
        n1498 = case shown="True" w3229 {
          tunnel: [w3237 w3246] -> w3233
          tunnel: w3232 -> [w3237 w3245]
          tunnel: w3230 -> [_ w3244]
          frame False {
          }
          frame True {
            n1499 = Boolean To (0,1)(Boolean=w3244) -> (0, 1=w3243:i16)
            n1500 = call "TcpIDFGV.vi"("Error In"=w3245, "action"=enum16{"write", "read"}."read") -> ("Error Out"=w3247:errorcluster, "connection ID out"=w3248:refnum<k5>)  [unwired: 8 in]
            n1501 = Number To Fractional String(number=w3243, width (-)=i16 1, precision (6)=i16 0) -> (F-format string=w3241:string)  [unwired: 1 in]
            n1502 = Concatenate Strings("!autocolor:" ("data in"), w3241) -> (w3239:string)
            n1503 = call "TCP_WriteRead.vi"("error in (no error)"=w3247, "data in"=w3239, "connectin ID in"=w3248) -> ("error out"=w3246:errorcluster)  [unwired: 4 in, 2 out]
          }
        }
        n1504 = call <vilib>:"Add State(s) to Queue__JKI_lib_State_Machine.vi"("State(s) in (\"\")"=w3236) -> ("States Out"=w3235:string)  [unwired: 14 in]
      }
      frame "TCP: sendScaleMaxMin" {
        # "Send scale bar max and min to AB PC\n(You can make a copy of, or modify, this frame)"
        n1505 = Unbundle By Name(w3253) -> ("System Status.TCP/IP"=w3250:bool, "VideoConfig.Scale Low"=w3252:dbl, "VideoConfig.Scale High"=w3251:dbl)
        n1506 = case shown="True" w3250 {
          tunnel: [w3259 w3272] -> w3255
          tunnel: w3254 -> [w3259 w3271]
          tunnel: w3252 -> [_ w3270]
          tunnel: w3251 -> [_ w3261]
          frame False {
          }
          frame True {
            n1507 = call "TcpIDFGV.vi"("Error In"=w3271, "action"=enum16{"write", "read"}."read") -> ("Error Out"=w3273:errorcluster, "connection ID out"=w3274:refnum<k5>)  [unwired: 8 in]
            n1508 = Number To Fractional String(number=w3270, width (-)=i16 4, precision (6)=i16 2) -> (F-format string=w3266:string)  [unwired: 1 in]
            n1509 = Number To Fractional String(number=w3261, width (-)=i16 4, precision (6)=i16 2) -> (F-format string=w3262:string)  [unwired: 1 in]
            n1510 = Concatenate Strings("!color:" ("string"), w3266, ";" ("string"), w3262) -> (w3260:string)
            n1511 = call "TCP_WriteRead.vi"("error in (no error)"=w3273, "data in"=w3260, "connectin ID in"=w3274) -> ("error out"=w3272:errorcluster)  [unwired: 4 in, 2 out]
          }
        }
        n1512 = call <vilib>:"Add State(s) to Queue__JKI_lib_State_Machine.vi"("State(s) in (\"\")"=w3258) -> ("States Out"=w3257:string)  [unwired: 14 in]
      }
      frame "TCP: sendDeconChannel" {
        # "Send Decon channel\n(You can make a copy of, or modify, this frame)"
        n1513 = Unbundle By Name(w3277) -> ("System Status.TCP/IP"=w3276:bool)
        n1514 = case shown="True" w3276 {
          tunnel: [w3283 w3288] -> w3279
          tunnel: w3278 -> [w3283 w3287]
          frame False {
          }
          frame True {
            n1515 = local read "Radio Buttons"() -> (w3286:T9)
            n1516 = Increment(x=w3286) -> (x+1=w3285:T9)
            n1517 = Number To Decimal String(number=w3285) -> (decimal integer string=w3284:string)  [unwired: 1 in]
            n1518 = call "TcpIDFGV.vi"("Error In"=w3287, "action"=enum16{"write", "read"}."read") -> ("Error Out"=w3289:errorcluster, "connection ID out"=w3292:refnum<k5>)  [unwired: 8 in]
            n1519 = Concatenate Strings("!channel:", w3284) -> (w3290:string)
            n1520 = call "TCP_WriteRead.vi"("error in (no error)"=w3289, "data in"=w3290, "connectin ID in"=w3292) -> ("error out"=w3288:errorcluster)  [unwired: 4 in, 2 out]
          }
        }
        n1521 = call <vilib>:"Add State(s) to Queue__JKI_lib_State_Machine.vi"("State(s) in (\"\")"=w3282) -> ("States Out"=w3281:string)  [unwired: 14 in]
      }
      frame "TCP: sendANSI" {
        # "Template Separator\n(You can make a copy of, or modify, this frame)"
        n1522 = Unbundle By Name(w3296) -> ("System Status.TCP/IP"=w3294:bool, "VideoConfig.ANSI"=w3295:dbl)
        n1523 = case shown="True" w3294 {
          tunnel: [w3302 w3308] -> w3298
          tunnel: w3297 -> [w3302 w3307]
          tunnel: w3295 -> [_ w3306]
          frame False {
          }
          frame True {
            n1524 = Number To Fractional String(number=w3306) -> (F-format string=w3304:string)  [unwired: 3 in]
            n1525 = call "TcpIDFGV.vi"("Error In"=w3307, "action"=enum16{"write", "read"}."read") -> ("Error Out"=w3309:errorcluster, "connection ID out"=w3310:refnum<k5>)  [unwired: 8 in]
            n1526 = Concatenate Strings("!ansi:" ("data in"), w3304) -> (w3303:string)
            n1527 = call "TCP_WriteRead.vi"("error in (no error)"=w3309, "data in"=w3303, "connectin ID in"=w3310) -> ("error out"=w3308:errorcluster)  [unwired: 4 in, 2 out]
          }
        }
        n1528 = call <vilib>:"Add State(s) to Queue__JKI_lib_State_Machine.vi"("State(s) in (\"\")"=w3301) -> ("States Out"=w3300:string)  [unwired: 14 in]
      }
      frame "TCP: sendRadius" {
        # "Send drawing radius to AB PC\n(You can make a copy of, or modify, this frame)"
        n1529 = Unbundle By Name(w3314) -> ("System Status.TCP/IP"=w3312:bool, "VideoConfig.Radius"=w3313:dbl)
        n1530 = case shown="True" w3312 {
          tunnel: [w3320 w3326] -> w3316
          tunnel: w3315 -> [w3320 w3325]
          tunnel: w3313 -> [_ w3324]
          frame False {
          }
          frame True {
            n1531 = Number To Fractional String(number=w3324) -> (F-format string=w3323:string)  [unwired: 3 in]
            n1532 = Concatenate Strings("!radius:" ("data in"), w3323) -> (w3321:string)
            n1533 = call "TcpIDFGV.vi"("Error In"=w3325, "action"=enum16{"write", "read"}."read") -> ("Error Out"=w3327:errorcluster, "connection ID out"=w3328:refnum<k5>)  [unwired: 8 in]
            n1534 = call "TCP_WriteRead.vi"("error in (no error)"=w3327, "data in"=w3321, "connectin ID in"=w3328) -> ("error out"=w3326:errorcluster)  [unwired: 4 in, 2 out]
          }
        }
        n1535 = call <vilib>:"Add State(s) to Queue__JKI_lib_State_Machine.vi"("State(s) in (\"\")"=w3319) -> ("States Out"=w3318:string)  [unwired: 14 in]
      }
      frame "TCP: send3Dsetting" {
        # "Send 3D setting to AB computer\n(You can make a copy of, or modify, this frame)"
        n1536 = Unbundle By Name(w3332) -> ("System Status.TCP/IP"=w3330:bool, "VideoConfig.3D?"=w3331:bool)
        n1537 = case shown="True" w3330 {
          tunnel: [w3338 w3345] -> w3334
          tunnel: w3333 -> [w3338 w3344]
          tunnel: w3331 -> [_ w3343]
          frame False {
          }
          frame True {
            n1538 = Boolean To (0,1)(Boolean=w3343) -> (0, 1=w3342:i16)
            n1539 = Number To Fractional String(number=w3342) -> (F-format string=w3341:string)  [unwired: 3 in]
            n1540 = call "TcpIDFGV.vi"("Error In"=w3344, "action"=enum16{"write", "read"}."read") -> ("Error Out"=w3346:errorcluster, "connection ID out"=w3347:refnum<k5>)  [unwired: 8 in]
            n1541 = Concatenate Strings("!3dset:" ("data in"), w3341) -> (w3339:string)
            n1542 = call "TCP_WriteRead.vi"("error in (no error)"=w3346, "data in"=w3339, "connectin ID in"=w3347) -> ("error out"=w3345:errorcluster)  [unwired: 4 in, 2 out]
          }
        }
        n1543 = call <vilib>:"Add State(s) to Queue__JKI_lib_State_Machine.vi"("State(s) in (\"\")"=w3337) -> ("States Out"=w3336:string)  [unwired: 14 in]
      }
      frame "TCP: sendFirefly" {
        # "Template Separator\n(You can make a copy of, or modify, this frame)"
        n1544 = Unbundle By Name(w3350) -> ("System Status.TCP/IP"=w3349:bool)
        n1545 = case shown="False" w3349 {
          tunnel: [w3356 w3358] -> w3352
          tunnel: w3351 -> [w3356 w3357]
          frame False {
          }
          frame True {
            n1546 = call "TcpIDFGV.vi"("Error In"=w3357, "action"=enum16{"write", "read"}."read") -> ("Error Out"=w3359:errorcluster, "connection ID out"=w3361:refnum<k5>)  [unwired: 8 in]
            n1547 = call "TCP_WriteRead.vi"("error in (no error)"=w3359, "data in"="!firefly:0", "connectin ID in"=w3361) -> ("error out"=w3358:errorcluster)  [unwired: 4 in, 2 out]
          }
        }
        n1548 = call <vilib>:"Add State(s) to Queue__JKI_lib_State_Machine.vi"("State(s) in (\"\")"=w3355) -> ("States Out"=w3354:string)  [unwired: 14 in]
      }
      frame "TCP: sendPentero" {
        # "Send Pentero setting to AB computer\n(You can make a copy of, or modify, this frame)"
        n1549 = Unbundle By Name(w3364) -> ("System Status.TCP/IP"=w3363:bool)
        n1550 = case shown="True" w3363 {
          tunnel: [w3370 w3372] -> w3366
          tunnel: w3365 -> [w3370 w3371]
          frame False {
          }
          frame True {
            n1551 = call "TcpIDFGV.vi"("Error In"=w3371, "action"=enum16{"write", "read"}."read") -> ("Error Out"=w3373:errorcluster, "connection ID out"=w3375:refnum<k5>)  [unwired: 8 in]
            n1552 = call "TCP_WriteRead.vi"("error in (no error)"=w3373, "data in"="!pentero:0", "connectin ID in"=w3375) -> ("error out"=w3372:errorcluster)  [unwired: 4 in, 2 out]
          }
        }
        n1553 = call <vilib>:"Add State(s) to Queue__JKI_lib_State_Machine.vi"("State(s) in (\"\")"=w3369) -> ("States Out"=w3368:string)  [unwired: 14 in]
      }
      frame "TCP: sendChannel" {
        # "Send DeCon Channel to AB computer\n()"
        n1554 = Unbundle By Name(w3378) -> ("System Status.TCP/IP"=w3377:bool)
        n1555 = case shown="True" w3377 {
          tunnel: [w3384 w3388] -> w3380
          tunnel: w3379 -> [w3384 w3387]
          frame False {
          }
          frame True {
            n1556 = local read "Radio Buttons"() -> (w3386:T9)
            n1557 = case shown="\"No Selection\", Default" w3386 {
              tunnel: ["" ("data in") "!channel:1" ("data in") "!channel:2" ("data in") "!channel:3" ("data in")] -> w3385
              frame "No Selection", Default {
              }
              frame "Ch1" {
              }
              frame "Ch2" {
              }
              frame "Ch3" {
              }
            }
            n1558 = call "TcpIDFGV.vi"("Error In"=w3387, "action"=enum16{"write", "read"}."read") -> ("Error Out"=w3389:errorcluster, "connection ID out"=w3390:refnum<k5>)  [unwired: 8 in]
            n1559 = call "TCP_WriteRead.vi"("error in (no error)"=w3389, "data in"=w3385, "connectin ID in"=w3390) -> ("error out"=w3388:errorcluster)  [unwired: 4 in, 2 out]
          }
        }
        n1560 = call <vilib>:"Add State(s) to Queue__JKI_lib_State_Machine.vi"("State(s) in (\"\")"=w3383) -> ("States Out"=w3382:string)  [unwired: 14 in]
      }
      frame "TCP: startCam" {
        # "Send Pentero setting to AB computer\n(You can make a copy of, or modify, this frame)"
        n1561 = Unbundle By Name(w3397) -> ("System Status.TCP/IP"=w3396:bool)
        n1562 = case shown="True" w3396 {
          tunnel: [w3403 w3405] -> w3399
          tunnel: w3398 -> [w3403 w3404]
          frame False {
          }
          frame True {
            n1563 = call "TcpIDFGV.vi"("Error In"=w3404, "action"=enum16{"write", "read"}."read") -> ("Error Out"=w3406:errorcluster, "connection ID out"=w3408:refnum<k5>)  [unwired: 8 in]
            n1564 = call "TCP_WriteRead.vi"("error in (no error)"=w3406, "data in"="!focus:1", "connectin ID in"=w3408) -> ("error out"=w3405:errorcluster)  [unwired: 4 in, 2 out]
          }
        }
        n1565 = call <vilib>:"Add State(s) to Queue__JKI_lib_State_Machine.vi"("State(s) in (\"\")"=w3402) -> ("States Out"=w3401:string)  [unwired: 14 in]
      }
      frame "TCP: stopCam" {
        # "Send Pentero setting to AB computer\n(You can make a copy of, or modify, this frame)"
        n1566 = Unbundle By Name(w3411) -> ("System Status.TCP/IP"=w3410:bool)
        n1567 = case shown="True" w3410 {
          tunnel: [w3417 w3419] -> w3413
          tunnel: w3412 -> [w3417 w3418]
          frame False {
          }
          frame True {
            n1568 = call "TcpIDFGV.vi"("Error In"=w3418, "action"=enum16{"write", "read"}."read") -> ("Error Out"=w3420:errorcluster, "connection ID out"=w3422:refnum<k5>)  [unwired: 8 in]
            n1569 = call "TCP_WriteRead.vi"("error in (no error)"=w3420, "data in"="!focus:0", "connectin ID in"=w3422) -> ("error out"=w3419:errorcluster)  [unwired: 4 in, 2 out]
          }
        }
        n1570 = call <vilib>:"Add State(s) to Queue__JKI_lib_State_Machine.vi"("State(s) in (\"\")"=w3416) -> ("States Out"=w3415:string)  [unwired: 14 in]
      }
      frame "TCP: Close" {
        # "Close TCP connection\n()"
        n1571 = Unbundle By Name(w3426) -> ("System Status.TCP/IP"=w3424:bool)
        n1572 = case shown="True" w3424 {
          tunnel: [w3432 w3434] -> w3427
          tunnel: w3425 -> [w3432 w3433]
          frame False {
          }
          frame True {
            n1573 = call "TcpIDFGV.vi"("Error In"=w3433, "action"=enum16{"write", "read"}."read") -> ("Error Out"=w3436:errorcluster, "connection ID out"=w3437:refnum<k5>)  [unwired: 8 in]
            n1574 = TCP Close Connection(connection ID=w3437, error in (no error)=w3436) -> (error out=w3434:errorcluster)  [unwired: 1 in, 1 out]
          }
        }
        n1575 = case shown="Error .." w3427 {
          tunnel: [w3440 w3441] -> w3428
          tunnel: w3426 -> [w3439 w3441]
          frame No Error {
            w3438 = FALSE ("System Status.TCP/IP")
            n1576 = Bundle By Name(cluster=w3439, "System Status.TCP/IP"=w3438) -> (w3440:T26)
            n1577 = global write "GlobalVariables.vi" "TCP connected?"(w3438) -> ()
          }
          frame Error {
          }
        }
        n1578 = call <vilib>:"Add State(s) to Queue__JKI_lib_State_Machine.vi"("State(s) in (\"\")"=w3431) -> ("States Out"=w3430:string)  [unwired: 14 in]
      }
      frame "---------- PID ----------" {
        # "Template Separator\n(You can make a copy of, or modify, this frame)"
        n1579 = call <vilib>:"Add State(s) to Queue__JKI_lib_State_Machine.vi"("State(s) in (\"\")"=w3446) -> ("States Out"=w3445:string)  [unwired: 14 in]
      }
      frame "PID: loadPID" {
        # "Template Separator\n(You can make a copy of, or modify, this frame)"
        n1580 = call "readPIDSetting.vi"("Error In"=w3450) -> ("Error Out"=w3451:errorcluster, "Ch3 PID out"=w3447:T8, "Ch2 PID out"=w3448:T8, "Ch1 PID out"=w3449:T8)  [unwired: 7 in]
        n1581 = local write "Ch1 PID gains"(w3449) -> ()
        n1582 = local write "Ch2 PID gains"(w3448) -> ()
        n1583 = local write "Ch3 PID gains"(w3447) -> ()
        n1584 = local write "Ch4 PID gains"(w3447) -> ()
        n1585 = call <vilib>:"Add State(s) to Queue__JKI_lib_State_Machine.vi"("State(s) in (\"\")"=w3455) -> ("States Out"=w3454:string)  [unwired: 14 in]
      }
      frame "---------- Temp ----------" {
        # "Template Separator\n(You can make a copy of, or modify, this frame)"
        n1586 = call <vilib>:"Add State(s) to Queue__JKI_lib_State_Machine.vi"("State(s) in (\"\")"=w3460) -> ("States Out"=w3459:string)  [unwired: 14 in]
      }
    }
    n1587 = Not(x=w196) -> (.not. x?=w195:bool)
    n1588 = local write "ML?"(w195) -> ()
    "ML?" <- TRUE ("main loop running?")
  }
  n1589 = while {
    tunnel: w19 -> [w3498]
    tunnel: w18 -> [w3494]
    tunnel: [w3493] -> w17
    tunnel: w13 -> [w3490]
    tunnel: [w3489] -> w16
    shift-right: [w3482] -> _
    shift-left: _ -> [w3483]
    stop <- w3480 stop-if-true
    # "Read data from notifier and deconvolve it and send to Aiming Beam computer"
    n1590 = Wait on Notification(notifier=w3498, ignore previous (F)=FALSE) -> (notification=w3463:T14, error out=w3465:errorcluster)  [unwired: 2 in, 2 out]
    n1591 = Unbundle(w3463) -> ("idx"=w3470:i32, "CH1&2"=w3497:dbl[][], "CH3"=w3496:dbl[][], "V cluster"=w3461:cluster{"V1":dbl, "V2":dbl, "V3":dbl, "V4":dbl})
    n1592 = call "SeperateChanData.vi"("Input (Ch1&2)"=w3497) -> ("Ch1"=w3476:dbl[][], "Ch2"=w3474:dbl[][])
    n1593 = call "SeperateChanData.vi"("Input (Ch1&2)"=w3496) -> ("Ch1"=w3472:dbl[][], "Ch2"=w3469:dbl[][])
    n1594 = call "AvgArrayTimeCritical.vi"("2D array"=w3476) -> ("1D Avg"=w3475:dbl[])  [unwired: 10 in]
    n1595 = call "AvgArrayTimeCritical.vi"("2D array"=w3474) -> ("1D Avg"=w3473:dbl[])  [unwired: 10 in]
    n1596 = call "AvgArrayTimeCritical.vi"("2D array"=w3472) -> ("1D Avg"=w3471:dbl[])  [unwired: 10 in]
    n1597 = call "AvgArrayTimeCritical.vi"("2D array"=w3469) -> ("1D Avg"=w3468:dbl[])  [unwired: 10 in]
    n1598 = case shown="1" "Overlay selection" {
      tunnel: "Radio Buttons" -> [w3508 w3527]
      tunnel: [w3506 w3525] -> w3488
      tunnel: [w3504 w3524] -> w3487
      tunnel: [w3502 w3523] -> w3486
      tunnel: [w3509 w3522] -> w3480
      tunnel: w3475 -> [w3507 w3521]
      tunnel: w3473 -> [w3505 w3520]
      tunnel: w3471 -> [w3503 w3519]
      tunnel: w3468 -> [w3501 w3518]
      tunnel: [w3500 w3517] -> w3467
      tunnel: w3465 -> [w3509 w3516]
      tunnel: [w3499 w3515] -> w3464
      frame 0, Default {
        # "overlay gain"
        n1599 = case shown="\"No Selection\", Default" w3508 {
          tunnel: [0.0 ("Gain1") w3511 w3512 w3513 w3514] -> w3499
          frame "No Selection", Default {
          }
          frame "Ch1" {
            n1600 = local read "Gain1"() -> (w3511:dbl)
          }
          frame "Ch2" {
            n1601 = local read "Gain2"() -> (w3512:dbl)
          }
          frame "Ch3" {
            n1602 = local read "Gain3"() -> (w3513:dbl)
          }
          frame "Ch4" {
            n1603 = local read "Gain4"() -> (w3514:dbl)
          }
        }
        n1604 = Build Array(w3507) -> (w3506:dbl[][])
        n1605 = Build Array(w3505) -> (w3504:dbl[][])
        n1606 = Build Array(w3503) -> (w3502:dbl[][])
        n1607 = Build Array(w3501) -> (w3500:dbl[][])
      }
      frame 1 {
        # "overlay lifetime"
        n1608 = case shown="\"Ch1\"" w3527 {
          selector: w3527 -> [_ w3540 w3554 w3569 w3586]
          tunnel: w3521 -> [w3537 w3548 w3560 w3574 w3590]
          tunnel: w3520 -> [w3535 w3545 w3562 w3572 w3588]
          tunnel: w3519 -> [w3533 w3543 w3557 w3577 w3580]
          tunnel: FALSE -> [_ w3551 w3565 w3579 w3593]
          tunnel: w3516 -> [w3531 w3550 w3564 w3568 w3585]
          tunnel: [w3531 w3549 w3563 w3578 w3592] -> w3522
          tunnel: [w3536 w3546 w3558 w3573 w3589] -> w3525
          tunnel: [w3534 w3544 w3559 w3571 w3587] -> w3524
          tunnel: [w3532 w3542 w3556 w3575 w3581] -> w3523
          tunnel: [0.0 ("lifetime (ns)") w3541 w3555 w3570 w3584] -> w3515
          tunnel: w3518 -> [w3529 w3539 w3553 w3567 w3583]
          tunnel: [w3528 w3538 w3552 w3566 w3582] -> w3517
          frame "No Selection", Default {
            n1609 = Build Array(w3537) -> (w3536:dbl[][])
            n1610 = Build Array(w3535) -> (w3534:dbl[][])
            n1611 = Build Array(w3533) -> (w3532:dbl[][])
            n1612 = Build Array(w3529) -> (w3528:dbl[][])
          }
          frame "Ch1" {
            n1613 = call "Deconvolution.vi"("DeconChannel"=w3540, "iRF align"=w3551, "error in (no error)"=w3550, "Waveform"=w3548) -> ("error out"=w3549:errorcluster, "lifetime (ns)"=w3541:dbl, "Fitting"=w3547:dbl[])  [unwired: 5 in]
            "Lifetime 1" <- w3541
            n1614 = Build Array(w3548, w3547) -> (w3546:dbl[][])
            n1615 = Build Array(w3545) -> (w3544:dbl[][])
            n1616 = Build Array(w3543) -> (w3542:dbl[][])
            n1617 = Build Array(w3539) -> (w3538:dbl[][])
          }
          frame "Ch2" {
            n1618 = call "Deconvolution.vi"("DeconChannel"=w3554, "iRF align"=w3565, "error in (no error)"=w3564, "Waveform"=w3562) -> ("error out"=w3563:errorcluster, "lifetime (ns)"=w3555:dbl, "Fitting"=w3561:dbl[])  [unwired: 5 in]
            "Lifetime 2" <- w3555
            n1619 = Build Array(w3560) -> (w3558:dbl[][])
            n1620 = Build Array(w3562, w3561) -> (w3559:dbl[][])
            n1621 = Build Array(w3557) -> (w3556:dbl[][])
            n1622 = Build Array(w3553) -> (w3552:dbl[][])
          }
          frame "Ch3" {
            n1623 = call "Deconvolution.vi"("DeconChannel"=w3569, "iRF align"=w3579, "error in (no error)"=w3568, "Waveform"=w3577) -> ("error out"=w3578:errorcluster, "lifetime (ns)"=w3570:dbl, "Fitting"=w3576:dbl[])  [unwired: 5 in]
            "Lifetime 3" <- w3570
            n1624 = Build Array(w3574) -> (w3573:dbl[][])
            n1625 = Build Array(w3572) -> (w3571:dbl[][])
            n1626 = Build Array(w3577, w3576) -> (w3575:dbl[][])
            n1627 = Build Array(w3567) -> (w3566:dbl[][])
          }
          frame "Ch4" {
            n1628 = call "Deconvolution.vi"("DeconChannel"=w3586, "iRF align"=w3593, "error in (no error)"=w3585, "Waveform"=w3583) -> ("error out"=w3592:errorcluster, "lifetime (ns)"=w3584:dbl, "Fitting"=w3591:dbl[])  [unwired: 5 in]
            "Lifetime 4" <- w3584
            n1629 = Build Array(w3590) -> (w3589:dbl[][])
            n1630 = Build Array(w3588) -> (w3587:dbl[][])
            n1631 = Build Array(w3583, w3591) -> (w3582:dbl[][])
            n1632 = Build Array(w3580) -> (w3581:dbl[][])
          }
        }
      }
    }
    "Lifetime (ns)" <- w3464
    n1633 = Bundle(w3488, w3487, w3486, w3467, "V cluster"=w3461) -> (w3491:T50)  [unwired: 1 in]
    n1634 = Bundle("idx"=w3470, "lifetime (ns)"=w3464) -> (w3495:cluster{"idx":i32, "lifetime (ns)":dbl})  [unwired: 1 in]
    n1635 = flat-sequence {
      tunnel: [w3594] -> w3482
      tunnel: w3465 -> [_]
      frame #0 {
        n1636 = call <vilib>:"High Resolution Relative Seconds.vi"() -> ("relative seconds"=w3594:dbl)
      }
    }
    n1637 = Subtract(x=w3482, y=w3483) -> (x-y=w3485:dbl)
    n1638 = Multiply(x=w3485, y=1000.0) -> (x*y=→"Decon Loop timing (ms)" →"DeCon Speed(ms)":dbl)
    n1639 = Send Notification(notification=w3491, notifier=w3490, error in (no error)=w3480) -> (notifier out=w3489:refnum<notifier>, error out=w3479:errorcluster)
    n1640 = Send Notification(notification=w3495, notifier=w3494, error in (no error)=w3480) -> (notifier out=w3493:refnum<notifier>, error out=w3478:errorcluster)
    n1641 = Merge Errors(w3479, w3478) -> (→"decon error out":errorcluster)
  }
  n1642 = while {
    tunnel: w18 -> [w3605]
    shift-right: [w3598] -> _
    shift-left: u32 0 -> [w3599]
    stop <- w3596 stop-if-true
    # "Send data to AB computer here"
    # "if TCP ip is not open loop will run once and stop. To re-establish connection and start this loop. Reboot softwrae."
    # "Data communication loop"
    n1643 = Tick Count (ms)() -> (millisecond timer value=w3598:u32)
    n1644 = Wait on Notification(notifier=w3605, ignore previous (F)=FALSE) -> (notification=w3603:cluster{"idx":i32, "lifetime":dbl}, error out=w3597:errorcluster)  [unwired: 2 in, 2 out]
    n1645 = Unbundle(w3603) -> ("idx"=w3602:i32, "lifetime"=w3601:dbl)
    n1646 = global read "GlobalVariables.vi" "TCP connected?"() -> (w3595:bool)
    n1647 = Subtract(x=w3598, y=w3599) -> (x-y=→"Communication loop(ms)":u32)
    n1648 = case shown="True" w3595 {
      tunnel: w3602 -> [_ w3614]
      tunnel: w3601 -> [_ w3613]
      tunnel: w3597 -> [w3606 w3610]
      tunnel: [w3606 w3607] -> w3596
      frame False {
      }
      frame True {
        n1649 = Number To Decimal String(number=w3614) -> (decimal integer string=w3622:string)  [unwired: 1 in]
        n1650 = call "TcpIDFGV.vi"("Error In"=w3610, "action"=enum16{"write", "read"}."read") -> ("Error Out"=w3609:errorcluster, "connection ID out"=w3620:refnum<k5>)  [unwired: 8 in]
        n1651 = Concatenate Strings("!idx:", w3622) -> (w3623:string)
        n1652 = call "TCP_WriteRead.vi"("error in (no error)"=w3609, "data in"=w3623, "connectin ID in"=w3620) -> ("error out"=w3608:errorcluster, "connectin ID out"=w3621:refnum<k5>)  [unwired: 4 in, 1 out]
        n1653 = Number To Fractional String(number=w3613, precision (6)=i16 2) -> (F-format string=w3612:string)  [unwired: 2 in]
        n1654 = Concatenate Strings("!lifetime:", w3612) -> (w3619:string)
        n1655 = call "TCP_WriteRead.vi"("error in (no error)"=w3608, "data in"=w3619, "connectin ID in"=w3621) -> ("error out"=w3607:errorcluster, "data out"=→"data out(communcation loop)":string)  [unwired: 4 in, 1 out]
      }
    }
  }
  n1656 = while {
    tunnel: w13 -> [w3634]
    shift-right: [w3625] -> _
    shift-left: w15 -> [w3632]
    shift-right: [w3627] -> _
    shift-left: w15 -> [w3626]
    i -> [w3628]
    stop <- w3629 stop-if-true
    # "Data display loop(30Hz)"
    n1657 = Wait on Notification(notifier=w3634, ignore previous (F)=FALSE) -> (notification=w3630:T13, error out=w3629:errorcluster)  [unwired: 2 in, 2 out]
    n1658 = Wait Until Next ms Multiple(millisecond multiple=u32 33) -> ()  [unwired: 1 out]
    n1659 = Tick Count (ms)() -> (millisecond timer value=w3625:u32)
    n1660 = Subtract(x=w3625, y=w3632) -> (x-y=→"display loop timing(ms)":u32)
    n1661 = case shown="No Error" w3629 {
      tunnel: w3630 -> [w3707 _]
      tunnel: w3626 -> [w3679 w3779]
      tunnel: [w3681 w3779] -> w3627
      tunnel: w3625 -> [w3678 _]
      frame No Error {
        w3636 = u32 1 ("Active Plot")
        w3655 = 0 ("index (row)")
        n1662 = Subtract(x=w3678, y=w3679) -> (x-y=w3680:u32)
        n1663 = Unbundle(w3707) -> ("CH1"=w3702:dbl[][], "CH2"=w3700:dbl[][], "CH3"=w3697:dbl[][], "CH4"=w3650:dbl[][], "Gain cluster"=w3656:cluster{"V1":dbl, "V2":dbl, "V3":dbl, "V4":dbl})
        n1664 = Unbundle By Name(w3656) -> ("V1"=w3674:dbl, "V2"=w3672:dbl, "V3"=w3670:dbl, "V4"=w3648:dbl)
        n1665 = Index Array(array=w3702, index (row)=w3655) -> (element=w3686:dbl[])  [unwired: 1 in]
        n1666 = Index Array(array=w3700, index (row)=w3655) -> (element=w3684:dbl[])  [unwired: 1 in]
        n1667 = Index Array(array=w3697, index (row)=w3655) -> (element=w3685:dbl[])  [unwired: 1 in]
        n1668 = Index Array(array=w3650, index (row)=w3655) -> (element=w3654:dbl[])  [unwired: 1 in]
        n1669 = call "RemoveDCBG.vi"("Channel"=enum16{"DC Only", "Ch1", "Ch2", "Ch3", "Ch4"}."Ch4", "WF in"=w3654) -> ("DC"=w3652:dbl, "WF out"=w3641:dbl[])  [unwired: 7 in, 1 out]
        n1670 = Greater?(x=w3680, y=u32 200) -> (0:w3682:bool)
        n1671 = call "CtrlVtoGain.vi"("CtrlV(V)"=w3648, "Channel"=enum16{"Ch1", "Ch2", "Ch3", "Ch4"}."Ch4") -> ("Gain"=w3640:dbl)  [unwired: 8 in, 1 out]
        n1672 = call "CtrlVtoGain.vi"("CtrlV(V)"=w3674, "Channel"=enum16{"Ch1", "Ch2", "Ch3"}."Ch1") -> ("Gain"=w3668:dbl)  [unwired: 8 in, 1 out]
        n1673 = call "RemoveDCBG.vi"("Channel"=enum16{"DC Only", "Ch1", "Ch2", "Ch3"}."Ch1", "WF in"=w3686) -> ("DC"=w3703:dbl, "WF out"=w3675:dbl[])  [unwired: 7 in, 1 out]
        n1674 = call "RemoveDCBG.vi"("Channel"=enum16{"DC Only", "Ch1", "Ch2", "Ch3"}."Ch2", "WF in"=w3684) -> ("DC"=w3699:dbl, "WF out"=w3676:dbl[])  [unwired: 7 in, 1 out]
        n1675 = call "CtrlVtoGain.vi"("CtrlV(V)"=w3672, "Channel"=enum16{"Ch1", "Ch2", "Ch3"}."Ch2") -> ("Gain"=w3663:dbl)  [unwired: 8 in, 1 out]
        n1676 = call "RemoveDCBG.vi"("Channel"=enum16{"DC Only", "Ch1", "Ch2", "Ch3"}."Ch3", "WF in"=w3685) -> ("DC"=w3696:dbl, "WF out"=w3677:dbl[])  [unwired: 7 in, 1 out]
        n1677 = call "CtrlVtoGain.vi"("CtrlV(V)"=w3670, "Channel"=enum16{"Ch1", "Ch2", "Ch3"}."Ch3") -> ("Gain"=w3659:dbl)  [unwired: 8 in, 1 out]
        n1678 = formula code="int32 out = 2;\nif (G<5){\nout = 1;\n}\nif (G>200){\nout = 3;\n}"("G"=w3640) -> ("out"=→"output variable":i32)
        n1679 = Add(x=w3641, y=w3652) -> (x+y=w3651:dbl[])
        n1680 = Less?(x=w3640, y=5.0) -> (x < y?=w3646:bool)
        n1681 = case shown="True" w3682 {
          tunnel: w3675 -> [_ w3736]
          tunnel: w3676 -> [_ w3739]
          tunnel: w3677 -> [_ w3738]
          tunnel: w3678 -> [_ w3754]
          tunnel: [w3718 w3754] -> w3681
          tunnel: w3679 -> [w3718 _]
          tunnel: w3668 -> [_ w3732]
          tunnel: w3663 -> [_ w3731]
          tunnel: w3659 -> [_ w3730]
          tunnel: w3641 -> [_ w3726]
          tunnel: w3640 -> [_ w3723]
          frame False {
          }
          frame True {
            n1682 = call "GetSNR(SubVI).vi"("Waveform"=w3736) -> ("SNR"=→"SNR1":dbl)  [unwired: 10 in]
            n1683 = Array Size(array=w3736) -> (size(s)=w3737:i32)
            n1684 = call "GetSNR(SubVI).vi"("Waveform"=w3739) -> ("SNR"=→"SNR2":dbl)  [unwired: 10 in]
            n1685 = call "GetSNR(SubVI).vi"("Waveform"=w3738) -> ("SNR"=→"SNR3":dbl)  [unwired: 10 in]
            n1686 = call "GetSNR(SubVI).vi"("Waveform"=w3726) -> ("SNR"=→"SNR4":dbl)  [unwired: 10 in]
            n1687 = global read "GlobalVariables.vi" "BG Idx2"() -> (w3725:i32)
            n1688 = Subtract(x=w3737, y=w3725) -> (x-y=w3724:i32)
            n1689 = Array Subset(array=w3736, index=w3725, length=w3724) -> (w3743:dbl[])
            n1690 = Array Subset(array=w3739, index=w3725, length=w3724) -> (w3745:dbl[])
            n1691 = Array Subset(array=w3738, index=w3725, length=w3724) -> (w3747:dbl[])
            n1692 = Array Subset(array=w3726, index=w3725, length=w3724) -> (w3727:dbl[])
            n1693 = Add Array Elements(numeric array=w3743) -> (sum=w3744:dbl)
            n1694 = Add Array Elements(numeric array=w3745) -> (sum=w3746:dbl)
            n1695 = Add Array Elements(numeric array=w3747) -> (sum=w3748:dbl)
            n1696 = Add Array Elements(numeric array=w3727) -> (sum=w3728:dbl)
            n1697 = Divide(x=w3744, y=w3732) -> (x/y=w3749:dbl)
            n1698 = Divide(x=w3746, y=w3731) -> (x/y=w3750:dbl)
            n1699 = Divide(x=w3748, y=w3730) -> (x/y=w3751:dbl)
            n1700 = Divide(x=w3728, y=w3723) -> (x/y=w3722:dbl)
            n1701 = Build Array(w3749, w3750, w3751, w3722) -> (w3752:dbl[])
            n1702 = Add Array Elements(numeric array=w3752) -> (sum=w3753:dbl)
            n1703 = Divide(x=w3752, y=w3753) -> (x/y=w3721:dbl[])
            n1704 = Index Array(array=w3721, index=2) -> (element=→"IntR3":dbl)
            n1705 = Index Array(array=w3721, index=1) -> (element=→"IntR2":dbl)
            n1706 = Index Array(array=w3721, index=0) -> (element=→"IntR1":dbl)
            n1707 = Index Array(array=w3721, index=3) -> (element=→"IntR4":dbl)
          }
        }
        n1708 = Add(x=w3675, y=w3703) -> (x+y=w3701:dbl[])
        n1709 = Add(x=w3676, y=w3699) -> (x+y=w3698:dbl[])
        n1710 = Add(x=w3677, y=w3696) -> (x+y=w3695:dbl[])
        n1711 = Less?(x=w3668, y=5.0 ("x")) -> (x < y?=w3666:bool)
        n1712 = Less?(x=w3663, y=5.0 ("x")) -> (x < y?=w3662:bool)
        n1713 = Less?(x=w3659, y=5.0 ("x")) -> (x < y?=w3658:bool)
        n1714 = case shown="False" w3658 {
          tunnel: [u32 16448250 ("Plot.Plot Color") u32 16711680 ("Plot.Plot Color")] -> w3657
          frame False {
          }
          frame True {
          }
        }
        n1715 = case shown="True" "Show BG removed?" {
          tunnel: w3702 -> [w3761 w3777]
          tunnel: w3701 -> [_ w3767]
          tunnel: [w3761 w3776] -> w3694
          tunnel: w3700 -> [w3760 w3775]
          tunnel: [w3760 w3774] -> w3638
          tunnel: w3698 -> [_ w3763]
          tunnel: w3697 -> [w3759 w3773]
          tunnel: [w3759 w3772] -> w3689
          tunnel: w3695 -> [_ w3768]
          tunnel: [w3758 w3771] -> w3645
          tunnel: w3651 -> [_ w3765]
          tunnel: w3650 -> [w3758 w3770]
          frame False {
          }
          frame True {
            n1716 = Insert Into Array(array=w3773, index (row)=1, new element=w3768) -> (w3772:dbl[][])  [unwired: 1 in]
            n1717 = Insert Into Array(array=w3777, index (row)=1, new element=w3767) -> (w3776:dbl[][])  [unwired: 1 in]
            n1718 = Insert Into Array(array=w3775, index (row)=1, new element=w3763) -> (w3774:dbl[][])  [unwired: 1 in]
            n1719 = Insert Into Array(array=w3770, index (row)=1, new element=w3765) -> (w3771:dbl[][])  [unwired: 1 in]
          }
        }
        "Channel 1" <- w3694
        "Channel 2" <- w3638
        "Channel 3" <- w3689
        "Channel 4" <- w3645
        n1720 = case shown="False" w3666 {
          tunnel: [u32 16448250 ("Plot.Plot Color") u32 16711680 ("Plot.Plot Color")] -> w3665
          frame False {
          }
          frame True {
          }
        }
        n1721 = case shown="False" w3662 {
          tunnel: [u32 16448250 ("Plot.Plot Color") u32 16711680 ("Plot.Plot Color")] -> w3661
          frame False {
          }
          frame True {
          }
        }
        n1722 = case shown="False" w3646 {
          tunnel: [u32 16448250 ("Plot.Plot Color") u32 16711680 ("Plot.Plot Color")] -> w3642
          frame False {
          }
          frame True {
          }
        }
        n1723 = case shown="False" "Show BG removed?" {
          tunnel: [u32 16744703 ("Plot.Plot Color") u32 16741120 ("Plot.Plot Color")] -> w3635
          frame False {
          }
          frame True {
          }
        }
        n1724 = property on="Channel 1" class="WFGraph (strict)"("Active Plot"=w3636, "Plot.Plot Color"=w3635, "Plot.Line Style"=u8 1, "Plot.Line Width"=u8 2, "BG Color"=w3665) -> ()  [unwired: 2 in, 2 out]
        n1725 = property on="Channel 2" class="WFGraph (strict)"("Active Plot"=w3636, "Plot.Plot Color"=w3635, "Plot.Line Style"=u8 1, "Plot.Line Width"=u8 2, "BG Color"=w3661) -> ()  [unwired: 2 in, 2 out]
        n1726 = property on="Channel 4" class="WFGraph (strict)"("Active Plot"=w3636, "Plot.Plot Color"=w3635, "Plot.Line Style"=u8 1, "Plot.Line Width"=u8 2, "BG Color"=w3642) -> ()  [unwired: 2 in, 2 out]
        n1727 = property on="Channel 3" class="WFGraph (strict)"("Active Plot"=w3636, "Plot.Plot Color"=w3635, "Plot.Line Style"=u8 1, "Plot.Line Width"=u8 2, "BG Color"=w3657) -> ()  [unwired: 2 in, 2 out]
      }
      frame Error {
        w3778 = u32 16448250 ("Plot Area:Colors:BG Color")
        n1728 = property on="Channel 1" class="WFGraph (strict)"("BG Color"=w3778) -> ()  [unwired: 2 in, 2 out]
        n1729 = property on="Channel 2" class="WFGraph (strict)"("BG Color"=w3778) -> ()  [unwired: 2 in, 2 out]
        n1730 = property on="Channel 3" class="WFGraph (strict)"("BG Color"=w3778) -> ()  [unwired: 2 in, 2 out]
      }
    }
    "DisplayLoop" <- w3628
  }
  n1731 = disable-structure "Diagram Disable Structure" shown="Disabled" {
    frame Disabled {
      w3780 = T51 {"Horizontal"=500, "Vertical"=100}  # Top Left Corner
      n1732 = Control Help Window(0:w3780, 1:TRUE ("Show")) -> ()
      n1733 = call <vilib>:"TDMS - File Viewer.vi"() -> ()  [unwired: 6 in, 2 out]
    }
    frame Enabled {
    }
  }
  n1734 = while {
    tunnel: w19 -> [w3829]
    shift-right: [w3792] -> _
    shift-left: _ -> [w3825]
    tunnel: [w3783] -> w1 mode=indexing
    i -> [w3809]
    stop <- w3789 stop-if-true
    # "Channel 3"
    # "Channel 2"
    # "Channel 1"
    # "use FGV for gain value"
    # "stop on error"
    # "Gain adjustment and Data processing"
    n1735 = Tick Count (ms)() -> (millisecond timer value=w3792:u32)
    n1736 = Wait on Notification(notifier=w3829, ignore previous (F)=TRUE) -> (notification=w3803:T14, error out=w3782:errorcluster)  [unwired: 2 in, 2 out]
    n1737 = Subtract(x=w3792, y=w3825) -> (x-y=→"PID loop timing(ms)":u32)
    n1738 = Unbundle(w3803) -> ("CH1&2"=w3819:dbl[][], "CH3"=w3818:dbl[][])  [unwired: 2 out]
    n1739 = call "SeperateChanData.vi"("Input (Ch1&2)"=w3819) -> ("Ch1"=w3814:dbl[][], "Ch2"=w3812:dbl[][])
    n1740 = call "SeperateChanData.vi"("Input (Ch1&2)"=w3818) -> ("Ch1"=w3808:dbl[][], "Ch2"=w3801:dbl[][])
    n1741 = call "AvgArrayTimeCritical.vi"("2D array"=w3814) -> ("1D Avg"=w3813:dbl[])  [unwired: 10 in]
    n1742 = call "AvgArrayTimeCritical.vi"("2D array"=w3812) -> ("1D Avg"=w3823:dbl[])  [unwired: 10 in]
    n1743 = call "AvgArrayTimeCritical.vi"("2D array"=w3808) -> ("1D Avg"=w3820:dbl[])  [unwired: 10 in]
    n1744 = call "AvgArrayTimeCritical.vi"("2D array"=w3801) -> ("1D Avg"=w3800:dbl[])  [unwired: 10 in]
    n1745 = Array Max & Min(array=w3813) -> (max value=w3811:dbl)  [unwired: 3 out]
    n1746 = Array Max & Min(array=w3823) -> (max value=w3810:dbl)  [unwired: 3 out]
    n1747 = Array Max & Min(array=w3820) -> (max value=w3793:dbl)  [unwired: 3 out]
    n1748 = Array Max & Min(array=w3800) -> (max value=w3798:dbl)  [unwired: 3 out]
    n1749 = local read "Auto gain ch4"() -> (w3799:bool)
    n1750 = local read "Auto gain ch1"() -> (w3817:bool)
    n1751 = local read "Auto gain ch2"() -> (w3816:bool)
    n1752 = local read "Auto gain ch3"() -> (w3815:bool)
    n1753 = case shown="True" w3799 {
      tunnel: w3798 -> [_ w3876]
      tunnel: "V target(1.0)" -> [_ w3874]
      tunnel: [FALSE w3871] -> w3796
      tunnel: [0.0 ("CtrlV") w3866] -> w3797
      frame False {
        # "Manual control"
      }
      frame True {
        # "PID control"
        n1754 = global read "GlobalVariables.vi" "Ch4GainLim(Log)"() -> (w3877:cluster{"GainMax":dbl, "GainMin":dbl})
        n1755 = call-poly <vilib>:"PID.vi"("output range"=w3877, "PID gains"="Ch4 PID gains", "process variable"=w3876, "setpoint"=w3874) -> ("output"=w3875:dbl)  [unwired: 6 in, 1 out]
        n1756 = Power Of 10(x=w3875) -> (10^x=w3867:dbl)
        "Gain4" <- w3867
        n1757 = call "V4FGV.vi"("action(write)"=enum16{"write", "read"}."read") -> ("Error Out"=w3870:errorcluster, "V3 out"=w3872:dbl)  [unwired: 9 in]
        n1758 = call "GainToCtrlV.vi"("Gain"=w3867, "Channel"=enum16{"Ch1", "Ch2", "Ch3", "Ch4"}."Ch4") -> ("CtrlV"=w3866:dbl)  [unwired: 8 in, 1 out]
        n1759 = call "V4FGV.vi"("Error In"=w3870, "V3 in"=w3866) -> ()  [unwired: 8 in, 2 out]
        n1760 = local write "V 4"(w3866) -> ()
        n1761 = Not Equal?(x=w3866, y=w3872) -> (x != y?=w3871:bool)
      }
    }
    n1762 = case shown="True" w3817 {
      tunnel: "V target(1.0)" -> [_ w3891]
      tunnel: w3811 -> [_ w3888]
      tunnel: [0.0 ("CtrlV") w3880] -> w3790
      tunnel: [FALSE w3882] -> w3807
      frame False {
        # "Manual control"
      }
      frame True {
        # "PID control"
        n1763 = global read "GlobalVariables.vi" "Ch1GainLim(Log)"() -> (w3887:cluster{"GainMax":dbl, "GainMin":dbl})
        n1764 = call-poly <vilib>:"PID.vi"("output range"=w3887, "PID gains"="Ch1 PID gains", "process variable"=w3888, "setpoint"=w3891) -> ("output"=w3886:dbl)  [unwired: 6 in, 1 out]
        n1765 = Power Of 10(x=w3886) -> (10^x=w3885:dbl)
        "Gain1" <- w3885
        n1766 = call "V1FGV.vi"("action (write)"=enum16{"write", "read"}."read") -> ("Error Out"=w3881:errorcluster, "V1 out"=w3883:dbl)  [unwired: 9 in]
        n1767 = call "GainToCtrlV.vi"("Gain"=w3885, "Channel"=enum16{"Ch1", "Ch2", "Ch3"}."Ch1") -> ("CtrlV"=w3880:dbl)  [unwired: 8 in, 1 out]
        n1768 = local write "V 1"(w3880) -> ()
        n1769 = call "V1FGV.vi"("Error In"=w3881, "V1 in"=w3880) -> ()  [unwired: 8 in, 2 out]
        n1770 = Not Equal?(x=w3880, y=w3883) -> (x != y?=w3882:bool)
      }
    }
    n1771 = case shown="True" w3816 {
      tunnel: w3810 -> [_ w3918]
      tunnel: "V target(1.0)" -> [_ w3919]
      tunnel: [FALSE w3912] -> w3806
      tunnel: [0.0 ("CtrlV") w3908] -> w3802
      frame False {
        # "Manual control"
      }
      frame True {
        # "PID control"
        n1772 = global read "GlobalVariables.vi" "Ch2GainLim(Log)"() -> (w3916:cluster{"GainMax":dbl, "GainMin":dbl})
        n1773 = call-poly <vilib>:"PID.vi"("output range"=w3916, "PID gains"="Ch2 PID gains", "process variable"=w3918, "setpoint"=w3919) -> ("output"=w3915:dbl)  [unwired: 6 in, 1 out]
        n1774 = Power Of 10(x=w3915) -> (10^x=w3913:dbl)
        "Gain2" <- w3913
        n1775 = call "V2FGV.vi"("action(write)"=enum16{"write", "read"}."read") -> ("Error Out"=w3909:errorcluster, "V2 out"=w3910:dbl)  [unwired: 9 in]
        n1776 = call "GainToCtrlV.vi"("Gain"=w3913, "Channel"=enum16{"Ch1", "Ch2", "Ch3"}."Ch2") -> ("CtrlV"=w3908:dbl)  [unwired: 8 in, 1 out]
        n1777 = local write "V 2"(w3908) -> ()
        n1778 = call "V2FGV.vi"("Error In"=w3909, "V2 in"=w3908) -> ()  [unwired: 8 in, 2 out]
        n1779 = Not Equal?(x=w3908, y=w3910) -> (x != y?=w3912:bool)
      }
    }
    n1780 = case shown="True" w3815 {
      tunnel: w3793 -> [_ w3903]
      tunnel: "V target(1.0)" -> [_ w3900]
      tunnel: [FALSE w3896] -> w3805
      tunnel: [0.0 ("CtrlV") w3894] -> w3804
      frame False {
        # "Manual control"
      }
      frame True {
        # "PID control"
        n1781 = global read "GlobalVariables.vi" "Ch3GainLim(Log)"() -> (w3904:cluster{"GainMax":dbl, "GainMin":dbl})
        n1782 = call-poly <vilib>:"PID.vi"("output range"=w3904, "PID gains"="Ch3 PID gains", "process variable"=w3903, "setpoint"=w3900) -> ("output"=w3902:dbl)  [unwired: 6 in, 1 out]
        n1783 = Power Of 10(x=w3902) -> (10^x=w3899:dbl)
        "Gain3" <- w3899
        n1784 = call "V3FGV.vi"("action(write)"=enum16{"write", "read"}."read") -> ("Error Out"=w3895:errorcluster, "V3 out"=w3897:dbl)  [unwired: 9 in]
        n1785 = call "GainToCtrlV.vi"("Gain"=w3899, "Channel"=enum16{"Ch1", "Ch2", "Ch3"}."Ch3") -> ("CtrlV"=w3894:dbl)  [unwired: 8 in, 1 out]
        n1786 = local write "V 3"(w3894) -> ()
        n1787 = call "V3FGV.vi"("Error In"=w3895, "V3 in"=w3894) -> ()  [unwired: 8 in, 2 out]
        n1788 = Not Equal?(x=w3894, y=w3897) -> (x != y?=w3896:bool)
      }
    }
    n1789 = call "LabJack_FGV.vi"("Operation(Read)"=enum16{"Write", "Read"}."Read" ("Operation"), "error in (no error)"=w3782) -> ("error out"=w3791:errorcluster, "Read data"=w3827:i32)  [unwired: 8 in]
    n1790 = flat-sequence {
      tunnel: [w3831] -> w3788
      tunnel: w3782 -> [_]
      frame #0 {
        n1791 = Tick Count (ms)() -> (millisecond timer value=w3831:u32)
      }
    }
    n1792 = case "Channel 1" shown="True" w3807 {
      tunnel: w3791 -> [w3857 w3863]
      tunnel: w3827 -> [w3856 w3862]
      tunnel: [w3857 w3858] -> w3786
      tunnel: [w3856 w3861] -> w3822
      tunnel: w3790 -> [_ w3859]
      frame False {
        # "Do nothing"
      }
      frame True {
        # "request V\nupdate FGV"
        n1793 = global read "GlobalVariables.vi" "Ch1 LJ pin"() -> (w3860:string)
        n1794 = call "LJM_eWriteName.vi"("Handle In"=w3862, "Name"=w3860, "Value"=w3859, "error in"=w3863) -> ("Handle Out"=w3861:i32, "error out"=w3858:errorcluster)  [unwired: 10 in]
      }
    }
    n1795 = case "Channel 2" shown="True" w3806 {
      tunnel: w3786 -> [w3848 w3855]
      tunnel: [w3848 w3850] -> w3785
      tunnel: w3822 -> [w3849 w3854]
      tunnel: [w3849 w3853] -> w3821
      tunnel: w3802 -> [_ w3851]
      frame False {
        # "Do nothing"
      }
      frame True {
        # "request V\nupdate FGV"
        n1796 = global read "GlobalVariables.vi" "Ch2 LJ pin"() -> (w3852:string)
        n1797 = call "LJM_eWriteName.vi"("Handle In"=w3854, "Name"=w3852, "Value"=w3851, "error in"=w3855) -> ("Handle Out"=w3853:i32, "error out"=w3850:errorcluster)  [unwired: 10 in]
      }
    }
    n1798 = case "Channel 3" shown="True" w3805 {
      tunnel: w3785 -> [w3841 w3847]
      tunnel: [w3841 w3843] -> w3784
      tunnel: w3821 -> [w3840 w3846]
      tunnel: w3804 -> [_ w3844]
      tunnel: [w3840 w3842] -> w3795
      frame False {
        # "Do nothing"
      }
      frame True {
        # "request V\nupdate FGV"
        n1799 = global read "GlobalVariables.vi" "Ch3 LJ pin"() -> (w3845:string)
        n1800 = call "LJM_eWriteName.vi"("Handle In"=w3846, "Name"=w3845, "Value"=w3844, "error in"=w3847) -> ("Handle Out"=w3842:i32, "error out"=w3843:errorcluster)  [unwired: 10 in]
      }
    }
    n1801 = case "Channel 4" shown="True" w3796 {
      tunnel: w3784 -> [w3833 w3839]
      tunnel: w3795 -> [w3832 w3838]
      tunnel: [w3833 w3834] -> w3789
      tunnel: [w3832 w3837] -> _
      tunnel: w3797 -> [_ w3835]
      frame False {
        # "Do nothing"
      }
      frame True {
        # "request V\nupdate FGV"
        n1802 = global read "GlobalVariables.vi" "Ch4 LJ pin"() -> (w3836:string)
        n1803 = call "LJM_eWriteName.vi"("Handle In"=w3838, "Name"=w3836, "Value"=w3835, "error in"=w3839) -> ("Handle Out"=w3837:i32, "error out"=w3834:errorcluster)  [unwired: 10 in]
      }
    }
    "PID loop error out" <- w3789
    n1804 = flat-sequence {
      tunnel: [w3830] -> w3787
      tunnel: w3789 -> [_]
      frame #0 {
        n1805 = Tick Count (ms)() -> (millisecond timer value=w3830:u32)
      }
    }
    n1806 = Subtract(x=w3787, y=w3788) -> (x-y=w3783:u32)
    "LJ process (ms)" <- w3783
    "PID loop" <- w3809
  }
  "LJ time(ms)" <- w1
  n1807 = Unregister For Events(event registration refnum=w46, error in=w4) -> (error out=w52:errorcluster)
  n1808 = Destroy User Event(user event=w39, error in=w52) -> (error out=w3:errorcluster)
  n1809 = Close File(refnum=w21, error in=w3) -> ()  [unwired: 2 out]
  n1810 = Release Notifier(notifier=w16, error in (no error)=w49) -> (error out=w50:errorcluster)  [unwired: 1 in, 2 out]
  n1811 = Release Notifier(notifier=w17, error in (no error)=w38) -> (error out=w43:errorcluster)  [unwired: 1 in, 2 out]
  n1812 = call <vilib>:"Simple Error Handler.vi"("error in (no error)"=w50) -> ()  [unwired: 4 in, 5 out]
  n1813 = call <vilib>:"Simple Error Handler.vi"("error in (no error)"=w43) -> ()  [unwired: 4 in, 5 out]
  n1814 = Release Notifier(notifier=w59, error in (no error)=w58) -> (error out=w57:errorcluster)  [unwired: 1 in, 2 out]
  n1815 = Unregister For Events(event registration refnum=w63, error in=w61) -> (error out=w62:errorcluster)
  n1816 = call <vilib>:"Simple Error Handler.vi"("error in (no error)"=w57) -> ()  [unwired: 4 in, 5 out]
  n1817 = Destroy User Event(user event=w53, error in=w62) -> ()  [unwired: 1 out]
